vi "main4Ch_Biopsy.vi"() -> ()   [LabVIEW 2024]
doc: "Main VI for FLS imaging system."
uses:
  SubVI/DigitizerConfiguration/FLImDAQ.ctl
  <instrlib>/niScope/Controls/niScope trigger source.ctl
  SubVI/LabJack/LJ Pin Setting.ctl
  ConfigFiles/AimingBeamVideoConfig.ctl
  LaguerreDeconLib/DeconEngineClass/LaguerreDeconEngineClass.lvclass/LaguerreDeconEngineClass.ctl
  <vilib>/Utility/error.llb/DialogType.ctl
  LaguerreDeconLib/DeconEngineClass/LaguerreDeconEngineClass.lvclass
  <vilib>/event_ctls.llb/usereventprio.ctl
  <vilib>/Utility/miscctls.llb/LVMinMaxIncTypeDef.ctl
  SubVI/APD/APDClass.lvclass
  <vilib>/userDefined/High Color/IMAQdx.ctl
  <vilib>/vision/driver/IMAQdx.llb/IMAQdx Camera Control Mode.ctl
  <vilib>/vision/driver/IMAQdx.llb/IMAQdx Acquisition Mode.ctl
  <vilib>/vision/driver/IMAQdx.llb/IMAQdx Buffer Number Mode.ctl
  <vilib>/Analysis/baseanly.llb/Mean (DBL).vi
  SubVI/GlobalVariables.vi
  <vilib>/addons/control/pid/pid.llb/PID (DBL).vi
  <vilib>/Utility/file.llb/Write Delimited Spreadsheet (DBL).vi
  <instrlib>/niScope/Acquire/Fetch/niScope Multi Fetch Binary 16.vi
  <vilib>/Instr/_visa.llb/VISA Configure Serial Port (Instr).vi
  C:/Users/MarcuLab/Desktop/V6 APD LV/V6 APD LV/Kinesis/ThorLabs.MotionControl.KCube.DCServoCLI.dll
  Kinesis/ThorLabs.MotionControl.KCube.DCServoCLI.dll
  C:/Users/MarcuLab/Desktop/V6 APD LV/V6 APD LV/Kinesis/Thorlabs.MotionControl.DeviceManagerCLI.dll
  Kinesis/Thorlabs.MotionControl.DeviceManagerCLI.dll
  C:/Users/MarcuLab/Desktop/V6 APD LV/V6 APD LV/Kinesis/Thorlabs.MotionControl.GenericMotorCLI.dll
  Kinesis/Thorlabs.MotionControl.GenericMotorCLI.dll
  <userlib>/_OpenG.lib/file/file.llb/openg_file.lvlib
  <userlib>/_OpenG.lib/time/time.llb/openg_time.lvlib
  <vilib>/Analysis/NI_AALBase.lvlib
  <vilib>/Utility/miscctls.llb/LVPointTypeDef.ctl
  <vilib>/addons/control/pid/NI_PID_pid.lvlib
  <vilib>/vision/driver/NI_Vision_Acquisition_Software.lvlib
  <resource>/objmgr/imaqdx.rc
panel:
  out "Image 2":T1(plugin-control)
  in  "Live?":bool
  out "Record Backlog 2":i32
  in  "Auto gain ch4":bool=TRUE caption="Auto gain ch3"
  in  "V 4":dbl caption="Gain 3" min=0.0 max=4.67 step=0.1
  out "Gain4":dbl
  out "Lifetime 4":dbl caption="Lifetime 3"
  out "IntR4":dbl format="%#_2g"
  out "SNR4":dbl format="%#_3g"
  out "Channel 4":dbl[][](graph) caption="Channel 3"
  out "RunStartTime":u32
  out "Dig1 Temp":dbl
  out "Dig2 Temp":dbl
  out "Visualization PC video source":T2
  in  "V target(1.0)":dbl=1.0 caption="V target(1.5)" min=0.3 max=1.5 step=0.1 format="%#_4g"
  out "SNR3":dbl format="%#_3g"
  out "SNR2":dbl format="%#_3g"
  out "SNR1":dbl format="%#_3g"
  in  "Show BG removed?":bool=TRUE
  out "IntR3":dbl format="%#_2g"
  out "IntR2":dbl format="%#_2g"
  out "IntR1":dbl format="%#_2g"
  in  "Video Display":bool
  out "Gain3":dbl
  out "Gain2":dbl
  out "Gain1":dbl
  in  "Skip Data Save?":bool
  out "Aq Loop?":bool
  out "ML?":bool
  out "aquisition loop Error Out":errorcluster
  out "Laser f (Hz)":dbl
  out "Record Backlog":i32
  out "Fetch Record #":i32
  out "Sync Success?":bool
  out "Disclamer":picture
  out "Calibration #":i8
  out "BG #":i8
  in  "TCP Connect":bool
  out "Help":string
  in  "355nm Laser toggle":bool caption="355nm 460Hz"
  in  "Cali&iRF alignment":bool
  in  "Background":bool
  in  "Aiming beam toggle":bool caption="445nm 0Hz 20mA"
  out "Lifetime 3":dbl
  out "Lifetime 2":dbl
  in  "Auto gain ch3":bool=TRUE
  in  "Auto gain ch2":bool=TRUE
  in  "Auto gain ch1":bool=TRUE
  out "Run #":i8
  in  "StopButton":bool caption="Stop"
  out "Aquisition Status:":bool
  in  "StartButton":bool caption="Start"
  in  "V 3":dbl caption="Gain 3" min=0.0 max=4.68 step=0.1
  in  "V 2":dbl caption="Gain 2" min=0.0 max=4.62 step=0.1
  out "Lifetime 1":dbl
  in  "V 1":dbl caption="Gain 1" min=0.0 max=4.66 step=0.1 format="%#_4g"
  in  "Video Source":enum32{"Camera", "FrameGrabber"}(radio)
  out "Case #":string
  out "System Hardware Connection Status":T3
  out "Channel 3":dbl[][](graph)
  out "Channel 2":dbl[][](graph)
  out "Channel 1":dbl[][](graph)
  in  "Tab Control":T4(tab)
  in  "ScanRange(mm)":dbl=25.0
  in  "SerialNumber(Slow)":string="27000986"
  out "SlowAxisInfo":T5
  out "SlowAxisStatus":T6
  out "PNG write time (ms)":dbl(graph)
  in  "VideoMode":u32=12
  out "Acquired Frames/s":dbl
  out "FLIm 1st point time":dbl format="%_19f"
  out "Cam error out":errorcluster
  out "display loop timing(ms)":u32
  out "Aquisition loop timing(ms)":u32 format="%.2f"
  out "DisplayLoop":i32
  out "PID loop":i32 caption="processing loop"
  out "PID loop timing(ms)":u32 caption="processing loop timing(ms)"
  out "laser EM lamp V":dbl format="%0.6f"
  out "Decon Loop timing (ms)":dbl
  out "Auisition Loop idx":i32
  out "LJ process (ms)":u32
  out "LJ time(ms)":u32[](array[numeric])
  out "output variable":i32
  out "Lifetime (ns)":dbl(graph)
  out "Waveform Chart":dbl(graph)
  in  "Truncation":u32=600
  out "iRF Graph":dbl[][](graph)
  in  "Show BG":bool
  out "iRF length":i32
  out "BG length":i32
  out "data length":i32
  out "SysConfigCluster":T7
  out "LJ Pinout":T8={"Ch1 Bias"="DAC0", "Ch2 Bias"="DAC1", "Ch3 Bias"="DAC2", "Ch4 Bias"="DAC0", "355 PWM"="FIO0", "AimingBeam PWM"="FIO2", "Laser Ready"="FIO3", "Interlock"="FIO1", "Laser Start/Stop"="FIO1", "Red LED"="FIO1", "Green LED"="DIO3", "Foot Pedal"="DIO15"}
  out "FLImDAQ":T9={"Digitizer 1"="", "Digitizer 2"="", "Channel"=enum."Channel 0", "trigger source"="VAL_EXTERNAL", "trigger level"=0.5, "trigger delay"=1.35e-07, "min sample rate"=12500000000.0, "min record length"=2500, "vertical range"=1.0, "vertical offset"=-0.25, "Waveform to Avg"=2000} caption="FLIm DAQ Configuration" {"trigger delay" format="%^#.4e"; "trigger level" min=0.0 max=3.5 step=0.5 format="%.2f"; "vertical offset" format="%.4f"; "vertical range" format="%.2f"; "min sample rate" format="%#.2p"}
  in  "Sys Reconfig":bool
  out "PID loop error out":errorcluster caption="processing Error Out"
  out "decon error out":errorcluster
  out "Laser Rep Rate":dbl
  out "V4 Size":i32 caption="V3 Size"
  in  "Data Class":enum16{"Data", "BG", "Cali"}(ring)
  out "V1 Size":i32
  out "V2 Size":i32
  out "V3 Size":i32
  out "data Size":i32[](array[numeric])
  out "State log":string
  in  "Ch4 PID gains":T11={"proportional gain (Kc)"=30.0, "integral time (Ti, min)"=0.0003, "derivative time (Td, min)"=1e-05}
  in  "Ch3 PID gains":T11={"proportional gain (Kc)"=30.0, "integral time (Ti, min)"=0.0003, "derivative time (Td, min)"=1e-05}
  in  "Ch2 PID gains":T11={"proportional gain (Kc)"=30.0, "integral time (Ti, min)"=0.0003, "derivative time (Td, min)"=1e-05}
  in  "Ch1 PID gains":T11={"proportional gain (Kc)"=30.0, "integral time (Ti, min)"=0.0003, "derivative time (Td, min)"=1e-05}
  in  "Quit":bool
  in  "Radio Buttons":T12(radio)=enum."Ch2" caption="DeCon Chan"
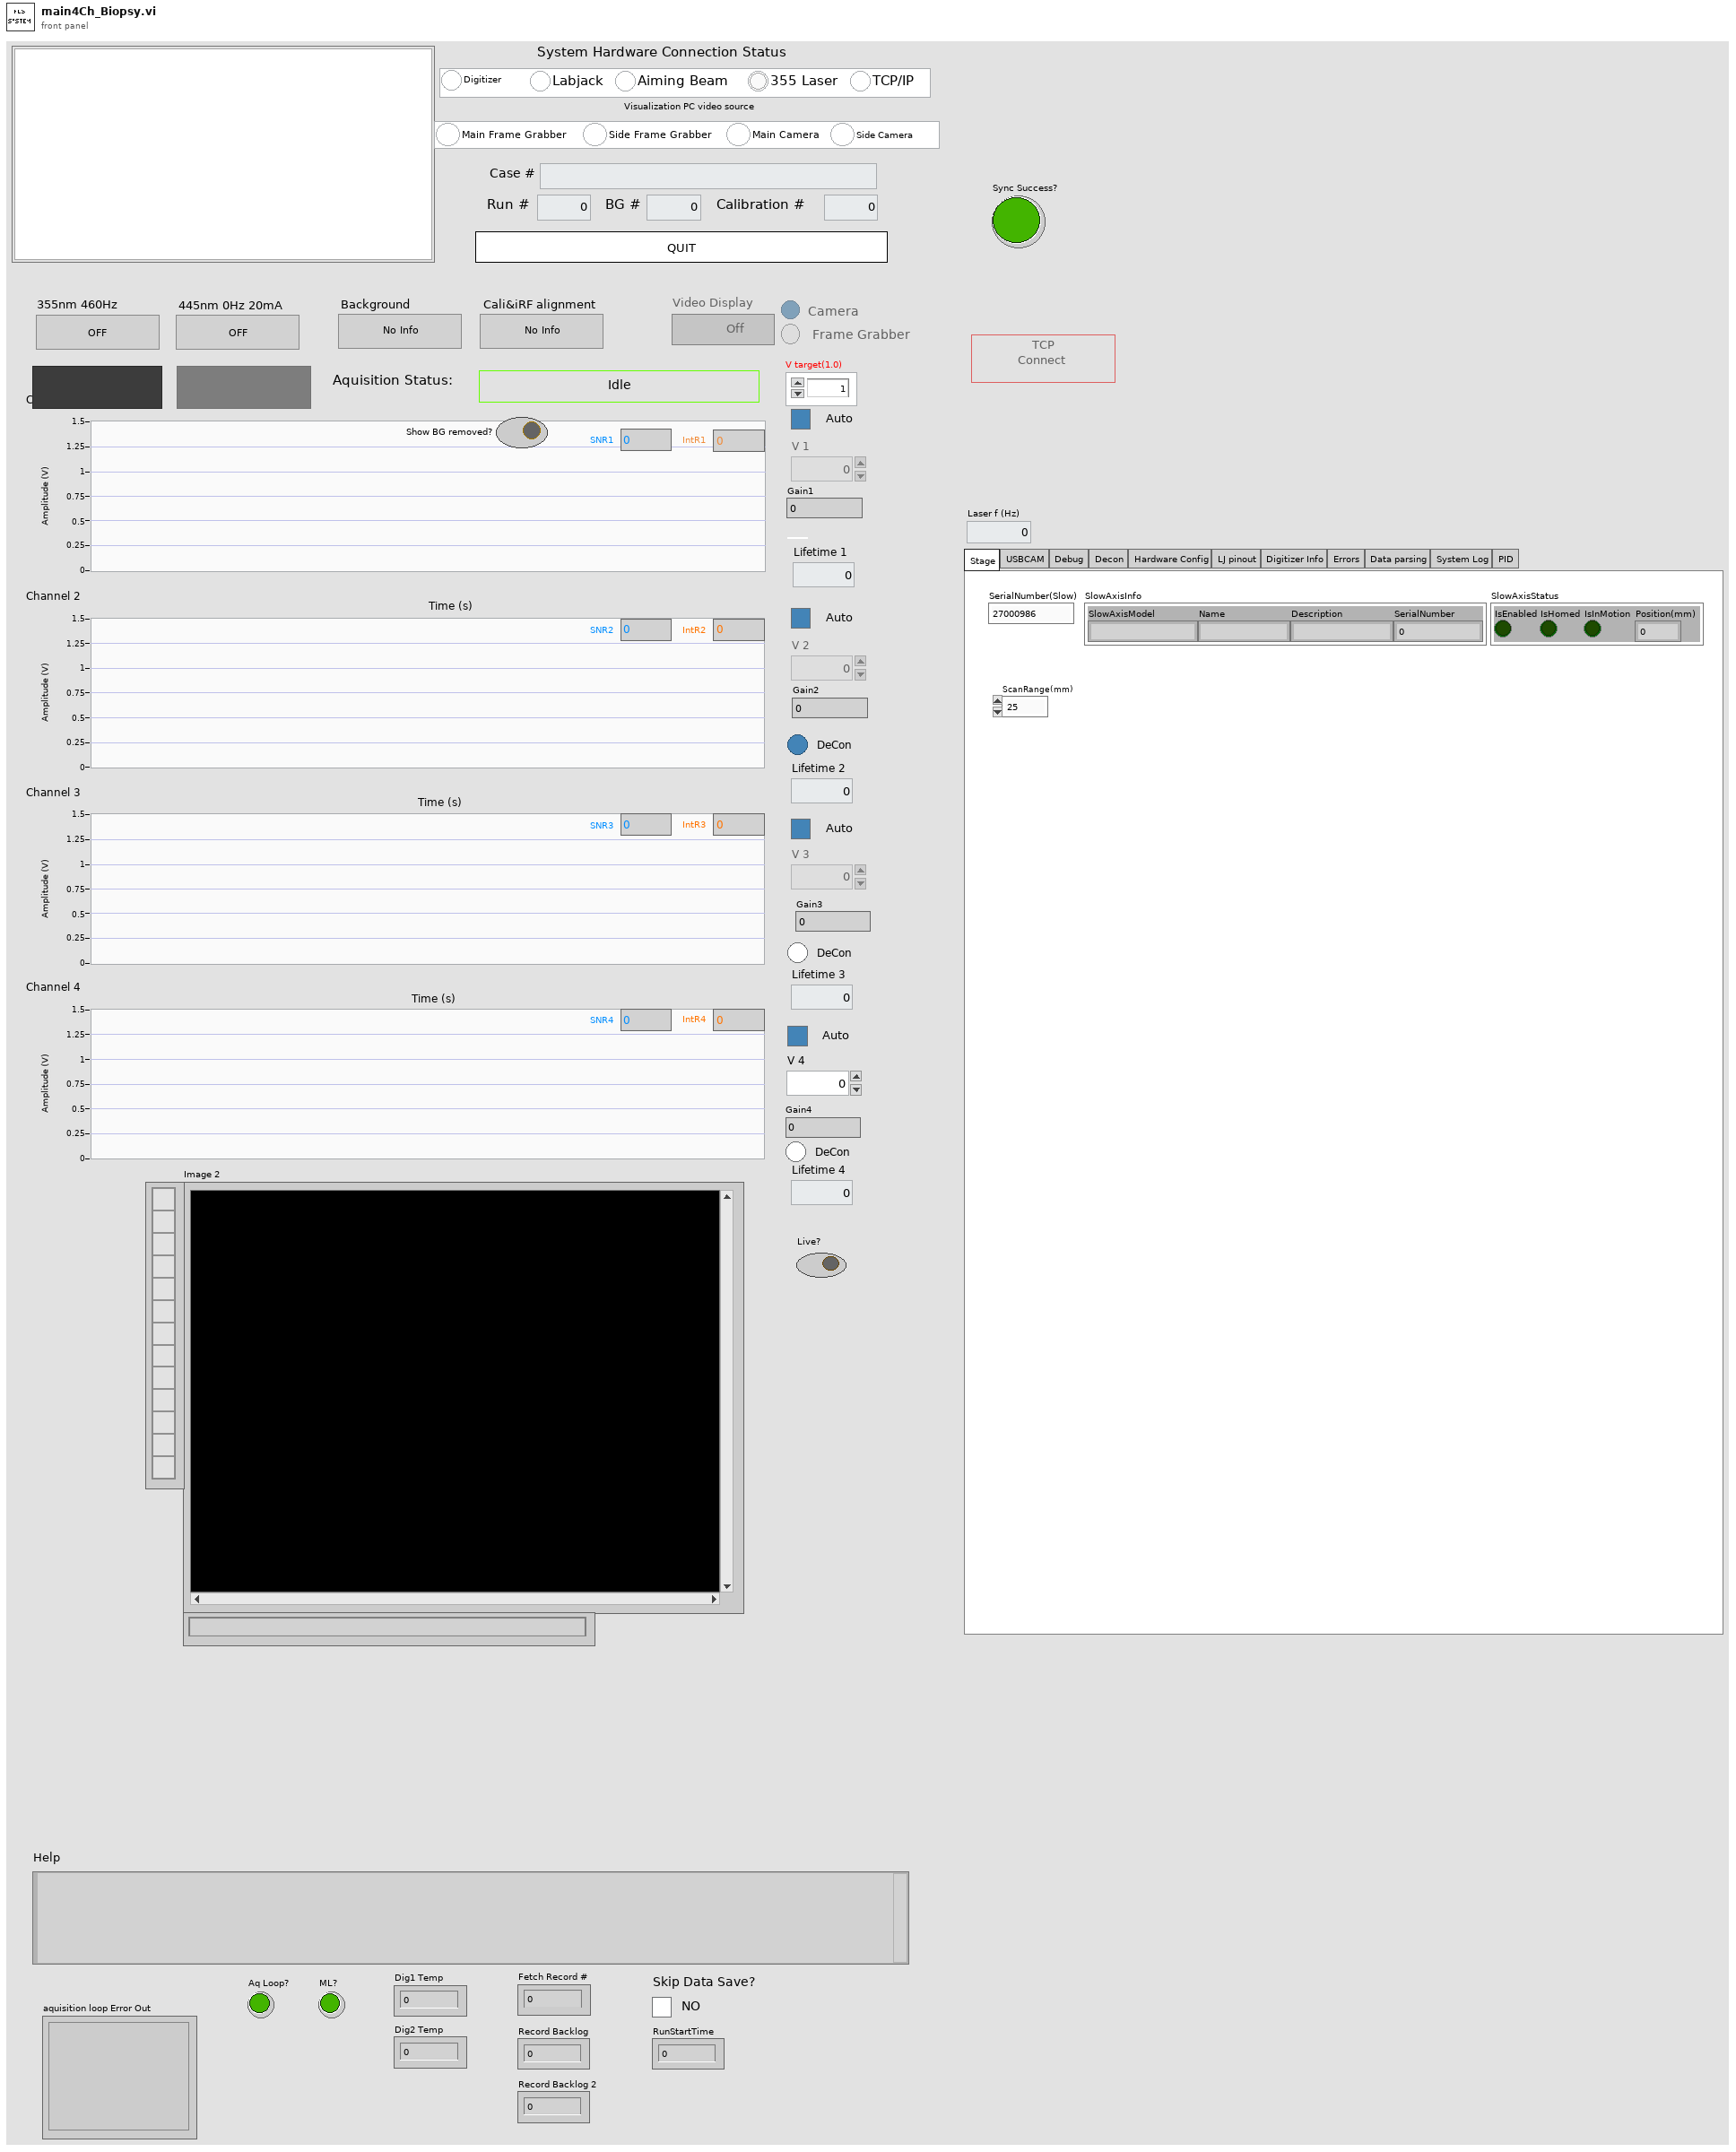
[diagram p1: front panel]
types:
  T1 = typedef "IMAQ Image.ctl" = refnum<image>
  T2 = cluster{"Main Frame Grabber":bool, "Side Frame Grabber":bool, "Main Camera":bool, "Side Camera":bool}
  T3 = cluster{"Digitizer":bool, "Labjack":bool, "Aiming Beam":bool, "355 Laser":bool, "TCP/IP":bool}
  T4 = enum32{"Stage", "USBCAM", "Debug", "Decon", "Hardware Config", "LJ pinout", "Digitizer Info", "Errors", "Data parsing", "System Log", "PID"}
  T5 = cluster{"SlowAxisModel":string, "Name":string, "Description":string, "SerialNumber":u32}
  T6 = cluster{"IsEnabled":bool, "IsHomed":bool, "IsInMotion":bool, "Position(mm)":dbl}
  T7 = cluster{"Ch1Enable?":bool, "Ch2Enable?":bool, "Ch3Enable?":bool, "Ch1AutoGain?":bool, "Ch2AutoGain?":bool, "Ch3AutoGain?":bool, "AimingBeamEnable?":bool}
  T8 = typedef "LJ Pin Setting.ctl" = cluster{"Ch1 Bias":string, "Ch2 Bias":string, "Ch3 Bias":string, "Ch4 Bias":string, "355 PWM":string, "AimingBeam PWM":string, "Laser Ready":string, "Interlock":string, "Laser Start/Stop":string, "Red LED":string, "Green LED":string, "Foot Pedal":string}
  T9 = typedef "FLImDAQ.ctl" = cluster{"Digitizer 1":refnum<k15>, "Digitizer 2":refnum<k15>, "Channel":enum16{"Channel 0", "Channel 1", "Channel 0&1"}, "trigger source":T10, "trigger level":dbl, "trigger delay":dbl, "min sample rate":dbl, "min record length":i32, "vertical range":dbl, "vertical offset":dbl, "Waveform to Avg":i16}
  T10 = typedef "niScope trigger source.ctl" = string
  T11 = cluster{"proportional gain (Kc)":dbl, "integral time (Ti, min)":dbl, "derivative time (Td, min)":dbl}
  T12 = enum32{"No Selection", "Ch1", "Ch2", "Ch3", "Ch4"}
  T13 = cluster{"remote start event":refnum<user-event>, "remote stop  event":refnum<user-event>}
  T14 = enum8{"Enabled", "Disabled", "Disabled and Grayed Out"}
  T15 = enum16{"open", "replace", "create", "open or create", "replace or create", "replace or create with confirmation"}
  T16 = cluster{"CH1":dbl[][], "CH2":dbl[][], "CH3":dbl[][], "CH4":dbl[][], "Gain cluster":cluster{"V1":dbl, "V2":dbl, "V3":dbl, "V4":dbl}}
  T17 = cluster{"idx":i32, "CH1&2":dbl[][], "CH3":dbl[][], "V cluster":cluster{"V1":dbl, "V2":dbl, "V3":dbl, "V4":dbl}}
  T18 = cluster{"Ch1 iRF":dbl[], "Ch2 iRF":dbl[], "Ch3 iRF":dbl[], "Ch4 iRF":dbl[]}
  T19 = enum16{"open", "open or create", "create or replace", "create", "open (read-only)"}
  T20 = enum32{"Invalid", "Standard", "Closed", "Hidden", "Minimized", "Maximized"}
  T21 = enum32{"invalid app kind", "Development System", "Run Time System", "Student Edition", "Embedded LabVIEW", "Evaluation", "Custom"}
  T22 = typedef "usereventprio.ctl" = enum32{"high priority", "normal priority"}
  T23 = enum32{"Bad", "Idle", "Run top level", "Running"}
  T24 = enum16{"Standard", "Buffered", "CRLF", "Immediate"}
  T25 = typedef "NI_Vision_Acquisition_Software.lvlib/IMAQdx Camera Control Mode.ctl" = enum32{"Controller", "Listener"}
  T26 = typedef "IMAQdx.ctl" = refnum<k21>
  T27 = typedef "NI_Vision_Acquisition_Software.lvlib/IMAQdx Acquisition Mode.ctl" = enum32{"One Shot", "Continuous"}
  T28 = typedef "AimingBeamVideoConfig.ctl" = cluster{"DeCon Channel":enum16{"1", "2", "3"}, "Scale Bar":bool, "Scale Low":dbl, "Scale High":dbl, "ANSI":dbl, "Radius":dbl, "3D?":bool, "Firefly?":bool, "Pentero?":bool}
  T29 = cluster{"Core":cluster{"Current VI Reference":refnum<vi>, "Close Panel on Exit?":bool}, "SysConfigCluster":cluster{"Ch1Enable?":bool, "Ch2Enable?":bool, "Ch3Enable?":bool, "Ch1AutoGain?":bool, "Ch2AutoGain?":bool, "Ch3AutoGain?":bool, "AimingBeamEnable?":bool}, "System Status":cluster{"Digitizer":bool, "Labjack":bool, "Aiming Beam":bool, "355 Laser":bool, "TCP/IP":bool}, "IDs":cluster{"RunID":i8, "BG ID":i8, "Cali ID":i8}, "CaseID":string, "DefaultPath":path, "Pathes":cluster{"DataPath":path, "BG Path":path, "iRFPath":path, "CaliPath":path}, "FLImDAQ":cluster{"resource name":refnum<k15>, "resource name 2":refnum<k15>, "Channel":enum16{"Channel 0", "Channel 1", "Channel 0&1"}, "trigger source":T10, "trigger level":dbl, "trigger delay":dbl, "min sample rate":dbl, "min record length":i32, "vertical range":dbl, "vertical offset":dbl, "Waveform to Avg":i32}, "SysRunning?":bool, "AB Cluster":cluster{"Aiming Beam COM Port":refnum<visa-resource-name>, "Min Current":dbl, "Max Current":dbl, "Default Current":dbl, "Freq":i32}, "LJ Pinout":T8, "355 PWM setting":cluster{"DIO_EF_CLOCK1_DIVISOR":i16, "DIO_EF_CLOCK1_ROLL_VALUE":i32, "DIO#_EF_INDEX":i16, "DIO#_EF_OPTIONS":i16, "DIO#_EF_CONFIG_A":i32}, "AB PWM setting":cluster{"DIO_EF_CLOCK1_DIVISOR":i16, "DIO_EF_CLOCK1_ROLL_VALUE":i32, "DIO#_EF_INDEX":i16, "DIO#_EF_OPTIONS":i16, "DIO#_EF_CONFIG_A":i32}, "Last Trigger":u32, "niTClk sessions":refnum<k20>[], "Laser start tic":u32, "TCP attempt count":i32, "Ch1Data":dbl[][], "Ch2Data":dbl[][], "Ch3Data":dbl[][], "Ch4Data":dbl[][], "V1":dbl[], "V2":dbl[], "V3":dbl[], "V4":dbl[], "SlowTimer":u32, "FastTimer":u32, "listener ID":refnum<k5>, "TempPath":path, "CaliPath":path, "LED vi reference":refnum<vi>, "Aquisition Timer":u32, "APDSerialNum":cluster{"Ch1APDSerial#":string, "Ch2APDSerial#":string, "Ch3APDSerial#":string, "Ch4APDSerial#":string}, "VideoConfig":T28, "LED vi ref open?":bool, "video source":cluster{"Main Frame Grabber":bool, "Side Frame Grabber":bool, "Main Camera":bool, "Side Camera":bool}, "bothVidSourceAvail":bool, "StageSerial":string, "DeviceHandle":refnum<k24>, "StageHomed?":bool}
  T30 = typedef "LVCursorListTypeDef.ctl" = cluster{"Name":string, "Color":u32, "Style":u8, "Point Style":u8, "Name Visible":bool, "Allow Drag":bool, "Cursor Mode":u32, "Plot":i32, "Index":i32, "Position":cluster{"X":dbl, "Y":dbl}, "X Scale":u32, "Y Scale":u32, "Watch Plots":i32[], "Watch All Plots":bool, "Plot Area":i32, "Label Offset":cluster{"X":dbl, "Y":dbl}}[]
  T31 = cluster{"Name":string, "Color":u32, "Style":u8, "Point Style":u8, "Name Visible":bool, "Allow Drag":bool, "Cursor Mode":u32, "Plot":i32, "Index":i32, "Position":cluster{"X":dbl, "Y":dbl}, "X Scale":u32, "Y Scale":u32, "Watch Plots":i32[], "Watch All Plots":bool, "Plot Area":i32, "Label Offset":cluster{"X":dbl, "Y":dbl}}
  T32 = cluster{"Ch1APDSerial#":string, "Ch2APDSerial#":string, "Ch3APDSerial#":string, "Ch4APDSerial#":string}
  T33 = cluster{"DataPath":path, "BG Path":path, "iRFPath":path, "CaliPath":path}
  T34 = cluster{"DIO_EF_CLOCK1_DIVISOR":i16, "DIO_EF_CLOCK1_ROLL_VALUE":i32, "DIO#_EF_INDEX":i16, "DIO#_EF_OPTIONS":i16, "DIO#_EF_CONFIG_A":i32}
  T35 = cluster{"Aiming Beam COM Port":refnum<visa-resource-name>, "Min Current":dbl, "Max Current":dbl, "Default Current":dbl, "Freq":i32}
  T36 = cluster{"resource name":refnum<k15>, "resource name 2":refnum<k15>, "Channel":enum16{"Channel 0", "Channel 1", "Channel 0&1"}, "trigger source":T10, "trigger level":dbl, "trigger delay":dbl, "min sample rate":dbl, "min record length":i32, "vertical range":dbl, "vertical offset":dbl, "Waveform to Avg":i32}
  T37 = cluster{"Current VI Reference":refnum<vi>, "Close Panel on Exit?":bool}
  T38 = cluster{"Channel 1":dbl[], "Channel 2":dbl[], "Channel 3":dbl[], "Channel 4":dbl[]}
  T39 = cluster{"V 1":dbl[], "V 2":dbl[], "V 3":dbl[], "V 4":dbl[]}
  T40 = cluster{"Ch1 WF":dbl[], "Ch2 WF":dbl[], "Ch3 WF":dbl[], "Ch4 WF":dbl[], "V1":dbl, "V2":dbl, "V3":dbl, "V4":dbl}
  T41 = typedef "iRFData.ctl" = cluster{"dt":dbl, "NumOfWFs":i32, "WFLength":i32, "iRFCtrlV":dbl[], "iRFWFsAvg":dbl[][], "iRFRaw":dbl[][]}
  T42 = cluster{"mean":dbl, "mean":dbl, "mean":dbl, "mean":dbl}
  T43 = cluster{"V1":dbl, "V2":dbl, "V3":dbl, "V4":dbl}[]
  T44 = cluster{"DataPath":path, "CaseID":string, "RunID":i16, "Ch1Data":dbl[][], "Ch2Data":dbl[][], "Ch3Data":dbl[][], "Ch4Data":dbl[][], "V1":dbl[], "V2":dbl[], "V3":dbl[], "V4":dbl[], "LaserRepRate":u16, "WFAverage":i16, "RunStartTime":u64}
  T45 = typedef "DialogType.ctl" = u16
  T46 = typedef "LJ PWM Setting.ctl" = cluster{"DIO_EF_CLOCK1_DIVISOR":i16, "DIO_EF_CLOCK1_ROLL_VALUE":i32, "DIO#_EF_INDEX":i16, "DIO#_EF_OPTIONS":i16, "DIO#_EF_CONFIG_A":i32}
  T47 = typedef "AimingBeam.ctl" = cluster{"Aiming Beam COM Port":refnum<visa-resource-name>, "Min Current":dbl, "Max Current":dbl, "Default Current":dbl, "Frequency(Hz)":u32}
  T48 = cluster{"DC1":i32, "DC2":i32, "BG1":i32, "BG2":i32}
  T49 = typedef "LVMinMaxIncTypeDef.ctl" = cluster{"Minimum":dbl, "Maximum":dbl, "Increment":dbl}
  T50 = typedef "LVBoundsTypeDef.ctl" = cluster{"Width":u32, "Height":u32}
  T51 = typedef "imagedata.ctl" = cluster{"image type":i32, "image depth":i32, "image":u8[], "mask":u8[], "colors":u32[], "Rectangle":cluster{"left":i16, "top":i16, "right":i16, "bottom":i16}}
  T52 = cluster{"DC Idx1":i32, "DC Idx2":i32, "BG Idx1":i32, "BG Idx2":i32}
  T53 = cluster{"IsEnabled":bool, "IsHomed":bool, "IsInMotion":bool, "Position":dbl}
  T54 = typedef "LVPointTypeDef.ctl" = cluster{"Horizontal":i16, "Vertical":i16}
  T55 = cluster{"actualSamples":i32, "absoluteInitialX":dbl, "relativeInitialX":dbl, "xIncrement":dbl, "offset":dbl, "gain":dbl, "reserved1":dbl, "reserved2":dbl}[]
  T56 = cluster{"V1 out":dbl, "V2 out":dbl, "V3 out":dbl, "V3 out":dbl}
  T57 = cluster{i32, dbl[][], dbl[][], cluster{"V1 out":dbl, "V2 out":dbl, "V3 out":dbl, "V3 out":dbl}}
  T58 = cluster{dbl[][], dbl[][], dbl[][], dbl[][], "V cluster":cluster{"V1":dbl, "V2":dbl, "V3":dbl, "V4":dbl}}
  T59 = typedef "NI_Vision_Acquisition_Software.lvlib/IMAQdx Buffer Number Mode.ctl" = enum32{"Next", "Last", "Buffer Number", "Every", "Last New"}
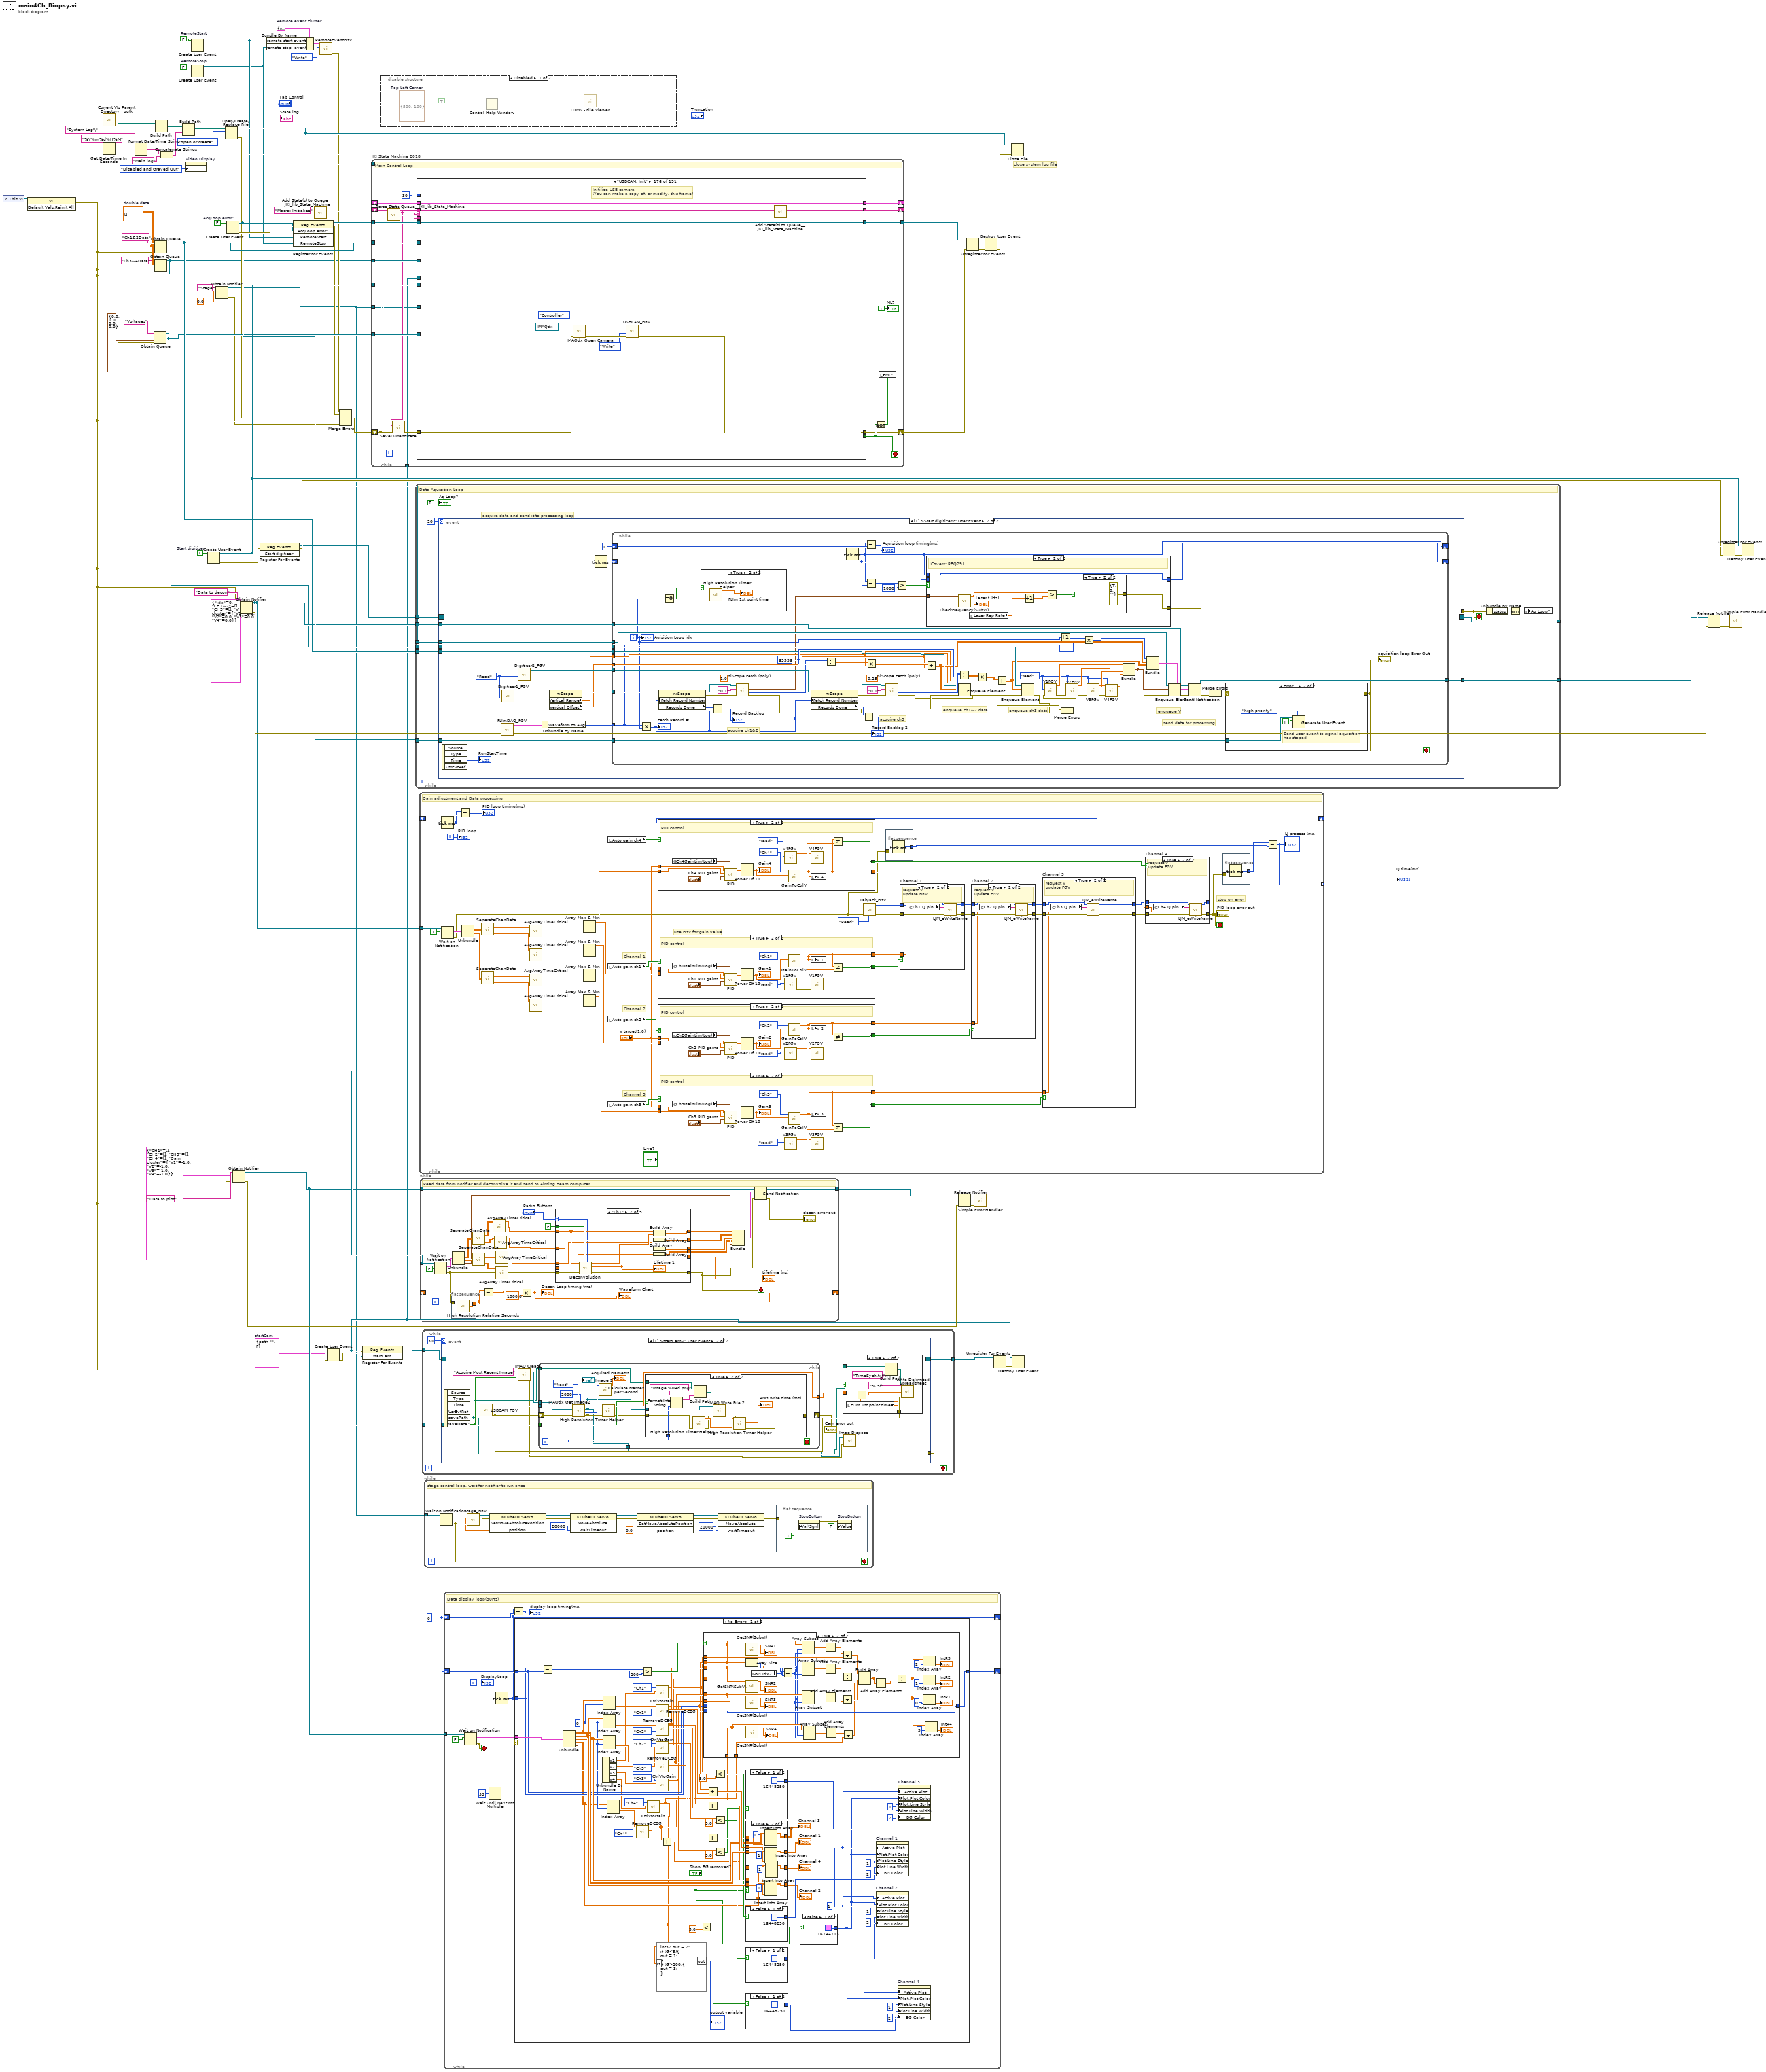
[diagram p0: block diagram]
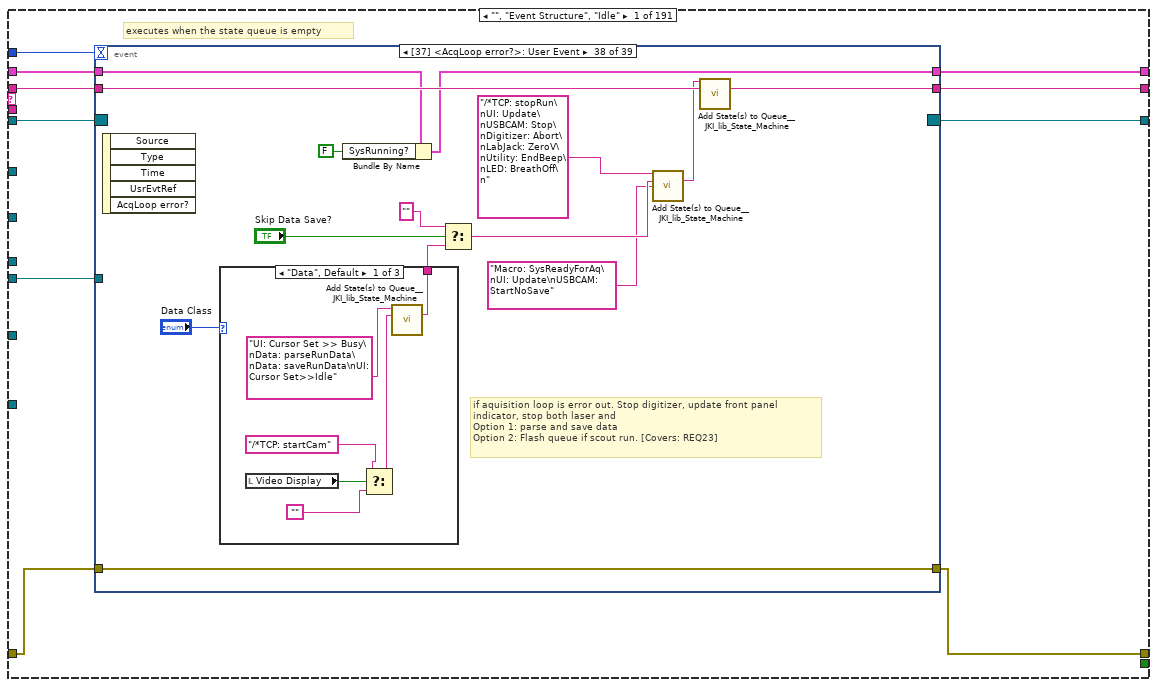
[diagram p2: hidden frame]
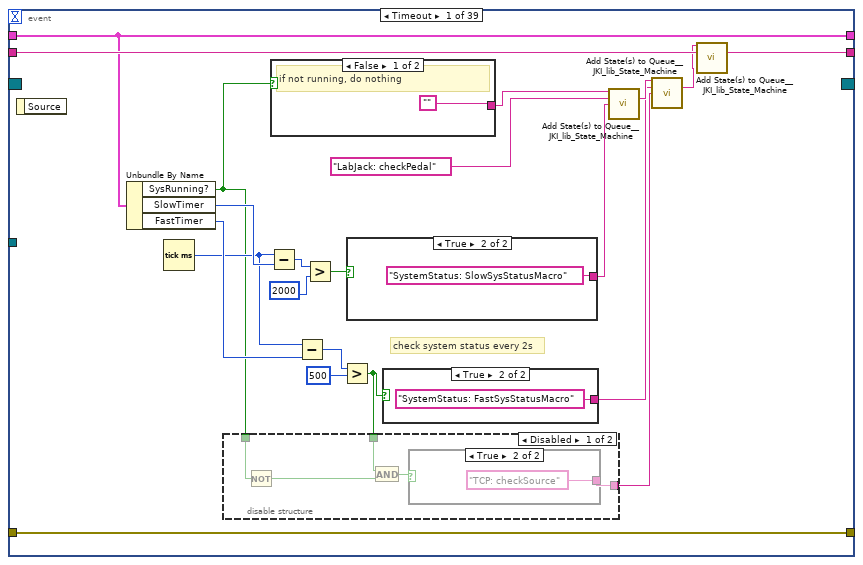
[diagram p3: hidden frame]
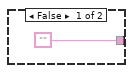
[diagram p4: hidden frame]
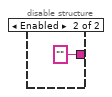
[diagram p5: hidden frame]
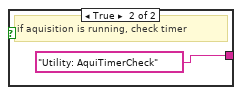
[diagram p6: hidden frame]
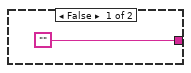
[diagram p7: hidden frame]
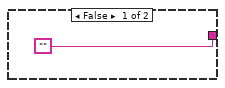
[diagram p8: hidden frame]
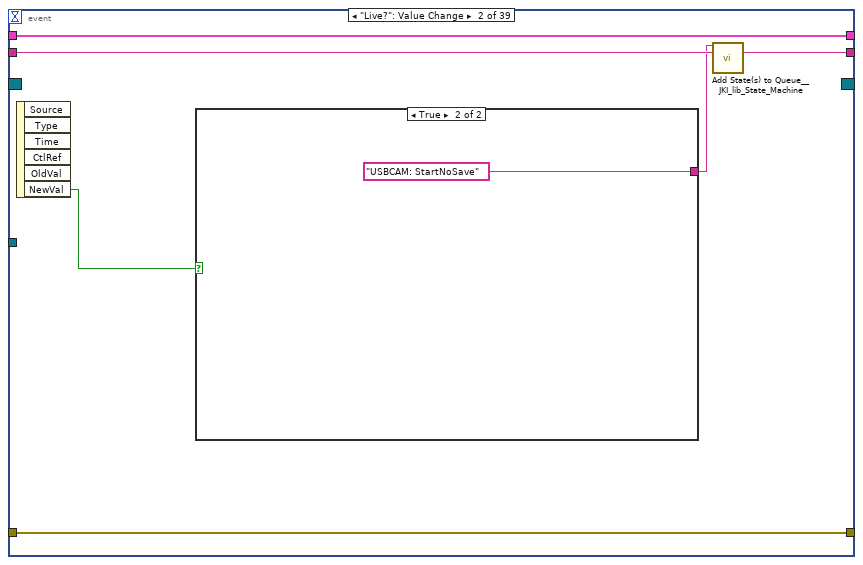
[diagram p9: hidden frame]
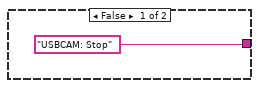
[diagram p10: hidden frame]
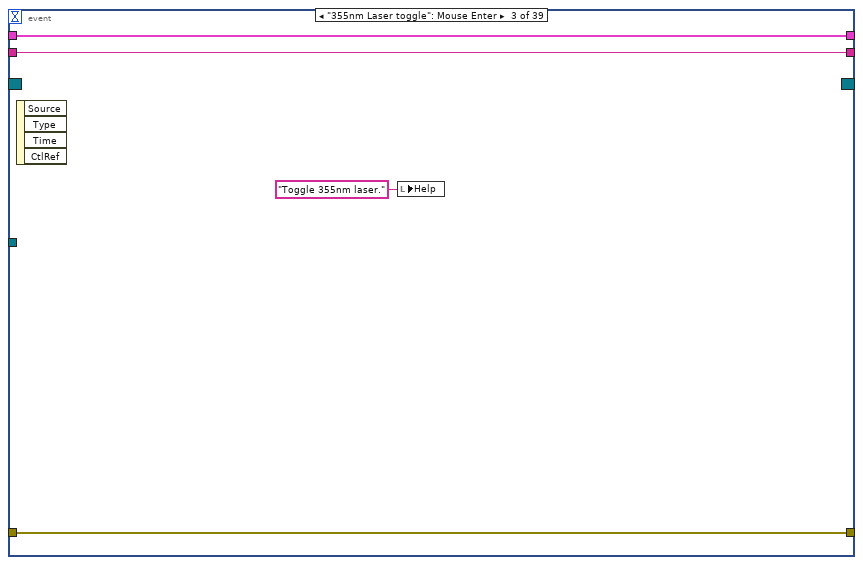
[diagram p11: hidden frame]
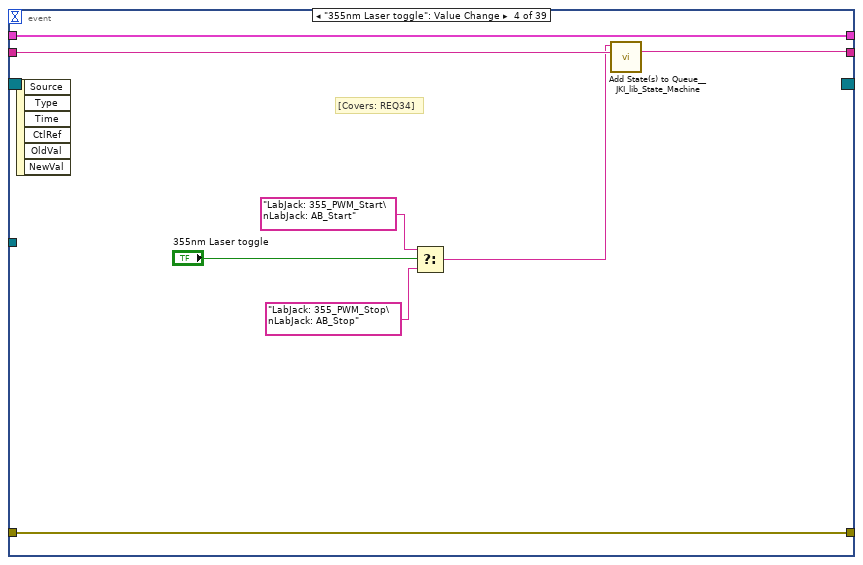
[diagram p12: hidden frame]
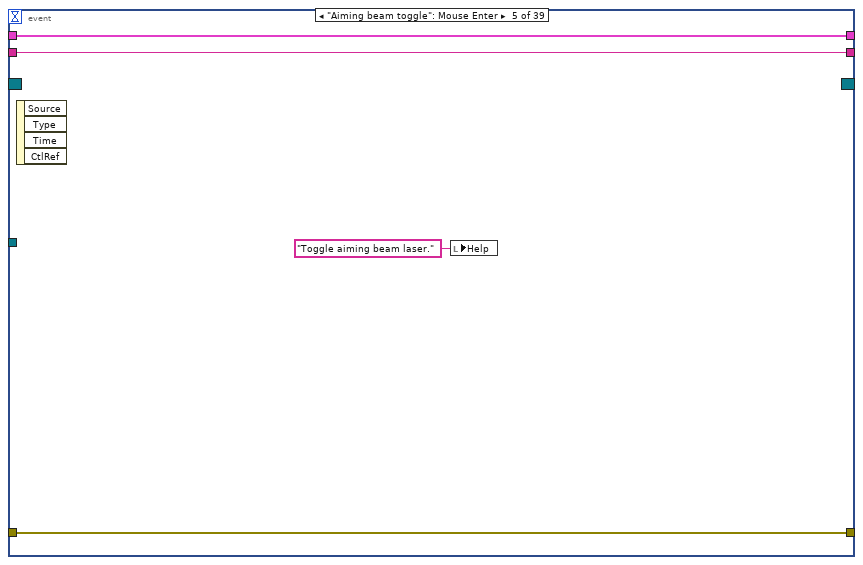
[diagram p13: hidden frame]
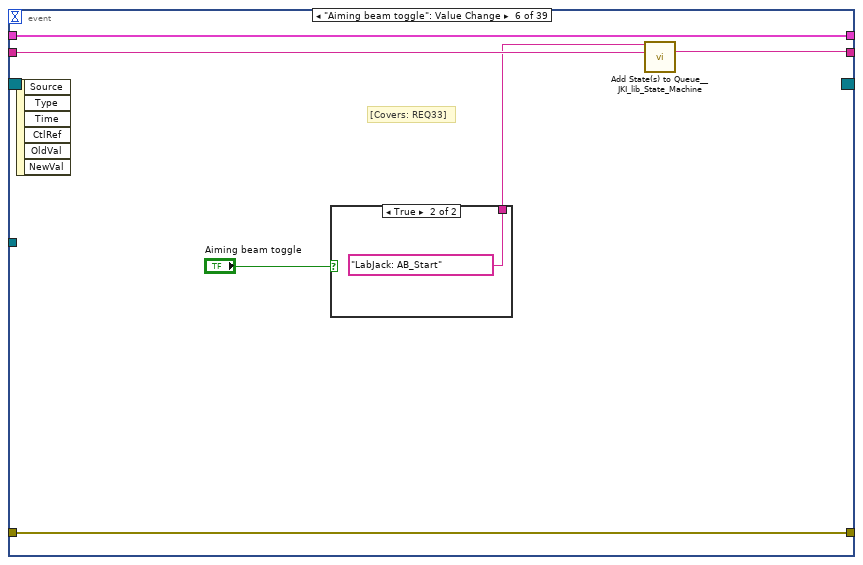
[diagram p14: hidden frame]
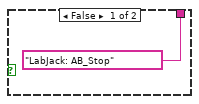
[diagram p15: hidden frame]
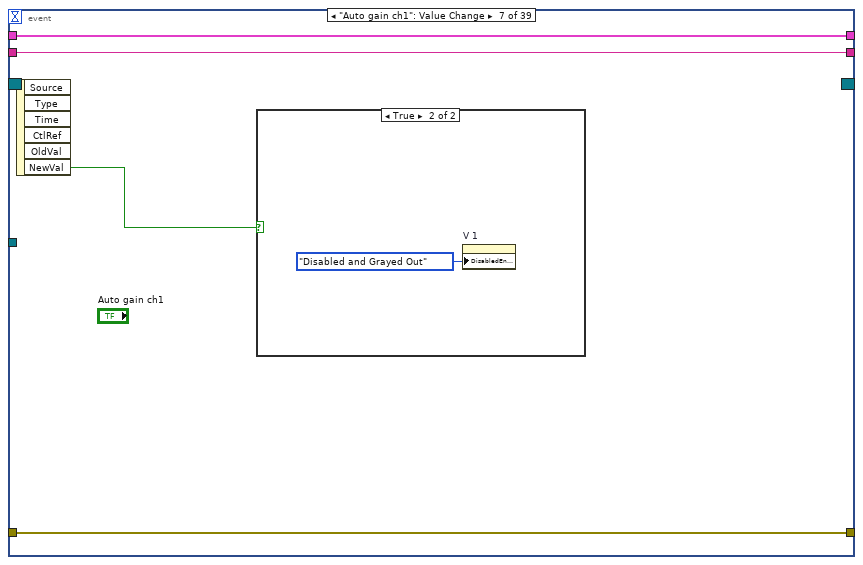
[diagram p16: hidden frame]
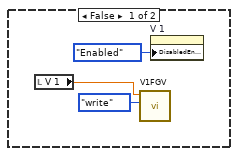
[diagram p17: hidden frame]
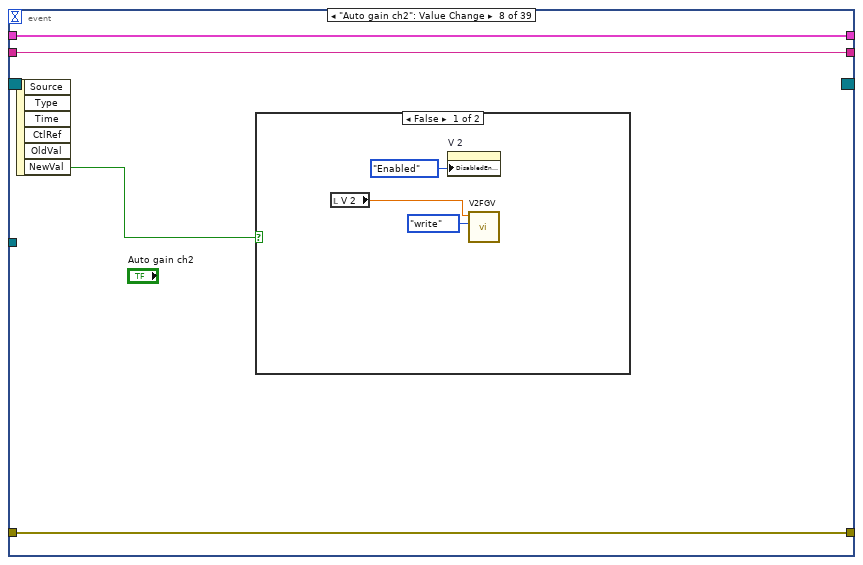
[diagram p18: hidden frame]
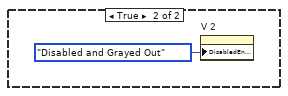
[diagram p19: hidden frame]
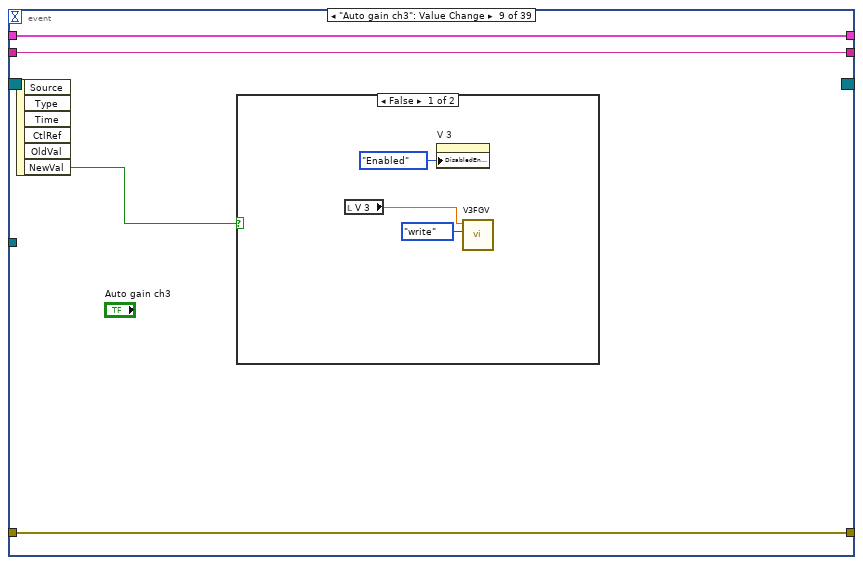
[diagram p20: hidden frame]
diagram:
  w12 = cluster{"savePath":path, "saveData?":bool} {"savePath"=path "", "saveData?"=FALSE}  # startCam
  w20 = T13 {"remote start event"=refnum, "remote stop  event"=refnum}  # Remote event cluster
  w23 = FALSE  # RemoteStop
  w24 = FALSE  # RemoteStart
  w27 = u32 0 ("millisecond timer value")
  w57 = FALSE  # AcqLoop error?
  w67 = TRUE  # Start digitizer
  w70 = dbl[][] []  # double data
  # "close system log file"
  n1 = control-ref of="This VI"() -> (w72:refnum<vi>)
  n2 = invoke on="Invoke Node" class="VI" method="Default Vals.Reinit All"(reference=w72) -> (error out=w11:errorcluster)  [unwired: 2 in, 2 out]
  n3 = call <userlib>:"Current VIs Parent Directory__ogtk.vi"() -> ("Parent Directory (+ Relative)"=w43:path)  [unwired: 5 in]
  n4 = Get Date/Time In Seconds() -> (seconds since 1Jan1904=w41:timestamp)
  n5 = Format Date/Time String(time format string (%c)="%Y%m%d%H%M", seconds (now)=w41) -> (date/time string=w38:string)  [unwired: 1 in]
  n6 = Obtain Queue(name (unnamed)="Voltages", element data type=cluster{"V1":dbl, "V2":dbl, "V3":dbl, "V4":dbl} {"V1"=0.0, "V2"=0.0, "V3"=0.0, "V4"=0.0}, error in (no error)=w11) -> (queue out=w44:refnum<queue>)  [unwired: 2 in, 2 out]
  n7 = Obtain Queue(name (unnamed)="Ch3&4Data", element data type=w70, error in (no error)=w11) -> (queue out=w8:refnum<queue>)  [unwired: 2 in, 2 out]
  n8 = Obtain Queue(name (unnamed)="Ch1&2Data", element data type=w70, error in (no error)=w11) -> (queue out=w68:refnum<queue>)  [unwired: 2 in, 2 out]
  n9 = Build Path(base path=w43, name or relative path="System Log\\") -> (appended path=w34:path)
  n10 = Concatenate Strings(w38, "Main.log" ("string")) -> (w36:string)
  n11 = Build Path(base path=w34, name or relative path=w36) -> (appended path=w39:path)
  n12 = property on="Video Display" class="Bool (strict)"("DisabledEnum"=T14."Disabled and Grayed Out" ("Disabled")) -> ()  [unwired: 2 in, 2 out]
  n13 = Create User Event(user event datatype=w24) -> (user event=w22:refnum<user-event>)  [unwired: 1 in, 1 out]
  n14 = Create User Event(user event datatype=w23) -> (user event=w21:refnum<user-event>)  [unwired: 1 in, 1 out]
  n15 = Create User Event(user event datatype=w67, error in=w11) -> (user event=w56:refnum<user-event>, error out=w48:errorcluster)
  n16 = Obtain Notifier(name (unnamed)="Stage", notification data type=0.0) -> (notifier out=w1:refnum<notifier>, error out=w2:errorcluster)  [unwired: 2 in, 1 out]
  n17 = Open/Create/Replace File(file path (use dialog)=w39, operation (0:open)=T15."open or create") -> (refnum out=w31:refnum<file>, error out=w32:errorcluster)  [unwired: 4 in, 1 out]
  n18 = Create User Event(user event datatype=w57) -> (user event=w47:refnum<user-event>, error out=w49:errorcluster)  [unwired: 1 in]
  n19 = Obtain Notifier(name (unnamed)="Data to plot", notification data type=T16 {"CH1"=[], "CH2"=[], "CH3"=[], "CH4"=[], "Gain cluster"={"V1"=-1.0, "V2"=-1.0, "V3"=-1.0, "V4"=-1.0}}, error in (no error)=w11) -> (notifier out=w25:refnum<notifier>, error out=w52:errorcluster)  [unwired: 1 in, 1 out]
  n20 = Obtain Notifier(name (unnamed)="Data to decon", notification data type=T17 {"idx"=0, "CH1&2"=[], "CH3"=[], "V cluster"={"V1"=0.0, "V2"=0.0, "V3"=0.0, "V4"=0.0}}, error in (no error)=w11) -> (notifier out=w29:refnum<notifier>, error out=w61:errorcluster)  [unwired: 1 in, 1 out]
  n21 = register-events(error in=w48, w56) -> (reference out=w58:refnum<event-registration>, error out=w64:errorcluster)  [unwired: 1 in]
  n22 = Bundle By Name(cluster=w20, "remote start event"=w22, "remote stop  event"=w21) -> (w18:T13)
  n23 = register-events(error in=w49, w47, w22, w21) -> (reference out=w51:refnum<event-registration>, error out=w17:errorcluster)  [unwired: 1 in]
  n24 = call <vilib>:"Add State(s) to Queue__JKI_lib_State_Machine.vi"("State(s) in (\"\")"="Macro: Initialize") -> ("States Out"=w74:string)  [unwired: 14 in]
  n25 = call "RemoteEventFGV.vi"("Operation (Read)"=enum16{"Read", "Write"}."Write", "Remote Event in"=w18) -> ("Error Out"=w14:errorcluster)  [unwired: 8 in, 1 out]
  n26 = Create User Event(user event datatype=w12, error in=w11) -> (user event=w5:refnum<user-event>, error out=w10:errorcluster)
  n27 = Merge Errors(w14, w17, w32, w11, w2) -> (w33:errorcluster)
  n28 = register-events(error in=w10, w5) -> (reference out=w9:refnum<event-registration>)  [unwired: 1 in, 1 out]
  n29 = while "JKI State Machine 2018" {
    shift-right: [w93] -> _
    shift-left: _ -> [w92]
    shift-right: [w77] -> w16
    shift-left: w33 -> [w79]
    shift-right: [w94] -> _
    shift-left: w74 -> [w95]
    tunnel: w68 -> [w90]
    tunnel: w8 -> [w89]
    tunnel: w56 -> [w88]
    tunnel: w51 -> [w87]
    tunnel: [w86] -> w50
    tunnel: w44 -> [w82]
    tunnel: w31 -> [w81]
    tunnel: w5 -> [w76]
    tunnel: w1 -> [w75]
    stop <- w85 stop-if-true
    # "Main Control Loop"
    n30 = call <vilib>:"Parse State Queue__JKI_lib_State_Machine.vi"("State Queue"=w95, "Error In (no error)"=w79) -> ("Remaining States"=w97:string, "Current State"=w80:string, "Arguments"=w96:string)  [unwired: 11 in]
    n31 = call "SaveCurrentState.vi"("error in (no error)"=w79, "Current State"=w80, "Byte Stream File in"=w81) -> ("error out"=w78:errorcluster)  [unwired: 8 in]
    n32 = case shown="\"USBCAM: Init\"" w80 {
      selector: w80 -> [_ _ _ _ _ _ _ _ _ _ _ _ _ _ _ _ _ _ _ _ _ _ _ _ w1090 _ _ _ _ _ _ _ _ _ _ _ _ _ _ _ _ _ _ _ _ _ _ _ _ _ _ _ _ _ _ _ _ _ _ _ _ _ _ _ _ _ _ _ _ _ _ _ _ _ _ _ _ _ _ _ _ _ _ _ _ _ _ _ _ _ _ _ _ _ _ _ _ _ _ _ _ _ _ _ _ _ _ _ _ _ _ _ _ _ _ _ _ _ _ _ _ _ _ _ _ _ _ _ _ _ _ _ _ _ _ _ _ _ _ _ _ _ _ _ _ _ _ _ _ _ _ _ _ _ _ _ _ _ _ _ _ _ _ _ _ _ _ _ _ _ _ _ _ _ _ _ _ _ _ _ _ _ _ _ _ _ _ _ _ _ _]
      tunnel: w97 -> [w107 w523 w532 w538 w544 w566 w579 w624 w630 w657 w676 w747 w762 w793 w820 w852 w866 w895 w909 w994 w1031 w1070 w1083 w1088 w1094 w1122 w1130 w1153 w1158 w1171 w1190 w1218 w1246 w1284 w1289 w1295 w1319 w1343 w1367 w1391 w1396 w1413 w1460 w1482 w1498 w1513 w1533 w1538 w1550 w1579 w1605 w1617 w1655 w1668 w1674 w1685 w1697 w1728 w1741 w1755 w1770 w1789 w1824 w1829 w1843 w1853 w1869 w1881 w1893 w1921 w1936 w1941 w1953 w1967 w1972 w1980 w1988 w1997 w2006 w2011 w2019 w2028 w2046 w2063 w2083 w2094 w2116 w2131 w2148 w2153 w2161 w2169 w2174 w2182 w2189 w2197 w2204 w2214 w2242 w2250 w2257 w2265 w2270 w2278 w2285 w2291 w2300 w2316 w2321 w2328 w2340 w2410 w2422 w2431 w2448 w2457 w2480 w2497 w2508 w2521 w2546 w2569 w2575 w2591 w2613 w2621 w2627 w2632 w2639 w2649 w2661 w2670 w2675 w2687 w2692 w2702 w2708 w2714 w2719 w2724 w2729 w2739 w2763 w2784 w2789 w2800 w2825 w2852 w2875 w2880 w2895 w2946 w2992 w3037 w3048 w3066 w3086 w3100 w3113 w3121 w3138 w3160 w3184 w3203 w3221 w3239 w3257 w3271 w3285 w3304 w3318 w3333 w3348 w3357 w3362 w3373 w3385 w3406 w3420 w3428 w3439 w3444 w3451 w3475 w3482 w3501 w3515 w3523 w3550 w3559 w3564]
      tunnel: w96 -> [_ _ _ _ _ _ _ _ _ _ _ _ _ _ _ _ _ _ _ _ _ _ _ _ _ _ _ _ _ _ _ _ _ _ _ _ _ _ _ _ _ _ _ _ _ _ _ _ _ _ _ _ _ _ _ _ w1695 _ _ _ _ _ _ _ _ _ _ _ _ _ _ _ _ _ _ _ _ _ _ _ _ _ _ _ _ _ _ _ _ _ _ _ _ _ _ _ _ w2205 _ _ _ _ _ _ _ _ _ _ _ w2323 w2334 _ _ _ _ w2454 _ _ _ _ _ w2565 _ _ _ _ _ _ w2634 _ _ _ _ _ _ w2698 _ _ _ _ _ _ _ _ _ _ _ _ _ _ _ _ _ _ _ _ _ _ _ _ _ _ _ _ _ _ _ _ _ _ _ _ _ _ _ _ _ _ _ _ _ _ _ _ _ _ _ _ _ _ _]
      tunnel: w92 -> [w105 w520 w528 w535 w541 w563 w576 _ w626 w653 w672 w744 w753 w790 w812 w843 w863 w892 w906 w955 w1023 w1058 w1078 w1085 w1092 w1115 w1127 w1151 w1155 w1159 w1180 w1210 w1238 w1280 w1286 w1292 w1300 w1324 w1349 w1373 w1393 w1406 w1450 w1479 w1483 w1510 w1530 w1535 w1539 w1568 w1595 w1610 w1638 w1666 w1671 w1678 w1693 w1711 w1736 w1747 w1765 w1782 w1807 w1826 w1839 w1847 w1866 w1878 w1890 w1909 w1925 w1938 w1951 w1965 w1969 w1974 w1981 w1993 w2002 w2008 w2015 w2025 w2033 w2050 w2078 w2084 w2113 w2124 w2146 w2150 w2154 w2162 w2171 w2180 w2186 w2194 w2201 w2211 w2239 w2247 w2254 w2262 w2267 w2272 w2283 w2288 w2294 w2313 w2318 w2326 w2336 w2407 w2412 w2425 w2446 w2455 w2470 w2494 w2505 w2515 w2539 w2566 w2572 w2584 w2609 w2618 w2624 w2629 w2636 w2643 w2657 w2667 w2672 w2684 w2689 w2695 w2705 w2711 w2716 w2721 w2726 w2736 w2761 w2782 w2786 w2798 w2823 w2850 w2873 w2877 w2888 w2940 w2988 w3034 w3044 w3061 w3081 w3095 w3109 w3115 w3133 w3155 w3179 w3198 w3216 w3234 w3252 w3266 w3280 w3299 w3313 w3328 w3345 w3355 w3359 w3367 w3383 w3398 w3412 w3426 w3436 w3442 w3449 w3461 w3479 w3490 w3502 w3519 w3548 w3551 w3561]
      tunnel: [w98 w521 w530 w536 w542 w564 w577 w622 w628 w649 w668 w721 w749 w791 w800 w832 w856 w883 w907 w931 w1020 w1057 w1079 w1086 w1096 w1119 errorcluster {"status"=FALSE, "code"=0, "source"=""} ("error out") w1150 w1156 w1169 w1188 w1202 w1225 w1282 w1287 w1293 w1301 w1325 w1350 w1374 w1394 w1397 w1442 w1473 w1487 w1511 w1521 w1536 w1542 w1566 w1594 w1609 w1625 w1660 w1672 w1683 w1687 w1702 w1731 w1743 w1761 w1781 w1798 w1827 w1831 w1849 w1864 w1876 w1888 w1911 w1926 w1939 w1943 w1962 w1970 w1978 w1986 w1990 w1999 w2009 w2012 w2021 w2036 w2058 w2077 w2088 w2106 w2128 w2144 w2151 w2159 w2167 w2172 w2179 w2187 w2195 w2202 w2212 w2240 w2248 w2255 w2263 w2268 w2276 w2282 w2289 w2297 w2314 w2319 w2324 w2337 w2408 w2416 w2428 w2438 w2451 w2471 w2495 w2504 w2517 w2541 w2567 w2573 w2581 w2603 w2619 w2625 w2630 w2637 w2647 w2659 w2668 w2673 w2685 w2690 w2700 w2706 w2712 w2717 w2722 w2727 w2737 w2751 w2775 w2787 w2791 w2810 w2842 w2867 w2878 w2882 w2941 w2989 w3035 w3043 w3063 w3083 w3097 w3111 w3117 w3135 w3157 w3181 w3200 w3218 w3236 w3254 w3268 w3282 w3301 w3315 w3329 w3346 w3353 w3360 w3364 w3374 w3400 w3414 w3422 w3435 w3440 w3446 w3455 w3477 w3498 w3512 w3518 w3545 w3556 w3562] -> w77
      tunnel: w78 -> [w104 w521 w530 w536 w542 w564 w577 w622 w628 w650 w666 w721 w748 w791 w801 w839 w856 w873 w907 w931 w1021 w1060 w1080 w1086 w1095 w1119 w1123 w1150 w1156 w1169 w1188 w1201 w1237 w1282 w1287 w1293 w1305 w1329 w1354 w1378 w1394 w1404 w1445 w1472 w1486 w1511 w1523 w1536 w1541 w1567 w1585 w1615 w1636 w1659 w1672 w1680 w1690 w1701 w1730 w1746 w1760 w1780 w1797 w1827 w1837 w1850 w1863 w1875 w1887 w1910 w1927 w1939 w1942 w1955 w1970 w1978 w1986 w1989 w1998 w2009 w2013 w2022 w2041 w2057 w2076 w2087 w2112 w2127 w2143 w2151 w2159 w2167 w2172 w2179 w2187 w2195 w2202 w2212 w2240 w2248 w2255 w2263 w2268 w2276 w2282 w2289 w2297 w2314 w2319 w2325 w2338 w2408 w2417 w2427 w2434 w2450 w2472 w2495 w2504 w2512 w2544 w2567 w2573 w2586 w2602 w2619 w2625 w2630 w2637 w2647 w2659 w2668 w2673 w2685 w2690 w2700 w2706 w2712 w2717 w2722 w2727 w2737 w2750 w2774 w2787 w2790 w2809 w2832 w2858 w2878 _ w2942 w2989 w3035 w3042 w3062 w3082 w3096 w3111 w3116 w3134 w3156 w3180 w3199 w3217 w3235 w3253 w3267 w3281 w3300 w3314 w3327 w3346 w3352 w3360 w3368 w3381 w3399 w3413 w3421 w3434 w3440 w3445 w3459 w3476 w3498 w3512 w3517 w3544 w3556 w3562]
      tunnel: [w106 w522 w531 w537 w543 w565 w578 w623 w629 w656 w675 w746 w761 w792 w819 w851 w865 w894 w908 w993 w1030 w1069 w1082 w1087 w1093 w1121 w1129 w1152 w1157 w1170 w1189 w1217 w1245 w1283 w1288 w1294 w1318 w1342 w1366 w1390 w1395 w1412 w1459 w1481 w1497 w1512 w1532 w1537 w1549 w1578 w1604 w1616 w1654 w1667 w1673 w1684 w1696 w1727 w1740 w1754 w1769 w1788 w1823 w1828 w1842 w1852 w1868 w1880 w1892 w1920 w1935 w1940 w1952 w1966 w1971 w1979 w1987 w1996 w2005 w2010 w2018 w2027 w2045 w2062 w2082 w2093 w2115 w2130 w2147 w2152 w2160 w2168 w2173 w2181 w2188 w2196 w2203 w2213 w2241 w2249 w2256 w2264 w2269 w2277 w2284 w2290 w2299 w2315 w2320 w2327 w2339 w2409 w2421 w2430 w2447 w2456 w2479 w2496 w2507 w2520 w2545 w2568 w2574 w2590 w2612 w2620 w2626 w2631 w2638 w2648 w2660 w2669 w2674 w2686 w2691 w2701 w2707 w2713 w2718 w2723 w2728 w2738 w2762 w2783 w2788 w2799 w2824 w2851 w2874 w2879 w2894 w2945 w2991 w3036 w3047 w3065 w3085 w3099 w3112 w3120 w3137 w3159 w3183 w3202 w3220 w3238 w3256 w3270 w3284 w3303 w3317 w3332 w3347 w3356 w3361 w3372 w3384 w3405 w3419 w3427 w3438 w3443 w3450 w3474 w3481 w3500 w3514 w3522 w3549 w3558 w3563] -> w94
      tunnel: [_ _ _ _ _ _ _ _ _ _ _ _ _ _ _ _ _ _ _ _ _ _ _ _ _ _ _ TRUE _ _ _ _ _ _ _ _ _ _ _ _ _ _ _ _ _ _ _ _ _ _ _ _ _ _ _ _ _ _ _ _ _ _ _ _ _ _ _ _ _ _ _ _ _ _ _ _ _ _ _ _ _ _ _ _ _ _ _ _ _ _ _ _ _ _ _ _ _ _ _ _ _ _ _ _ _ _ _ _ _ _ _ _ _ _ _ _ _ _ _ _ _ _ _ _ _ _ _ _ _ _ _ _ _ _ _ _ _ _ _ _ _ _ _ _ _ _ _ _ _ _ _ _ _ _ _ _ _ _ _ _ _ _ _ _ _ _ _ _ _ _ _ _ _ _ _ _ _ _ _ _ _ _ _ _ _ _ _ _ _ _ _] -> w85
      tunnel: [w103 w520 w528 w535 w541 w563 w576 w597 w626 w653 w672 w744 w753 w790 w812 w843 w863 w892 w906 w955 w1024 w1059 w1078 w1085 w1092 w1120 w1127 w1151 w1155 w1160 w1181 w1211 w1239 w1281 w1286 w1292 w1300 w1324 w1349 w1373 w1393 w1406 w1451 w1479 w1484 w1510 w1531 w1535 w1540 w1568 w1595 w1614 w1638 w1666 w1671 w1681 w1693 w1711 w1736 w1747 w1765 w1782 w1807 w1826 w1840 w1847 w1866 w1878 w1890 w1909 w1925 w1938 w1951 w1965 w1969 w1975 w1982 w1994 w2003 w2008 w2016 w2026 w2034 w2056 w2065 w2089 w2114 w2125 w2146 w2150 w2155 w2163 w2171 w2180 w2186 w2194 w2201 w2211 w2239 w2247 w2254 w2262 w2267 w2272 w2283 w2288 w2294 w2313 w2318 w2326 w2336 w2407 w2413 w2426 w2446 w2455 w2470 w2494 w2505 w2516 w2540 w2566 w2572 w2585 w2609 w2618 w2624 w2629 w2636 w2644 w2657 w2667 w2672 w2684 w2689 w2695 w2705 w2711 w2716 w2721 w2726 w2736 w2761 w2782 w2786 w2798 w2823 w2850 w2873 w2877 w2893 w2939 w2988 w3034 w3044 w3061 w3081 w3095 w3109 w3115 w3133 w3155 w3179 w3198 w3216 w3234 w3252 w3266 w3280 w3299 w3313 w3330 w3345 w3355 w3359 w3367 w3383 w3398 w3412 w3426 w3436 w3442 w3449 w3462 w3479 w3490 w3503 w3519 w3548 w3551 w3561] -> w93
      tunnel: 30 ("Timeout") -> [w102 _ _ _ _ _ _ _ _ _ _ _ _ _ _ _ _ _ _ _ _ _ _ _ _ _ _ _ _ _ _ _ _ _ _ _ _ _ _ _ _ _ _ _ _ _ _ _ _ _ _ _ _ _ _ _ _ _ _ _ _ _ _ _ _ _ _ _ _ _ _ _ _ _ _ _ _ _ _ _ _ _ _ _ _ _ _ _ _ _ _ _ _ _ _ _ _ _ _ _ _ _ _ _ _ _ _ _ _ _ _ _ _ _ _ _ _ _ _ _ _ _ _ _ _ _ _ _ _ _ _ _ _ _ _ _ _ _ _ _ _ _ _ _ _ _ _ _ _ _ _ _ _ _ _ _ _ _ _ _ _ _ _ _ _ _ _ _ _ _ _ _ _ _ _ _ _ _ _ _ _ _ _ _ _ _ _ _ _ _ _]
      tunnel: w90 -> [_ _ _ _ _ _ _ _ _ _ _ _ _ _ _ _ _ _ _ _ w1028 _ _ _ _ _ _ _ _ _ _ _ _ _ _ _ _ _ _ _ _ _ _ _ _ _ _ _ _ _ _ _ _ _ _ _ _ _ _ _ _ _ _ _ _ _ _ _ _ _ _ _ w1948 w1961 _ _ _ _ _ _ _ _ _ _ _ _ _ _ _ _ _ _ _ _ _ _ _ _ _ _ _ _ _ _ _ _ _ _ _ _ _ _ _ _ _ _ _ _ _ _ _ _ _ _ _ _ _ _ _ _ _ _ _ _ _ _ _ _ _ _ _ _ _ _ _ _ _ _ _ _ _ _ _ _ _ _ _ _ _ _ _ _ _ _ _ _ _ _ _ _ _ _ _ _ _ _ _ _ _ _ _ _ _ _ _ _ _ _ _ _ _]
      tunnel: w89 -> [_ _ _ _ _ _ _ _ _ _ _ _ _ _ _ _ _ _ _ _ w1027 _ _ _ _ _ _ _ _ _ _ _ _ _ _ _ _ _ _ _ _ _ _ _ _ _ _ _ _ _ _ _ _ _ _ _ _ _ _ _ _ _ _ _ _ _ _ _ _ _ _ _ w1949 w1960 _ _ _ _ _ _ _ _ _ _ _ _ _ _ _ _ _ _ _ _ _ _ _ _ _ _ _ _ _ _ _ _ _ _ _ _ _ _ _ _ _ _ _ _ _ _ _ _ _ _ _ _ _ _ _ _ _ _ _ _ _ _ _ _ _ _ _ _ _ _ _ _ _ _ _ _ _ _ _ _ _ _ _ _ _ _ _ _ _ _ _ _ _ _ _ _ _ _ _ _ _ _ _ _ _ _ _ _ _ _ _ _ _ _ _ _ _]
      tunnel: w88 -> [w101 _ _ _ _ _ _ _ _ _ _ _ _ _ _ _ _ _ _ _ _ _ _ _ _ _ _ _ _ _ _ _ _ _ _ _ _ _ _ _ _ _ _ w1475 _ _ _ _ _ _ _ _ _ _ _ _ _ _ _ _ _ _ _ _ _ _ _ _ _ _ _ _ _ _ _ _ _ _ _ _ _ _ _ _ _ _ _ _ _ _ _ _ _ _ _ _ _ _ _ _ _ _ _ _ _ _ _ _ _ _ _ _ _ _ _ _ _ _ _ _ _ _ _ _ _ _ _ _ _ _ _ _ _ _ _ _ _ _ _ _ _ _ _ _ _ _ _ _ _ _ _ _ _ _ _ _ _ _ _ _ _ _ _ _ _ _ _ _ _ _ _ _ _ _ _ _ _ _ _ _ _ _ _ _ _ _ _ _ _ _ _]
      tunnel: w87 -> [w100 w519 w529 w534 w540 w555 w575 w607 w627 w655 w674 w745 w760 w789 w818 w850 w864 w893 w905 w992 w1029 w1068 w1077 w1084 w1089 w1107 w1126 w1149 w1154 w1168 w1187 w1216 w1236 w1279 w1285 w1291 w1299 w1323 w1348 w1372 w1392 w1401 w1425 w1480 w1496 w1509 w1518 w1534 w1548 w1577 w1603 w1608 w1653 w1658 w1670 w1677 w1686 w1698 w1729 w1745 w1759 w1779 w1794 w1825 w1841 w1851 w1867 w1879 w1891 w1919 w1922 w1937 w1950 w1959 w1968 w1977 w1985 w1992 w2001 w2007 w2017 w2020 w2032 w2051 w2066 w2085 w2111 w2129 w2145 w2149 w2157 w2165 w2170 w2178 w2185 w2193 w2200 w2210 w2238 w2246 w2253 w2258 w2266 w2275 w2281 w2287 w2296 w2308 w2317 w2322 w2333 w2406 w2411 w2423 w2433 w2449 w2478 w2493 w2506 w2518 w2542 w2562 w2570 w2583 w2611 w2616 w2622 w2628 w2635 w2646 w2658 w2666 w2671 w2683 w2688 w2699 w2704 w2710 w2715 w2720 w2725 w2735 w2760 w2781 w2785 w2797 w2822 w2849 w2872 w2876 w2892 w2944 w2990 w3031 w3046 w3064 w3084 w3098 w3110 w3119 w3136 w3158 w3182 w3201 w3219 w3237 w3255 w3269 w3283 w3302 w3316 w3331 w3344 w3354 w3358 w3371 w3382 w3404 w3418 w3425 w3437 w3441 w3448 w3473 w3480 w3499 w3513 w3521 w3547 w3557 w3560]
      tunnel: [w99 w519 w529 w534 w540 w555 w575 w607 w627 w655 w674 w745 w760 w789 w818 w850 w864 w893 w905 w992 w1029 w1068 w1077 w1084 w1089 w1107 w1126 w1149 w1154 w1168 w1187 w1216 w1236 w1279 w1285 w1291 w1299 w1323 w1348 w1372 w1392 w1401 w1425 w1480 w1496 w1509 w1518 w1534 w1548 w1577 w1603 w1608 w1653 w1658 w1670 w1677 w1686 w1698 w1729 w1745 w1759 w1779 w1794 w1825 w1841 w1851 w1867 w1879 w1891 w1919 w1922 w1937 w1950 w1959 w1968 w1977 w1985 w1992 w2001 w2007 w2017 w2020 w2032 w2051 w2066 w2085 w2111 w2129 w2145 w2149 w2157 w2165 w2170 w2178 w2185 w2193 w2200 w2210 w2238 w2246 w2253 w2258 w2266 w2275 w2281 w2287 w2296 w2308 w2317 w2322 w2333 w2406 w2411 w2423 w2433 w2449 w2478 w2493 w2506 w2518 w2542 w2562 w2570 w2583 w2611 w2616 w2622 w2628 w2635 w2646 w2658 w2666 w2671 w2683 w2688 w2699 w2704 w2710 w2715 w2720 w2725 w2735 w2760 w2781 w2785 w2797 w2822 w2849 w2872 w2876 w2892 w2944 w2990 w3031 w3046 w3064 w3084 w3098 w3110 w3119 w3136 w3158 w3182 w3201 w3219 w3237 w3255 w3269 w3283 w3302 w3316 w3331 w3344 w3354 w3358 w3371 w3382 w3404 w3418 w3425 w3437 w3441 w3448 w3473 w3480 w3499 w3513 w3521 w3547 w3557 w3560] -> w86
      tunnel: w82 -> [_ _ _ _ _ _ _ _ _ _ _ _ _ _ _ _ _ _ _ _ w1022 _ _ _ _ _ _ _ _ _ _ _ _ _ _ _ _ _ _ _ _ _ _ _ _ _ _ _ _ _ _ _ _ _ _ _ _ _ _ _ _ _ _ _ _ _ _ _ _ _ _ _ w1947 w1958 _ _ _ _ _ _ _ _ _ _ _ _ _ _ _ _ _ _ _ _ _ _ _ _ _ _ _ _ _ _ _ _ _ _ _ _ _ _ _ _ _ _ _ _ _ _ _ _ _ _ _ _ _ _ _ _ _ _ _ _ _ _ _ _ _ _ _ _ _ _ _ _ _ _ _ _ _ _ _ _ _ _ _ _ _ _ _ _ _ _ _ _ _ _ _ _ _ _ _ _ _ _ _ _ _ _ _ _ _ _ _ _ _ _ _ _ _]
      tunnel: w76 -> [_ _ _ _ _ _ _ _ _ _ _ _ _ _ _ _ _ _ _ _ _ _ _ _ _ _ _ _ _ _ _ _ _ _ _ _ _ _ _ _ _ _ _ _ _ _ _ _ _ _ _ _ _ _ _ _ _ _ _ _ _ _ _ _ _ _ _ _ _ _ _ _ _ _ _ _ _ _ _ _ _ _ _ _ _ _ _ _ _ _ _ _ _ _ _ _ _ _ _ _ _ _ _ _ _ _ _ _ _ _ _ _ _ _ _ _ _ _ _ _ _ _ _ _ _ _ _ _ _ _ _ _ _ _ _ _ _ _ _ _ _ _ _ _ _ _ _ _ _ _ _ _ _ _ _ _ _ _ _ _ _ _ _ _ _ _ _ _ _ _ _ _ _ _ _ _ _ w3401 w3415 _ _ _ _ _ _ _ _ _ _ _ _]
      tunnel: w75 -> [_ _ _ _ _ _ _ _ _ _ _ _ _ _ _ _ _ _ _ _ _ _ _ _ _ _ _ _ _ _ _ _ _ _ _ _ _ _ _ _ _ _ _ _ _ _ _ _ _ _ _ _ _ _ _ _ _ _ _ _ _ _ _ _ _ _ _ _ _ _ _ _ _ w1956 _ _ _ _ _ _ _ _ _ _ _ _ _ _ _ _ _ _ _ _ _ _ _ _ _ _ _ _ _ _ _ _ _ _ _ _ _ _ _ _ _ _ _ _ _ _ _ _ _ _ _ _ _ _ _ _ _ _ _ _ _ _ _ _ _ _ _ _ _ _ _ _ _ _ _ _ _ _ _ _ _ _ _ _ _ _ _ _ _ _ _ _ _ _ _ _ _ _ _ _ _ _ _ _ _ _ _ _ _ _ _ _ _ _ w3546 _ _]
      frame "", "Event Structure", "Idle" {
        # "executes when the state queue is empty"
        n33 = event shown="[37] <AcqLoop error?>: User Event" {
          selector: w100 -> [_ _ _ _ _ _ _ _ _ _ _ _ _ _ _ _ _ _ _ _ _ _ _ _ _ _ _ _ _ _ _ _ _ _ _ _ _ _ _]
          dyn-events: [_ _ _ _ _ _ _ _ _ _ _ _ _ _ _ _ _ _ _ _ _ _ _ _ _ _ _ _ _ _ _ _ _ _ _ _ _ _ _] -> w99
          timeout: w102 -> [_ _ _ _ _ _ _ _ _ _ _ _ _ _ _ _ _ _ _ _ _ _ _ _ _ _ _ _ _ _ _ _ _ _ _ _ _ _ _]
          tunnel: w107 -> [w127 w145 w154 w162 w166 w170 w178 w184 w192 w200 w210 w217 w246 w266 w286 w306 w310 w317 w340 w354 w368 w382 w387 w390 w396 w403 w410 w416 w422 w428 w435 w448 w459 w471 w478 w482 w486 w502 w518]
          tunnel: [w128 w144 w154 w161 w166 w169 w178 w184 w192 w200 w210 w216 w246 w266 w286 w306 w310 w316 w340 w354 w368 w382 w386 w389 w396 w404 w411 w415 w421 w428 w436 w449 w459 w472 w478 w482 w485 w503 w517] -> w106
          tunnel: w105 -> [w111 w147 w152 w156 w164 w171 w177 w185 w193 w201 w208 w212 w244 w264 w284 w304 w308 w312 w339 w353 w367 w381 w383 w391 w394 w399 w406 w418 w423 w426 w430 w443 w457 w467 w476 w480 w487 w500 w515]
          tunnel: [w126 w148 w153 w157 w165 w172 w176 w183 w191 w199 w209 w218 w245 w265 w285 w305 w309 w318 w337 w341 w364 w379 w385 w392 w395 w400 w407 w419 w424 w427 w434 w447 w458 w468 w477 w481 w488 w504 w516] -> w98
          tunnel: w104 -> [w126 w148 w153 w157 w165 w172 w176 w183 w191 w199 w209 w218 w245 w265 w285 w305 w309 w318 w334 w343 w355 w371 w385 w392 w395 w400 w407 w419 w424 w427 w434 w447 w458 w470 w477 w481 w488 w504 w516]
          tunnel: [w111 w147 w152 w156 w164 w171 w177 w185 w193 w201 w208 w213 w244 w264 w284 w304 w308 w313 w339 w353 w367 w381 w383 w391 w394 w401 w408 w418 w423 w426 w431 w444 w457 w473 w476 w480 w487 w501 w515] -> w103
          tunnel: w101 -> [_ _ _ _ _ _ _ _ _ _ _ _ _ _ _ _ _ _ _ _ _ _ _ _ _ _ _ _ _ _ _ _ _ _ _ _ _ _ _]
          event Timeout {
            # "check system status every 2s"
            n34 = event-data() -> ()  [unwired: 1 in, 1 out]
            n35 = Unbundle By Name(w111) -> ("SysRunning?"=w109:bool, "SlowTimer"=w125:u32, "FastTimer"=w119:u32)
            n36 = Tick Count (ms)() -> (millisecond timer value=w112:u32)
            n37 = Subtract(x=w112, y=w125) -> (x-y=w122:u32)
            n38 = case shown="False" w109 {
              tunnel: ["" "Utility: AquiTimerCheck" ("State(s) in Front (\"\")")] -> w117
              frame False {
                # "if not running, do nothing"
              }
              frame True {
                # "if aquisition is running, check timer"
              }
            }
            n39 = Subtract(x=w112, y=w119) -> (x-y=w120:u32)
            n40 = Greater?(x=w122, y=u32 2000) -> (0:w123:bool)
            n41 = Greater?(x=w120, y=u32 500) -> (0:w110:bool)
            n42 = disable-structure shown="Disabled" {
              disable-tunnel: w110 -> [w133 _]
              disable-tunnel: w109 -> [w132 _]
              disable-tunnel: [w129 "" ("State(s) at Back (\"\")")] -> w108
              frame Disabled {
                n43 = Not(x=w132) -> (.not. x?=w131:bool)
                n44 = And(x=w133, y=w131) -> (x .and. y?=w130:bool)
                n45 = case shown="True" w130 {
                  tunnel: ["" ("Empty String Constant") "TCP: checkSource" ("State(s) in Front (\"\")")] -> w129
                  frame False {
                  }
                  frame True {
                  }
                }
              }
              frame Enabled {
              }
            }
            n46 = case shown="True" w123 {
              tunnel: ["" ("Empty String Constant") "SystemStatus: SlowSysStatusMacro" ("State(s) in Front (\"\")")] -> w115
              frame False {
              }
              frame True {
              }
            }
            n47 = case shown="True" w110 {
              tunnel: ["" ("Empty String Constant") "SystemStatus: FastSysStatusMacro" ("State(s) in Front (\"\")")] -> w113
              frame False {
              }
              frame True {
              }
            }
            n48 = call <vilib>:"Add State(s) to Queue__JKI_lib_State_Machine.vi"("State(s) in Front (\"\")"=w117, "State(s) in (\"\")"="LabJack: checkPedal" ("State(s) in Front (\"\")"), "State(s) at Back (\"\")"=w115) -> ("States Out"=w114:string)  [unwired: 12 in]
            n49 = call <vilib>:"Add State(s) to Queue__JKI_lib_State_Machine.vi"("State(s) in Front (\"\")"=w114, "State(s) in (\"\")"=w113, "State(s) at Back (\"\")"=w108) -> ("States Out"=w118:string)  [unwired: 12 in]
            n50 = call <vilib>:"Add State(s) to Queue__JKI_lib_State_Machine.vi"("State(s) in Front (\"\")"=w118, "State(s) in (\"\")"=w127) -> ("States Out"=w128:string)  [unwired: 13 in]
          }
          event "Live?": Value Change {
            n51 = event-data() -> ("NewVal"=w146:bool)  [unwired: 1 in, 5 out]
            n52 = case shown="True" w146 {
              tunnel: ["USBCAM: Stop" "USBCAM: StartNoSave"] -> w143
              frame False {
              }
              frame True {
              }
            }
            n53 = call <vilib>:"Add State(s) to Queue__JKI_lib_State_Machine.vi"("State(s) in Front (\"\")"=w143, "State(s) in (\"\")"=w145) -> ("States Out"=w144:string)  [unwired: 13 in]
          }
          event "355nm Laser toggle": Mouse Enter {
            n54 = event-data() -> ()  [unwired: 1 in, 4 out]
            n55 = local write "Help"("Toggle 355nm laser." ("Help")) -> ()
          }
          event "355nm Laser toggle": Value Change {
            # "[Covers: REQ34]"
            n56 = event-data() -> ()  [unwired: 1 in, 6 out]
            n57 = Select(t="LabJack: 355_PWM_Start\nLabJack: AB_Start", s="355nm Laser toggle", f="LabJack: 355_PWM_Stop\nLabJack: AB_Stop") -> (s? t:f=w159:string)
            n58 = call <vilib>:"Add State(s) to Queue__JKI_lib_State_Machine.vi"("State(s) in Front (\"\")"=w159, "State(s) in (\"\")"=w162) -> ("States Out"=w161:string)  [unwired: 13 in]
          }
          event "Aiming beam toggle": Mouse Enter {
            n59 = event-data() -> ()  [unwired: 1 in, 4 out]
            n60 = local write "Help"("Toggle aiming beam laser." ("Help")) -> ()
          }
          event "Aiming beam toggle": Value Change {
            # "[Covers: REQ33]"
            n61 = event-data() -> ()  [unwired: 1 in, 6 out]
            n62 = case shown="True" "Aiming beam toggle" {
              tunnel: ["LabJack: AB_Stop" ("State(s) in Front (\"\")") "LabJack: AB_Start" ("State(s) in Front (\"\")")] -> w168
              frame False {
              }
              frame True {
              }
            }
            n63 = call <vilib>:"Add State(s) to Queue__JKI_lib_State_Machine.vi"("State(s) in Front (\"\")"=w168, "State(s) in (\"\")"=w170) -> ("States Out"=w169:string)  [unwired: 13 in]
          }
          event "Auto gain ch1": Value Change {
            n64 = event-data() -> ("NewVal"=w175:bool)  [unwired: 1 in, 5 out]
            n65 = case shown="True" w175 {
              frame False {
                n66 = local read "V 1"() -> (w179:dbl)
                n67 = call "V1FGV.vi"("action (write)"=enum16{"write", "read"}."write" ("action"), "V1 in"=w179) -> ()  [unwired: 8 in, 2 out]
                n68 = property on="V 1" class="DigNum (strict)"("DisabledEnum"=T14."Enabled" ("Disabled")) -> ()  [unwired: 2 in, 2 out]
              }
              frame True {
                n69 = property on="V 1" class="DigNum (strict)"("DisabledEnum"=T14."Disabled and Grayed Out" ("Disabled")) -> ()  [unwired: 2 in, 2 out]
              }
            }
          }
          event "Auto gain ch2": Value Change {
            n70 = event-data() -> ("NewVal"=w186:bool)  [unwired: 1 in, 5 out]
            n71 = case shown="False" w186 {
              frame False {
                n72 = local read "V 2"() -> (w187:dbl)
                n73 = property on="V 2" class="DigNum (strict)"("DisabledEnum"=T14."Enabled" ("Disabled")) -> ()  [unwired: 2 in, 2 out]
                n74 = call "V2FGV.vi"("action(write)"=enum16{"write", "read"}."write" ("action"), "V2 in"=w187) -> ()  [unwired: 8 in, 2 out]
              }
              frame True {
                n75 = property on="V 2" class="DigNum (strict)"("DisabledEnum"=T14."Disabled and Grayed Out" ("Disabled")) -> ()  [unwired: 2 in, 2 out]
              }
            }
          }
          event "Auto gain ch3": Value Change {
            n76 = event-data() -> ("NewVal"=w194:bool)  [unwired: 1 in, 5 out]
            n77 = case shown="False" w194 {
              frame False {
                n78 = local read "V 3"() -> (w195:dbl)
                n79 = property on="V 3" class="DigNum (strict)"("DisabledEnum"=T14."Enabled" ("Disabled")) -> ()  [unwired: 2 in, 2 out]
                n80 = call "V3FGV.vi"("action(write)"=enum16{"write", "read"}."write" ("action"), "V3 in"=w195) -> ()  [unwired: 8 in, 2 out]
              }
              frame True {
                n81 = property on="V 3" class="DigNum (strict)"("DisabledEnum"=T14."Disabled and Grayed Out" ("Disabled")) -> ()  [unwired: 2 in, 2 out]
              }
            }
          }
          event "Auto gain ch4": Value Change {
            n82 = event-data() -> ("NewVal"=w202:bool)  [unwired: 1 in, 5 out]
            n83 = case shown="False" w202 {
              frame False {
                n84 = local read "V 4"() -> (w203:dbl)
                n85 = property on="V 4" class="DigNum (strict)"("DisabledEnum"=T14."Enabled" ("Disabled")) -> ()  [unwired: 2 in, 2 out]
                n86 = call "V4FGV.vi"("action(write)"=enum16{"write", "read"}."write" ("action"), "V3 in"=w203) -> ()  [unwired: 8 in, 2 out]
              }
              frame True {
                n87 = property on="V 4" class="DigNum (strict)"("DisabledEnum"=T14."Disabled and Grayed Out" ("Disabled")) -> ()  [unwired: 2 in, 2 out]
              }
            }
          }
          event "Background": Mouse Enter {
            n88 = event-data() -> ()  [unwired: 1 in, 4 out]
            n89 = local write "Help"("Click to record a background." ("Help")) -> ()
          }
          event "Background": Value Change {
            n90 = event-data() -> ("NewVal"=w214:bool)  [unwired: 1 in, 5 out]
            n91 = case shown="True" w214 {
              tunnel: ["Utility: SetAllChanManualGain\nQueue: Flash\nUtility: Dewelling >> 2500\nLabJack: 355_PWM_Stop\nLabJack: AB_Stop" "Utility: SetDataClass >> Bg\nUI: Update\nLabJack: 355_PWM_Start\nLabJack: AB_Start\nUtility: SaveDeconChan\nUtility: Dewelling >> 50\nLabJack: SetV\nDigitizer: Start\nUtility: AquiTimerReset\nLED: BreathGreen\nUI: duringBGAcquire"] -> w215
              tunnel: [FALSE TRUE] -> w211
              frame False {
                n92 = local read "Skip Data Save?"() -> (w219:bool)
                n93 = case shown="False" w219 {
                  frame False {
                    n94 = property on="Background" class="Bool (strict)"("BoolText.Text"="Done!" ("Boolean Text.Text")) -> ()  [unwired: 2 in, 2 out]
                  }
                  frame True {
                  }
                }
              }
              frame True {
                # "[Covers: REQ6]"
                n95 = property on="Background" class="Bool (strict)"("BoolText.Text"="Running" ("Boolean Text.Text"), "Colors [4]"=cluster{u32, u32}[] [{6618880, 6618880}, {16711680, 16711680}]) -> ()  [unwired: 2 in, 2 out]
              }
            }
            n96 = Bundle By Name(cluster=w212, "SysRunning?"=w211) -> (w213:T29)
            n97 = call <vilib>:"Add State(s) to Queue__JKI_lib_State_Machine.vi"("State(s) in Front (\"\")"=w215, "State(s) in (\"\")"=w217) -> ("States Out"=w216:string)  [unwired: 13 in]
          }
          event "Channel 1": Cursor Move {
            n98 = event-data() -> ("CursIdx"=w230:i32, "CursLoc"=w242:cluster{"X":dbl, "Y":dbl})  [unwired: 1 in, 7 out]
            n99 = property on="Channel 3" class="WFGraph (strict)"() -> ("CrsrList"=w237:T30)  [unwired: 2 in, 2 out]
            n100 = property on="Channel 4" class="WFGraph (strict)"() -> ("CrsrList"=w229:T30)  [unwired: 2 in, 2 out]
            n101 = property on="Channel 2" class="WFGraph (strict)"() -> ("CrsrList"=w240:T30)  [unwired: 2 in, 2 out]
            n102 = Index Array(array=w237, index=w230) -> (element=w241:T31)
            n103 = Index Array(array=w229, index=w230) -> (element=w232:T31)
            n104 = Unbundle By Name(w242) -> ("X"=w231:dbl)
            n105 = Index Array(array=w240, index=w230) -> (element=w243:T31)
            n106 = Bundle By Name(cluster=w241, "Position.X"=w231) -> (w236:T31)
            n107 = Bundle By Name(cluster=w232, "Position.X"=w231) -> (w228:T31)
            n108 = Bundle By Name(cluster=w243, "Position.X"=w231) -> (w239:T31)
            n109 = control-ref of="Channel 1"() -> (w233:refnum<vi>)
            n110 = Replace Array Subset(array=w237, new element=w236, index=w230) -> (w235:T30)
            n111 = Replace Array Subset(array=w229, new element=w228, index=w230) -> (w227:T30)
            n112 = Replace Array Subset(array=w240, new element=w239, index=w230) -> (w238:T30)
            n113 = property on="Channel 3" class="WFGraph (strict)"("CrsrList"=w235) -> (error out=w234:errorcluster)  [unwired: 2 in, 1 out]
            n114 = property on="Channel 4" class="WFGraph (strict)"("CrsrList"=w227) -> ()  [unwired: 2 in, 2 out]
            n115 = property on="Channel 2" class="WFGraph (strict)"("CrsrList"=w238) -> ()  [unwired: 2 in, 2 out]
            n116 = call "UpdateCurserIdx(SubVI).vi"("error in (no error)"=w234, "WaveformGraph in"=w233) -> ()  [unwired: 9 in, 1 out]
          }
          event "Channel 2": Cursor Move {
            n117 = event-data() -> ("CursIdx"=w249:i32, "CursLoc"=w263:cluster{"X":dbl, "Y":dbl})  [unwired: 1 in, 7 out]
            n118 = Unbundle By Name(w263) -> ("X"=w251:dbl)
            n119 = property on="Channel 1" class="WFGraph (strict)"() -> ("CrsrList"=w257:T30)  [unwired: 2 in, 2 out]
            n120 = property on="Channel 3" class="WFGraph (strict)"() -> ("CrsrList"=w259:T30)  [unwired: 2 in, 2 out]
            n121 = property on="Channel 4" class="WFGraph (strict)"() -> ("CrsrList"=w250:T30)  [unwired: 2 in, 2 out]
            n122 = Index Array(array=w257, index=w249) -> (element=w262:T31)
            n123 = Index Array(array=w259, index=w249) -> (element=w261:T31)
            n124 = Index Array(array=w250, index=w249) -> (element=w252:T31)
            n125 = Bundle By Name(cluster=w252, "Position.X"=w251) -> (w248:T31)
            n126 = Bundle By Name(cluster=w262, "Position.X"=w251) -> (w260:T31)
            n127 = Bundle By Name(cluster=w261, "Position.X"=w251) -> (w258:T31)
            n128 = Replace Array Subset(array=w257, new element=w260, index=w249) -> (w256:T30)
            n129 = Replace Array Subset(array=w259, new element=w258, index=w249) -> (w255:T30)
            n130 = Replace Array Subset(array=w250, new element=w248, index=w249) -> (w247:T30)
            n131 = control-ref of="Channel 1"() -> (w254:refnum<vi>)
            n132 = property on="Channel 1" class="WFGraph (strict)"("CrsrList"=w256) -> ()  [unwired: 2 in, 2 out]
            n133 = property on="Channel 3" class="WFGraph (strict)"("CrsrList"=w255) -> (error out=w253:errorcluster)  [unwired: 2 in, 1 out]
            n134 = property on="Channel 4" class="WFGraph (strict)"("CrsrList"=w247) -> ()  [unwired: 2 in, 2 out]
            n135 = call "UpdateCurserIdx(SubVI).vi"("error in (no error)"=w253, "WaveformGraph in"=w254) -> ()  [unwired: 9 in, 1 out]
          }
          event "Channel 3": Cursor Move {
            n136 = event-data() -> ("CursIdx"=w269:i32, "CursLoc"=w283:cluster{"X":dbl, "Y":dbl})  [unwired: 1 in, 7 out]
            n137 = Unbundle By Name(w283) -> ("X"=w271:dbl)
            n138 = property on="Channel 4" class="WFGraph (strict)"() -> ("CrsrList"=w270:T30)  [unwired: 2 in, 2 out]
            n139 = property on="Channel 1" class="WFGraph (strict)"() -> ("CrsrList"=w280:T30)  [unwired: 2 in, 2 out]
            n140 = property on="Channel 2" class="WFGraph (strict)"() -> ("CrsrList"=w278:T30)  [unwired: 2 in, 2 out]
            n141 = Index Array(array=w270, index=w269) -> (element=w272:T31)
            n142 = Index Array(array=w280, index=w269) -> (element=w282:T31)
            n143 = Index Array(array=w278, index=w269) -> (element=w281:T31)
            n144 = Bundle By Name(cluster=w272, "Position.X"=w271) -> (w268:T31)
            n145 = Bundle By Name(cluster=w282, "Position.X"=w271) -> (w279:T31)
            n146 = Bundle By Name(cluster=w281, "Position.X"=w271) -> (w277:T31)
            n147 = Replace Array Subset(array=w270, new element=w268, index=w269) -> (w267:T30)
            n148 = Replace Array Subset(array=w280, new element=w279, index=w269) -> (w276:T30)
            n149 = Replace Array Subset(array=w278, new element=w277, index=w269) -> (w275:T30)
            n150 = control-ref of="Channel 1"() -> (w273:refnum<vi>)
            n151 = property on="Channel 4" class="WFGraph (strict)"("CrsrList"=w267) -> ()  [unwired: 2 in, 2 out]
            n152 = property on="Channel 1" class="WFGraph (strict)"("CrsrList"=w276) -> ()  [unwired: 2 in, 2 out]
            n153 = property on="Channel 2" class="WFGraph (strict)"("CrsrList"=w275) -> (error out=w274:errorcluster)  [unwired: 2 in, 1 out]
            n154 = call "UpdateCurserIdx(SubVI).vi"("error in (no error)"=w274, "WaveformGraph in"=w273) -> ()  [unwired: 9 in, 1 out]
          }
          event "Channel 4": Cursor Move {
            n155 = event-data() -> ("CursIdx"=w291:i32, "CursLoc"=w303:cluster{"X":dbl, "Y":dbl})  [unwired: 1 in, 7 out]
            n156 = Unbundle By Name(w303) -> ("X"=w289:dbl)
            n157 = property on="Channel 1" class="WFGraph (strict)"() -> ("CrsrList"=w301:T30)  [unwired: 2 in, 2 out]
            n158 = property on="Channel 2" class="WFGraph (strict)"() -> ("CrsrList"=w297:T30)  [unwired: 2 in, 2 out]
            n159 = property on="Channel 3" class="WFGraph (strict)"() -> ("CrsrList"=w292:T30)  [unwired: 2 in, 2 out]
            n160 = Index Array(array=w301, index=w291) -> (element=w302:T31)
            n161 = Index Array(array=w297, index=w291) -> (element=w298:T31)
            n162 = Index Array(array=w292, index=w291) -> (element=w294:T31)
            n163 = Bundle By Name(cluster=w302, "Position.X"=w289) -> (w300:T31)
            n164 = Bundle By Name(cluster=w298, "Position.X"=w289) -> (w296:T31)
            n165 = Bundle By Name(cluster=w294, "Position.X"=w289) -> (w293:T31)
            n166 = Replace Array Subset(array=w301, new element=w300, index=w291) -> (w299:T30)
            n167 = Replace Array Subset(array=w297, new element=w296, index=w291) -> (w295:T30)
            n168 = Replace Array Subset(array=w292, new element=w293, index=w291) -> (w290:T30)
            n169 = control-ref of="Channel 1"() -> (w287:refnum<vi>)
            n170 = call "UpdateCurserIdx(SubVI).vi"() -> ()  [unwired: 11 in, 1 out]
            n171 = call "UpdateCurserIdx(SubVI).vi"() -> ()  [unwired: 11 in, 1 out]
            n172 = property on="Channel 1" class="WFGraph (strict)"("CrsrList"=w299) -> ()  [unwired: 2 in, 2 out]
            n173 = property on="Channel 2" class="WFGraph (strict)"("CrsrList"=w295) -> ()  [unwired: 2 in, 2 out]
            n174 = property on="Channel 3" class="WFGraph (strict)"("CrsrList"=w290) -> (error out=w288:errorcluster)  [unwired: 2 in, 1 out]
            n175 = call "UpdateCurserIdx(SubVI).vi"("error in (no error)"=w288, "WaveformGraph in"=w287) -> ()  [unwired: 9 in, 1 out]
          }
          event "Cali&iRF alignment": Mouse Enter {
            n176 = event-data() -> ()  [unwired: 1 in, 4 out]
            n177 = local write "Help"("Click to run system intensity calibration and irf alignment" ("Help")) -> ()
          }
          event "Cali&iRF alignment": Value Change {
            n178 = event-data() -> ("NewVal"=w314:bool)  [unwired: 1 in, 5 out]
            n179 = case shown="False" w314 {
              tunnel: ["Utility: SetAllChanManualGain\nQueue: Flash\nUtility: Dewelling >> 2500\nLabJack: 355_PWM_Stop\nLabJack: AB_Stop" "Utility: SetDataClass >> Cali\nUI: Update\nUtility: SaveDeconChan\nLabJack: 355_PWM_Start\nLabJack: AB_Start\nLabJack: SetV\nDigitizer: Start\nUtility: AquiTimerReset\nLED: BreathGreen\nUI: duringIRFAlign"] -> w315
              tunnel: [FALSE TRUE] -> w311
              frame False {
                n180 = local read "Skip Data Save?"() -> (w319:bool)
                n181 = case shown="False" w319 {
                  frame False {
                    n182 = property on="Cali&iRF alignment" class="Bool (strict)"("BoolText.Text"="Done!" ("Boolean Text.Text")) -> ()  [unwired: 2 in, 2 out]
                  }
                  frame True {
                  }
                }
              }
              frame True {
                n183 = property on="Cali&iRF alignment" class="Bool (strict)"("BoolText.Text"="Running" ("Boolean Text.Text"), "Colors [4]"=cluster{u32, u32}[] [{6618880, 6618880}, {16711680, 16711680}]) -> ()  [unwired: 2 in, 2 out]
              }
            }
            n184 = Bundle By Name(cluster=w312, "SysRunning?"=w311) -> (w313:T29)
            n185 = call <vilib>:"Add State(s) to Queue__JKI_lib_State_Machine.vi"("State(s) in Front (\"\")"=w315, "State(s) in (\"\")"=w317) -> ("States Out"=w316:string)  [unwired: 13 in]
          }
          event "V 1": Value Change {
            n186 = event-data() -> ()  [unwired: 1 in, 6 out]
            n187 = call "LabJack_FGV.vi"("Operation(Read)"=enum16{"Write", "Read"}."Read" ("Operation"), "error in (no error)"=w334) -> ("error out"=w331:errorcluster, "Read data"=w332:i32)  [unwired: 8 in]
            n188 = global read "GlobalVariables.vi" "Ch1 LJ pin"() -> (w330:string)
            n189 = call "LJM_eWriteName.vi"("Handle In"=w332, "Name"=w330, "Value"="V 1", "error in"=w331) -> ("error out"=w328:errorcluster)  [unwired: 10 in, 1 out]
            n190 = call "V1FGV.vi"("Error In"=w328, "action (write)"=enum16{"write", "read"}."write" ("action"), "V1 in"="V 1") -> ("Error Out"=w327:errorcluster)  [unwired: 7 in, 1 out]
            n191 = call "CtrlVtoGain.vi"("error in (no error)"=w327, "CtrlV(V)"="V 1", "Channel"=enum16{"Ch1", "Ch2", "Ch3"}."Ch1" ("Enum")) -> ("error out"=w337:errorcluster, "Gain"=w336:dbl)  [unwired: 7 in]
            n192 = local write "Gain1"(w336) -> ()
          }
          event "V 2": Value Change {
            n193 = event-data() -> ()  [unwired: 1 in, 6 out]
            n194 = call "LabJack_FGV.vi"("Operation(Read)"=enum16{"Write", "Read"}."Read" ("Operation"), "error in (no error)"=w343) -> ("error out"=w348:errorcluster, "Read data"=w349:i32)  [unwired: 8 in]
            n195 = global read "GlobalVariables.vi" "Ch2 LJ pin"() -> (w347:string)
            n196 = call "LJM_eWriteName.vi"("Handle In"=w349, "Name"=w347, "Value"="V 2", "error in"=w348) -> ("error out"=w346:errorcluster)  [unwired: 10 in, 1 out]
            n197 = call "V2FGV.vi"("Error In"=w346, "action(write)"=enum16{"write", "read"}."write" ("action"), "V2 in"="V 2") -> ("Error Out"=w345:errorcluster)  [unwired: 7 in, 1 out]
            n198 = call "CtrlVtoGain.vi"("error in (no error)"=w345, "CtrlV(V)"="V 2", "Channel"=enum16{"Ch1", "Ch2", "Ch3"}."Ch2" ("Enum")) -> ("error out"=w341:errorcluster, "Gain"=w342:dbl)  [unwired: 7 in]
            n199 = local write "Gain2"(w342) -> ()
          }
          event "V 3": Value Change {
            n200 = event-data() -> ()  [unwired: 1 in, 6 out]
            n201 = call "LabJack_FGV.vi"("Operation(Read)"=enum16{"Write", "Read"}."Read" ("Operation"), "error in (no error)"=w355) -> ("error out"=w360:errorcluster, "Read data"=w361:i32)  [unwired: 8 in]
            n202 = global read "GlobalVariables.vi" "Ch3 LJ pin"() -> (w359:string)
            n203 = call "LJM_eWriteName.vi"("Handle In"=w361, "Name"=w359, "Value"="V 3", "error in"=w360) -> ("error out"=w357:errorcluster)  [unwired: 10 in, 1 out]
            n204 = call "V3FGV.vi"("Error In"=w357, "action(write)"=enum16{"write", "read"}."write" ("action"), "V3 in"="V 3") -> ("Error Out"=w356:errorcluster)  [unwired: 7 in, 1 out]
            n205 = call "CtrlVtoGain.vi"("error in (no error)"=w356, "CtrlV(V)"="V 3", "Channel"=enum16{"Ch1", "Ch2", "Ch3"}."Ch3" ("Enum")) -> ("error out"=w364:errorcluster, "Gain"=w363:dbl)  [unwired: 7 in]
            n206 = local write "Gain3"(w363) -> ()
          }
          event "V 4": Value Change {
            n207 = event-data() -> ()  [unwired: 1 in, 6 out]
            n208 = call "LabJack_FGV.vi"("Operation(Read)"=enum16{"Write", "Read"}."Read" ("Operation"), "error in (no error)"=w371) -> ("error out"=w375:errorcluster, "Read data"=w376:i32)  [unwired: 8 in]
            n209 = global read "GlobalVariables.vi" "Ch4 LJ pin"() -> (w374:string)
            n210 = call "LJM_eWriteName.vi"("Handle In"=w376, "Name"=w374, "Value"="V 4", "error in"=w375) -> ("error out"=w373:errorcluster)  [unwired: 10 in, 1 out]
            n211 = call "V4FGV.vi"("Error In"=w373, "action(write)"=enum16{"write", "read"}."write" ("action"), "V3 in"="V 4") -> ("Error Out"=w372:errorcluster)  [unwired: 7 in, 1 out]
            n212 = call "CtrlVtoGain.vi"("error in (no error)"=w372, "CtrlV(V)"="V 4", "Channel"=enum16{"Ch1", "Ch2", "Ch3", "Ch4"}."Ch4") -> ("error out"=w379:errorcluster, "Gain"=w378:dbl)  [unwired: 7 in]
            n213 = local write "Gain4"(w378) -> ()
          }
          event "Quit": Value Change {
            # "Exit Button Value Change (pressed) Event\n(when pressed.  quite)"
            n214 = event-data() -> ()  [unwired: 1 in, 1 out]
            n215 = call <vilib>:"Add State(s) to Queue__JKI_lib_State_Machine.vi"("State(s) in Front (\"\")"="LED: Off\nMacro: Exit", "State(s) in (\"\")"=w387) -> ("States Out"=w386:string)  [unwired: 13 in]
          }
          event "Show BG": Value Change {
            n216 = event-data() -> ()  [unwired: 1 in, 6 out]
            n217 = call <vilib>:"Add State(s) to Queue__JKI_lib_State_Machine.vi"("State(s) in Front (\"\")"="Data: showBG" ("State(s) in Front (\"\")"), "State(s) in (\"\")"=w390) -> ("States Out"=w389:string)  [unwired: 13 in]
          }
          event "StartButton": Mouse Enter {
            n218 = event-data() -> ()  [unwired: 1 in, 4 out]
            n219 = local write "Help"("Press to start aquisition." ("Help")) -> ()
          }
          event "StartButton": Value Change {
            # "[Covers: REQ32]"
            # "start PWM before acquisition"
            # "Initialize both digitizer aquisition and\n send user event to trigger aquisition loop"
            n220 = event-data() -> ()  [unwired: 1 in, 6 out]
            n221 = local write "StartButton"(FALSE ("StartButton")) -> ()
            n222 = Bundle By Name(cluster=w399, "SysRunning?"=TRUE) -> (w401:T29)
            n223 = call <vilib>:"Add State(s) to Queue__JKI_lib_State_Machine.vi"("State(s) in Front (\"\")"="/*TCP: stopCam\nUSBCAM: Stop\nUtility: SetDataClass >> Data\nQueue: Flash\nUI: Update\nUSBCAM: StartAndSave\nUtility: StartBeep\nLabJack: 355_PWM_Start\nLabJack: AB_Start\nLabJack: SetV\nDigitizer: Start\nUtility: AquiTimerReset\nUI: DuringAquisition\nLED: BreathGreen\nStage: Scan\n/*TCP: sendRunNum\n/*TCP: sendVideoSource\n/*TCP: sendChannel\n/*TCP: startRun", "State(s) in (\"\")"=w403) -> ("States Out"=w404:string)  [unwired: 13 in]
          }
          event User Event {
            # "[Covers: REQ32]"
            # "start PWM before acquisition"
            # "Initialize both digitizer aquisition and\n send user event to trigger aquisition loop"
            n224 = event-data() -> ()  [unwired: 1 in, 5 out]
            n225 = Bundle By Name(cluster=w406, "SysRunning?"=TRUE) -> (w408:T29)
            n226 = call <vilib>:"Add State(s) to Queue__JKI_lib_State_Machine.vi"("State(s) in Front (\"\")"="/*TCP: stopCam\nUtility: SetDataClass >> Data\nQueue: Flash\nUI: Update\nUtility: StartBeep\nLabJack: 355_PWM_Start\nLabJack: AB_Start\nLabJack: SetV\nDigitizer: Start\nUtility: AquiTimerReset\nUI: DuringAquisition\nLED: BreathGreen\n/*TCP: sendRunNum\n/*TCP: sendVideoSource\n/*TCP: sendChannel\n/*TCP: startRun", "State(s) in (\"\")"=w410) -> ("States Out"=w411:string)  [unwired: 13 in]
          }
          event "Video Display": Value Change {
            n227 = event-data() -> ("NewVal"=w417:bool)  [unwired: 1 in, 5 out]
            n228 = Select(t="/*TCP: startCam", s=w417, f="/*TCP: stopCam") -> (s? t:f=w414:string)
            n229 = call <vilib>:"Add State(s) to Queue__JKI_lib_State_Machine.vi"("State(s) in (\"\")"=w416, "State(s) at Back (\"\")"=w414) -> ("States Out"=w415:string)  [unwired: 13 in]
          }
          event "Video Source": Value Change {
            n230 = event-data() -> ()  [unwired: 1 in, 6 out]
            n231 = call <vilib>:"Add State(s) to Queue__JKI_lib_State_Machine.vi"("State(s) in Front (\"\")"="TCP: sendVideoSource" ("State(s) in Front (\"\")"), "State(s) in (\"\")"=w422) -> ("States Out"=w421:string)  [unwired: 13 in]
          }
          event "StopButton": Mouse Enter {
            n232 = event-data() -> ()  [unwired: 1 in, 4 out]
            n233 = local write "Help"("Press to stop data aquisition." ("Help")) -> ()
          }
          event "StopButton": Value Change {
            # "if system is running, send stop command, if not do nothing."
            # "stop aquisition\nupdate UI"
            n234 = event-data() -> ()  [unwired: 1 in, 6 out]
            n235 = Unbundle By Name(w430) -> ("SysRunning?"=w432:bool)
            n236 = case shown="True" w432 {
              tunnel: ["" ("Empty String Constant") "LabJack: AB_Stop\nLabJack: 355_PWM_Stop\n/*Digitizer: Abort"] -> w433
              tunnel: w430 -> [w437 w441]
              tunnel: [w437 w440] -> w431
              frame False {
              }
              frame True {
                n237 = Bundle By Name(cluster=w441, "SysRunning?"=FALSE) -> (w440:T29)
              }
            }
            n238 = call <vilib>:"Add State(s) to Queue__JKI_lib_State_Machine.vi"("State(s) in Front (\"\")"=w433, "State(s) in (\"\")"=w435) -> ("States Out"=w436:string)  [unwired: 13 in]
            n239 = local write "StopButton"(FALSE ("StopButton")) -> ()
          }
          event User Event {
            # "if system is running, send stop command, if not do nothing."
            # "stop aquisition\nupdate UI"
            n240 = event-data() -> ()  [unwired: 1 in, 5 out]
            n241 = Unbundle By Name(w443) -> ("SysRunning?"=w445:bool)
            n242 = case shown="True" w445 {
              tunnel: ["" ("Empty String Constant") "LabJack: AB_Stop\nLabJack: 355_PWM_Stop\n/*Digitizer: Abort"] -> w446
              tunnel: w443 -> [w450 w454]
              tunnel: [w450 w453] -> w444
              frame False {
              }
              frame True {
                n243 = Bundle By Name(cluster=w454, "SysRunning?"=FALSE) -> (w453:T29)
              }
            }
            n244 = call <vilib>:"Add State(s) to Queue__JKI_lib_State_Machine.vi"("State(s) in Front (\"\")"=w446, "State(s) in (\"\")"=w448) -> ("States Out"=w449:string)  [unwired: 13 in]
          }
          event "Sys Reconfig": Mouse Enter {
            n245 = event-data() -> ()  [unwired: 1 in, 4 out]
            n246 = local write "Help"("Click to reconfig digitizer settings." ("Help")) -> ()
          }
          event "Sys Reconfig": Value Change {
            # "everytime the user change data aquisition setting, need to reinitilize decon engine and realign iRF.\ncheck whether data length has changed, if changed, reinitialize Decon engine\nreset BG ready, need a new BG"
            # "update DAQ FGV"
            n247 = event-data() -> ()  [unwired: 1 in, 6 out]
            n248 = call "SystemConfigEditorV6.vi"("error in"=w470) -> ("error out"=w469:errorcluster, "FLImDAQ out"=w464:T9)  [unwired: 1 in]
            n249 = Unbundle By Name(w467) -> ("FLImDAQ.min record length"=w466:i32)
            n250 = Unbundle By Name(w464) -> ("min record length"=w465:i32)
            n251 = call "FLImDAQ_FGV.vi"("error in (no error)"=w469, "Operation (Read)"=enum16{"Write", "Read"}."Write" ("Operation"), "Write data"=w464) -> ("error out"=w468:errorcluster, "Read data"=w463:T9)  [unwired: 7 in]
            n252 = Equal?(x=w466, y=w465) -> (x = y?=w462:bool)
            n253 = case shown="False" w462 {
              tunnel: ["UI: Cursor Set >> Busy\nDigitizer: Config\nDeconEngine: InitializeCh1\nDeconEngine: InitializeCh2\nDeconEngine: InitializeCh3\nUI: CaliAndiRFNotReady\n/*UI iRF not ready\nUI: Update\nUI: Cursor Set >> Idle" "UI: Cursor Set >> Busy\nDigitizer: Config\nUI: Update\nUI: Cursor Set >> Idle"] -> w461
              frame False {
              }
              frame True {
              }
            }
            n254 = Bundle By Name(cluster=w467, "FLImDAQ"=w463) -> (w473:T29)
            n255 = call <vilib>:"Add State(s) to Queue__JKI_lib_State_Machine.vi"("State(s) in Front (\"\")"=w461, "State(s) in (\"\")"=w471) -> ("States Out"=w472:string)  [unwired: 13 in]
          }
          event "System Hardware Connection Status", "StartButton", "StopButton", "355nm Laser toggle", "Aiming beam toggle", "Cali&iRF alignment", "Background", "Sys Reconfig": Mouse Leave {
            n256 = event-data() -> ()  [unwired: 1 in, 4 out]
            n257 = invoke on="Help" class="Str" method="Reinit To Default"() -> ()  [unwired: 3 in, 3 out]
          }
          event "System Hardware Connection Status.Digitizer": Mouse Enter {
            n258 = event-data() -> ()  [unwired: 1 in, 4 out]
            n259 = local write "Help"("Status of hardware connections. TCP/IP is optional." ("Help")) -> ()
          }
          event "TCP Connect": Value Change {
            n260 = event-data() -> ("NewVal"=w483:bool)  [unwired: 1 in, 5 out]
            n261 = case shown="False" w483 {
              tunnel: ["/*TCP: Close\nUI: Update" ("State(s) in Front (\"\")") "/*TCP: SendSettingMacro\nUI: Update" ("State(s) in Front (\"\")")] -> w484
              frame False {
              }
              frame True {
              }
            }
            n262 = call <vilib>:"Add State(s) to Queue__JKI_lib_State_Machine.vi"("State(s) in Front (\"\")"=w484, "State(s) in (\"\")"=w486) -> ("States Out"=w485:string)  [unwired: 13 in]
          }
          event User Event {
            # "if aquisition loop is error out. Stop digitizer, update front panel indicator, stop both laser and \nOption 1: parse and save data\nOption 2: Flash queue if scout run. [Covers: REQ23]"
            n263 = event-data() -> ()  [unwired: 1 in, 5 out]
            n264 = case shown="\"Data\", Default" "Data Class" {
              tunnel: [w508 "UI: Cursor Set >> Busy\nUtility: SetAllChanAutoGain\nUtility: RestoreDeConChan\nData: parseRunData\nData: irfAlignment\nUI: Cursor Set >> Idle" "UI: Cursor Set >> Busy\nUtility: SetAllChanAutoGain\nUtility: RestoreDeConChan\nData: parseRunData\nData: saveBGtoFGV\nData: saveBGtoFile\nUI: Cursor Set >> Idle\nData: showBG\nRun: BGIncrement"] -> w498
              frame "Data", Default {
                n265 = local read "Video Display"() -> (w510:bool)
                n266 = Select(t="/*TCP: startCam", s=w510, f="") -> (s? t:f=w506:string)
                n267 = call <vilib>:"Add State(s) to Queue__JKI_lib_State_Machine.vi"("State(s) in Front (\"\")"="UI: Cursor Set >> Busy\nData: parseRunData\nData: saveRunData\nUI: Cursor Set>>Idle" ("State(s) in Front (\"\")"), "State(s) in (\"\")"=w506) -> ("States Out"=w508:string)  [unwired: 13 in]
              }
              frame "Cali" {
              }
              frame "BG" {
              }
            }
            n268 = Bundle By Name(cluster=w500, "SysRunning?"=FALSE) -> (w501:T29)
            n269 = Select(t="" ("State(s) in Front (\"\")"), s="Skip Data Save?", f=w498) -> (s? t:f=w495:string)
            n270 = call <vilib>:"Add State(s) to Queue__JKI_lib_State_Machine.vi"("State(s) in Front (\"\")"="/*TCP: stopRun\nUI: Update\nUSBCAM: Stop\nDigitizer: Abort\nLabJack: ZeroV\nUtility: EndBeep\nLED: BreathOff\n" ("State(s) in Front (\"\")"), "State(s) in (\"\")"=w495, "State(s) at Back (\"\")"="Macro: SysReadyForAq\nUI: Update\nUSBCAM: StartNoSave" ("State(s) in Front (\"\")")) -> ("States Out"=w493:string)  [unwired: 12 in]
            n271 = call <vilib>:"Add State(s) to Queue__JKI_lib_State_Machine.vi"("State(s) in Front (\"\")"=w493, "State(s) in (\"\")"=w502) -> ("States Out"=w503:string)  [unwired: 13 in]
          }
          event Panel Close? {
            # "Discard the event because we'll close the front panel ourselves in Macro: Exit"
            # "Close Panel button (pressed) Event\n(this executes Macro: Exit to terminate the VI)"
            n272 = event-data() -> ()  [unwired: 1 in, 1 out]
            n273 = call <vilib>:"Add State(s) to Queue__JKI_lib_State_Machine.vi"("State(s) in Front (\"\")"="Macro: Exit", "State(s) in (\"\")"=w518) -> ("States Out"=w517:string)  [unwired: 13 in]
            n274 = event-data ("Event Filter Node")("Discard?"=TRUE) -> ()  [unwired: 1 in, 1 out]
          }
        }
      }
      frame "---------- Macro ----------" {
        # "Do not put any code in this frame.\n(It is a separator no-op. You can make a copy of this frame to create a new Macro frame)"
        n275 = call <vilib>:"Add State(s) to Queue__JKI_lib_State_Machine.vi"("State(s) in (\"\")"=w523) -> ("States Out"=w522:string)  [unwired: 14 in]
      }
      frame "Macro: Initialize" {
        # "load Labjack setting 1st as it contaisn laser pin infortmation"
        # "start laser 1st, need 7.5s for laser to get ready"
        # "Initialization Macro\n(This is called once, when the VI starts)"
        n276 = call <vilib>:"Add State(s) to Queue__JKI_lib_State_Machine.vi"("State(s) in Front (\"\")"="UI: showDisclaimer\nUI: Cursor Set >> Busy\nData: Initialize\nInitialize Core Data\nUI: Initialize\nUI: Front Panel State >> Open\nMacro: LoadSysConfig\nUSBCAM: Init\nUSBCAM: Config\n/*TCP: InitializeNew\n/*TCP: checkSource\nUI: Update\nLabJack: Open\nLabJack: SetDefaultSub\nLED: OpenVIRef\nLED: BreathOrange\nUI: Update\n355 Laser: CheckControllerStatus\n355 Laser: Laser enable\n355 Laser: Dewelling>>500\n355 Laser: CheckControllerStatus\nUI: Update\nLabJack: 355_PWM_Config\nLabJack: AB_PWM_Config\nUI: Update", "State(s) in (\"\")"="Digitizer: Initialize\nDigitizer: Config\nUI: Update\nAimingBeam: Initialize\nAimingBeam: Set Status>>Enable\nAimingBeam: Set Current\nUI: Update\n355 Laser: Check Dewelling\nUSBCAM: StartNoSave\nStage: BuildDeviceList\nStage: Connect\nStage: WaitSettingToLoad\nStage: GetDeviceInfo\nStage: CheckStatus\nStage: Home\nUI: Cursor Set >> Idle\nCase: GetID\nUI: Update\n/*TCP: SendSettingMacro\nCase: CreatFileStruct\nUI: Update\nData: loadLastUseMacro\nDeconEngine: InitilizeMacro\nGraph: SetXMultiplier\nGraph: AddCursors\nAPD: Initialize\nAPD: LoadFromSerial\nAPD: UpdateCtrlVLimit\nAPD: GetGainLimits\nPID: loadPID\nLED: BreathOff\nMacro: SysReadyForAq") -> ("States Out"=w524:string)  [unwired: 13 in]
        n277 = call <vilib>:"Add State(s) to Queue__JKI_lib_State_Machine.vi"("State(s) in Front (\"\")"=w524, "State(s) in (\"\")"=w532) -> ("States Out"=w531:string)  [unwired: 13 in]
        "Help" <- "Hover over controls to see help!" ("Help")
      }
      frame "Macro: LoadSysConfig" {
        # "System configuration Macro. [Covers: REQ15]\n(Load configurations for different component of the system)"
        n278 = call <vilib>:"Add State(s) to Queue__JKI_lib_State_Machine.vi"("State(s) in Front (\"\")"="SysConfig: Load Sys Config\nSysConfig: Load Digitizer Setting\nSysConfig: Load AB setting\nSysConfig: Load LJ Pinout\nSysConfig: Load 355 PWM\nSysConfig: LoadAPDSerialNumber\nSysConfig: LoadABVideoSetting\nSysConfig: LoadCursorLocation", "State(s) in (\"\")"=w538) -> ("States Out"=w537:string)  [unwired: 13 in]
      }
      frame "Macro: SysReadyForAq" {
        # "Macro for system ready\n(It is a separator no-op. You can make a copy of this frame to create a new Macro frame)"
        n279 = call <vilib>:"Add State(s) to Queue__JKI_lib_State_Machine.vi"("State(s) in Front (\"\")"="UI: ReadyForAquisition\nLED: Green" ("State(s) in Front (\"\")"), "State(s) in (\"\")"=w544) -> ("States Out"=w543:string)  [unwired: 13 in]
      }
      frame "Macro: Exit" {
        # "close LJ last"
        # "check whether hardware is initilized, if so close, if not do nothing"
        # "Exit Macro, close all hardware\n(This is called once, when the VI exits)"
        n280 = Unbundle By Name(w563) -> ("System Status.Digitizer"=w559:bool, "System Status.Aiming Beam"=w558:bool, "System Status.355 Laser"=w557:bool, "System Status.Labjack"=w548:bool, "Core.Close Panel on Exit?"=w552:bool)
        n281 = case shown="True" w559 {
          tunnel: ["" ("Empty String Constant") "Digitizer: Close"] -> w554
          frame False {
          }
          frame True {
          }
        }
        n282 = case shown="True" w548 {
          tunnel: ["" ("Empty String Constant") "LabJack: SetDefaultAndClose"] -> w545
          frame False {
          }
          frame True {
          }
        }
        n283 = case shown="True" w558 {
          tunnel: ["" ("Empty String Constant") w570] -> w547
          frame False {
          }
          frame True {
            w570 = "AimingBeam: Set Status >> Disable\nAimingBeam: Close"  # AimingBeam: Set Status >> Disable AimingBeam: Close
          }
        }
        n284 = case shown="True" w557 {
          tunnel: ["" ("Empty String Constant") "355 Laser: Close\n355 Laser: CheckControllerStatus"] -> w546
          frame False {
          }
          frame True {
          }
        }
        n285 = Select(t="UI: Front Panel State >> Close", s=w552, f="" ("Empty String Constant")) -> (s? t:f=w549:string)
        n286 = call <vilib>:"Add State(s) to Queue__JKI_lib_State_Machine.vi"("State(s) in Front (\"\")"="USBCAM: Close\nStage: Close", "State(s) in (\"\")"=w554, "State(s) at Back (\"\")"=w547) -> ("States Out"=w556:string)  [unwired: 12 in]
        n287 = call <vilib>:"Add State(s) to Queue__JKI_lib_State_Machine.vi"("State(s) in Front (\"\")"=w556, "State(s) in (\"\")"=w546, "State(s) at Back (\"\")"=w545) -> ("States Out"=w551:string)  [unwired: 12 in]
        n288 = call <vilib>:"Add State(s) to Queue__JKI_lib_State_Machine.vi"("State(s) in Front (\"\")"=w551, "State(s) in (\"\")"="UI: Update\nUI: Reset\nGraph: SaveCursorLoc\nLED: CloseVIRef\nQueue: Destory\nData: Cleanup\nExit", "State(s) at Back (\"\")"=w549) -> ("States Out"=w560:string)  [unwired: 12 in]
        n289 = call <vilib>:"Add State(s) to Queue__JKI_lib_State_Machine.vi"("State(s) in Front (\"\")"=w560, "State(s) in (\"\")"=w566) -> ("States Out"=w565:string)  [unwired: 13 in]
      }
      frame "---------- Data ----------" {
        # "Do not put any code in this frame.\n(It is a separator no-op. You can make a copy of this frame to create a new Data frame)"
        n290 = call <vilib>:"Add State(s) to Queue__JKI_lib_State_Machine.vi"("State(s) in (\"\")"=w579) -> ("States Out"=w578:string)  [unwired: 14 in]
      }
      frame "Data: Initialize" {
        w582 = ""  # StageSerial
        w583 = path ""  # CaliPath
        w584 = dbl[] []  # V4
        w585 = dbl[][] []  # Ch4Data
        w586 = FALSE  # bothVidSourceAvail
        w587 = T2 {"Main Frame Grabber"=FALSE, "Side Frame Grabber"=FALSE, "Main Camera"=FALSE, "Side Camera"=FALSE}  # video source
        w588 = FALSE  # LED vi ref open?
        w590 = T28 {"DeCon Channel"=enum."1", "Scale Bar"=FALSE, "Scale Low"=3.0, "Scale High"=8.0, "ANSI"=20.0, "Radius"=1.0, "3D?"=FALSE, "Firefly?"=FALSE, "Pentero?"=FALSE}  # VideoConfig
        w591 = T32 {"Ch1APDSerial#"="", "Ch2APDSerial#"="", "Ch3APDSerial#"="", "Ch4APDSerial#"=""}  # APDSerialNum
        w592 = u32 0  # Aquisition Timer
        w593 = cluster{"RunID":i8, "BG ID":i8, "Cali ID":i8} {"RunID"=1, "BG ID"=1, "Cali ID"=1}  # IDs
        w594 = refnum<vi> refnum  # LED vi reference
        w595 = path ""  # TempPath
        w596 = T33 {"DataPath"=path "", "BG Path"=path "", "iRFPath"=path "", "CaliPath"=path ""}  # Pathes
        w598 = dbl[] []  # V3
        w599 = dbl[] []  # V2
        w600 = dbl[] []  # V1
        w602 = u32 0  # FastTimer
        w603 = u32 0  # SlowTimer
        w604 = dbl[][] []  # Ch3Data
        w605 = dbl[][] []  # Ch2Data
        w589 = dbl[][] []  # Ch1Data
        w608 = T3 {"Digitizer"=FALSE, "Labjack"=FALSE, "Aiming Beam"=FALSE, "355 Laser"=FALSE, "TCP/IP"=FALSE}  # System Status
        w609 = T34 {"DIO_EF_CLOCK1_DIVISOR"=16, "DIO_EF_CLOCK1_ROLL_VALUE"=25000, "DIO#_EF_INDEX"=0, "DIO#_EF_OPTIONS"=1, "DIO#_EF_CONFIG_A"=6250}  # AB PWM setting
        w610 = T8 {"Ch1 Bias"="TDA11", "Ch2 Bias"="DAC10", "Ch3 Bias"="DAC0", "Ch4 Bias"="DAC0", "355 PWM"="FIO0", "AimingBeam PWM"="FIO2", "Laser Ready"="FIO3", "Interlock"="FIO1", "Laser Start/Stop"="FIO1", "Red LED"="FIO1", "Green LED"="FIO1", "Foot Pedal"="DIO15"}  # LJ Pinout
        w611 = 0  # TCP attempt count
        w612 = u32 0  # Laser start tic
        w613 = refnum<k20>[] []  # niTClk sessions
        w614 = u32 0  # Last Trigger
        w615 = T34 {"DIO_EF_CLOCK1_DIVISOR"=16, "DIO_EF_CLOCK1_ROLL_VALUE"=25000, "DIO#_EF_INDEX"=0, "DIO#_EF_OPTIONS"=1, "DIO#_EF_CONFIG_A"=6250}  # 355 PWM setting
        w616 = T35 {"Aiming Beam COM Port"="COM3", "Min Current"=0.0, "Max Current"=63.0, "Default Current"=20.0, "Freq"=0}  # AB Cluster
        w617 = T36 {"resource name"="", "resource name 2"="", "Channel"=enum."Channel 0", "trigger source"="VAL_EXTERNAL", "trigger level"=0.5, "trigger delay"=1.35e-07, "min sample rate"=12500000000.0, "min record length"=2500, "vertical range"=1.0, "vertical offset"=-0.25, "Waveform to Avg"=2000}  # FLImDAQ
        w618 = FALSE  # SysRunning?
        w606 = path ""  # DefaultPath
        w619 = ""  # CaseID
        w620 = T7 {"Ch1Enable?"=FALSE, "Ch2Enable?"=FALSE, "Ch3Enable?"=FALSE, "Ch1AutoGain?"=FALSE, "Ch2AutoGain?"=FALSE, "Ch3AutoGain?"=FALSE, "AimingBeamEnable?"=FALSE}  # SysConfigCluster
        w621 = T37 {"Current VI Reference"=refnum, "Close Panel on Exit?"=FALSE}  # Core
        # "Initialize the shift-register data, here.\n(data names are defined by what you wire into the bundle function)"
        n291 = Bundle("Core"=w621, "SysConfigCluster"=w620, "System Status"=w608, "IDs"=w593, "CaseID"=w619, "DefaultPath"=w606, "Pathes"=w596, "FLImDAQ"=w617, "SysRunning?"=w618, "AB Cluster"=w616, "LJ Pinout"=w610, "355 PWM setting"=w615, "AB PWM setting"=w609, "Last Trigger"=w614, "niTClk sessions"=w613, "Laser start tic"=w612, "TCP attempt count"=w611, "Ch1Data"=w589, "Ch2Data"=w605, "Ch3Data"=w604, "Ch4Data"=w585, "V1"=w600, "V2"=w599, "V3"=w598, "V4"=w584, "SlowTimer"=w603, "FastTimer"=w602, "listener ID"=refnum<k5> refnum, "TempPath"=w595, "CaliPath"=w583, "LED vi reference"=w594, "Aquisition Timer"=w592, "APDSerialNum"=w591, "VideoConfig"=w590, "LED vi ref open?"=w588, "video source"=w587, "bothVidSourceAvail"=w586, "StageSerial"=w582, "DeviceHandle"=refnum<k24> refnum, "StageHomed?"=FALSE) -> (w597:T29)  [unwired: 1 in]
        n292 = call <vilib>:"Add State(s) to Queue__JKI_lib_State_Machine.vi"("State(s) in (\"\")"=w624) -> ("States Out"=w623:string)  [unwired: 14 in]
      }
      frame "Data: loadLastUseMacro" {
        # "Load last use BG and Cali and iRF.\n(It is a separator no-op. You can make a copy of this frame to create a new Data frame)"
        n293 = call <vilib>:"Add State(s) to Queue__JKI_lib_State_Machine.vi"("State(s) in Front (\"\")"="Data: loadLastUseBG\nData: loadSystemCali\nData: loadLastUseiRF\n/*Data: LoadiRFFromAPDFile\nUI: CaliAndiRFLoaded\nData: ShowiRF" ("State(s) in Front (\"\")"), "State(s) in (\"\")"=w630) -> ("States Out"=w629:string)  [unwired: 13 in]
      }
      frame "Data: loadLastUseBG" {
        w634 = enum16{"write", "read"}."write" ("action")
        # "Load last use BG.\n()"
        n294 = Unbundle By Name(w653) -> ("TempPath"=w652:path)
        n295 = call "FLImDAQ_FGV.vi"() -> ("Read data"=w648:T9)  [unwired: 10 in, 1 out]
        n296 = Build Path(base path=w652, name or relative path="Background.tdms") -> (appended path=w651:path)
        n297 = call "ReadBGorCali (SubVI).vi"("DataType"=enum16{"BG", "Cali"}."BG", "error in (no error)"=w650, "file path in"=w651) -> ("error out"=w649:errorcluster, "AvgDataCluster"=w644:T38)  [unwired: 6 in, 1 out]
        n298 = Unbundle By Name(w644) -> ("Channel 1"=w631:dbl[], "Channel 2"=w643:dbl[], "Channel 3"=w636:dbl[], "Channel 4"=w633:dbl[])
        n299 = Unbundle By Name(w648) -> ("min record length"=w640:i32)
        n300 = Array Size(array=w631) -> (size(s)=w642:i32)
        "BG length" <- w642
        n301 = Equal?(x=w642, y=w640) -> (x = y?=w641:bool)
        n302 = Select(t="UI: BGLoaded" ("State(s) in Front (\"\")"), s=w641, f="UI: BGSizeError" ("State(s) in Front (\"\")")) -> (s? t:f=w645:string)
        n303 = case shown="True" w641 {
          tunnel: w631 -> [_ w664]
          tunnel: w643 -> [_ w663]
          tunnel: w636 -> [_ w662]
          tunnel: w640 -> [w659 _]
          tunnel: [w658 w664] -> w639
          tunnel: [w658 w663] -> w638
          tunnel: [w658 w662] -> w637
          tunnel: w633 -> [_ w661]
          tunnel: [w658 w661] -> w632
          frame False {
            # "If error set BG all 0, update UI"
            n304 = for {
              N: w659 -> [_]
              tunnel: [0.0] -> w658 mode=indexing
            }
          }
          frame True {
            # "If no error, check size match"
          }
        }
        n305 = call "BG4FGV.vi"("action"=w634, "BG4 in"=w632) -> ()  [unwired: 8 in, 2 out]
        n306 = call "BG3FGV.vi"("action"=w634, "BG3 in"=w637) -> ()  [unwired: 8 in, 2 out]
        n307 = call "BG1FGV.vi"("action"=w634, "BG1 in"=w639) -> ()  [unwired: 8 in, 2 out]
        n308 = call "BG2FGV.vi"("action"=w634, "BG2 in"=w638) -> ()  [unwired: 8 in, 2 out]
        n309 = call <vilib>:"Add State(s) to Queue__JKI_lib_State_Machine.vi"("State(s) in Front (\"\")"=w645, "State(s) in (\"\")"=w657) -> ("States Out"=w656:string)  [unwired: 13 in]
      }
      frame "Data: loadSystemCali" {
        # "Load last use calibration.\n()"
        n310 = Unbundle By Name(w672) -> ("CaliPath"=w671:path)
        n311 = Build Path(base path=w671, name or relative path="Calibration.tdms") -> (appended path=w667:path)
        n312 = call "ReadBGorCali (SubVI).vi"("DataType"=enum16{"BG", "Cali"}."Cali", "error in (no error)"=w666, "file path in"=w667) -> ("error out"=w668:errorcluster, "CtrlVCluster"=w670:T39, "AvgDataCluster"=w669:T38)  [unwired: 6 in]
        n313 = case shown="No Error" w668 {
          tunnel: w670 -> [w691 _]
          tunnel: w669 -> [w690 _]
          frame No Error {
            w681 = T40 {"Ch1 WF"=[], "Ch2 WF"=[], "Ch3 WF"=[], "Ch4 WF"=[], "V1"=0.0, "V2"=0.0, "V3"=0.0, "V4"=0.0}  # SysCaliData
            n314 = Unbundle By Name(w690) -> ("Channel 1"=w689:dbl[], "Channel 2"=w688:dbl[], "Channel 3"=w687:dbl[], "Channel 4"=w680:dbl[])
            n315 = Unbundle By Name(w691) -> ("V 1"=w686:dbl[], "V 2"=w685:dbl[], "V 3"=w679:dbl[], "V 4"=w677:dbl[])
            n316 = Index Array(array=w686) -> (element=w684:dbl)  [unwired: 1 in]
            n317 = Index Array(array=w685) -> (element=w683:dbl)  [unwired: 1 in]
            n318 = Index Array(array=w679) -> (element=w682:dbl)  [unwired: 1 in]
            n319 = Index Array(array=w677) -> (element=w678:dbl)  [unwired: 1 in]
            n320 = Bundle By Name(cluster=w681, "Ch1 WF"=w689, "Ch2 WF"=w688, "Ch3 WF"=w687, "Ch4 WF"=w680, "V1"=w684, "V2"=w683, "V3"=w682, "V4"=w678) -> (w692:T40)
            n321 = global write "GlobalVariables.vi" "SysCaliData"(w692) -> ()
          }
          frame Error {
          }
        }
        n322 = call <vilib>:"Add State(s) to Queue__JKI_lib_State_Machine.vi"("State(s) in (\"\")"=w676) -> ("States Out"=w675:string)  [unwired: 14 in]
      }
      frame "Data: LoadiRFFromAPDFile" {
        w722 = T18 {"Ch1 iRF"=[], "Ch2 iRF"=[], "Ch3 iRF"=[], "Ch4 iRF"=[]}  # LastUseiRF
        # "only load the last 5th  iRF for the moment"
        # "Load APD detector data\n(It is a separator no-op. You can make a copy of this frame to create a new Data frame)"
        n323 = Unbundle By Name(w744) -> ("APDSerialNum.Ch1APDSerial#"=w743:string, "APDSerialNum.Ch2APDSerial#"=w724:string, "APDSerialNum.Ch3APDSerial#"=w723:string, "APDSerialNum.Ch4APDSerial#"=w720:string)
        n324 = call "CreatFromSerialNumNoRaw.vi"("error in (no error)"=w721, "APD Serial #"=w743) -> ("error out"=w741:errorcluster, "APDClass out"=w742:refnum<class "APDClass.lvclass">)  [unwired: 8 in]
        n325 = call "CreatFromSerialNumNoRaw.vi"("error in (no error)"=w721, "APD Serial #"=w724) -> ("error out"=w732:errorcluster, "APDClass out"=w733:refnum<class "APDClass.lvclass">)  [unwired: 8 in]
        n326 = call "CreatFromSerialNumNoRaw.vi"("error in (no error)"=w721, "APD Serial #"=w723) -> ("error out"=w726:errorcluster, "APDClass out"=w727:refnum<class "APDClass.lvclass">)  [unwired: 8 in]
        n327 = call "CreatFromSerialNumNoRaw.vi"("error in (no error)"=w721, "APD Serial #"=w720) -> ("error out"=w718:errorcluster, "APDClass out"=w719:refnum<class "APDClass.lvclass">)  [unwired: 8 in]
        n328 = call-dynamic "Read iRFData.vi"("error in (no error)"=w741, "APDClass in"=w742) -> ("iRFData"=w740:T41)  [unwired: 7 in, 2 out]
        n329 = call-dynamic "Read iRFData.vi"("error in (no error)"=w732, "APDClass in"=w733) -> ("iRFData"=w736:T41)  [unwired: 7 in, 2 out]
        n330 = call-dynamic "Read iRFData.vi"("error in (no error)"=w726, "APDClass in"=w727) -> ("iRFData"=w730:T41)  [unwired: 7 in, 2 out]
        n331 = call-dynamic "Read iRFData.vi"("error in (no error)"=w718, "APDClass in"=w719) -> ("iRFData"=w717:T41)  [unwired: 7 in, 2 out]
        n332 = Unbundle By Name(w740) -> ("iRFWFsAvg"=w739:dbl[][])
        n333 = Unbundle By Name(w736) -> ("iRFWFsAvg"=w735:dbl[][])
        n334 = Unbundle By Name(w730) -> ("iRFWFsAvg"=w729:dbl[][])
        n335 = Unbundle By Name(w717) -> ("iRFWFsAvg"=w714:dbl[][])
        n336 = Array Size(array=w739) -> (size(s)=w738:i32[])
        n337 = Array Size(array=w735) -> (size(s)=w731:i32[])
        n338 = Array Size(array=w729) -> (size(s)=w725:i32[])
        n339 = Array Size(array=w714) -> (size(s)=w715:i32[])
        n340 = Index Array(array=w738, index=0) -> (element=w713:i32)
        n341 = Index Array(array=w731, index=0) -> (element=w709:i32)
        n342 = Index Array(array=w725, index=0) -> (element=w706:i32)
        n343 = Index Array(array=w715, index=0) -> (element=w703:i32)
        n344 = Subtract(x=w713, y=5) -> (x-y=w711:i32)
        n345 = Subtract(x=w709, y=5) -> (x-y=w708:i32)
        n346 = Subtract(x=w706, y=5) -> (x-y=w705:i32)
        n347 = Subtract(x=w703, y=5) -> (x-y=w702:i32)
        n348 = Index Array(array=w739, index (row)=w711) -> (element=w701:dbl[])  [unwired: 1 in]
        n349 = Index Array(array=w735, index (row)=w708) -> (element=w700:dbl[])  [unwired: 1 in]
        n350 = Index Array(array=w729, index (row)=w705) -> (element=w699:dbl[])  [unwired: 1 in]
        n351 = Index Array(array=w714, index (row)=w702) -> (element=w698:dbl[])  [unwired: 1 in]
        n352 = call "DownSampleAndShiftiRF (SubVI).vi"("ArrayIn"=w701) -> ("ArrayOut"=w697:dbl[])  [unwired: 10 in]
        n353 = call "DownSampleAndShiftiRF (SubVI).vi"("ArrayIn"=w700) -> ("ArrayOut"=w693:dbl[])  [unwired: 10 in]
        n354 = call "DownSampleAndShiftiRF (SubVI).vi"("ArrayIn"=w699) -> ("ArrayOut"=w694:dbl[])  [unwired: 10 in]
        n355 = call "DownSampleAndShiftiRF (SubVI).vi"("ArrayIn"=w698) -> ("ArrayOut"=w696:dbl[])  [unwired: 10 in]
        n356 = call <vilib>:"Add State(s) to Queue__JKI_lib_State_Machine.vi"("State(s) in (\"\")"=w747) -> ("States Out"=w746:string)  [unwired: 14 in]
        n357 = Bundle(cluster=w722, "Ch1 iRF"=w697, "Ch2 iRF"=w693, "Ch3 iRF"=w694, "Ch4 iRF"=w696) -> (w695:T18)
        n358 = global write "GlobalVariables.vi" "LastUseiRF"(w695) -> ()
      }
      frame "Data: loadLastUseiRF" {
        # "Load last use iRF.\n()"
        n359 = Unbundle By Name(w753) -> ("TempPath"=w752:path)
        n360 = Build Path(base path=w752, name or relative path="iRF.tdms") -> (appended path=w758:path)
        n361 = TDMS Open(8:w748, 11:w758) -> (0:w756:errorcluster, 3:w757:refnum<k34>)  [unwired: 5 in]
        n362 = TDMS Read(0:w757, 11:w756, 12:dbl[][] []) -> (4:w751:refnum<k34>, 10:w754:dbl[][], 15:w750:errorcluster)  [unwired: 5 in, 3 out]
        n363 = TDMS Close(8:w750, 11:w751) -> (0:w749:errorcluster)  [unwired: 1 out]
        n364 = case shown="No Error" w750 {
          tunnel: w754 -> [w764 _]
          frame No Error {
            w768 = T18 {"Ch1 iRF"=[], "Ch2 iRF"=[], "Ch3 iRF"=[], "Ch4 iRF"=[]}  # LastUseiRF
            n365 = Index Array(array=w764, index (row)=0) -> (element=w777:dbl[])  [unwired: 1 in]
            n366 = Index Array(array=w764, index (row)=1) -> (element=w774:dbl[])  [unwired: 1 in]
            n367 = Index Array(array=w764, index (row)=2) -> (element=w771:dbl[])  [unwired: 1 in]
            n368 = Index Array(array=w764, index (row)=3) -> (element=w766:dbl[])  [unwired: 1 in]
            n369 = Add Array Elements(numeric array=w777) -> (sum=w776:dbl)
            n370 = Add Array Elements(numeric array=w774) -> (sum=w773:dbl)
            n371 = Add Array Elements(numeric array=w771) -> (sum=w770:dbl)
            n372 = Add Array Elements(numeric array=w766) -> (sum=w765:dbl)
            n373 = Divide(x=w777, y=w776) -> (x/y=w775:dbl[])
            n374 = Divide(x=w774, y=w773) -> (x/y=w772:dbl[])
            n375 = Divide(x=w771, y=w770) -> (x/y=w769:dbl[])
            n376 = Divide(x=w766, y=w765) -> (x/y=w763:dbl[])
            n377 = Bundle(cluster=w768, "Ch1 iRF"=w775, "Ch2 iRF"=w772, "Ch3 iRF"=w769, "Ch4 iRF"=w763) -> (w779:T18)
            n378 = Array Size(array=w777) -> (size(s)=→"iRF length":i32)
            n379 = global write "GlobalVariables.vi" "LastUseiRF"(w779) -> ()
          }
          frame Error {
          }
        }
        n380 = call <vilib>:"Add State(s) to Queue__JKI_lib_State_Machine.vi"("State(s) in (\"\")"=w762) -> ("States Out"=w761:string)  [unwired: 14 in]
      }
      frame "Data: ShowiRF" {
        # "Show loaded iRF.\n(It is a separator no-op. You can make a copy of this frame to create a new Data frame)"
        n381 = global read "GlobalVariables.vi" "LastUseiRF"() -> (w788:T18)
        n382 = Unbundle By Name(w788) -> ("Ch1 iRF"=w787:dbl[], "Ch2 iRF"=w786:dbl[], "Ch3 iRF"=w785:dbl[], "Ch4 iRF"=w784:dbl[])
        n383 = Build Array(w787, w786, w785, w784) -> (→"iRF Graph":dbl[][])
        n384 = call <vilib>:"Add State(s) to Queue__JKI_lib_State_Machine.vi"("State(s) in (\"\")"=w793) -> ("States Out"=w792:string)  [unwired: 14 in]
      }
      frame "Data: saveCalibration" {
        # "Average data and save calibration file. [Covers: REQ11]\n(It is a separator no-op. You can make a copy of this frame to create a new Data frame)"
        n385 = Unbundle By Name(w812) -> ("Ch1Data"=w811:dbl[][], "V1"=w810:dbl[], "Ch2Data"=w809:dbl[][], "V2"=w808:dbl[], "Ch3Data"=w807:dbl[][], "V3"=w806:dbl[], "Ch4Data"=w797:dbl[][], "V4"=w796:dbl[], "Pathes.CaliPath"=w815:path, "IDs.Cali ID"=w814:i8)
        n386 = Increment(x=w814) -> (x+1=w798:i8)
        n387 = Bundle("Ch1Data"=w811, "V1"=w810) -> (w805:cluster{"Ch1Data":dbl[][], "V1":dbl[]})  [unwired: 1 in]
        n388 = Bundle("Ch4Data"=w797, "V4"=w796) -> (w795:cluster{"Ch4Data":dbl[][], "V4":dbl[]})  [unwired: 1 in]
        n389 = Bundle("Ch2Data"=w809, "V2"=w808) -> (w804:cluster{"Ch2Data":dbl[][], "V2":dbl[]})  [unwired: 1 in]
        n390 = Bundle("Ch3Data"=w807, "V3"=w806) -> (w803:cluster{"Ch3Data":dbl[][], "V3":dbl[]})  [unwired: 1 in]
        n391 = Format Value(string ("")="Calibration" ("default name"), format string="%02d", value (0)=w798) -> (output string=w817:string)
        n392 = Build Path(base path=w815, name or relative path=w817) -> (appended path=w802:path)
        n393 = call "SaveBGorCali(SubVI).vi"("Channel1"=w805, "BG path"=w802, "DataType"=enum16{"BG", "Cali"}."Cali", "Channel 2"=w804, "Channel 3"=w803, "Channel 4"=w795, "error in (no error)"=w801, "SytemID"="UCDVetMed") -> ("error out"=w800:errorcluster)  [unwired: 7 in]
        n394 = call <vilib>:"Add State(s) to Queue__JKI_lib_State_Machine.vi"("State(s) in (\"\")"=w820) -> ("States Out"=w819:string)  [unwired: 14 in]
      }
      frame "Data: saveiRF" {
        w826 = enum16{"write", "read"}."read" ("action")
        # "Get iRF from decon stracture and save it on disk.\n(It is a separator no-op. You can make a copy of this frame to create a new Data frame)"
        n395 = Unbundle By Name(w843) -> ("TempPath"=w842:path)
        n396 = call "Ch1DeconEngineFGV.vi"("action(read)"=w826) -> ("Error Out"=w848:errorcluster, "Ch1DeconEngine out"=w849:refnum<class "LaguerreDeconEngineClass.lvclass">)  [unwired: 9 in]
        n397 = call "Ch2DeconEngineFGV.vi"("action(read)"=w826) -> ("Error Out"=w846:errorcluster, "Ch2DeconEngine out"=w847:refnum<class "LaguerreDeconEngineClass.lvclass">)  [unwired: 9 in]
        n398 = call "Ch3DeconEngineFGV.vi"("action(read)"=w826) -> ("Error Out"=w844:errorcluster, "Ch3DeconEngine out"=w845:refnum<class "LaguerreDeconEngineClass.lvclass">)  [unwired: 9 in]
        n399 = call "Ch4DeconEngineFGV.vi"("action(read)"=w826) -> ("Error Out"=w825:errorcluster, "Ch3DeconEngine out"=w824:refnum<class "LaguerreDeconEngineClass.lvclass">)  [unwired: 9 in]
        n400 = Build Path(base path=w842, name or relative path="iRF" ("default name")) -> (appended path=w840:path)
        n401 = call "getIRF.vi"("error in (no error)"=w825, "LaguerreDeconEngineClass in"=w824) -> ("iRF"=w823:dbl[])  [unwired: 7 in, 2 out]
        n402 = call "getIRF.vi"("error in (no error)"=w848, "LaguerreDeconEngineClass in"=w849) -> ("iRF"=w831:dbl[])  [unwired: 7 in, 2 out]
        n403 = call "getIRF.vi"("error in (no error)"=w846, "LaguerreDeconEngineClass in"=w847) -> ("iRF"=w830:dbl[])  [unwired: 7 in, 2 out]
        n404 = call "getIRF.vi"("error in (no error)"=w844, "LaguerreDeconEngineClass in"=w845) -> ("iRF"=w829:dbl[])  [unwired: 7 in, 2 out]
        n405 = TDMS Open(8:w839, 10:T19."create or replace" ("operation (0:open)"), 11:w840) -> (0:w836:errorcluster, 3:w837:refnum<k34>)  [unwired: 4 in]
        n406 = Bundle(cluster=T18 {"Ch1 iRF"=[], "Ch2 iRF"=[], "Ch3 iRF"=[], "Ch4 iRF"=[]} ("LastUseiRF"), "Ch1 iRF"=w831, "Ch2 iRF"=w830, "Ch3 iRF"=w829, "Ch4 iRF"=w823) -> (w827:T18)
        n407 = Build Array(w831, w830, w829, w823) -> (w835:dbl[][])
        n408 = global write "GlobalVariables.vi" "LastUseiRF"(w827) -> ()
        n409 = TDMS Write(0:w837, 5:"iRF" ("group name in (Untitled)"), 7:string[] ["Ch1", "Ch2", "Ch3", "Ch4"] ("channel name(s) in (Untitled)"), 9:w835, 11:w836) -> (4:w834:refnum<k34>, 15:w833:errorcluster)  [unwired: 1 in, 2 out]
        n410 = TDMS Close(8:w833, 11:w834) -> (0:w832:errorcluster)  [unwired: 1 out]
        n411 = call <vilib>:"Add State(s) to Queue__JKI_lib_State_Machine.vi"("State(s) in (\"\")"=w852) -> ("States Out"=w851:string)  [unwired: 14 in]
      }
      frame "Data: saveBGtoFGV" {
        w853 = enum16{"write", "read"}."write" ("action")
        # "Save BG and pass it to FGV.\n(save BG to disk and set it to FGV)"
        n412 = Unbundle By Name(w863) -> ("Ch1Data"=w862:dbl[][], "Ch2Data"=w861:dbl[][], "Ch3Data"=w860:dbl[][], "Ch4Data"=w855:dbl[][])
        n413 = call "AvgArrayTimeCritical.vi"("2D array"=w862) -> ("1D Avg"=w859:dbl[])  [unwired: 10 in]
        n414 = call "AvgArrayTimeCritical.vi"("2D array"=w861) -> ("1D Avg"=w858:dbl[])  [unwired: 10 in]
        n415 = call "AvgArrayTimeCritical.vi"("2D array"=w860) -> ("1D Avg"=w857:dbl[])  [unwired: 10 in]
        n416 = call "AvgArrayTimeCritical.vi"("2D array"=w855) -> ("1D Avg"=w854:dbl[])  [unwired: 10 in]
        n417 = call "BG1FGV.vi"("action"=w853, "BG1 in"=w859) -> ()  [unwired: 8 in, 2 out]
        n418 = call "BG2FGV.vi"("action"=w853, "BG2 in"=w858) -> ()  [unwired: 8 in, 2 out]
        n419 = call "BG3FGV.vi"("action"=w853, "BG3 in"=w857) -> ()  [unwired: 8 in, 2 out]
        n420 = call "BG4FGV.vi"("action"=w853, "BG4 in"=w854) -> ()  [unwired: 8 in, 2 out]
        n421 = call <vilib>:"Add State(s) to Queue__JKI_lib_State_Machine.vi"("State(s) in (\"\")"=w866) -> ("States Out"=w865:string)  [unwired: 14 in]
      }
      frame "Data: saveBGtoFile" {
        w888 = "Background" ("name or relative path")
        # "Save BG to file.\n(save BG to disk both data folder and temp folder)"
        n422 = Unbundle By Name(w892) -> ("Pathes.BG Path"=w885:path, "IDs.BG ID"=w884:i8, "Ch1Data"=w882:dbl[][], "V1"=w881:dbl[], "Ch2Data"=w880:dbl[][], "V2"=w879:dbl[], "Ch3Data"=w878:dbl[][], "V3"=w877:dbl[], "Ch4Data"=w869:dbl[][], "V4"=w868:dbl[], "TempPath"=w890:path)
        n423 = Increment(x=w884) -> (x+1=w889:i8)
        n424 = Format Value(string ("")=w888, format string="%02d", value (0)=w889) -> (output string=w887:string)
        n425 = Build Path(base path=w890, name or relative path=w888) -> (appended path=w871:path)
        n426 = call "File Dialog2"("start path"=w885, "prompt"="Please select BG name, DO NOT CANCEL!", "default name"=w887) -> ("selected path"=w872:path)  [unwired: 9 in, 3 out]
        n427 = Bundle("Ch1Data"=w882, "V1"=w881) -> (w876:cluster{"Ch1Data":dbl[][], "V1":dbl[]})  [unwired: 1 in]
        n428 = Bundle("Ch4Data"=w869, "V4"=w868) -> (w867:cluster{"Ch4Data":dbl[][], "V4":dbl[]})  [unwired: 1 in]
        n429 = Bundle("Ch2Data"=w880, "V2"=w879) -> (w875:cluster{"Ch2Data":dbl[][], "V2":dbl[]})  [unwired: 1 in]
        n430 = Bundle("Ch3Data"=w878, "V3"=w877) -> (w874:cluster{"Ch3Data":dbl[][], "V3":dbl[]})  [unwired: 1 in]
        n431 = Build Array(w872, w871) -> (w870:path[])
        n432 = for {
          tunnel: w876 -> [w903]
          tunnel: w875 -> [w902]
          tunnel: w874 -> [w901]
          shift-right: [w904] -> w883
          shift-left: w873 -> [w900]
          tunnel: w870 -> [w899] mode=indexing
          tunnel: w867 -> [w897]
          n433 = call "SaveBGorCali(SubVI).vi"("Channel1"=w903, "BG path"=w899, "DataType"=enum16{"BG", "Cali"}."BG", "Channel 2"=w902, "Channel 3"=w901, "Channel 4"=w897, "error in (no error)"=w900, "SytemID"="UCDVetMed") -> ("error out"=w904:errorcluster)  [unwired: 7 in]
        }
        n434 = call <vilib>:"Add State(s) to Queue__JKI_lib_State_Machine.vi"("State(s) in (\"\")"=w895) -> ("States Out"=w894:string)  [unwired: 14 in]
      }
      frame "Data: showBG" {
        # "Show BG in seperate window.\n()"
        n435 = call "showBG.vi"() -> ()  [unwired: 12 in]
        n436 = call <vilib>:"Add State(s) to Queue__JKI_lib_State_Machine.vi"("State(s) in (\"\")"=w909) -> ("States Out"=w908:string)  [unwired: 14 in]
      }
      frame "Data: irfAlignment" {
        w910 = enum16{"write", "read"}."write" ("action")
        # "do iRF alignment in this state\n(It is a separator no-op. You can make a copy of this frame to create a new Data frame)"
        n437 = Unbundle By Name(w955) -> ("Ch1Data"=w991:dbl[][], "Ch2Data"=w990:dbl[][], "Ch3Data"=w989:dbl[][], "Ch4Data"=w932:dbl[][])
        n438 = call "Ch1DeconEngineFGV.vi"("Error In"=w931) -> ("Error Out"=w987:errorcluster, "Ch1DeconEngine out"=w988:refnum<class "LaguerreDeconEngineClass.lvclass">)  [unwired: 9 in]
        n439 = call "Ch2DeconEngineFGV.vi"("Error In"=w931) -> ("Error Out"=w985:errorcluster, "Ch2DeconEngine out"=w986:refnum<class "LaguerreDeconEngineClass.lvclass">)  [unwired: 9 in]
        n440 = call "Ch3DeconEngineFGV.vi"("Error In"=w931) -> ("Error Out"=w983:errorcluster, "Ch3DeconEngine out"=w984:refnum<class "LaguerreDeconEngineClass.lvclass">)  [unwired: 9 in]
        n441 = call "Ch4DeconEngineFGV.vi"("Error In"=w931) -> ("Error Out"=w922:errorcluster, "Ch3DeconEngine out"=w921:refnum<class "LaguerreDeconEngineClass.lvclass">)  [unwired: 9 in]
        n442 = call "AvgArray.vi"("2D array in"=w990) -> ("1D Avg out"=w937:dbl[])  [unwired: 10 in]
        n443 = call "AvgArray.vi"("2D array in"=w989) -> ("1D Avg out"=w936:dbl[])  [unwired: 10 in]
        n444 = call "AvgArray.vi"("2D array in"=w932) -> ("1D Avg out"=w911:dbl[])  [unwired: 10 in]
        n445 = call "AvgArray.vi"("2D array in"=w991) -> ("1D Avg out"=w938:dbl[])  [unwired: 10 in]
        n446 = call "RemoveDCBG.vi"("WF in"=w938) -> ("DC"=w945:dbl, "WF out"=w935:dbl[])  [unwired: 8 in, 1 out]
        n447 = call "RemoveDCBG.vi"("WF in"=w937) -> ("DC"=w942:dbl, "WF out"=w948:dbl[])  [unwired: 8 in, 1 out]
        n448 = call "RemoveDCBG.vi"("WF in"=w936) -> ("DC"=w940:dbl, "WF out"=w947:dbl[])  [unwired: 8 in, 1 out]
        n449 = call "RemoveDCBG.vi"("WF in"=w911) -> ("DC"=w915:dbl, "WF out"=w913:dbl[])  [unwired: 8 in, 1 out]
        n450 = call "computeIRFAlignment.vi"("error in (no error)"=w987, "fIRF temp"=w935, "LaguerreDeconEngineClass in"=w988) -> ("error out"=w979:errorcluster, "LaguerreDeconEngineClass out"=w980:refnum<class "LaguerreDeconEngineClass.lvclass">)  [unwired: 6 in, 1 out]
        n451 = call "computeIRFAlignment.vi"("error in (no error)"=w985, "fIRF temp"=w948, "LaguerreDeconEngineClass in"=w986) -> ("error out"=w977:errorcluster, "LaguerreDeconEngineClass out"=w978:refnum<class "LaguerreDeconEngineClass.lvclass">)  [unwired: 6 in, 1 out]
        n452 = call "computeIRFAlignment.vi"("error in (no error)"=w983, "fIRF temp"=w947, "LaguerreDeconEngineClass in"=w984) -> ("error out"=w981:errorcluster, "LaguerreDeconEngineClass out"=w982:refnum<class "LaguerreDeconEngineClass.lvclass">)  [unwired: 6 in, 1 out]
        n453 = call "computeIRFAlignment.vi"("error in (no error)"=w922, "fIRF temp"=w913, "LaguerreDeconEngineClass in"=w921) -> ("error out"=w929:errorcluster, "LaguerreDeconEngineClass out"=w930:refnum<class "LaguerreDeconEngineClass.lvclass">)  [unwired: 6 in, 1 out]
        n454 = call "Ch1DeconEngineFGV.vi"("Error In"=w979, "action(read)"=w910, "Ch1DeconEngine in"=w980) -> ("Error Out"=w975:errorcluster, "Ch1DeconEngine out"=w976:refnum<class "LaguerreDeconEngineClass.lvclass">)  [unwired: 7 in]
        n455 = call "Ch2DeconEngineFGV.vi"("Error In"=w977, "action(read)"=w910, "Ch2DeconEngine in"=w978) -> ("Error Out"=w965:errorcluster, "Ch2DeconEngine out"=w966:refnum<class "LaguerreDeconEngineClass.lvclass">)  [unwired: 7 in]
        n456 = call "Ch3DeconEngineFGV.vi"("Error In"=w981, "action(read)"=w910, "Ch3DeconEngine in"=w982) -> ("Error Out"=w959:errorcluster, "Ch3DeconEngine out"=w960:refnum<class "LaguerreDeconEngineClass.lvclass">)  [unwired: 7 in]
        n457 = call "Ch4DeconEngineFGV.vi"("Error In"=w929, "action(read)"=w910, "Ch3DeconEngine in"=w930) -> ("Error Out"=w923:errorcluster, "Ch3DeconEngine out"=w924:refnum<class "LaguerreDeconEngineClass.lvclass">)  [unwired: 7 in]
        n458 = call "setfIRF.vi"("error in (no error)"=w959, "fIRF"=w947, "LaguerreDeconEngineClass in"=w960) -> ("error out"=w963:errorcluster, "LaguerreDeconEngineClass out"=w964:refnum<class "LaguerreDeconEngineClass.lvclass">)  [unwired: 7 in]
        n459 = call "setfIRF.vi"("error in (no error)"=w923, "fIRF"=w913, "LaguerreDeconEngineClass in"=w924) -> ("error out"=w927:errorcluster, "LaguerreDeconEngineClass out"=w928:refnum<class "LaguerreDeconEngineClass.lvclass">)  [unwired: 7 in]
        n460 = call "setfIRF.vi"("error in (no error)"=w965, "fIRF"=w948, "LaguerreDeconEngineClass in"=w966) -> ("error out"=w969:errorcluster, "LaguerreDeconEngineClass out"=w970:refnum<class "LaguerreDeconEngineClass.lvclass">)  [unwired: 7 in]
        n461 = call "setfIRF.vi"("error in (no error)"=w975, "fIRF"=w935, "LaguerreDeconEngineClass in"=w976) -> ("error out"=w973:errorcluster, "LaguerreDeconEngineClass out"=w974:refnum<class "LaguerreDeconEngineClass.lvclass">)  [unwired: 7 in]
        n462 = Unbundle By Name(w955) -> ("V1"=w934:dbl[], "V2"=w954:dbl[], "V3"=w953:dbl[], "V4"=w920:dbl[])
        n463 = call "computeLCs.vi"("error in (no error)"=w973, "LaguerreDeconClass in"=w974) -> ("error out"=w971:errorcluster, "LaguerreDeconClass out"=w972:refnum<class "LaguerreDeconEngineClass.lvclass">)  [unwired: 8 in]
        n464 = call "computeLCs.vi"("error in (no error)"=w969, "LaguerreDeconClass in"=w970) -> ("error out"=w967:errorcluster, "LaguerreDeconClass out"=w968:refnum<class "LaguerreDeconEngineClass.lvclass">)  [unwired: 8 in]
        n465 = call "computeLCs.vi"("error in (no error)"=w963, "LaguerreDeconClass in"=w964) -> ("error out"=w961:errorcluster, "LaguerreDeconClass out"=w962:refnum<class "LaguerreDeconEngineClass.lvclass">)  [unwired: 8 in]
        n466 = call "computeLCs.vi"("error in (no error)"=w927, "LaguerreDeconClass in"=w928) -> ("error out"=w925:errorcluster, "LaguerreDeconClass out"=w926:refnum<class "LaguerreDeconEngineClass.lvclass">)  [unwired: 8 in]
        n467 = call-poly <vilib>:"Mean.vi"("X"=w934) -> ("mean"=w933:dbl)  [unwired: 1 out]
        n468 = call-poly <vilib>:"Mean.vi"("X"=w920) -> ("mean"=w919:dbl)  [unwired: 1 out]
        n469 = call-poly <vilib>:"Mean.vi"("X"=w954) -> ("mean"=w952:dbl)  [unwired: 1 out]
        n470 = call "getFitting.vi"("error in (no error)"=w971, "LaguerreDeconEngineClass in"=w972) -> ("Fitting"=w944:dbl[])  [unwired: 7 in, 2 out]
        n471 = call "getFitting.vi"("error in (no error)"=w967, "LaguerreDeconEngineClass in"=w968) -> ("Fitting"=w941:dbl[])  [unwired: 7 in, 2 out]
        n472 = call "getFitting.vi"("error in (no error)"=w961, "LaguerreDeconEngineClass in"=w962) -> ("Fitting"=w917:dbl[])  [unwired: 7 in, 2 out]
        n473 = call "getFitting.vi"("error in (no error)"=w925, "LaguerreDeconEngineClass in"=w926) -> ("Fitting"=w916:dbl[])  [unwired: 7 in, 2 out]
        n474 = Add(x=w945, y=w944) -> (x+y=w946:dbl[])
        n475 = Add(x=w942, y=w941) -> (x+y=w943:dbl[])
        n476 = call-poly <vilib>:"Mean.vi"("X"=w953) -> ("mean"=w951:dbl)  [unwired: 1 out]
        n477 = Add(x=w940, y=w917) -> (x+y=w939:dbl[])
        n478 = Build Array(w938, w946) -> (w958:dbl[][])
        n479 = Build Array(w937, w943) -> (w957:dbl[][])
        n480 = Build Array(w936, w939) -> (w956:dbl[][])
        n481 = Add(x=w915, y=w916) -> (x+y=w914:dbl[])
        n482 = Bundle("mean"=w933, "mean"=w952, "mean"=w951, "mean"=w919) -> (w918:T42)  [unwired: 1 in]
        n483 = Build Array(w911, w914) -> (w912:dbl[][])
        n484 = call "Calib_and_iRFAlign_confirm.vi"("Current V"=w918, "Ch4 Data"=w912, "Ch3 Data"=w956, "Ch2 Data"=w957, "Ch1 Data"=w958) -> ("Save?"=w950:bool)  [unwired: 6 in]
        n485 = case shown="True" w950 {
          tunnel: ["" ("Empty String Constant") "Data: saveCalibration\nData: saveiRF\nRun: CaliIncrement"] -> w949
          frame False {
          }
          frame True {
            # "[Covers: REQ2]"
          }
        }
        n486 = call <vilib>:"Add State(s) to Queue__JKI_lib_State_Machine.vi"("State(s) in Front (\"\")"=w949, "State(s) in (\"\")"=w994) -> ("States Out"=w993:string)  [unwired: 13 in]
      }
      frame "Data: parseRunData" {
        # "All APD bias"
        # "flash queue"
        # "Ch3&4"
        # "Ch1&2"
        # "Flash data from queue and save it in structure\n()"
        n487 = Flush Queue(queue=w1022, error in (no error)=w1021) -> (remaining elements=w1016:T43, error out=w1017:errorcluster)  [unwired: 1 out]
        n488 = Flush Queue(queue=w1027, error in (no error)=w1021) -> (remaining elements=w1025:cluster{"double data":dbl[][]}[], error out=w1018:errorcluster)  [unwired: 1 out]
        n489 = Flush Queue(queue=w1028, error in (no error)=w1021) -> (remaining elements=w1026:cluster{"double data":dbl[][]}[], error out=w1019:errorcluster)  [unwired: 1 out]
        n490 = for {
          tunnel: w1026 -> [w1044] mode=indexing
          tunnel: [w1042] -> w1011 mode=concatenating
          tunnel: [w1041] -> w1012 mode=concatenating
          n491 = Unbundle By Name(w1044) -> ("double data"=w1043:dbl[][])
          n492 = call "SeperateChanData.vi"("Input (Ch1&2)"=w1043) -> ("Ch1"=w1042:dbl[][], "Ch2"=w1041:dbl[][])
        }
        n493 = for {
          tunnel: w1025 -> [w1040] mode=indexing
          tunnel: [w1039] -> w1001 mode=concatenating
          tunnel: [w1037] -> w1002 mode=concatenating
          n494 = Unbundle By Name(w1040) -> ("double data"=w1038:dbl[][])
          n495 = call "SeperateChanData.vi"("Input (Ch1&2)"=w1038) -> ("Ch1"=w1039:dbl[][], "Ch2"=w1037:dbl[][])
        }
        n496 = call "FLImDAQ_FGV.vi"() -> ("Read data"=w1009:T9)  [unwired: 10 in, 1 out]
        n497 = Unbundle By Name(w1009) -> ("Waveform to Avg"=w999:i16)
        n498 = for {
          tunnel: w1016 -> [w1036] mode=indexing
          tunnel: [w1035] -> w1008 mode=indexing
          tunnel: [w1034] -> w1006 mode=indexing
          tunnel: [w1033] -> w1004 mode=indexing
          tunnel: [w1032] -> w1000 mode=indexing
          n499 = Unbundle By Name(w1036) -> ("V1"=w1035:dbl, "V2"=w1034:dbl, "V3"=w1033:dbl, "V4"=w1032:dbl)
        }
        n500 = call "DuplicateV(SubVI).vi"("Averaging"=w999, "V in"=w1008) -> ("V out"=w1007:dbl[])  [unwired: 9 in]
        n501 = Array Size(array=w1001) -> (size(s)=→"data Size":i32[])
        n502 = call "DuplicateV(SubVI).vi"("Averaging"=w999, "V in"=w1006) -> ("V out"=w1005:dbl[])  [unwired: 9 in]
        n503 = call "DuplicateV(SubVI).vi"("Averaging"=w999, "V in"=w1004) -> ("V out"=w1003:dbl[])  [unwired: 9 in]
        n504 = call "DuplicateV(SubVI).vi"("Averaging"=w999, "V in"=w1000) -> ("V out"=w997:dbl[])  [unwired: 9 in]
        n505 = Bundle By Name(cluster=w1023, "Ch1Data"=w1011, "Ch2Data"=w1012, "Ch3Data"=w1001, "Ch4Data"=w1002, "V1"=w1007, "V2"=w1005, "V3"=w1003, "V4"=w997) -> (w1024:T29)
        n506 = Merge Errors(w1019, w1018, w1017) -> (w1020:errorcluster)
        n507 = Array Size(array=w1007) -> (size(s)=→"V1 Size":i32)
        n508 = Array Size(array=w1005) -> (size(s)=→"V2 Size":i32)
        n509 = Array Size(array=w1003) -> (size(s)=→"V3 Size":i32)
        n510 = Array Size(array=w997) -> (size(s)=→"V4 Size":i32)
        n511 = call <vilib>:"Add State(s) to Queue__JKI_lib_State_Machine.vi"("State(s) in (\"\")"=w1031) -> ("States Out"=w1030:string)  [unwired: 14 in]
      }
      frame "Data: saveRunData" {
        w1047 = T44 {"DataPath"=path "", "CaseID"="", "RunID"=0, "Ch1Data"=[], "Ch2Data"=[], "Ch3Data"=[], "Ch4Data"=[], "V1"=[], "V2"=[], "V3"=[], "V4"=[], "LaserRepRate"=0, "WFAverage"=0, "RunStartTime"=0}  # Data cluster
        # "Save FLIm data to disk.\n(Save to LV tdms file format)"
        n512 = Unbundle By Name(w1058) -> ("Pathes.DataPath"=w1054:path, "CaseID"=w1066:string, "IDs.RunID"=w1056:i8, "Ch1Data"=w1065:dbl[][], "Ch2Data"=w1064:dbl[][], "Ch3Data"=w1053:dbl[][], "Ch4Data"=w1046:dbl[][], "V1"=w1048:dbl[], "V2"=w1063:dbl[], "V3"=w1062:dbl[], "V4"=w1045:dbl[])
        n513 = call "FLImDAQ_FGV.vi"() -> ("Read data"=w1051:T9)  [unwired: 10 in, 1 out]
        n514 = Unbundle By Name(w1051) -> ("Waveform to Avg"=w1050:i16)
        n515 = local read "RunStartTime"() -> (w1049:u32)
        n516 = local read "Laser Rep Rate"() -> (w1052:dbl)
        n517 = Increment(x=w1056) -> (x+1=w1055:i8)
        n518 = Bundle By Name(cluster=w1047, "DataPath"=w1054, "CaseID"=w1066, "RunID"=w1055, "Ch1Data"=w1065, "Ch2Data"=w1064, "Ch3Data"=w1053, "Ch4Data"=w1046, "V1"=w1048, "V2"=w1063, "V3"=w1062, "V4"=w1045, "LaserRepRate"=w1052, "WFAverage"=w1050, "RunStartTime"=w1049) -> (w1061:T44)
        n519 = call "SaveRunData(SubVI).vi"("Data cluster"=w1061, "error in (no error)"=w1060) -> ("error out"=w1057:errorcluster)  [unwired: 13 in]
        n520 = flat-sequence {
          tunnel: w1058 -> [w1074]
          tunnel: [w1073] -> w1059
          tunnel: w1057 -> [_]
          frame #0 {
            w1071 = dbl[][] [] ("Ch1Data")
            w1072 = dbl[] [] ("V1")
            # "reset local data"
            n521 = Bundle By Name(cluster=w1074, "Ch1Data"=w1071, "Ch2Data"=w1071, "Ch3Data"=w1071, "Ch4Data"=w1071, "V1"=w1072, "V2"=w1072, "V3"=w1072, "V4"=w1072) -> (w1073:T29)
          }
        }
        n522 = case shown="No Error" w1057 {
          tunnel: ["Run: Increment" "" ("Empty String Constant")] -> w1067
          frame No Error {
          }
          frame Error {
          }
        }
        n523 = call <vilib>:"Add State(s) to Queue__JKI_lib_State_Machine.vi"("State(s) in Front (\"\")"=w1067, "State(s) in (\"\")"=w1070) -> ("States Out"=w1069:string)  [unwired: 13 in]
      }
      frame "Data: Cleanup" {
        # "Cleanup any data and references, here.\n(this is called automatically, by the Macro: Exit)"
        n524 = Unbundle By Name(w1078) -> ("Core.Current VI Reference"=w1081:refnum<vi>)
        n525 = Close Reference(reference=w1081, error in (no error)=w1080) -> (error out=w1079:errorcluster)
        n526 = call <vilib>:"Add State(s) to Queue__JKI_lib_State_Machine.vi"("State(s) in (\"\")"=w1083) -> ("States Out"=w1082:string)  [unwired: 14 in]
      }
      frame "---------- Core ----------" {
        # "Do not put any code in this frame.\n(it is a separator no-op)"
        n527 = call <vilib>:"Add State(s) to Queue__JKI_lib_State_Machine.vi"("State(s) in (\"\")"=w1088) -> ("States Out"=w1087:string)  [unwired: 14 in]
      }
      frame Default {
        w1099 = 42 items=["No error", "Argument error", "Memory is full", "Out of zone", "End of file", "File already open", "Generic file I/O error", "File not found", "File permission error", "Disk is full", "Duplicate path", "Too many files open", "System feature not enabled", "Resource file not found", "Cannot add resource", "Resource not found", "Image not found", "Image memory error", "Pen does not exist", "Config type invalid", "Config token not found", "Config parse error", "Config memory error", "Bad external code format", "Bad external code offset", "External code not present", "Null window", "Destroy window error", "Null menu", "Print aborted", "Bad print record", "Print driver error", "Windows error during printing", "Memory error during printing", "Print dialog error", "Generic print error", "Invalid device refnum", "Device not found", "Device parameter error", "Device unit error", "Cannot open device", "Device call aborted", "Generic error", "Cancelled by user", "Object ID too low", "Object ID too high", "Object not in heap", "Unknown heap", "Unknown object (invalid DefProc)", "Unknown object (DefProc not in table)", "Message out of range", "Invalid (null) method", "Unknown message", "Manager call not supported", "Bad address", "Network operation in progress", "Network operation timed out", "Connection is busy", "Network attribute not supported", "Network error", "Address in use", "System out of memory", "Connection aborted", "Connection refused", "Not connected", "Already connected", "Connection closed", "Initialization error (interapplication manager)", "Bad occurrence", "Wait on unbound occurrence handler", "Occurrence queue overflow", "Datalog type conflict", "Unused", "Unrecognized type (interapplication manager)", "Memory corrupt", "Failed to make temporary DLL", "Old CIN version", "Drag socket not found", "Failed to load drop-object", "Failed to register OLE object", "Failed to release OLE object", "Format specifier type mismatch", "Unknown format specifier", "Too few format specifiers", "Too many format specifiers", "Scan failed", "Newer CIN version", "Error converting to variant", "Runtime menu error", "Password tampered", "Variant attribute not found", "Incompatible variant data type", "Event data is not available", "Event Store is not present", "Occurrence is not found", "Event Queue is not created", "Event info is not available", "Refnum passed is NULL", "Error retrieving Class GUID", "Error retrieving CoClass GUID", "Error retrieving TypeLib GUID.", "Bad built application magic bytes.", "Specific driver is different from the specific driver associated with the Logical Name.", "There is no session opened to the class driver.", "Max Error", "MAX - Error with config objects", "MAX - Error loading configuration", "MAX - Group not supported"]
        # "Current State"
        # "Do not delete, rename, or modify this frame.\n(this is used to capture unhandled states and typos)"
        # "Handle mistyped state name (developer tool)"
        n528 = Format Into String(format string="Software Exception: Unhandled State \"%s\"." ("message"), error in=w1095, w1090) -> (resulting string=w1098:string, error out=w1097:errorcluster)  [unwired: 1 in]
        n529 = call <vilib>:"Error Cluster From Error Code.vi"("show call chain? (False)"=TRUE, "error in (no error)"=w1097, "error message (\"\")"=w1098, "error code (0)"=w1099) -> ("error out"=w1096:errorcluster)  [unwired: 5 in]
        n530 = call <vilib>:"Add State(s) to Queue__JKI_lib_State_Machine.vi"("State(s) in (\"\")"=w1094) -> ("States Out"=w1093:string)  [unwired: 14 in]
      }
      frame "Initialize Core Data" {
        # "Build default path based on the location of project"
        # "Do not delete, rename, or modify this frame.\n(this is used to determine panel behavior on exit)"
        # "originally closed?"
        # "exe?"
        # "If panel starts closed or is an EXE, then close it when we exit"
        n531 = call <vilib>:"Application Directory.vi"() -> ("Application Directory"=w1102:path)
        n532 = property on="Property Node" class="App"() -> ("App.Kind"=w1118:T21)  [unwired: 2 in, 2 out]
        n533 = property on="Property Node" class="VI"() -> ("FP.State"=w1112:T20)  [unwired: 2 in, 2 out]
        n534 = control-ref of="Current VI Reference"() -> (w1113:refnum<vi>)
        n535 = Equal?(x=w1112, y=T20."Closed" ("Front Panel Window:State")) -> (x = y?=w1110:bool)
        n536 = Strip Path(path=w1102) -> (stripped path=w1101:path)  [unwired: 1 out]
        n537 = Equal?(x=w1118, y=T21."Run Time System" ("Application:Kind")) -> (x = y?=w1116:bool)
        n538 = Build Path(base path=w1101, name or relative path="Data") -> (appended path=w1108:path)
        n539 = Build Path(base path=w1102, name or relative path="SystemTemp") -> (appended path=w1105:path)
        n540 = Build Path(base path=w1102, name or relative path="SystemCalibrationFile") -> (appended path=w1103:path)
        n541 = Or(x=w1110, y=w1116) -> (x .or. y?=w1114:bool)
        n542 = Bundle By Name(cluster=w1115, "Core.Current VI Reference"=w1113, "Core.Close Panel on Exit?"=w1114, "DefaultPath"=w1108, "TempPath"=w1105, "CaliPath"=w1103) -> (w1120:T29)
        n543 = call <vilib>:"Add State(s) to Queue__JKI_lib_State_Machine.vi"("State(s) in (\"\")"=w1122) -> ("States Out"=w1121:string)  [unwired: 14 in]
      }
      frame "Error Handler" {
        # "Unhandled Error -- Display it"
        # "Handle any errors here.\nYou can also output any states to clean-up after errors occur"
        # "Clear error"
        n544 = Unbundle By Name(w1123) -> ("code"=w1125:i32)
        n545 = case shown="Default" w1125 {
          tunnel: ["Macro: Exit" w1135 w1141] -> w1124
          tunnel: w1123 -> [w1131 _ _]
          frame Default {
            w1133 = T45 1 items=["no dialog", "OK message", "continue or stop message", "OK message + warnings", "continue/stop + warnings"] ("type of dialog (OK msg:1)")
            n546 = call <vilib>:"General Error Handler.vi"("type of dialog (OK msg:1)"=w1133, "error in (no error)"=w1131) -> ()  [unwired: 9 in, 5 out]
          }
          frame 5002 {
            n547 = Two Button Dialog(message="Laser interlock open! Please close interlock and try again! ", 1:"Safely Shutdown" ("F button name (\"Cancel\")"), 2:"OK" ("T button name (\"OK\")")) -> (T button?=w1136:bool)
            n548 = case shown="True" w1136 {
              tunnel: ["Macro: Exit" "355 Laser: CheckControllerStatus"] -> w1135
              frame False {
              }
              frame True {
              }
            }
          }
          frame 5001 {
            n549 = Two Button Dialog(message="Unable to connect to imaging computer, do you want to run data aquisiton alone? ", 1:"No" ("F button name (\"Cancel\")"), 2:"Yes" ("T button name (\"OK\")")) -> (T button?=w1142:bool)
            n550 = case shown="False" w1142 {
              tunnel: ["Macro: Exit" "" ("Empty String Constant")] -> w1141
              frame False {
              }
              frame True {
              }
            }
          }
        }
        n551 = call <vilib>:"Add State(s) to Queue__JKI_lib_State_Machine.vi"("State(s) in Front (\"\")"=w1124, "State(s) in (\"\")"=w1130) -> ("States Out"=w1129:string)  [unwired: 13 in]
      }
      frame "Exit" {
        # "Do not put any code in this frame.\n(No errors that occur here will be handled.)"
        n552 = call <vilib>:"Add State(s) to Queue__JKI_lib_State_Machine.vi"("State(s) in (\"\")"=w1153) -> ("States Out"=w1152:string)  [unwired: 14 in]
      }
      frame "---------- Case ----------" {
        # "Template Separator\n(You can make a copy of, or modify, this frame)"
        n553 = call <vilib>:"Add State(s) to Queue__JKI_lib_State_Machine.vi"("State(s) in (\"\")"=w1158) -> ("States Out"=w1157:string)  [unwired: 14 in]
      }
      frame "Case: getCaliID" {
        # "Get Calibration file #\n(You can make a copy of, or modify, this frame)"
        n554 = Unbundle By Name(w1159) -> ("Pathes.CaliPath"=w1162:path)
        n555 = call <vilib>:"Recursive File List.vi"("pattern"="*.tdms", "Treat LLBs as Folders?"=FALSE, "Folder Path"=w1162) -> ("All Files in Dir"=w1167:path[])  [unwired: 4 in, 4 out]
        n556 = for {
          tunnel: w1167 -> [w1177] mode=indexing
          tunnel: [w1176] -> w1166 mode=indexing
          tunnel: "Calibration" -> [w1173]
          n557 = Strip Path(path=w1177) -> (name=w1174:string)  [unwired: 1 out]
          n558 = Search and Replace String(input string=w1174, search string=w1173) -> (result string=w1172:string)  [unwired: 6 in, 3 out]
          n559 = Scan From String(format string="%d" ("string"), input string=w1172) -> (output 1=w1176:i32)  [unwired: 3 in, 3 out]
        }
        n560 = Array Max & Min(array=w1166) -> (max value=w1165:i32)  [unwired: 3 out]
        n561 = Bundle By Name(cluster=w1159, "IDs.Cali ID"=w1165) -> (w1160:T29)
        n562 = call <vilib>:"Add State(s) to Queue__JKI_lib_State_Machine.vi"("State(s) in (\"\")"=w1171) -> ("States Out"=w1170:string)  [unwired: 14 in]
      }
      frame "Case: getBGID" {
        # "Get background #\n(You can make a copy of, or modify, this frame)"
        n563 = Unbundle By Name(w1180) -> ("Pathes.BG Path"=w1185:path)
        n564 = call <vilib>:"Recursive File List.vi"("pattern"="*.tdms", "Treat LLBs as Folders?"=FALSE, "Folder Path"=w1185) -> ("All Files in Dir"=w1183:path[])  [unwired: 4 in, 4 out]
        n565 = for {
          tunnel: w1183 -> [w1200] mode=indexing
          tunnel: "Background" ("name or relative path") -> [w1198]
          shift-right: [w1191] -> w1178
          shift-left: 0 -> [w1195]
          n566 = Strip Path(path=w1200) -> (name=w1199:string)  [unwired: 1 out]
          n567 = Search and Replace String(input string=w1199, search string=w1198) -> (number of replacements=w1197:i32)  [unwired: 6 in, 3 out]
          n568 = Greater Than 0?(x=w1197) -> (x > 0?=w1196:bool)
          n569 = Select(t=1, s=w1196, f=0) -> (s? t:f=w1194:i32)
          n570 = Add(x=w1194, y=w1195) -> (x+y=w1191:i32)
        }
        n571 = Bundle By Name(cluster=w1180, "IDs.BG ID"=w1178) -> (w1181:T29)
        n572 = call <vilib>:"Add State(s) to Queue__JKI_lib_State_Machine.vi"("State(s) in (\"\")"=w1190) -> ("States Out"=w1189:string)  [unwired: 14 in]
      }
      frame "Case: getRunID" {
        # "Check folder for run ID\n(You can make a copy of, or modify, this frame)"
        n573 = Unbundle By Name(w1210) -> ("Pathes.DataPath"=w1209:path, "CaseID"=w1205:string)
        n574 = Build Array("Background" ("name or relative path"), "Calibration", "3DScanData" ("element")) -> (w1215:string[])
        n575 = call <vilib>:"Recursive File List.vi"("Folders to Exclude"=w1215, "pattern"="*.tdms", "Treat LLBs as Folders?"=FALSE, "Folder Path"=w1209) -> ("All Files in Dir"=w1206:path[])  [unwired: 3 in, 4 out]
        n576 = for {
          tunnel: w1206 -> [w1224] mode=indexing
          tunnel: [w1223] -> w1212 mode=indexing
          tunnel: w1205 -> [w1220]
          n577 = Strip Path(path=w1224) -> (name=w1221:string)  [unwired: 1 out]
          n578 = Search and Replace String(input string=w1221, search string=w1220) -> (result string=w1219:string)  [unwired: 6 in, 3 out]
          n579 = Scan From String(format string="_%d" ("string"), input string=w1219) -> (output 1=w1223:i32)  [unwired: 3 in, 3 out]
        }
        n580 = Array Max & Min(array=w1212) -> (max value=w1203:i32)  [unwired: 3 out]
        n581 = Bundle By Name(cluster=w1210, "IDs.RunID"=w1203) -> (w1211:T29)
        n582 = call "RunIDFGV.vi"("Error In"=w1201, "RunID in"=w1203) -> ("Error Out"=w1202:errorcluster)  [unwired: 8 in, 1 out]
        n583 = call <vilib>:"Add State(s) to Queue__JKI_lib_State_Machine.vi"("State(s) in (\"\")"=w1218) -> ("States Out"=w1217:string)  [unwired: 14 in]
      }
      frame "Case: CreatFileStruct" {
        # "Creat case file structure"
        n584 = Unbundle By Name(w1238) -> ("DefaultPath"=w1244:path, "CaseID"=w1231:string)
        n585 = Build Path(base path=w1244, name or relative path=w1231) -> (appended path=w1243:path)
        n586 = call <vilib>:"Check if File or Folder Exists.vi"("error in (no error)"=w1237, "path"=w1243) -> ("error out"=w1240:errorcluster, "file or folder exists?"=w1242:bool, "dup path"=w1241:path)  [unwired: 7 in]
        n587 = case shown="False" w1242 {
          tunnel: w1241 -> [w1261 w1269]
          tunnel: w1240 -> [w1259 w1264]
          tunnel: [w1253 w1269] -> w1229
          tunnel: [w1257 w1271] -> w1228
          tunnel: [u32 0 u32 0] -> w1227
          tunnel: [w1255 w1274] -> w1235
          tunnel: "Background" ("name or relative path") -> [w1254 w1266]
          tunnel: "Calibration" -> [w1252 w1265]
          tunnel: [w1248 w1267] -> w1232
          tunnel: w1231 -> [_ _]
          tunnel: ["" ("Empty String Constant") "Case: getRunID\nCase: getBGID\nCase: getCaliID\nUI: Update"] -> w1230
          frame False {
            # "Folder not exist. Creat folders."
            n588 = Create Folder(path (use dialog)=w1261, error in=w1259) -> (created path=w1253:path, error out=w1250:errorcluster)  [unwired: 1 in, 1 out]
            n589 = Build Path(base path=w1253, name or relative path=w1252) -> (appended path=w1251:path)
            n590 = Build Path(base path=w1253, name or relative path=w1254) -> (appended path=w1260:path)
            n591 = Create Folder(path (use dialog)=w1260, error in=w1250) -> (created path=w1255:path, error out=w1256:errorcluster)  [unwired: 1 in, 1 out]
            n592 = Create Folder(path (use dialog)=w1251, error in=w1250) -> (created path=w1248:path, error out=w1249:errorcluster)  [unwired: 1 in, 1 out]
            n593 = Merge Errors(w1256, w1249) -> (w1257:errorcluster)
          }
          frame True {
            # "Folder exsit, check file #"
            n594 = Build Path(base path=w1269, name or relative path=w1265) -> (appended path=w1270:path)
            n595 = Build Path(base path=w1269, name or relative path=w1266) -> (appended path=w1275:path)
            n596 = call <vilib>:"Check if File or Folder Exists.vi"("path"=w1270) -> ("file or folder exists?"=w1268:bool, "dup path"=w1267:path)  [unwired: 8 in, 1 out]
            n597 = call <vilib>:"Check if File or Folder Exists.vi"("path"=w1275) -> ("file or folder exists?"=w1273:bool, "dup path"=w1274:path)  [unwired: 8 in, 1 out]
            n598 = And(x=w1273, y=w1268) -> (x .and. y?=w1272:bool)
            n599 = case shown="False" w1272 {
              tunnel: w1264 -> [_ w1277]
              tunnel: [errorcluster {"status"=TRUE, "code"=5003, "source"="File structure error."} ("error out") w1277] -> w1271
              frame False {
              }
              frame True {
              }
            }
          }
        }
        n600 = Bundle By Name(cluster=w1238, "Pathes.DataPath"=w1229, "Pathes.BG Path"=w1235, "Pathes.CaliPath"=w1232, "IDs.RunID"=w1227, "IDs.BG ID"=w1227, "IDs.Cali ID"=w1227) -> (w1239:T29)
        n601 = call "DataRootPathFGV.vi"("Error In"=w1228, "PathIn"=w1229) -> ("Error Out"=w1226:errorcluster)  [unwired: 8 in, 1 out]
        n602 = call "RunIDFGV.vi"("Error In"=w1226, "RunID in"=w1227) -> ("Error Out"=w1225:errorcluster)  [unwired: 8 in, 1 out]
        n603 = call <vilib>:"Add State(s) to Queue__JKI_lib_State_Machine.vi"("State(s) in Front (\"\")"=w1230, "State(s) in (\"\")"=w1246) -> ("States Out"=w1245:string)  [unwired: 13 in]
      }
      frame "Case: GetID" {
        # "Template Separator\n(You can make a copy of, or modify, this frame)"
        n604 = call "set_subjectID.vi"() -> ("subject_id"=w1278:string)  [unwired: 10 in]
        n605 = Bundle By Name(cluster=w1280, "CaseID"=w1278) -> (w1281:T29)
        n606 = call <vilib>:"Add State(s) to Queue__JKI_lib_State_Machine.vi"("State(s) in (\"\")"=w1284) -> ("States Out"=w1283:string)  [unwired: 14 in]
      }
      frame "---------- DeconEngine ----------" {
        # "start data aquisition and then set irfAligh to ture and decon channel to 1,2 and 3."
        # "Template Separator\n(You can make a copy of, or modify, this frame)"
        n607 = call <vilib>:"Add State(s) to Queue__JKI_lib_State_Machine.vi"("State(s) in (\"\")"=w1289) -> ("States Out"=w1288:string)  [unwired: 14 in]
      }
      frame "DeconEngine: InitilizeMacro" {
        # "start data aquisition and then set irfAligh to ture and decon channel to 1,2 and 3."
        # "Initilize Decon Engine for all channel\n(You can make a copy of, or modify, this frame)"
        n608 = call <vilib>:"Add State(s) to Queue__JKI_lib_State_Machine.vi"("State(s) in Front (\"\")"="DeconEngine: InitializeCh1\nDeconEngine: InitializeCh2\nDeconEngine: InitializeCh3\nDeconEngine: InitializeCh4" ("State(s) in Front (\"\")"), "State(s) in (\"\")"=w1295) -> ("States Out"=w1294:string)  [unwired: 13 in]
      }
      frame "DeconEngine: InitializeCh1" {
        w1317 = refnum<class "LaguerreDeconEngineClass.lvclass"> refnum  # Ch1DeconObj
        # "Initilize Laguerre Deconvolution engine Object\n(You can make a copy of, or modify, this frame)"
        n609 = global read "GlobalVariables.vi" "LastUseiRF"() -> (w1298:T18)
        n610 = local read "Truncation"() -> (w1296:u32)
        n611 = call "setLaguerreOrder.vi"("error in (no error)"=w1305, "LaguerreOrder"=u32 12, "LaguerreDeconClass in"=w1317) -> ("error out"=w1314:errorcluster, "LaguerreDeconClass out"=w1315:refnum<class "LaguerreDeconEngineClass.lvclass">)  [unwired: 7 in]
        n612 = Unbundle By Name(w1298) -> ("Ch1 iRF"=w1297:dbl[])
        n613 = call "setDataLength.vi"("error in (no error)"=w1314, "dataLength"=w1296, "LaguerreDeconClass in"=w1315) -> ("error out"=w1313:errorcluster, "LaguerreDeconClass out"=w1312:refnum<class "LaguerreDeconEngineClass.lvclass">)  [unwired: 7 in]
        n614 = call "setIRF.vi"("error in (no error)"=w1313, "iRF"=w1297, "LaguerreDeconClass in"=w1312) -> ("error out"=w1310:errorcluster, "LaguerreDeconClass out"=w1311:refnum<class "LaguerreDeconEngineClass.lvclass">)  [unwired: 7 in]
        n615 = call "computeAlpha.vi"("error in (no error)"=w1310, "LaguerreDeconClass in"=w1311) -> ("error out"=w1308:errorcluster, "LaguerreDeconClass out"=w1309:refnum<class "LaguerreDeconEngineClass.lvclass">)  [unwired: 8 in]
        n616 = call "dataInitilize.vi"("error in (no error)"=w1308, "LaguerreDeconClass in"=w1309) -> ("error out"=w1306:errorcluster, "LaguerreDeconClass out"=w1307:refnum<class "LaguerreDeconEngineClass.lvclass">)  [unwired: 8 in]
        n617 = call "computeDeconMatrix.vi"("error in (no error)"=w1306, "LaguerreDeconClass in"=w1307) -> ("error out"=w1302:errorcluster, "LaguerreDeconClass out"=w1304:refnum<class "LaguerreDeconEngineClass.lvclass">)  [unwired: 8 in]
        n618 = call "Ch1DeconEngineFGV.vi"("Error In"=w1302, "action(read)"=enum16{"write", "read"}."write" ("action"), "Ch1DeconEngine in"=w1304) -> ("Error Out"=w1301:errorcluster)  [unwired: 7 in, 1 out]
        n619 = call <vilib>:"Add State(s) to Queue__JKI_lib_State_Machine.vi"("State(s) in (\"\")"=w1319) -> ("States Out"=w1318:string)  [unwired: 14 in]
      }
      frame "DeconEngine: InitializeCh2" {
        w1341 = refnum<class "LaguerreDeconEngineClass.lvclass"> refnum  # Ch2DeconObj
        # "Initilize Laguerre Deconvolution engine Object\n(You can make a copy of, or modify, this frame)"
        n620 = global read "GlobalVariables.vi" "LastUseiRF"() -> (w1322:T18)
        n621 = call "setLaguerreOrder.vi"("error in (no error)"=w1329, "LaguerreOrder"=u32 12, "LaguerreDeconClass in"=w1341) -> ("error out"=w1338:errorcluster, "LaguerreDeconClass out"=w1339:refnum<class "LaguerreDeconEngineClass.lvclass">)  [unwired: 7 in]
        n622 = local read "Truncation"() -> (w1320:u32)
        n623 = Unbundle By Name(w1322) -> ("Ch2 iRF"=w1321:dbl[])
        n624 = call "setDataLength.vi"("error in (no error)"=w1338, "dataLength"=w1320, "LaguerreDeconClass in"=w1339) -> ("error out"=w1337:errorcluster, "LaguerreDeconClass out"=w1336:refnum<class "LaguerreDeconEngineClass.lvclass">)  [unwired: 7 in]
        n625 = call "setIRF.vi"("error in (no error)"=w1337, "iRF"=w1321, "LaguerreDeconClass in"=w1336) -> ("error out"=w1334:errorcluster, "LaguerreDeconClass out"=w1335:refnum<class "LaguerreDeconEngineClass.lvclass">)  [unwired: 7 in]
        n626 = call "computeAlpha.vi"("error in (no error)"=w1334, "LaguerreDeconClass in"=w1335) -> ("error out"=w1332:errorcluster, "LaguerreDeconClass out"=w1333:refnum<class "LaguerreDeconEngineClass.lvclass">)  [unwired: 8 in]
        n627 = call "dataInitilize.vi"("error in (no error)"=w1332, "LaguerreDeconClass in"=w1333) -> ("error out"=w1330:errorcluster, "LaguerreDeconClass out"=w1331:refnum<class "LaguerreDeconEngineClass.lvclass">)  [unwired: 8 in]
        n628 = call "computeDeconMatrix.vi"("error in (no error)"=w1330, "LaguerreDeconClass in"=w1331) -> ("error out"=w1326:errorcluster, "LaguerreDeconClass out"=w1328:refnum<class "LaguerreDeconEngineClass.lvclass">)  [unwired: 8 in]
        n629 = call "Ch2DeconEngineFGV.vi"("Error In"=w1326, "action(read)"=enum16{"write", "read"}."write" ("action"), "Ch2DeconEngine in"=w1328) -> ("Error Out"=w1325:errorcluster)  [unwired: 7 in, 1 out]
        n630 = call <vilib>:"Add State(s) to Queue__JKI_lib_State_Machine.vi"("State(s) in (\"\")"=w1343) -> ("States Out"=w1342:string)  [unwired: 14 in]
      }
      frame "DeconEngine: InitializeCh3" {
        w1345 = refnum<class "LaguerreDeconEngineClass.lvclass"> refnum  # Ch3DeconObj
        # "Initilize Laguerre Deconvolution engine Object\n(You can make a copy of, or modify, this frame)"
        n631 = global read "GlobalVariables.vi" "LastUseiRF"() -> (w1347:T18)
        n632 = local read "Truncation"() -> (w1344:u32)
        n633 = call "setLaguerreOrder.vi"("error in (no error)"=w1354, "LaguerreOrder"=u32 12, "LaguerreDeconClass in"=w1345) -> ("error out"=w1363:errorcluster, "LaguerreDeconClass out"=w1364:refnum<class "LaguerreDeconEngineClass.lvclass">)  [unwired: 7 in]
        n634 = Unbundle By Name(w1347) -> ("Ch3 iRF"=w1346:dbl[])
        n635 = call "setDataLength.vi"("error in (no error)"=w1363, "dataLength"=w1344, "LaguerreDeconClass in"=w1364) -> ("error out"=w1362:errorcluster, "LaguerreDeconClass out"=w1361:refnum<class "LaguerreDeconEngineClass.lvclass">)  [unwired: 7 in]
        n636 = call "setIRF.vi"("error in (no error)"=w1362, "iRF"=w1346, "LaguerreDeconClass in"=w1361) -> ("error out"=w1359:errorcluster, "LaguerreDeconClass out"=w1360:refnum<class "LaguerreDeconEngineClass.lvclass">)  [unwired: 7 in]
        n637 = call "computeAlpha.vi"("error in (no error)"=w1359, "LaguerreDeconClass in"=w1360) -> ("error out"=w1357:errorcluster, "LaguerreDeconClass out"=w1358:refnum<class "LaguerreDeconEngineClass.lvclass">)  [unwired: 8 in]
        n638 = call "dataInitilize.vi"("error in (no error)"=w1357, "LaguerreDeconClass in"=w1358) -> ("error out"=w1355:errorcluster, "LaguerreDeconClass out"=w1356:refnum<class "LaguerreDeconEngineClass.lvclass">)  [unwired: 8 in]
        n639 = call "computeDeconMatrix.vi"("error in (no error)"=w1355, "LaguerreDeconClass in"=w1356) -> ("error out"=w1351:errorcluster, "LaguerreDeconClass out"=w1353:refnum<class "LaguerreDeconEngineClass.lvclass">)  [unwired: 8 in]
        n640 = call "Ch3DeconEngineFGV.vi"("Error In"=w1351, "action(read)"=enum16{"write", "read"}."write" ("action"), "Ch3DeconEngine in"=w1353) -> ("Error Out"=w1350:errorcluster)  [unwired: 7 in, 1 out]
        n641 = call <vilib>:"Add State(s) to Queue__JKI_lib_State_Machine.vi"("State(s) in (\"\")"=w1367) -> ("States Out"=w1366:string)  [unwired: 14 in]
      }
      frame "DeconEngine: InitializeCh4" {
        w1369 = refnum<class "LaguerreDeconEngineClass.lvclass"> refnum  # Ch3DeconObj
        # "Initilize Laguerre Deconvolution engine Object\n(You can make a copy of, or modify, this frame)"
        n642 = global read "GlobalVariables.vi" "LastUseiRF"() -> (w1371:T18)
        n643 = local read "Truncation"() -> (w1368:u32)
        n644 = call "setLaguerreOrder.vi"("error in (no error)"=w1378, "LaguerreOrder"=u32 12, "LaguerreDeconClass in"=w1369) -> ("error out"=w1387:errorcluster, "LaguerreDeconClass out"=w1388:refnum<class "LaguerreDeconEngineClass.lvclass">)  [unwired: 7 in]
        n645 = Unbundle By Name(w1371) -> ("Ch4 iRF"=w1370:dbl[])
        n646 = call "setDataLength.vi"("error in (no error)"=w1387, "dataLength"=w1368, "LaguerreDeconClass in"=w1388) -> ("error out"=w1386:errorcluster, "LaguerreDeconClass out"=w1385:refnum<class "LaguerreDeconEngineClass.lvclass">)  [unwired: 7 in]
        n647 = call "setIRF.vi"("error in (no error)"=w1386, "iRF"=w1370, "LaguerreDeconClass in"=w1385) -> ("error out"=w1383:errorcluster, "LaguerreDeconClass out"=w1384:refnum<class "LaguerreDeconEngineClass.lvclass">)  [unwired: 7 in]
        n648 = call "computeAlpha.vi"("error in (no error)"=w1383, "LaguerreDeconClass in"=w1384) -> ("error out"=w1381:errorcluster, "LaguerreDeconClass out"=w1382:refnum<class "LaguerreDeconEngineClass.lvclass">)  [unwired: 8 in]
        n649 = call "dataInitilize.vi"("error in (no error)"=w1381, "LaguerreDeconClass in"=w1382) -> ("error out"=w1379:errorcluster, "LaguerreDeconClass out"=w1380:refnum<class "LaguerreDeconEngineClass.lvclass">)  [unwired: 8 in]
        n650 = call "computeDeconMatrix.vi"("error in (no error)"=w1379, "LaguerreDeconClass in"=w1380) -> ("error out"=w1375:errorcluster, "LaguerreDeconClass out"=w1377:refnum<class "LaguerreDeconEngineClass.lvclass">)  [unwired: 8 in]
        n651 = call "Ch4DeconEngineFGV.vi"("Error In"=w1375, "action(read)"=enum16{"write", "read"}."write" ("action"), "Ch3DeconEngine in"=w1377) -> ("Error Out"=w1374:errorcluster)  [unwired: 7 in, 1 out]
        n652 = call <vilib>:"Add State(s) to Queue__JKI_lib_State_Machine.vi"("State(s) in (\"\")"=w1391) -> ("States Out"=w1390:string)  [unwired: 14 in]
      }
      frame "---------- Digitizer ----------" {
        # "Template Separator\n(You can make a copy of, or modify, this frame)"
        n653 = call <vilib>:"Add State(s) to Queue__JKI_lib_State_Machine.vi"("State(s) in (\"\")"=w1396) -> ("States Out"=w1395:string)  [unwired: 14 in]
      }
      frame "Digitizer: Initialize" {
        # "reset digitizer to everytime the system runs"
        # "reset digitizer to everytime the system runs"
        # "Initialize digitizer.\nInitialize both digitizer and update status."
        n654 = call "FLImDAQ_FGV.vi"("error in (no error)"=w1404) -> ("error out"=w1398:errorcluster, "Read data"=w1403:T9)  [unwired: 9 in]
        n655 = Unbundle By Name(w1406) -> ("SysConfigCluster.Ch1Enable?"=w1411:bool, "SysConfigCluster.Ch2Enable?"=w1410:bool, "SysConfigCluster.Ch3Enable?"=w1408:bool)
        n656 = Unbundle By Name(w1403) -> ("Digitizer 1"=w1399:refnum<k15>, "Digitizer 2"=w1402:refnum<k15>)
        n657 = property on="Digitizer" class="Bool (strict)"("Blinking"=TRUE) -> ()  [unwired: 2 in, 2 out]
        n658 = Or(x=w1411, y=w1410) -> (x .or. y?=w1409:bool)
        n659 = case shown="True" w1409 {
          tunnel: w1398 -> [w1419 w1422]
          tunnel: [w1419 w1421] -> w1400
          tunnel: w1399 -> [_ w1423]
          frame False {
          }
          frame True {
            n660 = call <instrlib>:"niScope Initialize.vi"("resource name"=w1423, "reset device"=TRUE, "error in"=w1422) -> ("error out"=w1421:errorcluster)  [unwired: 11 in, 1 out]
          }
        }
        n661 = case shown="True" w1408 {
          tunnel: w1398 -> [w1414 w1416]
          tunnel: [w1414 w1418] -> w1405
          tunnel: w1402 -> [_ w1417]
          frame False {
          }
          frame True {
            n662 = call <instrlib>:"niScope Initialize.vi"("resource name"=w1417, "reset device"=TRUE, "error in"=w1416) -> ("error out"=w1418:errorcluster)  [unwired: 11 in, 1 out]
          }
        }
        n663 = Merge Errors(w1400, w1405) -> (w1397:errorcluster)
        n664 = call <vilib>:"Add State(s) to Queue__JKI_lib_State_Machine.vi"("State(s) in (\"\")"=w1413) -> ("States Out"=w1412:string)  [unwired: 14 in]
      }
      frame "Digitizer: Config" {
        # "Synchronize is taking time ~3s."
        # "Config  digitizer\nCall subVi to config digitizer"
        n665 = call "FLImDAQ_FGV.vi"() -> ("Read data"=w1441:T9)  [unwired: 10 in, 1 out]
        n666 = Unbundle By Name(w1450) -> ("SysConfigCluster.Ch1Enable?"=w1458:bool, "SysConfigCluster.Ch2Enable?"=w1457:bool, "SysConfigCluster.Ch3Enable?"=w1455:bool, "FLImDAQ"=w1452:T36)
        n667 = Unbundle By Name(w1441) -> ("Digitizer 1"=w1444:refnum<k15>, "Digitizer 2"=w1443:refnum<k15>)
        n668 = property on="Digitizer" class="Bool (strict)"(error in=w1445, "Blinking"=TRUE) -> (error out=w1446:errorcluster)  [unwired: 1 in, 1 out]
        n669 = Or(x=w1458, y=w1457) -> (x .or. y?=w1456:bool)
        n670 = case shown="True" w1456 {
          tunnel: w1452 -> [_ w1471]
          tunnel: w1446 -> [w1467 w1470]
          tunnel: [w1467 w1469] -> w1453
          tunnel: w1444 -> [_ w1468]
          frame False {
          }
          frame True {
            n671 = call "DigitizerConfig.vi"("error in (no error)"=w1470, "FLImDAQ"=w1471, "IVI Refnum in"=w1468) -> ("error out"=w1469:errorcluster)  [unwired: 7 in, 1 out]
          }
        }
        n672 = case shown="True" w1455 {
          tunnel: w1452 -> [_ w1466]
          tunnel: w1453 -> [w1461 w1465]
          tunnel: [w1461 w1464] -> w1429
          tunnel: w1443 -> [_ w1462]
          frame False {
          }
          frame True {
            n673 = call "DigitizerConfig.vi"("Config Trigger? (T)"=FALSE ("Config Trigge(T)r:"), "error in (no error)"=w1465, "FLImDAQ"=w1466, "IVI Refnum in"=w1462) -> ("error out"=w1464:errorcluster)  [unwired: 6 in, 1 out]
          }
        }
        n674 = call "Digitizer1_FGV.vi"("error in (no error)"=w1429) -> ("error out"=w1439:errorcluster, "Read data"=w1440:refnum<k15>)  [unwired: 9 in]
        n675 = call <instrlib>:"niScope Get Session Reference.vi"("instrument handle"=w1440, "error in"=w1439) -> ("session reference"=w1433:refnum<k20>, "error out"=w1431:errorcluster)  [unwired: 11 in, 1 out]
        n676 = call "Digitizer2_FGV.vi"("error in (no error)"=w1431) -> ("error out"=w1437:errorcluster, "Read data"=w1438:refnum<k15>)  [unwired: 9 in]
        n677 = call <instrlib>:"niScope Get Session Reference.vi"("instrument handle"=w1438, "error in"=w1437) -> ("session reference"=w1432:refnum<k20>, "error out"=w1430:errorcluster)  [unwired: 11 in, 1 out]
        n678 = Build Array(w1433, w1432) -> (w1436:refnum<k20>[])
        n679 = call <instrlib>:"niTClk Configure For Homogeneous Triggers.vi"("error in (no error)"=w1430, "sessions"=w1436) -> ("error out"=w1435:errorcluster, "sessions out"=w1434:refnum<k20>[])  [unwired: 8 in]
        n680 = call <instrlib>:"niTClk Synchronize.vi"("error in (no error)"=w1435, "sessions"=w1434) -> ("error out"=w1428:errorcluster, "sessions out"=w1426:refnum<k20>[])  [unwired: 8 in]
        n681 = call <userlib>:"Wait (ms)__ogtk.vi"("error in (no error)"=w1428, "milliseconds to wait"=u32 1500) -> ("error out"=w1424:errorcluster)  [unwired: 8 in, 1 out]
        n682 = Unbundle By Name(w1424) -> ("status"=w1449:bool)
        n683 = Not(x=w1449) -> (.not. x?=w1448:bool)
        n684 = Bundle By Name(cluster=w1450, "System Status.Digitizer"=w1448, "niTClk sessions"=w1426) -> (w1451:T29)
        n685 = property on="Digitizer" class="Bool (strict)"(error in=w1424, "Blinking"=FALSE) -> (error out=w1442:errorcluster)  [unwired: 1 in, 1 out]
        n686 = call <vilib>:"Add State(s) to Queue__JKI_lib_State_Machine.vi"("State(s) in (\"\")"=w1460) -> ("States Out"=w1459:string)  [unwired: 14 in]
      }
      frame "Digitizer: Start" {
        # "send trigger to start acquisition loop"
        # "initilize aquisition"
        # "Start Digitizer\n(TClk start)"
        n687 = Unbundle By Name(w1479) -> ("niTClk sessions"=w1478:refnum<k20>[])
        n688 = call <instrlib>:"niTClk Initiate.vi"("error in (no error)"=w1472, "sessions"=w1478) -> ("error out"=w1474:errorcluster)  [unwired: 8 in, 1 out]
        n689 = Generate User Event(priority (normal)=usereventprio."high priority", user event=w1475, event data cluster=TRUE ("event data"), error in=w1474) -> (error out=w1473:errorcluster)  [unwired: 1 out]
        n690 = call <vilib>:"Add State(s) to Queue__JKI_lib_State_Machine.vi"("State(s) in (\"\")"=w1482) -> ("States Out"=w1481:string)  [unwired: 14 in]
      }
      frame "Digitizer: Abort" {
        # "Template Separator\n(You can make a copy of, or modify, this frame)"
        n691 = call "Digitizer1_FGV.vi"("error in (no error)"=w1486, "Operation (Read)"=enum16{"Write", "Read"}."Read" ("Operation")) -> ("error out"=w1493:errorcluster, "Read data"=w1490:refnum<k15>)  [unwired: 8 in]
        n692 = call "Digitizer2_FGV.vi"("error in (no error)"=w1486, "Operation (Read)"=enum16{"Write", "Read"}."Read" ("Operation")) -> ("error out"=w1489:errorcluster, "Read data"=w1491:refnum<k15>)  [unwired: 8 in]
        n693 = Bundle By Name(cluster=w1483, "SysRunning?"=FALSE ("System Status")) -> (w1484:T29)
        n694 = call <instrlib>:"niScope Abort.vi"("instrument handle"=w1490, "error in"=w1493) -> ("error out"=w1495:errorcluster)  [unwired: 12 in, 1 out]
        n695 = call <instrlib>:"niScope Abort.vi"("instrument handle"=w1491, "error in"=w1489) -> ("error out"=w1494:errorcluster)  [unwired: 12 in, 1 out]
        n696 = Merge Errors(w1495, w1494) -> (w1487:errorcluster)
        n697 = call <vilib>:"Add State(s) to Queue__JKI_lib_State_Machine.vi"("State(s) in (\"\")"=w1498) -> ("States Out"=w1497:string)  [unwired: 14 in]
      }
      frame "Digitizer: checkTemp" {
        w1501 = 65.0 ("y")
        w1506 = enum16{"Write", "Read"}."Read" ("Operation")
        # "Template Separator\n(You can make a copy of, or modify, this frame)"
        n698 = call "Digitizer1_FGV.vi"("Operation (Read)"=w1506) -> ("error out"=w1507:errorcluster, "Read data"=w1508:refnum<k15>)  [unwired: 9 in]
        n699 = call "Digitizer2_FGV.vi"("Operation (Read)"=w1506) -> ("error out"=w1504:errorcluster, "Read data"=w1505:refnum<k15>)  [unwired: 9 in]
        n700 = property on="Property Node" class="niScope"(reference=w1505, error in=w1504) -> ("Device Temperature"=w1502:dbl)  [unwired: 2 out]
        "Dig2 Temp" <- w1502
        n701 = property on="Property Node" class="niScope"(reference=w1508, error in=w1507) -> ("Device Temperature"=w1503:dbl)  [unwired: 2 out]
        "Dig1 Temp" <- w1503
        n702 = Greater?(x=w1503, y=w1501) -> (0:w1500:bool)
        n703 = Greater?(x=w1502, y=w1501) -> (0:w1499:bool)
        n704 = case shown="True" w1500 {
          frame False {
          }
          frame True {
            n705 = One Button Dialog(message="Digitizer 1 over heating!", button name ("OK")="OK") -> ()  [unwired: 1 out]
          }
        }
        n706 = case shown="True" w1499 {
          frame False {
          }
          frame True {
            n707 = One Button Dialog(message="Digitizer 2 over heating!", button name ("OK")="OK") -> ()  [unwired: 1 out]
          }
        }
        n708 = call <vilib>:"Add State(s) to Queue__JKI_lib_State_Machine.vi"("State(s) in (\"\")"=w1513) -> ("States Out"=w1512:string)  [unwired: 14 in]
      }
      frame "Digitizer: Close" {
        # "Close Digitizer"
        n709 = call "Digitizer1_FGV.vi"("error in (no error)"=w1523, "Operation (Read)"=enum16{"Write", "Read"}."Read" ("Operation")) -> ("error out"=w1525:errorcluster, "Read data"=w1529:refnum<k15>)  [unwired: 8 in]
        n710 = call "Digitizer2_FGV.vi"("error in (no error)"=w1523, "Operation (Read)"=enum16{"Write", "Read"}."Read" ("Operation")) -> ("error out"=w1524:errorcluster, "Read data"=w1527:refnum<k15>)  [unwired: 8 in]
        n711 = call <instrlib>:"niScope Close.vi"("instrument handle"=w1529, "error in"=w1525) -> ("error out"=w1522:errorcluster)  [unwired: 13 in]
        n712 = call <instrlib>:"niScope Close.vi"("instrument handle"=w1527, "error in"=w1524) -> ("error out"=w1521:errorcluster)  [unwired: 13 in]
        n713 = Merge Errors(w1522, w1521) -> (w1520:errorcluster)
        n714 = Unbundle By Name(w1520) -> ("status"=w1519:bool)
        n715 = Bundle By Name(cluster=w1530, "System Status.Digitizer"=w1519) -> (w1531:T29)
        n716 = call <vilib>:"Add State(s) to Queue__JKI_lib_State_Machine.vi"("State(s) in (\"\")"=w1533) -> ("States Out"=w1532:string)  [unwired: 14 in]
      }
      frame "---------- LabJack ----------" {
        # "Template Separator\n(You can make a copy of, or modify, this frame)"
        n717 = call <vilib>:"Add State(s) to Queue__JKI_lib_State_Machine.vi"("State(s) in (\"\")"=w1538) -> ("States Out"=w1537:string)  [unwired: 14 in]
      }
      frame "LabJack: checkPedal" {
        # "Template Separator\n(You can make a copy of, or modify, this frame)"
        n718 = Unbundle By Name(w1539) -> ("LJ Pinout.Foot Pedal"=w1543:string)
        n719 = call "LabJack_FGV.vi"("Operation(Read)"=enum16{"Write", "Read"}."Read" ("Operation"), "error in (no error)"=w1541) -> ("error out"=w1545:errorcluster, "Read data"=w1546:i32)  [unwired: 8 in]
        n720 = call "LJM_eReadName.vi"("Handle In"=w1546, "Name"=w1543, "error in"=w1545) -> ("Value"=w1544:dbl, "error out"=w1542:errorcluster)  [unwired: 10 in, 1 out]
        n721 = case shown="1" w1544 {
          tunnel: w1539 -> [w1551 w1554]
          tunnel: [w1551 w1552] -> w1540
          frame 0, Default {
          }
          frame 1 {
            # "If Pedal pressed"
            n722 = Tick Count (ms)() -> (millisecond timer value=w1558:u32)
            n723 = Unbundle By Name(w1554) -> ("Last Trigger"=w1553:u32)
            n724 = Subtract(x=w1558, y=w1553) -> (x-y=w1557:u32)
            n725 = Greater Or Equal?(x=w1557, y=u32 2000) -> (x >= y?=w1555:bool)
            n726 = case shown="True" w1555 {
              tunnel: w1554 -> [w1559 w1560]
              tunnel: w1553 -> [_ _]
              tunnel: [w1559 w1561] -> w1552
              frame False {
              }
              frame True {
                n727 = Tick Count (ms)() -> (millisecond timer value=w1562:u32)
                n728 = Unbundle By Name(w1560) -> ("SysRunning?"=w1563:bool)
                n729 = case shown="False" w1563 {
                  frame False {
                    n730 = property on="StartButton" class="Bool (strict)"("Val(Sgnl)"=TRUE ("Value (Signaling)")) -> ()  [unwired: 2 in, 2 out]
                  }
                  frame True {
                    n731 = property on="StopButton" class="Bool (strict)"("Val(Sgnl)"=TRUE ("Value (Signaling)")) -> ()  [unwired: 2 in, 2 out]
                  }
                }
                n732 = Bundle By Name(cluster=w1560, "Last Trigger"=w1562) -> (w1561:T29)
              }
            }
          }
        }
        n733 = call <vilib>:"Add State(s) to Queue__JKI_lib_State_Machine.vi"("State(s) in (\"\")"=w1550) -> ("States Out"=w1549:string)  [unwired: 14 in]
      }
      frame "LabJack: ZeroV" {
        # "Just Zero V\nDO not update FGV and front panel\nWIll resume from last V"
        # "set bias to 0"
        # "Zero APD bias\n(You can make a copy of, or modify, this frame)"
        n734 = Unbundle By Name(w1568) -> ("LJ Pinout.Ch1 Bias"=w1573:string, "LJ Pinout.Ch2 Bias"=w1572:string, "LJ Pinout.Ch3 Bias"=w1571:string)
        n735 = Build Array(w1573, w1572, w1571) -> (w1570:string[])
        n736 = call "LabJack_FGV.vi"("Operation(Read)"=enum16{"Write", "Read"}."Read" ("Operation"), "error in (no error)"=w1567) -> ("error out"=w1574:errorcluster, "Read data"=w1575:i32)  [unwired: 8 in]
        n737 = call "LJM_eWriteNames.vi"("Handle In"=w1575, "aNames"=w1570, "aValuesIn"=dbl[] [0.0, 0.0, 0.0], "error in"=w1574) -> ("error out"=w1566:errorcluster)  [unwired: 9 in, 2 out]
        n738 = call <vilib>:"Add State(s) to Queue__JKI_lib_State_Machine.vi"("State(s) in (\"\")"=w1579) -> ("States Out"=w1578:string)  [unwired: 14 in]
      }
      frame "LabJack: SetV" {
        w1586 = enum16{"write", "read"}."read" ("action (write)")
        # "set bias to user specifid"
        # "Set APD bias\n(You can make a copy of, or modify, this frame)"
        n739 = Unbundle By Name(w1595) -> ("LJ Pinout.Ch1 Bias"=w1599:string, "LJ Pinout.Ch2 Bias"=w1598:string, "LJ Pinout.Ch3 Bias"=w1597:string, "LJ Pinout.Ch4 Bias"=w1589:string)
        n740 = call "V2FGV.vi"("Error In"=w1585, "action(write)"=w1586) -> ("Error Out"=w1583:errorcluster, "V2 out"=w1591:dbl)  [unwired: 8 in]
        n741 = call "V4FGV.vi"("Error In"=w1585, "action(write)"=w1586) -> ("Error Out"=w1581:errorcluster, "V3 out"=w1587:dbl)  [unwired: 8 in]
        n742 = call "V1FGV.vi"("Error In"=w1585, "action (write)"=w1586) -> ("Error Out"=w1584:errorcluster, "V1 out"=w1588:dbl)  [unwired: 8 in]
        n743 = call "V3FGV.vi"("Error In"=w1585, "action(write)"=w1586) -> ("Error Out"=w1582:errorcluster, "V3 out"=w1590:dbl)  [unwired: 8 in]
        n744 = local write "V 3"(w1590) -> ()
        n745 = local write "V 2"(w1591) -> ()
        n746 = local write "V 4"(w1587) -> ()
        n747 = local write "V 1"(w1588) -> ()
        n748 = Build Array(w1599, w1598, w1597, w1589) -> (w1596:string[])
        n749 = call "LabJack_FGV.vi"("Operation(Read)"=enum16{"Write", "Read"}."Read" ("Operation"), "error in (no error)"=w1585) -> ("error out"=w1600:errorcluster, "Read data"=w1601:i32)  [unwired: 8 in]
        n750 = Build Array(w1588, w1591, w1590, w1587) -> (w1592:dbl[])
        n751 = call "LJM_eWriteNames.vi"("Handle In"=w1601, "aNames"=w1596, "aValuesIn"=w1592, "error in"=w1600) -> ("error out"=w1593:errorcluster)  [unwired: 9 in, 2 out]
        n752 = Merge Errors(w1584, w1583, w1582, w1581) -> (w1580:errorcluster)
        n753 = call <vilib>:"Add State(s) to Queue__JKI_lib_State_Machine.vi"("State(s) in (\"\")"=w1605) -> ("States Out"=w1604:string)  [unwired: 14 in]
        n754 = Merge Errors(w1580, w1593) -> (w1594:errorcluster)
      }
      frame "LabJack: Open" {
        # "Initialize LabJack T7\nEstablish connection and initialize pins"
        n755 = call "LJ_Open.vi"("error in"=w1615, "DeviceType"="LJM_dtT7") -> ("error out"=w1612:errorcluster, "Success?"=w1613:bool, "Handle Out"=w1607:i32)  [unwired: 7 in]
        n756 = call "LabJack_FGV.vi"("Operation(Read)"=enum16{"Write", "Read"}."Write" ("Operation"), "error in (no error)"=w1612, "Write data"=w1607) -> ("error out"=w1609:errorcluster)  [unwired: 7 in, 1 out]
        n757 = Bundle By Name(cluster=w1610, "System Status.Labjack"=w1613) -> (w1614:T29)
        n758 = call <vilib>:"Add State(s) to Queue__JKI_lib_State_Machine.vi"("State(s) in (\"\")"=w1617) -> ("States Out"=w1616:string)  [unwired: 14 in]
      }
      frame "LabJack: SetDefaultSub" {
        w1627 = enum16{"write", "read"}."write" ("action")
        w1628 = 0.0 ("V1 in")
        w1641 = "_EF_ENABLE" ("string")
        # "1. Disable PWM\n2. Set all V to 0\n3. Set 355 relay to open\n4. Set LED to off"
        # "read once to set DIO to input"
        # "set all initila V to 0. Set footpedal to input. Set PWM to low. Set laser relay to open. Set LEDs to yellow."
        # "Set Labjack to correct input and output state and initial values"
        n759 = disable-structure shown="Disabled" {
          frame Disabled {
            (unwired) dbl[] [0.0, 0.0, 0.0, 0.0, 0.0, 0.0, 0.0, 0.0, 0.0] ("aValuesIn")
          }
          frame Enabled {
          }
        }
        n760 = Unbundle By Name(w1638) -> ("LJ Pinout.355 PWM"=w1643:string, "LJ Pinout.AimingBeam PWM"=w1642:string, "LJ Pinout.Ch1 Bias"=w1648:string, "LJ Pinout.Ch2 Bias"=w1618:string, "LJ Pinout.Ch3 Bias"=w1652:string, "LJ Pinout.Ch4 Bias"=w1632:string, "LJ Pinout.Laser Start/Stop"=w1651:string, "LJ Pinout.Red LED"=w1650:string, "LJ Pinout.Green LED"=w1649:string)
        n761 = call "V1FGV.vi"("Error In"=w1636, "action (write)"=w1627, "V1 in"=w1628) -> ("Error Out"=w1631:errorcluster, "V1 out"=w1635:dbl)  [unwired: 7 in]
        n762 = local write "V 1"(w1635) -> ()
        n763 = call "V2FGV.vi"("Error In"=w1631, "action(write)"=w1627, "V2 in"=w1628) -> ("Error Out"=w1630:errorcluster, "V2 out"=w1634:dbl)  [unwired: 7 in]
        n764 = call "LabJack_FGV.vi"("Operation(Read)"=enum16{"Write", "Read"}."Read" ("Operation"), "error in (no error)"=w1636) -> ("error out"=w1624:errorcluster, "Read data"=w1646:i32)  [unwired: 8 in]
        n765 = Concatenate Strings(w1643, w1641) -> (w1640:string)
        n766 = Concatenate Strings(w1642, w1641) -> (w1639:string)
        n767 = local write "V 2"(w1634) -> ()
        n768 = call "V3FGV.vi"("Error In"=w1630, "action(write)"=w1627, "V3 in"=w1628) -> ("Error Out"=w1629:errorcluster, "V3 out"=w1633:dbl)  [unwired: 7 in]
        n769 = Build Array(w1640, w1639, w1648, w1618, w1652, w1632, w1651, w1650, w1649) -> (w1622:string[])
        n770 = local write "V 3"(w1633) -> ()
        n771 = call "V4FGV.vi"("Error In"=w1629, "action(write)"=w1627, "V3 in"=w1628) -> ("Error Out"=w1625:errorcluster, "V3 out"=w1626:dbl)  [unwired: 7 in]
        n772 = Array Size(array=w1622) -> (size(s)=w1621:i32)
        n773 = local write "V 4"(w1626) -> ()
        n774 = Initialize Array(0.0 ("element"), w1621) -> (w1619:dbl[])
        n775 = Unbundle By Name(w1638) -> ("LJ Pinout.Foot Pedal"=w1637:string)
        n776 = call "LJM_eWriteNames.vi"("Handle In"=w1646, "aNames"=w1622, "aValuesIn"=w1619, "error in"=w1624) -> ("Handle Out"=w1645:i32, "error out"=w1644:errorcluster)  [unwired: 9 in, 1 out]
        n777 = call "LJM_eReadName.vi"("Handle In"=w1645, "Name"=w1637, "error in"=w1644) -> ("error out"=w1623:errorcluster)  [unwired: 10 in, 2 out]
        n778 = case shown="Error .." w1623 {
          frame No Error {
            # "no error"
          }
          frame Error {
            # "handle error"
            n779 = One Button Dialog(message="Labjack error! The pin assignment is likely wrong. Please check pin setting of Labjack. Program will terminate.", button name ("OK")="OK") -> ()  [unwired: 1 out]
          }
        }
        n780 = call <vilib>:"Add State(s) to Queue__JKI_lib_State_Machine.vi"("State(s) in (\"\")"=w1655) -> ("States Out"=w1654:string)  [unwired: 14 in]
      }
      frame "LabJack: FootPedalConfig" {
        # "Setup footPedal\n(You can make a copy of, or modify, this frame)"
        n781 = call "LabJack_FGV.vi"("Operation(Read)"=enum16{"Write", "Read"}."Read" ("Operation"), "error in (no error)"=w1659) -> ("error out"=w1663:errorcluster, "Read data"=w1664:i32)  [unwired: 8 in]
        n782 = call "LJM_eWriteName.vi"("Handle In"=w1664, "Name"="DIO15", "Value"=1.0, "error in"=w1663) -> ("error out"=w1660:errorcluster)  [unwired: 10 in, 1 out]
        n783 = call <vilib>:"Add State(s) to Queue__JKI_lib_State_Machine.vi"("State(s) in (\"\")"=w1668) -> ("States Out"=w1667:string)  [unwired: 14 in]
      }
      frame "LabJack: SetDefaultAndClose" {
        # "Template Separator\n(You can make a copy of, or modify, this frame)"
        n784 = call <vilib>:"Add State(s) to Queue__JKI_lib_State_Machine.vi"("State(s) in Front (\"\")"="LabJack: SetDefaultSub\nLabJack: Close" ("State(s) in Front (\"\")"), "State(s) in (\"\")"=w1674) -> ("States Out"=w1673:string)  [unwired: 13 in]
      }
      frame "LabJack: Close" {
        # "Close LabJack Refnum"
        n785 = call "LabJack_FGV.vi"("Operation(Read)"=enum16{"Write", "Read"}."Read" ("Operation"), "error in (no error)"=w1680) -> ("error out"=w1675:errorcluster, "Read data"=w1676:i32)  [unwired: 8 in]
        n786 = Bundle By Name(cluster=w1678, "System Status.Labjack"=FALSE ("System Status.Gain Control")) -> (w1681:T29)
        n787 = call "LJM_Close.vi"("error in"=w1675, "Handle"=w1676) -> ("error out"=w1683:errorcluster)  [unwired: 9 in]
        n788 = call <vilib>:"Add State(s) to Queue__JKI_lib_State_Machine.vi"("State(s) in (\"\")"=w1685) -> ("States Out"=w1684:string)  [unwired: 14 in]
      }
      frame "LabJack: Interlock enable/disable" {
        w1694 = i8 0  # int8
        # "[Covers: REQ8]"
        # "Interlock enable/disable\n(Usage: \"LabJack: Interlock enable/disable >> 1|0\")"
        n789 = Fract/Exp String To Number(string=w1695, default (0 dbl)=w1694) -> (number=w1691:i8)  [unwired: 2 in, 1 out]
        n790 = Unbundle By Name(w1693) -> ("LJ Pinout.Interlock"=w1692:string)
        n791 = call "LabJack_FGV.vi"("Operation(Read)"=enum16{"Write", "Read"}."Read" ("Operation")) -> ("Read data"=w1689:i32)  [unwired: 9 in, 1 out]
        n792 = call "LJM_eWriteName.vi"("Handle In"=w1689, "Name"=w1692, "Value"=w1691, "error in"=w1690) -> ("error out"=w1687:errorcluster)  [unwired: 10 in, 1 out]
        n793 = call <vilib>:"Add State(s) to Queue__JKI_lib_State_Machine.vi"("State(s) in (\"\")"=w1697) -> ("States Out"=w1696:string)  [unwired: 14 in]
      }
      frame "LabJack: 355_PWM_Config" {
        w1699 = 0.0 ("element")
        w1719 = "DIO_EF_CLOCK1_ENABLE"
        # "Config PWM frequency"
        n794 = Unbundle By Name(w1711) -> ("LJ Pinout.355 PWM"=w1718:string)
        n795 = Unbundle By Name(w1711) -> ("355 PWM setting.DIO_EF_CLOCK1_DIVISOR"=w1710:i16, "355 PWM setting.DIO_EF_CLOCK1_ROLL_VALUE"=w1709:i32, "355 PWM setting.DIO#_EF_INDEX"=w1706:i16, "355 PWM setting.DIO#_EF_OPTIONS"=w1705:i16, "355 PWM setting.DIO#_EF_CONFIG_A"=w1704:i32)
        n796 = Concatenate Strings(w1718, "_EF_ENABLE" ("string")) -> (w1714:string)
        n797 = Concatenate Strings(w1718, "_EF_INDEX") -> (w1717:string)
        n798 = Concatenate Strings(w1718, "_EF_OPTIONS") -> (w1716:string)
        n799 = Concatenate Strings(w1718, "_EF_CONFIG_A") -> (w1715:string)
        n800 = call "LabJack_FGV.vi"("Operation(Read)"=enum16{"Write", "Read"}."Read" ("Operation")) -> ("Read data"=w1712:i32)  [unwired: 9 in, 1 out]
        n801 = Build Array(w1699, w1699, w1710, w1709, 1.0 ("element"), 0.0 ("element"), w1706, w1705, w1704) -> (w1703:dbl[])
        n802 = Build Array("DIO_EF_CLOCK0_ENABLE", w1719, "DIO_EF_CLOCK1_DIVISOR", "DIO_EF_CLOCK1_ROLL_VALUE", w1719, w1714, w1717, w1716, w1715) -> (w1713:string[])
        n803 = call "LJM_eWriteNames.vi"("Handle In"=w1712, "aNames"=w1713, "aValuesIn"=w1703, "error in"=w1701) -> ("error out"=w1702:errorcluster)  [unwired: 9 in, 2 out]
        n804 = call <vilib>:"Add State(s) to Queue__JKI_lib_State_Machine.vi"("State(s) in (\"\")"=w1728) -> ("States Out"=w1727:string)  [unwired: 14 in]
      }
      frame "LabJack: 355_PWM_Start" {
        # "Template Separator\n(You can make a copy of, or modify, this frame)"
        n805 = Unbundle By Name(w1736) -> ("LJ Pinout.355 PWM"=w1735:string)
        n806 = call "LabJack_FGV.vi"("Operation(Read)"=enum16{"Write", "Read"}."Read" ("Operation"), "error in (no error)"=w1730) -> ("error out"=w1737:errorcluster, "Read data"=w1738:i32)  [unwired: 8 in]
        n807 = Concatenate Strings(w1735, "_EF_ENABLE" ("string")) -> (w1733:string)
        n808 = call "LJM_eWriteName.vi"("Handle In"=w1738, "Name"=w1733, "Value"=1.0, "error in"=w1737) -> ("error out"=w1731:errorcluster)  [unwired: 10 in, 1 out]
        n809 = call <vilib>:"Add State(s) to Queue__JKI_lib_State_Machine.vi"("State(s) in (\"\")"=w1741) -> ("States Out"=w1740:string)  [unwired: 14 in]
      }
      frame "LabJack: 355_PWM_Stop" {
        # "Template Separator\n(You can make a copy of, or modify, this frame)"
        n810 = Unbundle By Name(w1747) -> ("LJ Pinout.355 PWM"=w1751:string)
        n811 = call "LabJack_FGV.vi"("Operation(Read)"=enum16{"Write", "Read"}."Read" ("Operation"), "error in (no error)"=w1746) -> ("error out"=w1752:errorcluster, "Read data"=w1744:i32)  [unwired: 8 in]
        n812 = Concatenate Strings(w1751, "_EF_ENABLE" ("string")) -> (w1749:string)
        n813 = call "LJM_eWriteName.vi"("Handle In"=w1744, "Name"=w1749, "Value"=0.0, "error in"=w1752) -> ("error out"=w1743:errorcluster)  [unwired: 10 in, 1 out]
        n814 = local write "355nm Laser toggle"(FALSE ("355nm Laser toggle")) -> ()
        n815 = call <vilib>:"Add State(s) to Queue__JKI_lib_State_Machine.vi"("State(s) in (\"\")"=w1755) -> ("States Out"=w1754:string)  [unwired: 14 in]
      }
      frame "LabJack: AB_Start" {
        # "Aiming Beam Start\n(Based on aimging beam frequency, set LabJack pin)"
        n816 = Unbundle By Name(w1765) -> ("AB Cluster.Freq"=w1757:i32, "LJ Pinout.AimingBeam PWM"=w1764:string)
        n817 = Greater Than 0?(x=w1757) -> (x > 0?=w1756:bool)
        n818 = case shown="False" w1756 {
          tunnel: w1764 -> [w1771 w1774]
          tunnel: [w1771 w1772] -> w1763
          frame False {
            # "if 0 freq, set PWM pin"
          }
          frame True {
            # "if non zero freq, set PWM enable"
            n819 = Concatenate Strings(w1774, "_EF_ENABLE" ("string")) -> (w1772:string)
          }
        }
        n820 = call "LabJack_FGV.vi"("Operation(Read)"=enum16{"Write", "Read"}."Read" ("Operation"), "error in (no error)"=w1760) -> ("error out"=w1766:errorcluster, "Read data"=w1767:i32)  [unwired: 8 in]
        n821 = call "LJM_eWriteName.vi"("Handle In"=w1767, "Name"=w1763, "Value"=1.0, "error in"=w1766) -> ("error out"=w1761:errorcluster)  [unwired: 10 in, 1 out]
        n822 = local write "Aiming beam toggle"(TRUE ("Aiming beam toggle")) -> ()
        n823 = call <vilib>:"Add State(s) to Queue__JKI_lib_State_Machine.vi"("State(s) in (\"\")"=w1770) -> ("States Out"=w1769:string)  [unwired: 14 in]
      }
      frame "LabJack: AB_Stop" {
        # "Aiming Beam Stop\n(Based on aiming beam frequency, set LabJack pin low)"
        n824 = Unbundle By Name(w1782) -> ("AB Cluster.Freq"=w1777:i32, "LJ Pinout.AimingBeam PWM"=w1784:string)
        n825 = Greater Than 0?(x=w1777) -> (x > 0?=w1776:bool)
        n826 = case shown="False" w1776 {
          tunnel: w1784 -> [w1790 w1793]
          tunnel: [w1790 w1791] -> w1775
          frame False {
          }
          frame True {
            n827 = Concatenate Strings(w1793, "_EF_ENABLE" ("string")) -> (w1791:string)
          }
        }
        n828 = call "LabJack_FGV.vi"("Operation(Read)"=enum16{"Write", "Read"}."Read" ("Operation"), "error in (no error)"=w1780) -> ("error out"=w1785:errorcluster, "Read data"=w1786:i32)  [unwired: 8 in]
        n829 = call "LJM_eWriteName.vi"("Handle In"=w1786, "Name"=w1775, "Value"=0.0, "error in"=w1785) -> ("error out"=w1781:errorcluster)  [unwired: 10 in, 1 out]
        n830 = local write "Aiming beam toggle"(FALSE ("Aiming beam toggle")) -> ()
        n831 = call <vilib>:"Add State(s) to Queue__JKI_lib_State_Machine.vi"("State(s) in (\"\")"=w1789) -> ("States Out"=w1788:string)  [unwired: 14 in]
      }
      frame "LabJack: AB_PWM_Config" {
        w1795 = 0.0 ("element")
        w1815 = "DIO_EF_CLOCK2_ENABLE"
        # "Config PWM frequency"
        n832 = Unbundle By Name(w1807) -> ("LJ Pinout.AimingBeam PWM"=w1814:string)
        n833 = Unbundle By Name(w1807) -> ("AB PWM setting.DIO_EF_CLOCK1_DIVISOR"=w1806:i16, "AB PWM setting.DIO_EF_CLOCK1_ROLL_VALUE"=w1805:i32, "AB PWM setting.DIO#_EF_INDEX"=w1802:i16, "AB PWM setting.DIO#_EF_OPTIONS"=w1801:i16, "AB PWM setting.DIO#_EF_CONFIG_A"=w1800:i32)
        n834 = Concatenate Strings(w1814, "_EF_ENABLE" ("string")) -> (w1810:string)
        n835 = Concatenate Strings(w1814, "_EF_INDEX") -> (w1813:string)
        n836 = Concatenate Strings(w1814, "_EF_OPTIONS") -> (w1812:string)
        n837 = Concatenate Strings(w1814, "_EF_CONFIG_A") -> (w1811:string)
        n838 = call "LabJack_FGV.vi"("Operation(Read)"=enum16{"Write", "Read"}."Read" ("Operation")) -> ("Read data"=w1808:i32)  [unwired: 9 in, 1 out]
        n839 = Build Array(w1795, w1795, w1806, w1805, 1.0 ("element"), 0.0 ("element"), w1802, w1801, w1800) -> (w1799:dbl[])
        n840 = Build Array("DIO_EF_CLOCK0_ENABLE", w1815, "DIO_EF_CLOCK2_DIVISOR", "DIO_EF_CLOCK2_ROLL_VALUE", w1815, w1810, w1813, w1812, w1811) -> (w1809:string[])
        n841 = call "LJM_eWriteNames.vi"("Handle In"=w1808, "aNames"=w1809, "aValuesIn"=w1799, "error in"=w1797) -> ("error out"=w1798:errorcluster)  [unwired: 9 in, 2 out]
        n842 = call <vilib>:"Add State(s) to Queue__JKI_lib_State_Machine.vi"("State(s) in (\"\")"=w1824) -> ("States Out"=w1823:string)  [unwired: 14 in]
      }
      frame "---------- LED ----------" {
        # "Template Separator\n(You can make a copy of, or modify, this frame)"
        n843 = call <vilib>:"Add State(s) to Queue__JKI_lib_State_Machine.vi"("State(s) in (\"\")"=w1829) -> ("States Out"=w1828:string)  [unwired: 14 in]
      }
      frame "LED: OpenVIRef" {
        # "Template Separator\n(You can make a copy of, or modify, this frame)"
        n844 = call <vilib>:"Application Directory.vi"() -> ("Application Directory"=w1836:path)
        n845 = Build Path(base path=w1836, name or relative path="SubVI") -> (appended path=w1834:path)
        n846 = Build Path(base path=w1834, name or relative path="LEDBreath.vi") -> (appended path=w1832:path)
        n847 = Open VI Reference(vi path=w1832, error in (no error)=w1837) -> (vi reference=w1838:refnum<vi>, error out=w1831:errorcluster)  [unwired: 4 in]
        n848 = case shown="Error .." w1831 {
          tunnel: [TRUE FALSE] -> w1830
          frame No Error {
          }
          frame Error {
          }
        }
        n849 = Bundle By Name(cluster=w1839, "LED vi reference"=w1838, "LED vi ref open?"=w1830) -> (w1840:T29)
        n850 = call <vilib>:"Add State(s) to Queue__JKI_lib_State_Machine.vi"("State(s) in (\"\")"=w1843) -> ("States Out"=w1842:string)  [unwired: 14 in]
      }
      frame "LED: CloseVIRef" {
        # "Template Separator\n(You can make a copy of, or modify, this frame)"
        n851 = Unbundle By Name(w1847) -> ("LED vi reference"=w1848:refnum<vi>, "LED vi ref open?"=w1846:bool)
        n852 = case shown="True" w1846 {
          tunnel: w1850 -> [w1854 w1857]
          tunnel: [w1854 w1856] -> w1849
          tunnel: w1848 -> [_ w1855]
          frame False {
          }
          frame True {
            n853 = Close Reference(reference=w1855, error in (no error)=w1857) -> (error out=w1856:errorcluster)
          }
        }
        n854 = call <vilib>:"Add State(s) to Queue__JKI_lib_State_Machine.vi"("State(s) in (\"\")"=w1853) -> ("States Out"=w1852:string)  [unwired: 14 in]
      }
      frame "LED: BreathGreen" {
        w1858 = FALSE ("Wait Until Done")
        # "Breath system LED\n(LED: Breath >> True/False)"
        n855 = Unbundle By Name(w1866) -> ("LED vi reference"=w1865:refnum<vi>)
        n856 = invoke class="VI" method="Ctrl Val.Set"(reference=w1865, error in=w1863, "Control Name"="Color", "Value"=0) -> (reference out=w1862:refnum<vi>, error out=w1861:errorcluster)  [unwired: 1 in, 3 out]
        n857 = invoke on="Invoke Node" class="VI" method="Run VI"(reference=w1862, error in=w1861, "Wait until done"=w1858, "Auto Dispose Ref"=w1858) -> (error out=w1864:errorcluster)  [unwired: 1 in, 4 out]
        n858 = call <vilib>:"Add State(s) to Queue__JKI_lib_State_Machine.vi"("State(s) in (\"\")"=w1869) -> ("States Out"=w1868:string)  [unwired: 14 in]
      }
      frame "LED: BreathOrange" {
        w1870 = FALSE ("Wait Until Done")
        # "Breath system LED\n(LED: Breath >> True/False)"
        n859 = Unbundle By Name(w1878) -> ("LED vi reference"=w1877:refnum<vi>)
        n860 = invoke class="VI" method="Ctrl Val.Set"(reference=w1877, error in=w1875, "Control Name"="Color", "Value"=1) -> (reference out=w1874:refnum<vi>, error out=w1873:errorcluster)  [unwired: 1 in, 3 out]
        n861 = invoke on="Invoke Node" class="VI" method="Run VI"(reference=w1874, error in=w1873, "Wait until done"=w1870, "Auto Dispose Ref"=w1870) -> (error out=w1876:errorcluster)  [unwired: 1 in, 4 out]
        n862 = call <vilib>:"Add State(s) to Queue__JKI_lib_State_Machine.vi"("State(s) in (\"\")"=w1881) -> ("States Out"=w1880:string)  [unwired: 14 in]
      }
      frame "LED: BreathOff" {
        # "System LED Breath Off\n(Breath off, check VI status to make sure it is off)"
        n863 = Unbundle By Name(w1890) -> ("LED vi reference"=w1889:refnum<vi>)
        n864 = invoke on="Invoke Node" class="VI" method="Ctrl Val.Set"(reference=w1889, error in=w1887, "Control Name"="Stop", "Value"=TRUE) -> (reference out=w1882:refnum<vi>, error out=w1883:errorcluster)  [unwired: 1 in, 3 out]
        n865 = case shown="No Error" w1883 {
          selector: w1883 -> [w1895 _]
          tunnel: [w1894 errorcluster {"status"=FALSE, "code"=0, "source"=""} ("error IO")] -> w1888
          tunnel: ["" ("State(s) in Front (\"\")") "LED: BreathOff" ("State(s) in Front (\"\")")] -> w1886
          tunnel: w1882 -> [w1896 _]
          frame No Error {
            # "No error, wait for VI to stop"
            n866 = while {
              tunnel: w1896 -> [w1904]
              shift-right: [w1898] -> w1894
              shift-left: w1895 -> [w1903]
              stop <- w1900 stop-if-true
              # "continue check whether vi is running"
              n867 = property class="VI"(reference=w1904, error in=w1903) -> (error out=w1898:errorcluster, "Exec.State"=w1902:T23)  [unwired: 1 out]
              n868 = Wait (ms)(milliseconds to wait=u32 50) -> ()  [unwired: 1 out]
              n869 = Equal?(x=w1902, y=T23."Idle") -> (x = y?=w1900:bool)
            }
          }
          frame Error {
            # "try again when error"
          }
        }
        n870 = call <vilib>:"Add State(s) to Queue__JKI_lib_State_Machine.vi"("State(s) in Front (\"\")"=w1886, "State(s) in (\"\")"=w1893) -> ("States Out"=w1892:string)  [unwired: 13 in]
      }
      frame "LED: Off" {
        # "set LED to red"
        # "Template Separator\n(You can make a copy of, or modify, this frame)"
        n871 = Unbundle By Name(w1909) -> ("LJ Pinout.Red LED"=w1908:string, "LJ Pinout.Green LED"=w1907:string)
        n872 = call "LabJack_FGV.vi"("Operation(Read)"=enum16{"Write", "Read"}."Read" ("Operation"), "error in (no error)"=w1910) -> ("error out"=w1917:errorcluster, "Read data"=w1916:i32)  [unwired: 8 in]
        n873 = call "LJM_eWriteName.vi"("Handle In"=w1916, "Name"=w1908, "Value"=0.0, "error in"=w1917) -> ("Handle Out"=w1914:i32, "error out"=w1913:errorcluster)  [unwired: 10 in]
        n874 = call "LJM_eWriteName.vi"("Handle In"=w1914, "Name"=w1907, "Value"=0.0, "error in"=w1913) -> ("error out"=w1911:errorcluster)  [unwired: 10 in, 1 out]
        n875 = call <vilib>:"Add State(s) to Queue__JKI_lib_State_Machine.vi"("State(s) in (\"\")"=w1921) -> ("States Out"=w1920:string)  [unwired: 14 in]
      }
      frame "LED: Green" {
        # "set LED to green"
        # "Template Separator\n(You can make a copy of, or modify, this frame)"
        n876 = Unbundle By Name(w1925) -> ("LJ Pinout.Red LED"=w1923:string, "LJ Pinout.Green LED"=w1924:string)
        n877 = call "LabJack_FGV.vi"("Operation(Read)"=enum16{"Write", "Read"}."Read" ("Operation"), "error in (no error)"=w1927) -> ("error out"=w1933:errorcluster, "Read data"=w1932:i32)  [unwired: 8 in]
        n878 = call "LJM_eWriteName.vi"("Handle In"=w1932, "Name"=w1923, "Value"=0.0, "error in"=w1933) -> ("Handle Out"=w1930:i32, "error out"=w1929:errorcluster)  [unwired: 10 in]
        n879 = call "LJM_eWriteName.vi"("Handle In"=w1930, "Name"=w1924, "Value"=9.0, "error in"=w1929) -> ("error out"=w1926:errorcluster)  [unwired: 10 in, 1 out]
        n880 = call <vilib>:"Add State(s) to Queue__JKI_lib_State_Machine.vi"("State(s) in (\"\")"=w1936) -> ("States Out"=w1935:string)  [unwired: 14 in]
      }
      frame "---------- Queue ----------" {
        # "Template Separator\n(You can make a copy of, or modify, this frame)"
        n881 = call <vilib>:"Add State(s) to Queue__JKI_lib_State_Machine.vi"("State(s) in (\"\")"=w1941) -> ("States Out"=w1940:string)  [unwired: 14 in]
      }
      frame "Queue: Flash" {
        # "Clear queue contnet\n(clear queue content by flash it)"
        n882 = Flush Queue(queue=w1948, error in (no error)=w1942) -> (error out=w1946:errorcluster)  [unwired: 2 out]
        n883 = Flush Queue(queue=w1949, error in (no error)=w1942) -> (error out=w1945:errorcluster)  [unwired: 2 out]
        n884 = Flush Queue(queue=w1947, error in (no error)=w1942) -> (error out=w1944:errorcluster)  [unwired: 2 out]
        n885 = Merge Errors(w1946, w1945, w1944) -> (w1943:errorcluster)
        n886 = call <vilib>:"Add State(s) to Queue__JKI_lib_State_Machine.vi"("State(s) in (\"\")"=w1953) -> ("States Out"=w1952:string)  [unwired: 14 in]
      }
      frame "Queue: Destory" {
        # "Destory Data Queue\nDistory data queue ref so the aquisition loop stop"
        n887 = Release Queue(queue=w1961, error in (no error)=w1955) -> (error out=w1964:errorcluster)  [unwired: 1 in, 2 out]
        n888 = Release Queue(queue=w1960, error in (no error)=w1955) -> (error out=w1963:errorcluster)  [unwired: 1 in, 2 out]
        n889 = Release Queue(queue=w1958, error in (no error)=w1955) -> (error out=w1957:errorcluster)  [unwired: 1 in, 2 out]
        n890 = Release Notifier(notifier=w1956, error in (no error)=w1955) -> (error out=w1954:errorcluster)  [unwired: 1 in, 2 out]
        n891 = Merge Errors(w1964, w1963, w1957, w1954) -> (w1962:errorcluster)
        n892 = call <vilib>:"Simple Error Handler.vi"("error in (no error)"=w1962) -> ()  [unwired: 4 in, 5 out]
        n893 = call <vilib>:"Add State(s) to Queue__JKI_lib_State_Machine.vi"("State(s) in (\"\")"=w1967) -> ("States Out"=w1966:string)  [unwired: 14 in]
      }
      frame "---------- Run ----------" {
        # "Template Separator\n(You can make a copy of, or modify, this frame)"
        n894 = call <vilib>:"Add State(s) to Queue__JKI_lib_State_Machine.vi"("State(s) in (\"\")"=w1972) -> ("States Out"=w1971:string)  [unwired: 14 in]
      }
      frame "Run: CaliIncrement" {
        # "Increment Calibration #\n(You can make a copy of, or modify, this frame)"
        n895 = Unbundle By Name(w1974) -> ("IDs.Cali ID"=w1976:i8)
        n896 = Increment(x=w1976) -> (x+1=w1973:i8)
        n897 = Bundle By Name(cluster=w1974, "IDs.Cali ID"=w1973) -> (w1975:T29)
        n898 = call <vilib>:"Add State(s) to Queue__JKI_lib_State_Machine.vi"("State(s) in (\"\")"=w1980) -> ("States Out"=w1979:string)  [unwired: 14 in]
      }
      frame "Run: BGIncrement" {
        # "Increment BG #\n(You can make a copy of, or modify, this frame)"
        n899 = Unbundle By Name(w1981) -> ("IDs.BG ID"=w1984:i8)
        n900 = Increment(x=w1984) -> (x+1=w1983:i8)
        n901 = Bundle By Name(cluster=w1981, "IDs.BG ID"=w1983) -> (w1982:T29)
        n902 = call <vilib>:"Add State(s) to Queue__JKI_lib_State_Machine.vi"("State(s) in (\"\")"=w1988) -> ("States Out"=w1987:string)  [unwired: 14 in]
      }
      frame "Run: Increment" {
        # "Increase Run# by 1"
        n903 = Unbundle By Name(w1993) -> ("IDs.RunID"=w1995:i8)
        n904 = Increment(x=w1995) -> (x+1=w1991:i8)
        n905 = Bundle By Name(cluster=w1993, "IDs.RunID"=w1991) -> (w1994:T29)
        n906 = call "RunIDFGV.vi"("Error In"=w1989, "RunID in"=w1991) -> ("Error Out"=w1990:errorcluster)  [unwired: 8 in, 1 out]
        n907 = call <vilib>:"Add State(s) to Queue__JKI_lib_State_Machine.vi"("State(s) in (\"\")"=w1997) -> ("States Out"=w1996:string)  [unwired: 14 in]
      }
      frame "Run: Decrement" {
        # "Increase Run# by 1"
        n908 = Unbundle By Name(w2002) -> ("IDs.RunID"=w2004:i8)
        n909 = Decrement(x=w2004) -> (x-1=w2000:i8)
        n910 = Bundle By Name(cluster=w2002, "IDs.RunID"=w2000) -> (w2003:T29)
        n911 = call "RunIDFGV.vi"("Error In"=w1998, "RunID in"=w2000) -> ("Error Out"=w1999:errorcluster)  [unwired: 8 in, 1 out]
        n912 = call <vilib>:"Add State(s) to Queue__JKI_lib_State_Machine.vi"("State(s) in (\"\")"=w2006) -> ("States Out"=w2005:string)  [unwired: 14 in]
      }
      frame "---------- SysConfig ----------" {
        # "Template Separator\n(You can make a copy of, or modify, this frame)"
        n913 = call <vilib>:"Add State(s) to Queue__JKI_lib_State_Machine.vi"("State(s) in (\"\")"=w2011) -> ("States Out"=w2010:string)  [unwired: 14 in]
      }
      frame "SysConfig: LoadAPDSerialNumber" {
        # "Template Separator\n(You can make a copy of, or modify, this frame)"
        n914 = call "readAPDSerial.vi"("Error In"=w2013) -> ("Error Out"=w2012:errorcluster, "output cluster"=w2014:T32)  [unwired: 9 in]
        n915 = Bundle By Name(cluster=w2015, "APDSerialNum"=w2014) -> (w2016:T29)
        n916 = call <vilib>:"Add State(s) to Queue__JKI_lib_State_Machine.vi"("State(s) in (\"\")"=w2019) -> ("States Out"=w2018:string)  [unwired: 14 in]
      }
      frame "SysConfig: Load Sys Config" {
        # "[Covers: REQ5]"
        # "Load System config"
        # "Load system configuration\n(Load both hardware and DAQ config)"
        n917 = call "LoadSysConfig.vi"("Error In"=w2022, "Enum"=enum16{"LastUse", "Default"}."LastUse") -> ("Error Out"=w2021:errorcluster, "SysConfigCluster"=w2024:T7)  [unwired: 8 in]
        "SysConfigCluster" <- w2024
        n918 = Bundle By Name(cluster=w2025, "SysConfigCluster"=w2024) -> (w2026:T29)
        n919 = call <vilib>:"Add State(s) to Queue__JKI_lib_State_Machine.vi"("State(s) in (\"\")"=w2028) -> ("States Out"=w2027:string)  [unwired: 14 in]
      }
      frame "SysConfig: Load Digitizer Setting" {
        w2029 = enum16{"Write", "Read"}."Write" ("Operation")
        # "Load DAQ config\nSave to FGV"
        # "Template Separator\n(You can make a copy of, or modify, this frame)"
        n920 = call <userlib>:"Current VIs Parent Directory__ogtk.vi"() -> ("Parent Directory (+ Relative)"=w2043:path)  [unwired: 5 in]
        n921 = Build Path(base path=w2043, name or relative path="SubVI\\DigitizerConfiguration\\V6_Scope_last_use.config") -> (appended path=w2044:path)
        n922 = call "ReadDigitizerConfig(SubVI).vi"("error in (no error)"=w2041, "appended path"=w2044) -> ("error out"=w2037:errorcluster, "FLImDAQ"=w2035:T9)  [unwired: 8 in]
        n923 = call "FLImDAQ_FGV.vi"("error in (no error)"=w2037, "Operation (Read)"=w2029, "Write data"=w2035) -> ("error out"=w2039:errorcluster)  [unwired: 7 in, 1 out]
        n924 = Unbundle By Name(w2035) -> ("min record length"=→"data length":i32, "Digitizer 1"=w2031:refnum<k15>, "Digitizer 2"=w2038:refnum<k15>)
        n925 = Bundle By Name(cluster=w2033, "FLImDAQ"=w2035) -> (w2034:T29)
        n926 = call "Digitizer1_FGV.vi"("error in (no error)"=w2039, "Operation (Read)"=w2029, "Write data"=w2031) -> ("error out"=w2040:errorcluster)  [unwired: 7 in, 1 out]
        n927 = call "Digitizer2_FGV.vi"("error in (no error)"=w2040, "Operation (Read)"=w2029, "Write data"=w2038) -> ("error out"=w2036:errorcluster)  [unwired: 7 in, 1 out]
        n928 = call <vilib>:"Add State(s) to Queue__JKI_lib_State_Machine.vi"("State(s) in (\"\")"=w2046) -> ("States Out"=w2045:string)  [unwired: 14 in]
      }
      frame "SysConfig: Load LJ Pinout" {
        # "Template Separator\n(You can make a copy of, or modify, this frame)"
        n929 = call <userlib>:"Current VIs Parent Directory__ogtk.vi"() -> ("Parent Directory (+ Relative)"=w2061:path)  [unwired: 5 in]
        n930 = Build Path(base path=w2061, name or relative path="SubVI\\LabJack\\LJ_pin_setting.config") -> (appended path=w2059:path)
        n931 = call "ReadLabjackConfig(SubVI).vi"("error in (no error)"=w2057, "appended path"=w2059) -> ("error out"=w2058:errorcluster, "Utility"=w2055:T8)  [unwired: 8 in]
        n932 = Unbundle By Name(w2055) -> ("Ch1 Bias"=w2054:string, "Ch2 Bias"=w2053:string, "Ch3 Bias"=w2052:string, "Ch4 Bias"=w2047:string, "Red LED"=w2049:string, "Green LED"=w2048:string)
        n933 = global write "GlobalVariables.vi" "LED Green pin"(w2048) -> ()
        n934 = global write "GlobalVariables.vi" "Ch1 LJ pin"(w2054) -> ()
        n935 = global write "GlobalVariables.vi" "Ch2 LJ pin"(w2053) -> ()
        n936 = global write "GlobalVariables.vi" "Ch3 LJ pin"(w2052) -> ()
        n937 = global write "GlobalVariables.vi" "Ch4 LJ pin"(w2047) -> ()
        n938 = global write "GlobalVariables.vi" "LED Red pin"(w2049) -> ()
        n939 = Bundle By Name(cluster=w2050, "LJ Pinout"=w2055) -> (w2056:T29)
        n940 = call <vilib>:"Add State(s) to Queue__JKI_lib_State_Machine.vi"("State(s) in (\"\")"=w2063) -> ("States Out"=w2062:string)  [unwired: 14 in]
      }
      frame "SysConfig: Load 355 PWM" {
        # "Template Separator\n(You can make a copy of, or modify, this frame)"
        n941 = call <userlib>:"Current VIs Parent Directory__ogtk.vi"() -> ("Parent Directory (+ Relative)"=w2081:path)  [unwired: 5 in]
        n942 = Build Path(base path=w2081, name or relative path="SubVI\\LabJack\\PWM_setting_355.config") -> (appended path=w2079:path)
        n943 = call "ReadPWMConfig(SubVI).vi"("error in (no error)"=w2076, "appended path"=w2079) -> ("error out"=w2077:errorcluster, "PWM Setting"=w2075:T46)  [unwired: 8 in]
        n944 = Unbundle By Name(w2075) -> ("DIO_EF_CLOCK1_DIVISOR"=w2072:i16, "DIO_EF_CLOCK1_ROLL_VALUE"=w2071:i32)
        n945 = Multiply(x=w2072, y=w2071) -> (x*y=w2073:i32)
        n946 = Bundle By Name(cluster=w2078, "355 PWM setting"=w2075) -> (w2065:T29)
        n947 = Divide(x=80000000.0, y=w2073) -> (x/y=w2070:dbl)
        "Laser Rep Rate" <- w2070
        n948 = Number To Decimal String(number=w2070) -> (decimal integer string=w2069:string)  [unwired: 1 in]
        n949 = Concatenate Strings("355nm " ("string"), w2069, "Hz" ("string")) -> (w2067:string)
        n950 = property on="355nm Laser toggle" class="Bool (strict)"("Caption.Text"=w2067) -> ()  [unwired: 2 in, 2 out]
        n951 = call <vilib>:"Add State(s) to Queue__JKI_lib_State_Machine.vi"("State(s) in (\"\")"=w2083) -> ("States Out"=w2082:string)  [unwired: 14 in]
      }
      frame "SysConfig: Load AB PWM" {
        # "Template Separator\n(You can make a copy of, or modify, this frame)"
        n952 = call <userlib>:"Current VIs Parent Directory__ogtk.vi"() -> ("Parent Directory (+ Relative)"=w2092:path)  [unwired: 5 in]
        n953 = Build Path(base path=w2092, name or relative path="SubVI\\LabJack\\PWM_setting_AB.config") -> (appended path=w2090:path)
        n954 = call "ReadPWMConfig(SubVI).vi"("error in (no error)"=w2087, "appended path"=w2090) -> ("error out"=w2088:errorcluster, "PWM Setting"=w2086:T46)  [unwired: 8 in]
        n955 = Bundle By Name(cluster=w2084, "AB PWM setting"=w2086) -> (w2089:T29)
        n956 = call <vilib>:"Add State(s) to Queue__JKI_lib_State_Machine.vi"("State(s) in (\"\")"=w2094) -> ("States Out"=w2093:string)  [unwired: 14 in]
      }
      frame "SysConfig: Load AB setting" {
        # "load aming beam setting\n(check frequency, if 0 do nothing, if not zero, config PWM)"
        n957 = call "readAimingBeamSetting.vi"("error in (no error)"=w2112) -> ("error out"=w2107:errorcluster, "Aiming Beam Setting"=w2099:T47)  [unwired: 9 in]
        n958 = Unbundle By Name(w2099) -> ("Default Current"=w2098:dbl)
        n959 = Unbundle By Name(w2099) -> ("Frequency(Hz)"=w2095:u32)
        n960 = Equal To 0?(x=w2095) -> (x = 0?=w2105:bool)
        n961 = Select(t="", s=w2105, f="SysConfig: Load AB PWM" ("State(s) in Front (\"\")")) -> (s? t:f=w2108:string)
        n962 = Number To Decimal String(number=w2095) -> (decimal integer string=w2104:string)  [unwired: 1 in]
        n963 = Number To Decimal String(number=w2098, width (-)=i16 2) -> (decimal integer string=w2097:string)
        n964 = Concatenate Strings("445nm " ("string"), w2104, "Hz " ("string"), w2097, "mA" ("string")) -> (w2103:string)
        n965 = property on="Aiming beam toggle" class="Bool (strict)"("Caption.Text"=w2103) -> ()  [unwired: 2 in, 2 out]
        n966 = case shown="False" w2105 {
          tunnel: w2107 -> [w2120 w2123]
          tunnel: [w2119 w2123] -> w2106
          tunnel: w2095 -> [w2118 _]
          frame False {
            n967 = call "LJ_calculate_PWM_parameters.vi"("Duty Cycle (%)"=u32 10, "Error In"=w2120, "Show Confirmation"=FALSE, "Laser Rep Rate (Hz)"=w2118, "Laser"=enum16{"355nm", "AimingBeam"}."AimingBeam") -> ("Error Out"=w2119:errorcluster)  [unwired: 5 in, 1 out]
          }
          frame True {
          }
        }
        n968 = Bundle By Name(cluster=w2113, "AB Cluster"=w2099) -> (w2114:T29)
        n969 = call <vilib>:"Add State(s) to Queue__JKI_lib_State_Machine.vi"("State(s) in Front (\"\")"=w2108, "State(s) in (\"\")"=w2116) -> ("States Out"=w2115:string)  [unwired: 13 in]
      }
      frame "SysConfig: LoadABVideoSetting" {
        # "Load AB video setting form ini file\n()"
        n970 = call "readVideoConfig.vi"("error in (no error)"=w2127) -> ("error out"=w2128:errorcluster, "Aiming Beam Config"=w2126:T28)  [unwired: 8 in, 1 out]
        n971 = Bundle By Name(cluster=w2124, "VideoConfig"=w2126) -> (w2125:T29)
        n972 = call <vilib>:"Add State(s) to Queue__JKI_lib_State_Machine.vi"("State(s) in (\"\")"=w2131) -> ("States Out"=w2130:string)  [unwired: 14 in]
      }
      frame "SysConfig: LoadCursorLocation" {
        # "Load cursor location from ini file\n(load cursor from system setting ini file)"
        n973 = call "readCursorConfigMain.vi"("error in (no error)"=w2143) -> ("error out"=w2144:errorcluster, "Cursor Locations"=w2142:T48)  [unwired: 9 in]
        n974 = Unbundle By Name(w2142) -> ("DC1"=w2141:i32, "DC2"=w2140:i32, "BG1"=w2135:i32, "BG2"=w2134:i32)
        n975 = Build Array(w2141, w2140) -> (w2139:i32[])
        n976 = Build Array(w2135, w2134) -> (w2136:i32[])
        n977 = Array Max & Min(array=w2139) -> (max value=w2138:i32, min value=w2137:i32)  [unwired: 2 out]
        n978 = Array Max & Min(array=w2136) -> (max value=w2133:i32, min value=w2132:i32)  [unwired: 2 out]
        n979 = global write "GlobalVariables.vi" "DC Idx2"(w2138) -> ()
        n980 = global write "GlobalVariables.vi" "DC Idx1"(w2137) -> ()
        n981 = global write "GlobalVariables.vi" "BG Idx2"(w2133) -> ()
        n982 = global write "GlobalVariables.vi" "BG Idx1"(w2132) -> ()
        n983 = call <vilib>:"Add State(s) to Queue__JKI_lib_State_Machine.vi"("State(s) in (\"\")"=w2148) -> ("States Out"=w2147:string)  [unwired: 14 in]
      }
      frame "---------- SystemStatus ----------" {
        # "Template Separator\n(You can make a copy of, or modify, this frame)"
        n984 = call <vilib>:"Add State(s) to Queue__JKI_lib_State_Machine.vi"("State(s) in (\"\")"=w2153) -> ("States Out"=w2152:string)  [unwired: 14 in]
      }
      frame "SystemStatus: SlowSysStatusMacro" {
        # "store system check time"
        # "Template Separator\n(You can make a copy of, or modify, this frame)"
        n985 = Tick Count (ms)() -> (millisecond timer value=w2156:u32)
        n986 = Bundle By Name(cluster=w2154, "SlowTimer"=w2156) -> (w2155:T29)
        n987 = call <vilib>:"Add State(s) to Queue__JKI_lib_State_Machine.vi"("State(s) in Front (\"\")"="Digitizer: checkTemp\n/*TCP: CheckConnection" ("State(s) in Front (\"\")"), "State(s) in (\"\")"=w2161) -> ("States Out"=w2160:string)  [unwired: 13 in]
      }
      frame "SystemStatus: FastSysStatusMacro" {
        # "store system check time"
        # "Template Separator\n(You can make a copy of, or modify, this frame)"
        n988 = Tick Count (ms)() -> (millisecond timer value=w2164:u32)
        n989 = Bundle By Name(cluster=w2162, "FastTimer"=w2164) -> (w2163:T29)
        n990 = call <vilib>:"Add State(s) to Queue__JKI_lib_State_Machine.vi"("State(s) in Front (\"\")"="355 Laser: CheckPWMStatus\nAimingBeam: GetPWMStatus\n/*355 Laser: CheckControllerStatus" ("State(s) in Front (\"\")"), "State(s) in (\"\")"=w2169) -> ("States Out"=w2168:string)  [unwired: 13 in]
      }
      frame "---------- UI ----------" {
        # "Do not put any code in this frame.\n(It is a separator no-op. You can make a copy of this frame to create a new UI frame)"
        n991 = call <vilib>:"Add State(s) to Queue__JKI_lib_State_Machine.vi"("State(s) in (\"\")"=w2174) -> ("States Out"=w2173:string)  [unwired: 14 in]
      }
      frame "UI: Initialize" {
        w2176 = T49 {"Minimum"=0.0, "Maximum"=4.6, "Increment"=0.1} ("Data Entry Limits")
        w2175 = T14."Disabled and Grayed Out" ("Disabled")
        # "Disable all button on startup"
        # "Initialize the User Interface, here.\n(this is called automatically, by the Macro: Init)"
        n992 = property on="V 1" class="DigNum (strict)"("DisabledEnum"=w2175) -> ()  [unwired: 2 in, 2 out]
        n993 = property on="V 2" class="DigNum (strict)"("DisabledEnum"=w2175) -> ()  [unwired: 2 in, 2 out]
        n994 = property on="StopButton" class="Bool (strict)"("DisabledEnum"=w2175) -> ()  [unwired: 2 in, 2 out]
        n995 = property on="Sys Reconfig" class="Bool"("DisabledEnum"=w2175) -> ()  [unwired: 2 in, 2 out]
        n996 = property on="StartButton" class="Bool (strict)"("DisabledEnum"=w2175) -> ()  [unwired: 2 in, 2 out]
        n997 = property on="355nm Laser toggle" class="Bool (strict)"("DisabledEnum"=w2175) -> ()  [unwired: 2 in, 2 out]
        n998 = property on="Aiming beam toggle" class="Bool (strict)"("DisabledEnum"=w2175) -> ()  [unwired: 2 in, 2 out]
        n999 = property on="Background" class="Bool (strict)"("DisabledEnum"=w2175) -> ()  [unwired: 2 in, 2 out]
        n1000 = property on="Cali&iRF alignment" class="Bool (strict)"("DisabledEnum"=w2175) -> ()  [unwired: 2 in, 2 out]
        n1001 = property on="V 3" class="DigNum (strict)"("DisabledEnum"=w2175) -> ()  [unwired: 2 in, 2 out]
        n1002 = property on="Video Source" class="RadioBtnsControl (strict)"("DisabledEnum"=w2175) -> ()  [unwired: 2 in, 2 out]
        n1003 = property on="V 1" class="DigNum (strict)"("Data Range"=w2176) -> ()  [unwired: 2 in, 2 out]
        n1004 = property on="V 2" class="DigNum (strict)"("Data Range"=w2176) -> ()  [unwired: 2 in, 2 out]
        n1005 = property on="V 3" class="DigNum (strict)"("Data Range"=w2176) -> ()  [unwired: 2 in, 2 out]
        n1006 = call <vilib>:"Add State(s) to Queue__JKI_lib_State_Machine.vi"("State(s) in Front (\"\")"="UI: CaliAndiRFNotReady" ("State(s) in Front (\"\")"), "State(s) in (\"\")"=w2182) -> ("States Out"=w2181:string)  [unwired: 13 in]
      }
      frame "UI: BGLoaded" {
        # "[Covers: REQ24]"
        # "Do not put any code in this frame.\n(It is a separator no-op. You can make a copy of this frame to create a new UI frame)"
        n1007 = property on="Background" class="Bool (strict)"("BoolText.Text"="Loaded!" ("Boolean Text.Text"), "Colors [4]"=cluster{u32, u32}[] [{15764023, 15764023}, {16711680, 16711680}]) -> ()  [unwired: 2 in, 2 out]
        n1008 = call <vilib>:"Add State(s) to Queue__JKI_lib_State_Machine.vi"("State(s) in (\"\")"=w2189) -> ("States Out"=w2188:string)  [unwired: 14 in]
      }
      frame "UI: BGSizeError" {
        # "[Covers: REQ24]"
        # "Do not put any code in this frame.\n(It is a separator no-op. You can make a copy of this frame to create a new UI frame)"
        n1009 = property on="Background" class="Bool (strict)"("BoolText.Text"="Loaded!" ("Boolean Text.Text"), "Colors [4]"=cluster{u32, u32}[] [{7171459, 7171459}, {16711680, 16711680}]) -> ()  [unwired: 2 in, 2 out]
        n1010 = One Button Dialog(message="Background waveform length and current digitizer setting mismatch! Please take a new background before any aquisition!") -> ()  [unwired: 1 in, 1 out]
        n1011 = call <vilib>:"Add State(s) to Queue__JKI_lib_State_Machine.vi"("State(s) in (\"\")"=w2197) -> ("States Out"=w2196:string)  [unwired: 14 in]
      }
      frame "UI: CaliAndiRFLoaded" {
        # "[Covers: REQ24]"
        # "Do not put any code in this frame.\n(It is a separator no-op. You can make a copy of this frame to create a new UI frame)"
        n1012 = property on="Cali&iRF alignment" class="Bool (strict)"("BoolText.Text"="Loaded!" ("Boolean Text.Text"), "Colors [4]"=cluster{u32, u32}[] [{15764023, 15764023}, {16711680, 16711680}]) -> ()  [unwired: 2 in, 2 out]
        n1013 = call <vilib>:"Add State(s) to Queue__JKI_lib_State_Machine.vi"("State(s) in (\"\")"=w2204) -> ("States Out"=w2203:string)  [unwired: 14 in]
      }
      frame "UI: WFAutoScale" {
        # "Set graph auto scale.\n(UI: WFAutoScale >> T/F)"
        n1014 = Equal?(x=w2205, y="F") -> (x = y?=w2206:bool)
        n1015 = Equal?(x=w2205, y="T") -> (x = y?=w2208:bool)
        n1016 = case shown="True" w2208 {
          frame False {
          }
          frame True {
            w2224 = u8 2 ("Y Scale.Scale Fit")
            n1017 = property on="Channel 1" class="WFGraph (strict)"("YScale.ScaleFit"=w2224) -> ()  [unwired: 2 in, 2 out]
            n1018 = property on="Channel 2" class="WFGraph (strict)"("YScale.ScaleFit"=w2224) -> ()  [unwired: 2 in, 2 out]
            n1019 = property on="Channel 3" class="WFGraph (strict)"("YScale.ScaleFit"=w2224) -> ()  [unwired: 2 in, 2 out]
          }
        }
        n1020 = case shown="True" w2206 {
          frame False {
          }
          frame True {
            w2221 = 0.0 ("Y Scale.Range:Maximum")
            w2222 = 2.0 ("Y Scale.Range:Maximum")
            w2223 = u8 0 ("Y Scale.Scale Fit")
            n1021 = property on="Channel 1" class="WFGraph (strict)"("YScale.ScaleFit"=w2223) -> (error out=w2220:errorcluster)  [unwired: 2 in, 1 out]
            n1022 = property on="Channel 2" class="WFGraph (strict)"("YScale.ScaleFit"=w2223) -> (error out=w2219:errorcluster)  [unwired: 2 in, 1 out]
            n1023 = property on="Channel 3" class="WFGraph (strict)"("YScale.ScaleFit"=w2223) -> (error out=w2218:errorcluster)  [unwired: 2 in, 1 out]
            n1024 = property on="Channel 1" class="WFGraph (strict)"(error in=w2220, "YScale.Maximum"=w2222) -> (error out=w2217:errorcluster)  [unwired: 1 in, 1 out]
            n1025 = property on="Channel 2" class="WFGraph (strict)"(error in=w2219, "YScale.Maximum"=w2222) -> (error out=w2216:errorcluster)  [unwired: 1 in, 1 out]
            n1026 = property on="Channel 3" class="WFGraph (strict)"(error in=w2218, "YScale.Maximum"=w2222) -> (error out=w2215:errorcluster)  [unwired: 1 in, 1 out]
            n1027 = property on="Channel 1" class="WFGraph (strict)"(error in=w2217, "YScale.Minimum"=w2221) -> ()  [unwired: 1 in, 2 out]
            n1028 = property on="Channel 2" class="WFGraph (strict)"(error in=w2216, "YScale.Minimum"=w2221) -> ()  [unwired: 1 in, 2 out]
            n1029 = property on="Channel 3" class="WFGraph (strict)"(error in=w2215, "YScale.Minimum"=w2221) -> ()  [unwired: 1 in, 2 out]
          }
        }
        n1030 = call <vilib>:"Add State(s) to Queue__JKI_lib_State_Machine.vi"("State(s) in (\"\")"=w2214) -> ("States Out"=w2213:string)  [unwired: 14 in]
      }
      frame "UI: showDisclaimer" {
        # "Show disclamer window.\n(It is a separator no-op. You can make a copy of this frame to create a new UI frame)"
        n1031 = call <vilib>:"Application Directory.vi"() -> ("Application Directory"=w2237:path)
        n1032 = Build Path(base path=w2237, name or relative path="Disclamer.png") -> (appended path=w2235:path)
        n1033 = property on="Disclamer" class="Pict"() -> ("Draw Area Size"=w2233:T50)  [unwired: 2 in, 2 out]
        n1034 = disable-structure "Diagram Disable Structure" shown="Disabled" {
          frame Disabled {
            n1035 = flat-sequence {
              frame #0 {
                n1036 = call "disclaimer.vi"() -> ()  [unwired: 12 in]
              }
              frame #1 {
                n1037 = Wait (ms)(milliseconds to wait=u32 250) -> ()  [unwired: 1 out]
              }
              frame #2 {
                n1038 = call "SoftwareNote.vi"() -> ()  [unwired: 12 in]
              }
            }
          }
          frame Enabled {
          }
        }
        n1039 = call <vilib>:"Read PNG File.vi"("path to PNG file"=w2235) -> ("image data"=w2232:T51)  [unwired: 8 in, 2 out]
        n1040 = Unbundle By Name(w2232) -> ("Rectangle.right"=w2230:i16, "Rectangle.bottom"=w2228:i16)
        n1041 = Unbundle By Name(w2233) -> ("Width"=w2231:u32, "Height"=w2229:u32)
        n1042 = call <vilib>:"Draw Flattened Pixmap.vi"("image data"=w2232) -> ("new picture"=→"Disclamer":picture)  [unwired: 8 in]
        n1043 = Divide(x=w2231, y=w2230) -> (x/y=w2227:dbl)
        n1044 = Divide(x=w2229, y=w2228) -> (x/y=w2226:dbl)
        n1045 = Max & Min(x=w2227, y=w2226) -> (min(x,y)=w2225:dbl)  [unwired: 1 out]
        n1046 = property on="Disclamer" class="Pict"("ZoomFactor"=w2225) -> ()  [unwired: 2 in, 2 out]
        n1047 = call <vilib>:"Add State(s) to Queue__JKI_lib_State_Machine.vi"("State(s) in (\"\")"=w2242) -> ("States Out"=w2241:string)  [unwired: 14 in]
      }
      frame "UI: CaliAndiRFNotReady" {
        # "Do not put any code in this frame.\n(It is a separator no-op. You can make a copy of this frame to create a new UI frame)"
        n1048 = property on="Cali&iRF alignment" class="Bool (strict)"("BoolText.Text"="No Info" ("Boolean Text.Text"), "Colors [4]"=cluster{u32, u32}[] [{13816530, 13816530}, {16711680, 16711680}]) -> ()  [unwired: 2 in, 2 out]
        n1049 = call <vilib>:"Add State(s) to Queue__JKI_lib_State_Machine.vi"("State(s) in (\"\")"=w2250) -> ("States Out"=w2249:string)  [unwired: 14 in]
      }
      frame "UI: BGnotReady" {
        # "Do not put any code in this frame.\n(It is a separator no-op. You can make a copy of this frame to create a new UI frame)"
        n1050 = property on="Background" class="Bool (strict)"("BoolText.Text"="No Info" ("Boolean Text.Text"), "Colors [4]"=cluster{u32, u32}[] [{13816530, 13816530}, {16711680, 16711680}]) -> ()  [unwired: 2 in, 2 out]
        n1051 = call <vilib>:"Add State(s) to Queue__JKI_lib_State_Machine.vi"("State(s) in (\"\")"=w2257) -> ("States Out"=w2256:string)  [unwired: 14 in]
      }
      frame "UI: Reset" {
        w2259 = cluster{u32, u32}[] [{13816530, 13816530}, {13816530, 13816530}] ("Colors [4]")
        # "Do not put any code in this frame.\n(It is a separator no-op. You can make a copy of this frame to create a new UI frame)"
        n1052 = property on="Cali&iRF alignment" class="Bool (strict)"("BoolText.Text"="No Info" ("Boolean Text.Text"), "Colors [4]"=w2259) -> ()  [unwired: 2 in, 2 out]
        n1053 = property on="Background" class="Bool (strict)"("BoolText.Text"="No Info" ("Boolean Text.Text"), "Colors [4]"=w2259) -> ()  [unwired: 2 in, 2 out]
        n1054 = call <vilib>:"Add State(s) to Queue__JKI_lib_State_Machine.vi"("State(s) in (\"\")"=w2265) -> ("States Out"=w2264:string)  [unwired: 14 in]
      }
      frame "UI: SetButtonText" {
        # "Set button text of 355nm laser and aiming beam."
        n1055 = call <vilib>:"Add State(s) to Queue__JKI_lib_State_Machine.vi"("State(s) in (\"\")"=w2270) -> ("States Out"=w2269:string)  [unwired: 14 in]
      }
      frame "UI: DuringAquisition" {
        w2273 = T14."Disabled and Grayed Out" ("Disabled")
        # "Do not put any code in this frame.\n(It is a separator no-op. You can make a copy of this frame to create a new UI frame)"
        n1056 = Unbundle By Name(w2272) -> ("bothVidSourceAvail"=w2271:bool)
        n1057 = case shown="True" w2271 {
          tunnel: w2273 -> [_ w2279]
          frame False {
          }
          frame True {
            n1058 = property on="Video Source" class="RadioBtnsControl (strict)"("DisabledEnum"=w2279) -> ()  [unwired: 2 in, 2 out]
          }
        }
        n1059 = property on="StartButton" class="Bool (strict)"("DisabledEnum"=w2273) -> ()  [unwired: 2 in, 2 out]
        n1060 = property on="Sys Reconfig" class="Bool"("DisabledEnum"=w2273) -> ()  [unwired: 2 in, 2 out]
        n1061 = property on="355nm Laser toggle" class="Bool (strict)"("DisabledEnum"=w2273) -> ()  [unwired: 2 in, 2 out]
        n1062 = property on="Aiming beam toggle" class="Bool (strict)"("DisabledEnum"=w2273) -> ()  [unwired: 2 in, 2 out]
        n1063 = property on="Background" class="Bool (strict)"("DisabledEnum"=w2273) -> ()  [unwired: 2 in, 2 out]
        n1064 = property on="Radio Buttons" class="RadioBtnsControl (strict)"("DisabledEnum"=w2273) -> ()  [unwired: 2 in, 2 out]
        n1065 = property on="Cali&iRF alignment" class="Bool (strict)"("DisabledEnum"=w2273) -> ()  [unwired: 2 in, 2 out]
        n1066 = property on="Quit" class="Bool"("DisabledEnum"=w2273) -> ()  [unwired: 2 in, 2 out]
        n1067 = property on="Skip Data Save?" class="Bool (strict)"("DisabledEnum"=w2273) -> ()  [unwired: 2 in, 2 out]
        n1068 = property on="Video Display" class="Bool (strict)"("DisabledEnum"=w2273) -> ()  [unwired: 2 in, 2 out]
        n1069 = property on="StopButton" class="Bool (strict)"("DisabledEnum"=T14."Enabled" ("Disabled")) -> ()  [unwired: 2 in, 2 out]
        n1070 = call <vilib>:"Add State(s) to Queue__JKI_lib_State_Machine.vi"("State(s) in (\"\")"=w2278) -> ("States Out"=w2277:string)  [unwired: 14 in]
      }
      frame "UI: duringIRFAlign" {
        w2280 = T14."Disabled and Grayed Out" ("Disabled")
        # "Set UI to during iRF alignment\n(It is a separator no-op. You can make a copy of this frame to create a new UI frame)"
        n1071 = property on="StartButton" class="Bool (strict)"("DisabledEnum"=w2280) -> ()  [unwired: 2 in, 2 out]
        n1072 = property on="Sys Reconfig" class="Bool"("DisabledEnum"=w2280) -> ()  [unwired: 2 in, 2 out]
        n1073 = property on="355nm Laser toggle" class="Bool (strict)"("DisabledEnum"=w2280) -> ()  [unwired: 2 in, 2 out]
        n1074 = property on="Aiming beam toggle" class="Bool (strict)"("DisabledEnum"=w2280) -> ()  [unwired: 2 in, 2 out]
        n1075 = property on="Background" class="Bool (strict)"("DisabledEnum"=w2280) -> ()  [unwired: 2 in, 2 out]
        n1076 = property on="StopButton" class="Bool (strict)"("DisabledEnum"=w2280) -> ()  [unwired: 2 in, 2 out]
        n1077 = call <vilib>:"Add State(s) to Queue__JKI_lib_State_Machine.vi"("State(s) in (\"\")"=w2285) -> ("States Out"=w2284:string)  [unwired: 14 in]
      }
      frame "UI: duringBGAcquire" {
        w2286 = T14."Disabled and Grayed Out" ("Disabled")
        # "Do not put any code in this frame.\n(It is a separator no-op. You can make a copy of this frame to create a new UI frame)"
        n1078 = property on="StartButton" class="Bool (strict)"("DisabledEnum"=w2286) -> ()  [unwired: 2 in, 2 out]
        n1079 = property on="StopButton" class="Bool (strict)"("DisabledEnum"=w2286) -> ()  [unwired: 2 in, 2 out]
        n1080 = property on="Sys Reconfig" class="Bool"("DisabledEnum"=w2286) -> ()  [unwired: 2 in, 2 out]
        n1081 = property on="355nm Laser toggle" class="Bool (strict)"("DisabledEnum"=w2286) -> ()  [unwired: 2 in, 2 out]
        n1082 = property on="Aiming beam toggle" class="Bool (strict)"("DisabledEnum"=w2286) -> ()  [unwired: 2 in, 2 out]
        n1083 = property on="Cali&iRF alignment" class="Bool (strict)"("DisabledEnum"=w2286) -> ()  [unwired: 2 in, 2 out]
        n1084 = call <vilib>:"Add State(s) to Queue__JKI_lib_State_Machine.vi"("State(s) in (\"\")"=w2291) -> ("States Out"=w2290:string)  [unwired: 14 in]
      }
      frame "UI: ReadyForAquisition" {
        w2295 = T14."Enabled" ("Disabled")
        # "Do not put any code in this frame.\n(It is a separator no-op. You can make a copy of this frame to create a new UI frame)"
        n1085 = Unbundle By Name(w2294) -> ("System Status.TCP/IP"=w2293:bool, "bothVidSourceAvail"=w2292:bool)
        n1086 = property on="StartButton" class="Bool (strict)"("DisabledEnum"=w2295) -> ()  [unwired: 2 in, 2 out]
        n1087 = property on="Sys Reconfig" class="Bool"("DisabledEnum"=w2295) -> ()  [unwired: 2 in, 2 out]
        n1088 = property on="355nm Laser toggle" class="Bool (strict)"("DisabledEnum"=w2295) -> ()  [unwired: 2 in, 2 out]
        n1089 = property on="Aiming beam toggle" class="Bool (strict)"("DisabledEnum"=w2295) -> ()  [unwired: 2 in, 2 out]
        n1090 = property on="Cali&iRF alignment" class="Bool (strict)"("DisabledEnum"=w2295) -> ()  [unwired: 2 in, 2 out]
        n1091 = property on="Background" class="Bool (strict)"("DisabledEnum"=w2295) -> ()  [unwired: 2 in, 2 out]
        n1092 = property on="Quit" class="Bool"("DisabledEnum"=w2295) -> ()  [unwired: 2 in, 2 out]
        n1093 = property on="Radio Buttons" class="RadioBtnsControl (strict)"("DisabledEnum"=w2295) -> ()  [unwired: 2 in, 2 out]
        n1094 = case shown="True" w2292 {
          tunnel: w2295 -> [_ w2301]
          frame False {
          }
          frame True {
            n1095 = property on="Video Source" class="RadioBtnsControl (strict)"("DisabledEnum"=w2301) -> ()  [unwired: 2 in, 2 out]
          }
        }
        n1096 = property on="Skip Data Save?" class="Bool (strict)"("DisabledEnum"=w2295) -> ()  [unwired: 2 in, 2 out]
        n1097 = case shown="True" w2293 {
          tunnel: w2295 -> [_ w2302]
          frame False {
          }
          frame True {
            n1098 = property on="Video Display" class="Bool (strict)"("DisabledEnum"=w2302) -> ()  [unwired: 2 in, 2 out]
          }
        }
        n1099 = property on="StopButton" class="Bool (strict)"("DisabledEnum"=T14."Disabled and Grayed Out" ("Disabled")) -> ()  [unwired: 2 in, 2 out]
        n1100 = call <vilib>:"Add State(s) to Queue__JKI_lib_State_Machine.vi"("State(s) in (\"\")"=w2300) -> ("States Out"=w2299:string)  [unwired: 14 in]
      }
      frame "UI: Update" {
        # "Do not put any code in this frame.\n(It is a separator no-op. You can make a copy of this frame to create a new UI frame)"
        n1101 = Unbundle By Name(w2313) -> ("System Status"=→"System Hardware Connection Status":T3, "IDs.RunID"=→"Run #":i8, "CaseID"=→"Case #":string, "FLImDAQ"=→"FLImDAQ":T36, "SysRunning?"=→"Aquisition Status:":bool, "LJ Pinout"=→"LJ Pinout":T8, "IDs.BG ID"=→"BG #":i8, "IDs.Cali ID"=→"Calibration #":i8, "video source"=→"Visualization PC video source":T2)
        n1102 = call <vilib>:"Add State(s) to Queue__JKI_lib_State_Machine.vi"("State(s) in (\"\")"=w2316) -> ("States Out"=w2315:string)  [unwired: 14 in]
      }
      frame "UI: updateVideoToggle" {
        # "Set video toggle based on visualization PC video source.\n(take )"
        n1103 = call <vilib>:"Add State(s) to Queue__JKI_lib_State_Machine.vi"("State(s) in (\"\")"=w2321) -> ("States Out"=w2320:string)  [unwired: 14 in]
      }
      frame "UI: Cursor Set" {
        # "Argument"
        # "Set and Unset Cursor Busy.\n(Usage: \"UI: Cursor Set >> Busy|Idle\")"
        n1104 = case shown="\"Idle\", Default" w2323 {
          tunnel: w2325 -> [w2330 w2332]
          tunnel: [w2329 w2331] -> w2324
          frame "Idle", Default {
            n1105 = call <vilib>:"Unset Busy.vi"("error in (no error)"=w2330) -> ("error out"=w2329:errorcluster)  [unwired: 10 in]
          }
          frame "Busy" {
            n1106 = call <vilib>:"Set Busy.vi"("error in (no error)"=w2332) -> ("error out"=w2331:errorcluster)  [unwired: 9 in, 1 out]
          }
        }
        n1107 = call <vilib>:"Add State(s) to Queue__JKI_lib_State_Machine.vi"("State(s) in (\"\")"=w2328) -> ("States Out"=w2327:string)  [unwired: 14 in]
      }
      frame "UI: Front Panel State" {
        # "Argument"
        # "Set Front Panel Open or Closed\n(Usage: \"UI: Front Panel State >> Open|Close\")"
        n1108 = Unbundle By Name(w2336) -> ("Core.Current VI Reference"=w2335:refnum<vi>)
        n1109 = case shown="\"Open\", \"Standard\", Default" w2334 {
          tunnel: w2338 -> [w2346 w2361 w2372 w2385 w2398]
          tunnel: [w2348 w2362 w2374 w2387 w2400] -> w2337
          tunnel: w2335 -> [w2347 w2359 w2373 w2386 w2399]
          frame "Open", "Standard", Default {
            w2341 = T20."Standard" ("State")
            n1110 = property on="Property Node" class="VI"(reference=w2347, error in=w2346) -> (reference out=w2344:refnum<vi>, error out=w2345:errorcluster, "FP.State"=w2343:T20)
            n1111 = Not Equal?(x=w2343, y=w2341) -> (x != y?=w2342:bool)
            n1112 = case shown="True" w2342 {
              tunnel: [w2352 w2354] -> w2348
              tunnel: w2345 -> [w2351 w2354]
              tunnel: w2344 -> [w2350 _]
              tunnel: w2341 -> [w2349 _]
              frame True {
                n1113 = invoke on="Invoke Node" class="VI" method="FP.Open"(reference=w2350, error in=w2351, "Activate"=TRUE, "State"=w2349) -> (error out=w2352:errorcluster)  [unwired: 1 in, 4 out]
              }
              frame False {
              }
            }
          }
          frame "Close", "Closed" {
            n1114 = property on="Property Node" class="VI"(reference=w2359, error in=w2361) -> (reference out=w2358:refnum<vi>, error out=w2360:errorcluster, "FP.State"=w2356:T20)
            n1115 = Not Equal?(x=w2356, y=T20."Closed" ("Front Panel Window:State")) -> (x != y?=w2355:bool)
            n1116 = case shown="True" w2355 {
              tunnel: [w2363 w2366] -> w2362
              tunnel: w2360 -> [w2363 w2365]
              tunnel: w2358 -> [_ w2364]
              frame False {
              }
              frame True {
                n1117 = invoke on="Invoke Node" class="VI" method="FP.Close"(reference=w2364, error in=w2365) -> (error out=w2366:errorcluster)  [unwired: 1 in, 2 out]
              }
            }
          }
          frame "Hidden", "Hide" {
            w2367 = T20."Hidden" ("State")
            n1118 = property on="Property Node" class="VI"(reference=w2373, error in=w2372) -> (reference out=w2370:refnum<vi>, error out=w2371:errorcluster, "FP.State"=w2369:T20)
            n1119 = Not Equal?(x=w2369, y=w2367) -> (x != y?=w2368:bool)
            n1120 = case shown="True" w2368 {
              tunnel: [w2378 w2379] -> w2374
              tunnel: w2371 -> [w2377 w2379]
              tunnel: w2370 -> [w2376 _]
              tunnel: w2367 -> [w2375 _]
              frame True {
                n1121 = invoke on="Invoke Node" class="VI" method="FP.Open"(reference=w2376, error in=w2377, "State"=w2375) -> (error out=w2378:errorcluster)  [unwired: 2 in, 4 out]
              }
              frame False {
              }
            }
          }
          frame "Minimize", "Minimized" {
            w2380 = T20."Minimized" ("State")
            n1122 = property on="Property Node" class="VI"(reference=w2386, error in=w2385) -> (reference out=w2383:refnum<vi>, error out=w2384:errorcluster, "FP.State"=w2382:T20)
            n1123 = Not Equal?(x=w2382, y=w2380) -> (x != y?=w2381:bool)
            n1124 = case shown="True" w2381 {
              tunnel: [w2391 w2392] -> w2387
              tunnel: w2384 -> [w2390 w2392]
              tunnel: w2383 -> [w2389 _]
              tunnel: w2380 -> [w2388 _]
              frame True {
                n1125 = invoke on="Invoke Node" class="VI" method="FP.Open"(reference=w2389, error in=w2390, "State"=w2388) -> (error out=w2391:errorcluster)  [unwired: 2 in, 4 out]
              }
              frame False {
              }
            }
          }
          frame "Maximize", "Maximized" {
            w2393 = T20."Maximized" ("State")
            n1126 = property on="Property Node" class="VI"(reference=w2399, error in=w2398) -> (reference out=w2396:refnum<vi>, error out=w2397:errorcluster, "FP.State"=w2395:T20)
            n1127 = Not Equal?(x=w2395, y=w2393) -> (x != y?=w2394:bool)
            n1128 = case shown="True" w2394 {
              tunnel: [w2404 w2405] -> w2400
              tunnel: w2397 -> [w2403 w2405]
              tunnel: w2396 -> [w2402 _]
              tunnel: w2393 -> [w2401 _]
              frame True {
                n1129 = invoke on="Invoke Node" class="VI" method="FP.Open"(reference=w2402, error in=w2403, "State"=w2401) -> (error out=w2404:errorcluster)  [unwired: 2 in, 4 out]
              }
              frame False {
              }
            }
          }
        }
        n1130 = call <vilib>:"Add State(s) to Queue__JKI_lib_State_Machine.vi"("State(s) in (\"\")"=w2340) -> ("States Out"=w2339:string)  [unwired: 14 in]
      }
      frame "---------- AimingBeam ----------" {
        # "Template Separator\n(You can make a copy of, or modify, this frame)"
        n1131 = call <vilib>:"Add State(s) to Queue__JKI_lib_State_Machine.vi"("State(s) in (\"\")"=w2410) -> ("States Out"=w2409:string)  [unwired: 14 in]
      }
      frame "AimingBeam: Initialize" {
        # "set aiming beam button color"
        # "Open COM port for Aiming Beam\n(Require USB connection)"
        n1132 = Unbundle By Name(w2412) -> ("AB Cluster.Aiming Beam COM Port"=w2420:refnum<visa-resource-name>)
        n1133 = call-poly "VISA Configure Serial Port"("VISA resource name"=w2420, "Enable Termination\nChar (T)"=TRUE ("Enable Termination\nChar (T)"), "baud rate (9600)"=u32 9600, "error in (no error)"=w2417) -> ("error out"=w2416:errorcluster)  [unwired: 10 in, 1 out]
        n1134 = Unbundle By Name(w2416) -> ("status"=w2415:bool)
        n1135 = Not(x=w2415) -> (.not. x?=w2414:bool)
        n1136 = Bundle By Name(cluster=w2412, "System Status.Aiming Beam"=w2414) -> (w2413:T29)
        n1137 = call <vilib>:"Add State(s) to Queue__JKI_lib_State_Machine.vi"("State(s) in (\"\")"=w2422) -> ("States Out"=w2421:string)  [unwired: 14 in]
      }
      frame "AimingBeam: Close" {
        # "Close Aiming Beam COM port\n(Require USB connection to Aiming Beam Laser)"
        n1138 = Unbundle By Name(w2425) -> ("AB Cluster.Aiming Beam COM Port"=w2429:refnum<visa-resource-name>)
        n1139 = VISA Close(VISA resource name=w2429, error in (no error)=w2427) -> (error out=w2428:errorcluster)
        n1140 = Bundle By Name(cluster=w2425, "System Status.Aiming Beam"=FALSE) -> (w2426:T29)
        n1141 = call <vilib>:"Add State(s) to Queue__JKI_lib_State_Machine.vi"("State(s) in (\"\")"=w2431) -> ("States Out"=w2430:string)  [unwired: 14 in]
      }
      frame "AimingBeam: Set Current" {
        # "Set Aiming Beam Current\n(You can make a copy of, or modify, this frame)"
        n1142 = Unbundle By Name(w2446) -> ("AB Cluster.Aiming Beam COM Port"=w2439:refnum<visa-resource-name>, "AB Cluster.Max Current"=w2435:dbl, "AB Cluster.Default Current"=w2437:dbl, "AB Cluster.Min Current"=w2436:dbl)
        n1143 = In Range and Coerce(upper limit=w2435, x=w2437, lower limit=w2436) -> (coerced(x)=w2432:dbl)  [unwired: 1 out]
        n1144 = Number To Fractional String(number=w2432, precision (6)=i16 2) -> (F-format string=w2440:string)  [unwired: 2 in]
        n1145 = Concatenate Strings("slc:", w2440, "\r" ("Carriage Return Constant"), "\n" ("Line Feed Constant")) -> (w2443:string)
        n1146 = VISA Write(VISA resource name=w2439, write buffer=w2443, error in (no error)=w2434) -> (error out=w2438:errorcluster)  [unwired: 2 out]
        n1147 = call <vilib>:"Add State(s) to Queue__JKI_lib_State_Machine.vi"("State(s) in (\"\")"=w2448) -> ("States Out"=w2447:string)  [unwired: 14 in]
      }
      frame "AimingBeam: Set Status" {
        # "Enable Aiming Beam\n(Usage: \"AimingBeam: Set >> Enable|Disable\")"
        n1148 = Unbundle By Name(w2455) -> ("AB Cluster.Aiming Beam COM Port"=w2452:refnum<visa-resource-name>)
        n1149 = case shown="\"Enable\"" w2454 {
          tunnel: [w2458 w2462] -> w2453
          frame "Disable", Default {
            n1150 = Concatenate Strings("cof", "\r" ("Carriage Return Constant"), "\n" ("Line Feed Constant")) -> (w2458:string)
          }
          frame "Enable" {
            n1151 = Concatenate Strings("con", "\r" ("Carriage Return Constant"), "\n" ("Line Feed Constant")) -> (w2462:string)
          }
        }
        n1152 = VISA Write(VISA resource name=w2452, write buffer=w2453, error in (no error)=w2450) -> (error out=w2451:errorcluster)  [unwired: 2 out]
        n1153 = call <vilib>:"Add State(s) to Queue__JKI_lib_State_Machine.vi"("State(s) in (\"\")"=w2457) -> ("States Out"=w2456:string)  [unwired: 14 in]
      }
      frame "AimingBeam: GetPWMStatus" {
        # "Get aiming beam PWM status\n()"
        n1154 = Unbundle By Name(w2470) -> ("AB Cluster.Freq"=w2469:i32, "LJ Pinout.AimingBeam PWM"=w2476:string)
        n1155 = Equal To 0?(x=w2469) -> (x = 0?=w2468:bool)
        n1156 = call "LabJack_FGV.vi"("Operation(Read)"=enum16{"Write", "Read"}."Read" ("Operation"), "error in (no error)"=w2472) -> ("error out"=w2474:errorcluster, "Read data"=w2475:i32)  [unwired: 8 in]
        n1157 = case shown="True" w2468 {
          tunnel: w2476 -> [w2489 _]
          tunnel: [w2487 "DIO_STATE"] -> w2473
          frame False {
            n1158 = Concatenate Strings(w2489, "_EF_ENABLE" ("string")) -> (w2487:string)
          }
          frame True {
          }
        }
        n1159 = call "LJM_eReadName.vi"("Handle In"=w2475, "Name"=w2473, "error in"=w2474) -> ("Value"=w2467:dbl, "error out"=w2471:errorcluster)  [unwired: 10 in, 1 out]
        n1160 = case shown="True" w2468 {
          tunnel: w2467 -> [w2482 w2486]
          tunnel: [w2481 w2483] -> w2466
          frame False {
            n1161 = Greater Than 0?(x=w2482) -> (x > 0?=w2481:bool)
          }
          frame True {
            n1162 = Number To Boolean Array(number=w2486) -> (Boolean array=w2485:bool[])
            n1163 = Index Array(array=w2485, index=3) -> (element=w2483:bool)
          }
        }
        n1164 = case shown="False" w2466 {
          frame False {
            # "PWM is off\nset color to dark green"
            n1165 = local write "Aiming beam toggle"(FALSE ("Aimging beam")) -> ()
          }
          frame True {
            # "PWM is on\nset color to light green"
            n1166 = local write "Aiming beam toggle"(TRUE ("Aimging beam")) -> ()
          }
        }
        n1167 = call <vilib>:"Add State(s) to Queue__JKI_lib_State_Machine.vi"("State(s) in (\"\")"=w2480) -> ("States Out"=w2479:string)  [unwired: 14 in]
      }
      frame "---------- 355 Laser ----------" {
        # "Template Separator\n(You can make a copy of, or modify, this frame)"
        n1168 = call <vilib>:"Add State(s) to Queue__JKI_lib_State_Machine.vi"("State(s) in (\"\")"=w2497) -> ("States Out"=w2496:string)  [unwired: 14 in]
      }
      frame "355 Laser: Check Dewelling" {
        # "if time laser start time is less than 7.5s before, wait 250ms then check again."
        # "Template Separator\n(You can make a copy of, or modify, this frame)"
        n1169 = Unbundle By Name(w2505) -> ("Laser start tic"=w2502:u32)
        n1170 = Tick Count (ms)() -> (millisecond timer value=w2503:u32)
        n1171 = Subtract(x=w2503, y=w2502) -> (x-y=w2501:u32)
        n1172 = Greater?(x=w2501, y=u32 5000) -> (0:w2499:bool)
        n1173 = case shown="False" w2499 {
          tunnel: ["355 Laser: Check Dewelling" ""] -> w2498
          frame False {
            n1174 = Wait (ms)(milliseconds to wait=u32 250) -> ()  [unwired: 1 out]
          }
          frame True {
          }
        }
        n1175 = call <vilib>:"Add State(s) to Queue__JKI_lib_State_Machine.vi"("State(s) in Front (\"\")"=w2498, "State(s) in (\"\")"=w2508) -> ("States Out"=w2507:string)  [unwired: 13 in]
      }
      frame "355 Laser: Laser enable" {
        # "Laser enable/disable\n(Usage: \"LabJack: Laser enable/disable >> 1|0\")"
        n1176 = Unbundle By Name(w2515) -> ("LJ Pinout.Laser Start/Stop"=w2519:string, "System Status.355 Laser"=w2513:bool)
        n1177 = case shown="False" w2513 {
          tunnel: w2512 -> [w2534 w2535]
          tunnel: w2519 -> [w2528 _]
          tunnel: [w2523 w2535] -> w2517
          tunnel: [w2522 u32 0 ("millisecond timer value")] -> w2514
          frame False {
            n1178 = call "LabJack_FGV.vi"("Operation(Read)"=enum16{"Write", "Read"}."Read" ("Operation")) -> ("Read data"=w2530:i32)  [unwired: 9 in, 1 out]
            n1179 = call "LJM_eWriteName.vi"("Handle In"=w2530, "Name"=w2528, "Value"=1.0, "error in"=w2534) -> ("Handle Out"=w2529:i32, "error out"=w2527:errorcluster)  [unwired: 10 in]
            n1180 = call <userlib>:"Wait (ms)__ogtk.vi"("error in (no error)"=w2527, "milliseconds to wait"=u32 250) -> ("error out"=w2526:errorcluster)  [unwired: 8 in, 1 out]
            n1181 = call "LJM_eWriteName.vi"("Handle In"=w2529, "Name"=w2528, "Value"=0.0, "error in"=w2526) -> ("error out"=w2524:errorcluster)  [unwired: 10 in, 1 out]
            n1182 = call <userlib>:"Tick Count (ms)__ogtk.vi"("error in (no error)"=w2524) -> ("error out"=w2523:errorcluster, "millisecond timer value"=w2522:u32)  [unwired: 9 in]
          }
          frame True {
          }
        }
        n1183 = Bundle By Name(cluster=w2515, "Laser start tic"=w2514) -> (w2516:T29)
        n1184 = call <vilib>:"Add State(s) to Queue__JKI_lib_State_Machine.vi"("State(s) in (\"\")"=w2521) -> ("States Out"=w2520:string)  [unwired: 14 in]
      }
      frame "355 Laser: Laser disable" {
        # "Laser enable/disable\n(Usage: \"LabJack: Laser enable/disable >> 1|0\")"
        n1185 = Unbundle By Name(w2539) -> ("LJ Pinout.Laser Start/Stop"=w2543:string, "System Status.355 Laser"=w2537:bool)
        n1186 = case shown="True" w2537 {
          tunnel: w2544 -> [w2547 w2561]
          tunnel: w2543 -> [_ w2555]
          tunnel: [w2547 w2550] -> w2541
          tunnel: [u32 0 ("millisecond timer value") w2549] -> w2538
          frame False {
          }
          frame True {
            n1187 = call "LabJack_FGV.vi"("Operation(Read)"=enum16{"Write", "Read"}."Read" ("Operation")) -> ("Read data"=w2557:i32)  [unwired: 9 in, 1 out]
            n1188 = call "LJM_eWriteName.vi"("Handle In"=w2557, "Name"=w2555, "Value"=1.0, "error in"=w2561) -> ("Handle Out"=w2556:i32, "error out"=w2554:errorcluster)  [unwired: 10 in]
            n1189 = call <userlib>:"Wait (ms)__ogtk.vi"("error in (no error)"=w2554, "milliseconds to wait"=u32 250) -> ("error out"=w2553:errorcluster)  [unwired: 8 in, 1 out]
            n1190 = call "LJM_eWriteName.vi"("Handle In"=w2556, "Name"=w2555, "Value"=0.0, "error in"=w2553) -> ("error out"=w2551:errorcluster)  [unwired: 10 in, 1 out]
            n1191 = call <userlib>:"Tick Count (ms)__ogtk.vi"("error in (no error)"=w2551) -> ("error out"=w2550:errorcluster, "millisecond timer value"=w2549:u32)  [unwired: 9 in]
          }
        }
        n1192 = Bundle By Name(cluster=w2539, "Laser start tic"=w2538) -> (w2540:T29)
        n1193 = call <vilib>:"Add State(s) to Queue__JKI_lib_State_Machine.vi"("State(s) in (\"\")"=w2546) -> ("States Out"=w2545:string)  [unwired: 14 in]
      }
      frame "355 Laser: Dewelling" {
        # "Wait some time (ms)\n(355 Laser: Dewelling >> #)"
        n1194 = Fract/Exp String To Number(string=w2565, default (0 dbl)=0) -> (number=w2563:i32)  [unwired: 2 in, 1 out]
        n1195 = Wait (ms)(milliseconds to wait=w2563) -> ()  [unwired: 1 out]
        n1196 = call <vilib>:"Add State(s) to Queue__JKI_lib_State_Machine.vi"("State(s) in (\"\")"=w2569) -> ("States Out"=w2568:string)  [unwired: 14 in]
      }
      frame "355 Laser: Close" {
        # "Template Separator\n(You can make a copy of, or modify, this frame)"
        n1197 = call <vilib>:"Add State(s) to Queue__JKI_lib_State_Machine.vi"("State(s) in Front (\"\")"="355 Laser: CheckControllerStatus\n355 Laser: Laser disable\n355 Laser: Dewelling >>1000", "State(s) in (\"\")"=w2575) -> ("States Out"=w2574:string)  [unwired: 13 in]
      }
      frame "355 Laser: CheckControllerStatus" {
        # "if average < 2, laser no power\nif average 2 < average < 9.3, laser on\nif 9.3<average<10, interlock open, blink indicator\nif average > 10, laser off\n[Covers: REQ30]"
        # "take 10 measuremt and look at average"
        # "Check 355 laser controller status\nBy probing Emisison Lamp negative terminal voltage"
        n1198 = Unbundle By Name(w2584) -> ("LJ Pinout.Laser Ready"=w2587:string)
        n1199 = call "LabJack_FGV.vi"("Operation(Read)"=enum16{"Write", "Read"}."Read" ("Operation")) -> ("Read data"=w2588:i32)  [unwired: 9 in, 1 out]
        n1200 = for {
          N: 20 -> [_]
          tunnel: w2588 -> [w2599]
          tunnel: w2587 -> [w2598]
          shift-right: [w2597] -> w2580
          shift-left: w2586 -> [w2596]
          tunnel: [w2594] -> w2579 mode=indexing
          n1201 = call "LJM_eReadName.vi"("Handle In"=w2599, "Name"=w2598, "error in"=w2596) -> ("Value"=w2594:dbl, "error out"=w2597:errorcluster)  [unwired: 10 in, 1 out]
          n1202 = Wait (ms)(milliseconds to wait=u32 25) -> ()  [unwired: 1 out]
        }
        n1203 = call "checkLaserStatus.vi"("error in (no error)"=w2580, "Laser LED voltage"=w2579) -> ("error out"=w2581:errorcluster, "Interlock open?"=w2576:bool, "Laser on?"=w2578:bool, "Mean voltage"=→"laser EM lamp V":dbl)  [unwired: 6 in]
        n1204 = Bundle By Name(cluster=w2584, "System Status.355 Laser"=w2578) -> (w2585:T29)
        n1205 = case shown="True" w2576 {
          frame False {
            n1206 = property on="355 Laser" class="Bool (strict)"("Blinking"=FALSE) -> ()  [unwired: 2 in, 2 out]
          }
          frame True {
            n1207 = property on="355 Laser" class="Bool (strict)"("Blinking"=TRUE) -> ()  [unwired: 2 in, 2 out]
          }
        }
        n1208 = call <vilib>:"Add State(s) to Queue__JKI_lib_State_Machine.vi"("State(s) in (\"\")"=w2591) -> ("States Out"=w2590:string)  [unwired: 14 in]
      }
      frame "355 Laser: CheckPWMStatus" {
        # "Check 355 laser PWM status\n(Read LJ DIO#EF_ENABLE register to determine PWM status)"
        n1209 = Unbundle By Name(w2609) -> ("LJ Pinout.355 PWM"=w2608:string)
        n1210 = call "LabJack_FGV.vi"("Operation(Read)"=enum16{"Write", "Read"}."Read" ("Operation"), "error in (no error)"=w2602) -> ("error out"=w2605:errorcluster, "Read data"=w2606:i32)  [unwired: 8 in]
        n1211 = Concatenate Strings(w2608, "_EF_ENABLE" ("string")) -> (w2604:string)
        n1212 = call "LJM_eReadName.vi"("Handle In"=w2606, "Name"=w2604, "error in"=w2605) -> ("Value"=w2601:dbl, "error out"=w2603:errorcluster)  [unwired: 10 in, 1 out]
        n1213 = Greater Than 0?(x=w2601) -> (x > 0?=w2600:bool)
        n1214 = case shown="False" w2600 {
          frame False {
            # "PWM is off\nset color to gray"
            n1215 = local write "355nm Laser toggle"(FALSE ("355nm Laser")) -> ()
          }
          frame True {
            # "PWM is on\nset color to light green"
            n1216 = local write "355nm Laser toggle"(TRUE ("355nm Laser")) -> ()
          }
        }
        n1217 = call <vilib>:"Add State(s) to Queue__JKI_lib_State_Machine.vi"("State(s) in (\"\")"=w2613) -> ("States Out"=w2612:string)  [unwired: 14 in]
      }
      frame "355 Laser: Start" {
        # "Template Separator\n(You can make a copy of, or modify, this frame)"
        n1218 = call <vilib>:"Add State(s) to Queue__JKI_lib_State_Machine.vi"("State(s) in Front (\"\")"="LabJack: 355_PWM_Start", "State(s) in (\"\")"=w2621) -> ("States Out"=w2620:string)  [unwired: 13 in]
      }
      frame "355 Laser: Stop" {
        # "Template Separator\n(You can make a copy of, or modify, this frame)"
        n1219 = call <vilib>:"Add State(s) to Queue__JKI_lib_State_Machine.vi"("State(s) in Front (\"\")"="LabJack: 355_PWM_Stop", "State(s) in (\"\")"=w2627) -> ("States Out"=w2626:string)  [unwired: 13 in]
      }
      frame "---------- Utility ----------" {
        # "Template Separator\n(You can make a copy of, or modify, this frame)"
        n1220 = call <vilib>:"Add State(s) to Queue__JKI_lib_State_Machine.vi"("State(s) in (\"\")"=w2632) -> ("States Out"=w2631:string)  [unwired: 14 in]
      }
      frame "Utility: SetDataClass" {
        # "Set Data Class in Queues\n(Set data class to either Data, Bg or Cali)"
        n1221 = case shown="\"Cali\"" w2634 {
          tunnel: [enum16{"Data", "BG", "Cali"}."Data" ("Data Class") enum16{"Data", "BG", "Cali"}."BG" ("Data Class") enum16{"Data", "BG", "Cali"}."Cali" ("Data Class")] -> w2633
          frame "Data", Default {
          }
          frame "Bg" {
          }
          frame "Cali" {
          }
        }
        n1222 = local write "Data Class"(w2633) -> ()
        n1223 = call <vilib>:"Add State(s) to Queue__JKI_lib_State_Machine.vi"("State(s) in (\"\")"=w2639) -> ("States Out"=w2638:string)  [unwired: 14 in]
      }
      frame "Utility: AquiTimerReset" {
        # "Set Aquisition Timer\n(You can make a copy of, or modify, this frame)"
        n1224 = Tick Count (ms)() -> (millisecond timer value=w2645:u32)
        n1225 = Bundle By Name(cluster=w2643, "Aquisition Timer"=w2645) -> (w2644:T29)
        n1226 = call <vilib>:"Add State(s) to Queue__JKI_lib_State_Machine.vi"("State(s) in (\"\")"=w2649) -> ("States Out"=w2648:string)  [unwired: 14 in]
      }
      frame "Utility: AquiTimerCheck" {
        # "5min to ms"
        # "Set Aquisition Timer\n([Covers: REQ35])"
        n1227 = Unbundle By Name(w2657) -> ("Aquisition Timer"=w2655:u32)
        n1228 = Tick Count (ms)() -> (millisecond timer value=w2656:u32)
        n1229 = Subtract(x=w2656, y=w2655) -> (x-y=w2654:u32)
        n1230 = Multiply(x=1000, y=300) -> (x*y=w2651:i32)
        n1231 = Greater Or Equal?(x=w2654, y=w2651) -> (x >= y?=w2650:bool)
        n1232 = case shown="True" w2650 {
          frame False {
            # "do nothing"
          }
          frame True {
            # "if timed out, stop aquisition"
            n1233 = property on="StopButton" class="Bool (strict)"("Val(Sgnl)"=TRUE ("Value (Signaling)")) -> ()  [unwired: 2 in, 2 out]
          }
        }
        n1234 = call <vilib>:"Add State(s) to Queue__JKI_lib_State_Machine.vi"("State(s) in (\"\")"=w2661) -> ("States Out"=w2660:string)  [unwired: 14 in]
      }
      frame "Utility: StartBeep" {
        # "Beep\n([Covers: REQ18])"
        n1235 = call <vilib>:"Beep.vi"("use system alert? (T)"=FALSE, "duration (msec)"=u32 1000, "frequency (Hz)"=u32 2000) -> ()  [unwired: 9 in]
        n1236 = call <vilib>:"Add State(s) to Queue__JKI_lib_State_Machine.vi"("State(s) in (\"\")"=w2670) -> ("States Out"=w2669:string)  [unwired: 14 in]
      }
      frame "Utility: EndBeep" {
        # "Beep\n([Covers: REQ18])"
        n1237 = flat-sequence {
          frame #0 {
            n1238 = call <vilib>:"Beep.vi"("use system alert? (T)"=FALSE, "duration (msec)"=u32 500, "frequency (Hz)"=u32 2000) -> ()  [unwired: 9 in]
          }
          frame #1 {
            n1239 = call <vilib>:"Beep.vi"("use system alert? (T)"=FALSE, "duration (msec)"=u32 500, "frequency (Hz)"=u32 2000) -> ()  [unwired: 9 in]
          }
        }
        n1240 = call <vilib>:"Add State(s) to Queue__JKI_lib_State_Machine.vi"("State(s) in (\"\")"=w2675) -> ("States Out"=w2674:string)  [unwired: 14 in]
      }
      frame "Utility: RestoreDeConChan" {
        # "Template Separator\n(You can make a copy of, or modify, this frame)"
        n1241 = global read "GlobalVariables.vi" "DeconChan Temp"() -> (w2682:T12)
        n1242 = local write "Radio Buttons"(w2682) -> ()
        n1243 = call <vilib>:"Add State(s) to Queue__JKI_lib_State_Machine.vi"("State(s) in (\"\")"=w2687) -> ("States Out"=w2686:string)  [unwired: 14 in]
      }
      frame "Utility: SaveDeconChan" {
        # "Save Decon Channel to global temp\n(You can make a copy of, or modify, this frame)"
        n1244 = flat-sequence {
          frame #0 {
            n1245 = local read "Radio Buttons"() -> (w2693:T12)
            n1246 = global write "GlobalVariables.vi" "DeconChan Temp"(w2693) -> ()
          }
          frame #1 {
            n1247 = local write "Radio Buttons"(T12."No Selection" ("Radio Buttons")) -> ()
          }
        }
        n1248 = flat-sequence {
          frame #0 {
          }
          frame #1 {
            (unwired) enum32{"No Selection", "Ch1", "Ch2", "Ch3"}."No Selection" ("Radio Buttons")
          }
        }
        n1249 = call <vilib>:"Add State(s) to Queue__JKI_lib_State_Machine.vi"("State(s) in (\"\")"=w2692) -> ("States Out"=w2691:string)  [unwired: 14 in]
      }
      frame "Utility: Dewelling" {
        # "Main loop dewell\n(Dewelling >> #)"
        n1250 = Fract/Exp String To Number(string=w2698, default (0 dbl)=0) -> (number=w2696:i32)  [unwired: 2 in, 1 out]
        n1251 = Wait (ms)(milliseconds to wait=w2696) -> ()  [unwired: 1 out]
        n1252 = call <vilib>:"Add State(s) to Queue__JKI_lib_State_Machine.vi"("State(s) in (\"\")"=w2702) -> ("States Out"=w2701:string)  [unwired: 14 in]
      }
      frame "Utility: SetAllChanManualGain" {
        w2703 = FALSE ("Value (Signaling)")
        # "Set all channel to manual gain\n(You can make a copy of, or modify, this frame)"
        n1253 = property on="Auto gain ch1" class="Bool (strict)"("Val(Sgnl)"=w2703) -> ()  [unwired: 2 in, 2 out]
        n1254 = property on="Auto gain ch2" class="Bool (strict)"("Val(Sgnl)"=w2703) -> ()  [unwired: 2 in, 2 out]
        n1255 = property on="Auto gain ch3" class="Bool (strict)"("Val(Sgnl)"=w2703) -> ()  [unwired: 2 in, 2 out]
        n1256 = property on="Auto gain ch4" class="Bool (strict)"("Val(Sgnl)"=w2703) -> ()  [unwired: 2 in, 2 out]
        n1257 = call <vilib>:"Add State(s) to Queue__JKI_lib_State_Machine.vi"("State(s) in (\"\")"=w2708) -> ("States Out"=w2707:string)  [unwired: 14 in]
      }
      frame "Utility: SetAllChanAutoGain" {
        w2709 = TRUE ("Value (Signaling)")
        # "Set all channels to auto gain\n(You can make a copy of, or modify, this frame)"
        n1258 = property on="Auto gain ch1" class="Bool (strict)"("Val(Sgnl)"=w2709) -> ()  [unwired: 2 in, 2 out]
        n1259 = property on="Auto gain ch2" class="Bool (strict)"("Val(Sgnl)"=w2709) -> ()  [unwired: 2 in, 2 out]
        n1260 = property on="Auto gain ch3" class="Bool (strict)"("Val(Sgnl)"=w2709) -> ()  [unwired: 2 in, 2 out]
        n1261 = property on="Auto gain ch4" class="Bool (strict)"("Val(Sgnl)"=w2709) -> ()  [unwired: 2 in, 2 out]
        n1262 = call <vilib>:"Add State(s) to Queue__JKI_lib_State_Machine.vi"("State(s) in (\"\")"=w2714) -> ("States Out"=w2713:string)  [unwired: 14 in]
      }
      frame "---------- SysLog ----------" {
        # "Template Separator\n(You can make a copy of, or modify, this frame)"
        n1263 = call <vilib>:"Add State(s) to Queue__JKI_lib_State_Machine.vi"("State(s) in (\"\")"=w2719) -> ("States Out"=w2718:string)  [unwired: 14 in]
      }
      frame "SysLog: OpenLogFile" {
        # "Template Separator\n(You can make a copy of, or modify, this frame)"
        n1264 = call <vilib>:"Add State(s) to Queue__JKI_lib_State_Machine.vi"("State(s) in (\"\")"=w2724) -> ("States Out"=w2723:string)  [unwired: 14 in]
      }
      frame "---------- Graph ----------" {
        # "Template Separator\n(You can make a copy of, or modify, this frame)"
        n1265 = call <vilib>:"Add State(s) to Queue__JKI_lib_State_Machine.vi"("State(s) in (\"\")"=w2729) -> ("States Out"=w2728:string)  [unwired: 14 in]
      }
      frame "Graph: SetXMultiplier" {
        # "Set X multiplier of WF graphs\n(You can make a copy of, or modify, this frame)"
        n1266 = call "Digitizer1_FGV.vi"() -> ("error out"=w2733:errorcluster, "Read data"=w2734:refnum<k15>)  [unwired: 10 in]
        n1267 = property class="niScope"(reference=w2734, error in=w2733) -> ("Min Sample Rate"=w2732:dbl)  [unwired: 2 out]
        n1268 = Divide(x=1.0, y=w2732) -> (x/y=w2730:dbl)
        n1269 = property on="Channel 1" class="WFGraph (strict)"("XScale.Multiplier"=w2730) -> ()  [unwired: 2 in, 2 out]
        n1270 = property on="Channel 2" class="WFGraph (strict)"("XScale.Multiplier"=w2730) -> ()  [unwired: 2 in, 2 out]
        n1271 = property on="Channel 3" class="WFGraph (strict)"("XScale.Multiplier"=w2730) -> ()  [unwired: 2 in, 2 out]
        n1272 = property on="Channel 4" class="WFGraph (strict)"("XScale.Multiplier"=w2730) -> ()  [unwired: 2 in, 2 out]
        n1273 = call <vilib>:"Add State(s) to Queue__JKI_lib_State_Machine.vi"("State(s) in (\"\")"=w2739) -> ("States Out"=w2738:string)  [unwired: 14 in]
      }
      frame "Graph: AddCursors" {
        # "Add BG and DC cursor to all graphs\n(You can make a copy of, or modify, this frame)"
        n1274 = property on="Channel 1" class="WFGraph (strict)"() -> ("XScale.Multiplier"=w2748:dbl)  [unwired: 2 in, 2 out]
        n1275 = global read "GlobalVariables.vi" "DC Idx1"() -> (w2747:i32)
        n1276 = global read "GlobalVariables.vi" "DC Idx2"() -> (w2746:i32)
        n1277 = global read "GlobalVariables.vi" "BG Idx1"() -> (w2745:i32)
        n1278 = global read "GlobalVariables.vi" "BG Idx2"() -> (w2744:i32)
        n1279 = property on="Channel 1" class="WFGraph (strict)"(error in=w2750) -> ("CrsrList"=w2759:T30)  [unwired: 1 in, 2 out]
        n1280 = property on="Channel 2" class="WFGraph (strict)"() -> ("CrsrList"=w2756:T30)  [unwired: 2 in, 2 out]
        n1281 = property on="Channel 3" class="WFGraph (strict)"() -> ("CrsrList"=w2755:T30)  [unwired: 2 in, 2 out]
        n1282 = property on="Channel 4" class="WFGraph (strict)"() -> ("CrsrList"=w2741:T30)  [unwired: 2 in, 2 out]
        n1283 = Build Array(w2747, w2746, w2745, w2744) -> (w2743:i32[])
        n1284 = Multiply(x=w2743, y=w2748) -> (x*y=w2742:dbl[])
        n1285 = for {
          tunnel: w2759 -> [w2773] mode=indexing
          tunnel: w2742 -> [w2766] mode=indexing
          tunnel: [w2772] -> w2758 mode=indexing
          tunnel: u32[] [6618880, 6618880, 16711680, 16711680] -> [w2765] mode=indexing
          tunnel: w2756 -> [w2771] mode=indexing
          tunnel: w2755 -> [w2770] mode=indexing
          tunnel: [w2769] -> w2754 mode=indexing
          tunnel: [w2768] -> w2753 mode=indexing
          tunnel: w2741 -> [w2767] mode=indexing
          tunnel: [w2764] -> w2740 mode=indexing
          n1286 = Bundle By Name(cluster=w2773, "Position.X"=w2766, "Color"=w2765) -> (w2772:T31)
          n1287 = Bundle By Name(cluster=w2771, "Position.X"=w2766, "Color"=w2765) -> (w2769:T31)
          n1288 = Bundle By Name(cluster=w2770, "Position.X"=w2766, "Color"=w2765) -> (w2768:T31)
          n1289 = Bundle By Name(cluster=w2767, "Position.X"=w2766, "Color"=w2765) -> (w2764:T31)
        }
        n1290 = property on="Channel 1" class="WFGraph (strict)"("CrsrList"=w2758) -> (error out=w2749:errorcluster)  [unwired: 2 in, 1 out]
        n1291 = property on="Channel 2" class="WFGraph (strict)"("CrsrList"=w2754) -> ()  [unwired: 2 in, 2 out]
        n1292 = property on="Channel 3" class="WFGraph (strict)"("CrsrList"=w2753) -> ()  [unwired: 2 in, 2 out]
        n1293 = property on="Channel 4" class="WFGraph (strict)"("CrsrList"=w2740) -> ()  [unwired: 2 in, 2 out]
        n1294 = control-ref of="Channel 1"() -> (w2752:refnum<vi>)
        n1295 = call <vilib>:"Add State(s) to Queue__JKI_lib_State_Machine.vi"("State(s) in (\"\")"=w2763) -> ("States Out"=w2762:string)  [unwired: 14 in]
        n1296 = call "UpdateCurserIdx(SubVI).vi"("error in (no error)"=w2749, "WaveformGraph in"=w2752) -> ("error out"=w2751:errorcluster)  [unwired: 9 in]
      }
      frame "Graph: SaveCursorLoc" {
        # "Save cursor location to ini file\n(Save cursor location to system setting ini file)"
        n1297 = global read "GlobalVariables.vi" "DC Idx1"() -> (w2780:i32)
        n1298 = global read "GlobalVariables.vi" "DC Idx2"() -> (w2779:i32)
        n1299 = global read "GlobalVariables.vi" "BG Idx1"() -> (w2778:i32)
        n1300 = global read "GlobalVariables.vi" "BG Idx2"() -> (w2777:i32)
        n1301 = Bundle("DC Idx1"=w2780, "DC Idx2"=w2779, "BG Idx1"=w2778, "BG Idx2"=w2777) -> (w2776:T52)  [unwired: 1 in]
        n1302 = call "writeCursorConfigMain.vi"("error in (no error)"=w2774, "Cursor Locations"=w2776) -> ("error out"=w2775:errorcluster)  [unwired: 9 in]
        n1303 = call <vilib>:"Add State(s) to Queue__JKI_lib_State_Machine.vi"("State(s) in (\"\")"=w2784) -> ("States Out"=w2783:string)  [unwired: 14 in]
      }
      frame "---------- APD ----------" {
        # "Template Separator\n(You can make a copy of, or modify, this frame)"
        n1304 = call <vilib>:"Add State(s) to Queue__JKI_lib_State_Machine.vi"("State(s) in (\"\")"=w2789) -> ("States Out"=w2788:string)  [unwired: 14 in]
      }
      frame "APD: Initialize" {
        w2796 = enum16{"Read", "Write"}."Write" ("Operation (Read)")
        w2795 = refnum<class "APDClass.lvclass"> refnum  # APDClass.lvclass
        # "Initialize APD FGV\n(Initialized APD FGV for holding data)"
        n1305 = call "APD1FGV.vi"("Error In"=w2790, "Operation (Read)"=w2796, "APDClass in"=w2795) -> ("Error Out"=w2794:errorcluster)  [unwired: 7 in, 1 out]
        n1306 = call "APD2FGV.vi"("Error In"=w2790, "Operation (Read)"=w2796, "APDClass in"=w2795) -> ("Error Out"=w2793:errorcluster)  [unwired: 7 in, 1 out]
        n1307 = call "APD3FGV.vi"("Error In"=w2790, "Operation (Read)"=w2796, "APDClass in"=w2795) -> ("Error Out"=w2792:errorcluster)  [unwired: 7 in, 1 out]
        n1308 = Merge Errors(w2794, w2793, w2792) -> (w2791:errorcluster)
        n1309 = call <vilib>:"Add State(s) to Queue__JKI_lib_State_Machine.vi"("State(s) in (\"\")"=w2800) -> ("States Out"=w2799:string)  [unwired: 14 in]
      }
      frame "APD: LoadFromSerial" {
        w2802 = enum16{"Read", "Write"}."Write" ("Operation (Read)")
        # "Load APD data from tdms file\n(load and update FGV)"
        n1310 = call "readAPDSerial.vi"("Error In"=w2809) -> ("Error Out"=w2805:errorcluster, "output cluster"=w2808:T32)  [unwired: 9 in]
        n1311 = Unbundle By Name(w2808) -> ("Ch1APDSerial#"=w2821:string, "Ch2APDSerial#"=w2807:string, "Ch3APDSerial#"=w2820:string, "Ch4APDSerial#"=w2806:string)
        n1312 = call "CreatFromSerialNumNoRaw.vi"("error in (no error)"=w2805, "APD Serial #"=w2821) -> ("error out"=w2818:errorcluster, "APDClass out"=w2819:refnum<class "APDClass.lvclass">)  [unwired: 8 in]
        n1313 = call "CreatFromSerialNumNoRaw.vi"("error in (no error)"=w2805, "APD Serial #"=w2807) -> ("error out"=w2816:errorcluster, "APDClass out"=w2817:refnum<class "APDClass.lvclass">)  [unwired: 8 in]
        n1314 = call "CreatFromSerialNumNoRaw.vi"("error in (no error)"=w2805, "APD Serial #"=w2820) -> ("error out"=w2814:errorcluster, "APDClass out"=w2815:refnum<class "APDClass.lvclass">)  [unwired: 8 in]
        n1315 = call "CreatFromSerialNumNoRaw.vi"("error in (no error)"=w2805, "APD Serial #"=w2806) -> ("error out"=w2803:errorcluster, "APDClass out"=w2804:refnum<class "APDClass.lvclass">)  [unwired: 8 in]
        n1316 = call "APD1FGV.vi"("Error In"=w2818, "Operation (Read)"=w2802, "APDClass in"=w2819) -> ("Error Out"=w2813:errorcluster)  [unwired: 7 in, 1 out]
        n1317 = call "APD2FGV.vi"("Error In"=w2816, "Operation (Read)"=w2802, "APDClass in"=w2817) -> ("Error Out"=w2811:errorcluster)  [unwired: 7 in, 1 out]
        n1318 = call "APD3FGV.vi"("Error In"=w2814, "Operation (Read)"=w2802, "APDClass in"=w2815) -> ("Error Out"=w2812:errorcluster)  [unwired: 7 in, 1 out]
        n1319 = call "APD4FGV.vi"("Error In"=w2803, "Operation (Read)"=w2802, "APDClass in"=w2804) -> ("Error Out"=w2801:errorcluster)  [unwired: 7 in, 1 out]
        n1320 = Merge Errors(w2813, w2811, w2812, w2801) -> (w2810:errorcluster)
        n1321 = call <vilib>:"Add State(s) to Queue__JKI_lib_State_Machine.vi"("State(s) in (\"\")"=w2825) -> ("States Out"=w2824:string)  [unwired: 14 in]
      }
      frame "APD: UpdateCtrlVLimit" {
        w2831 = enum16{"Read", "Write"}."Read" ("Operation (Read)")
        # "Set V limit\n(You can make a copy of, or modify, this frame)"
        n1322 = call "APD1FGV.vi"("Error In"=w2832, "Operation (Read)"=w2831) -> ("Error Out"=w2847:errorcluster, "APDClass out"=w2848:refnum<class "APDClass.lvclass">)  [unwired: 8 in]
        n1323 = call "APD2FGV.vi"("Error In"=w2832, "Operation (Read)"=w2831) -> ("Error Out"=w2845:errorcluster, "APDClass out"=w2846:refnum<class "APDClass.lvclass">)  [unwired: 8 in]
        n1324 = call "APD3FGV.vi"("Error In"=w2832, "Operation (Read)"=w2831) -> ("Error Out"=w2843:errorcluster, "APDClass out"=w2844:refnum<class "APDClass.lvclass">)  [unwired: 8 in]
        n1325 = call "APD4FGV.vi"("Error In"=w2832, "Operation (Read)"=w2831) -> ("Error Out"=w2829:errorcluster, "APDClass out"=w2830:refnum<class "APDClass.lvclass">)  [unwired: 8 in]
        n1326 = call-dynamic "ReadMaxCtrlV.vi"("error in (no error)"=w2847, "APDClass in"=w2848) -> ("error out"=w2838:errorcluster, "Numeric"=w2841:dbl)  [unwired: 7 in, 1 out]
        n1327 = call-dynamic "ReadMaxCtrlV.vi"("error in (no error)"=w2845, "APDClass in"=w2846) -> ("error out"=w2836:errorcluster, "Numeric"=w2840:dbl)  [unwired: 7 in, 1 out]
        n1328 = call-dynamic "ReadMaxCtrlV.vi"("error in (no error)"=w2843, "APDClass in"=w2844) -> ("error out"=w2834:errorcluster, "Numeric"=w2839:dbl)  [unwired: 7 in, 1 out]
        n1329 = call-dynamic "ReadMaxCtrlV.vi"("error in (no error)"=w2829, "APDClass in"=w2830) -> ("error out"=w2827:errorcluster, "Numeric"=w2828:dbl)  [unwired: 7 in, 1 out]
        n1330 = property on="V 1" class="DigNum (strict)"(error in=w2838, "Maximum"=w2841) -> (error out=w2837:errorcluster)  [unwired: 1 in, 1 out]
        n1331 = property on="V 2" class="DigNum (strict)"(error in=w2836, "Maximum"=w2840) -> (error out=w2835:errorcluster)  [unwired: 1 in, 1 out]
        n1332 = property on="V 4" class="DigNum (strict)"(error in=w2827, "Maximum"=w2828) -> (error out=w2826:errorcluster)  [unwired: 1 in, 1 out]
        n1333 = property on="V 3" class="DigNum (strict)"(error in=w2834, "Maximum"=w2839) -> (error out=w2833:errorcluster)  [unwired: 1 in, 1 out]
        n1334 = Merge Errors(w2837, w2835, w2833, w2826) -> (w2842:errorcluster)
        n1335 = call <vilib>:"Add State(s) to Queue__JKI_lib_State_Machine.vi"("State(s) in (\"\")"=w2852) -> ("States Out"=w2851:string)  [unwired: 14 in]
      }
      frame "APD: GetGainLimits" {
        w2857 = enum16{"Read", "Write"}."Read" ("Operation (Read)")
        # "Template Separator\n(You can make a copy of, or modify, this frame)"
        n1336 = call "APD1FGV.vi"("Error In"=w2858, "Operation (Read)"=w2857) -> ("Error Out"=w2863:errorcluster, "APDClass out"=w2864:refnum<class "APDClass.lvclass">)  [unwired: 8 in]
        n1337 = call "APD2FGV.vi"("Error In"=w2858, "Operation (Read)"=w2857) -> ("Error Out"=w2870:errorcluster, "APDClass out"=w2871:refnum<class "APDClass.lvclass">)  [unwired: 8 in]
        n1338 = call "APD3FGV.vi"("Error In"=w2858, "Operation (Read)"=w2857) -> ("Error Out"=w2868:errorcluster, "APDClass out"=w2869:refnum<class "APDClass.lvclass">)  [unwired: 8 in]
        n1339 = call "APD4FGV.vi"("Error In"=w2858, "Operation (Read)"=w2857) -> ("Error Out"=w2855:errorcluster, "APDClass out"=w2856:refnum<class "APDClass.lvclass">)  [unwired: 8 in]
        n1340 = call-dynamic "Read Gain Limits(Log).vi"("error in (no error)"=w2863, "APDClass in"=w2864) -> ("error out"=w2862:errorcluster, "GainLimits(Log)"=w2859:cluster{"GainMax":dbl, "GainMin":dbl})  [unwired: 7 in, 1 out]
        n1341 = call-dynamic "Read Gain Limits(Log).vi"("error in (no error)"=w2870, "APDClass in"=w2871) -> ("error out"=w2866:errorcluster, "GainLimits(Log)"=w2861:cluster{"GainMax":dbl, "GainMin":dbl})  [unwired: 7 in, 1 out]
        n1342 = call-dynamic "Read Gain Limits(Log).vi"("error in (no error)"=w2868, "APDClass in"=w2869) -> ("error out"=w2865:errorcluster, "GainLimits(Log)"=w2860:cluster{"GainMax":dbl, "GainMin":dbl})  [unwired: 7 in, 1 out]
        n1343 = call-dynamic "Read Gain Limits(Log).vi"("error in (no error)"=w2855, "APDClass in"=w2856) -> ("error out"=w2853:errorcluster, "GainLimits(Log)"=w2854:cluster{"GainMax":dbl, "GainMin":dbl})  [unwired: 7 in, 1 out]
        n1344 = Merge Errors(w2862, w2866, w2865, w2853) -> (w2867:errorcluster)
        n1345 = global write "GlobalVariables.vi" "Ch1GainLim(Log)"(w2859) -> ()
        n1346 = global write "GlobalVariables.vi" "Ch2GainLim(Log)"(w2861) -> ()
        n1347 = global write "GlobalVariables.vi" "Ch3GainLim(Log)"(w2860) -> ()
        n1348 = global write "GlobalVariables.vi" "Ch4GainLim(Log)"(w2854) -> ()
        n1349 = call <vilib>:"Add State(s) to Queue__JKI_lib_State_Machine.vi"("State(s) in (\"\")"=w2875) -> ("States Out"=w2874:string)  [unwired: 14 in]
      }
      frame "---------- TCP ----------" {
        # "Template Separator\n(You can make a copy of, or modify, this frame)"
        n1350 = call <vilib>:"Add State(s) to Queue__JKI_lib_State_Machine.vi"("State(s) in (\"\")"=w2880) -> ("States Out"=w2879:string)  [unwired: 14 in]
      }
      frame "TCP: InitializeNew" {
        # "if unsuccessful and count <10, increament count \nand try again"
        # "Initialize TCP connection to aimging beam computer\n(You can make a copy of, or modify, this frame)"
        n1351 = TCP Create Listener(10:u16 2100 ("port"), 11:"RTLT" ("service name")) -> (0:w2889:errorcluster, 3:w2881:refnum<k5>)  [unwired: 3 in, 1 out]
        n1352 = while {
          tunnel: w2881 -> [w2909]
          tunnel: w2889 -> [w2908]
          tunnel: [w2899] -> w2887
          tunnel: [w2896] -> w2883
          i -> [w2905]
          stop <- w2896 stop-if-true
          n1353 = TCP Wait On Listener(8:w2908, 9:200 ("timeout ms (wait forever: -1)"), 11:w2909) -> (0:w2906:errorcluster, 4:w2903:refnum<k5>)  [unwired: 1 in, 3 out]
          n1354 = Less Or Equal?(x=50, y=w2905) -> (x <= y?=w2902:bool)
          n1355 = case shown="No Error" w2906 {
            selector: w2906 -> [w2919 w2929]
            tunnel: w2903 -> [w2920 _]
            tunnel: [errorcluster {"status"=TRUE, "code"=0, "source"=""} ("No error") w2930] -> w2898
            tunnel: [w2911 FALSE ("TCP connected?")] -> w2899
            frame No Error {
              # "connection is ready, read data"
              n1356 = TCP Read(connection ID=w2920, bytes to read=512, error in (no error)=w2919, 7:T24."CRLF" ("mode (standard)"), 9:5000 ("timeout ms (25000)")) -> (connection ID out=w2913:refnum<k5>, data out=w2915:string, error out=w2912:errorcluster)
              n1357 = Concatenate Strings("alive" ("string"), "\r\n" ("End of Line Constant")) -> (w2916:string)
              n1358 = Equal?(x=w2916, y=w2915) -> (x = y?=w2914:bool)
              n1359 = case shown="False" w2914 {
                tunnel: w2913 -> [_ w2925]
                tunnel: w2912 -> [_ _]
                tunnel: [FALSE ("TCP connected?") TRUE ("TCP connected?")] -> w2911
                frame False {
                }
                frame True {
                  n1360 = call "TcpIDFGV.vi"("action"=enum16{"write", "read"}."write", "connection ID in"=w2925) -> ()  [unwired: 8 in, 2 out]
                }
              }
            }
            frame Error {
              # "connection not ready, keep waiting"
              n1361 = Unbundle By Name(w2929) -> ("code"=w2931:i32)
              n1362 = case shown="56" w2931 {
                tunnel: w2929 -> [w2932 _]
                tunnel: [w2932 w2933] -> w2930
                frame Default {
                }
                frame 56 {
                  w2933 = errorcluster {"status"=FALSE, "code"=0, "source"=""}  # No error
                }
              }
            }
          }
          n1363 = Select(t=errorcluster {"status"=TRUE, "code"=5001, "source"=""} ("error in (no error)"), s=w2902, f=errorcluster {"status"=FALSE, "code"=0, "source"=""} ("error in (no error)")) -> (s? t:f=w2897:errorcluster)
          n1364 = Merge Errors(w2898, w2897) -> (w2896:errorcluster)
        }
        n1365 = Unbundle By Name(w2883) -> ("code"=w2886:i32)
        n1366 = Bundle By Name(cluster=w2888, "System Status.TCP/IP"=w2887, "listener ID"=w2881) -> (w2893:T29)
        n1367 = global write "GlobalVariables.vi" "TCP connected?"(w2887) -> ()
        n1368 = Equal To 0?(x=w2886) -> (x = 0?=w2885:bool)
        n1369 = Select(t=errorcluster {"status"=FALSE, "code"=0, "source"=""} ("error in (no error)"), s=w2885, f=w2883) -> (s? t:f=w2882:errorcluster)
        n1370 = call <vilib>:"Add State(s) to Queue__JKI_lib_State_Machine.vi"("State(s) in (\"\")"=w2895) -> ("States Out"=w2894:string)  [unwired: 14 in]
      }
      frame "TCP: checkSource" {
        # "Check visualization PC video source\n(send !video_source message, listen for response, then parse it to binary mask)"
        n1371 = Unbundle By Name(w2940) -> ("System Status.TCP/IP"=w2943:bool)
        n1372 = case shown="True" w2943 {
          tunnel: w2942 -> [w2948 w2971]
          tunnel: [w2948 w2955] -> w2941
          tunnel: [w2947 w2960] -> w2938
          tunnel: [w2947 w2958] -> w2937
          tunnel: [w2947 w2959] -> w2936
          tunnel: [w2947 w2957] -> w2935
          tunnel: [w2947 w2949] -> w2934
          frame False {
            w2947 = FALSE
          }
          frame True {
            n1373 = call "TcpIDFGV.vi"("Error In"=w2971, "action"=enum16{"write", "read"}."read") -> ("Error Out"=w2968:errorcluster, "connection ID out"=w2970:refnum<k5>)  [unwired: 8 in]
            n1374 = call "TCP_WriteRead.vi"("error in (no error)"=w2968, "data in"="!video_source", "connectin ID in"=w2970) -> ("error out"=w2965:errorcluster, "data out"=w2967:string)  [unwired: 4 in, 1 out]
            n1375 = Scan From String(format string="!video_source:%d", input string=w2967, error in=w2965) -> (error out=w2956:errorcluster, output 1=w2954:i32)  [unwired: 2 in, 2 out]
            n1376 = case shown="5..7, 9..11, 13..15" w2954 {
              tunnel: w2956 -> [_ _ _ _]
              tunnel: [errorcluster {"status"=TRUE, "code"=5007, "source"="Visualization PC"} ("error out") errorcluster {"status"=FALSE, "code"=0, "source"=""} ("error out") errorcluster {"status"=FALSE, "code"=0, "source"=""} ("error out") errorcluster {"status"=FALSE, "code"=0, "source"=""} ("error out")] -> w2955
              tunnel: [FALSE FALSE FALSE TRUE] -> w2949
              frame 0, Default {
                # "No video source available or default"
                n1377 = property on="Video Source" class="RadioBtnsControl (strict)"("DisabledEnum"=T14."Disabled and Grayed Out" ("Disabled")) -> ()  [unwired: 2 in, 2 out]
              }
              frame 1..3 {
                # "one or both camera available"
                n1378 = local write "Video Source"(enum32{"Camera", "FrameGrabber"}."Camera" ("Video Source")) -> ()
                n1379 = property on="Video Source" class="RadioBtnsControl (strict)"("DisabledEnum"=T14."Disabled and Grayed Out" ("Disabled")) -> ()  [unwired: 2 in, 2 out]
              }
              frame 4, 8, 12 {
                # "one or both frame grabber available"
                n1380 = local write "Video Source"(enum32{"Camera", "FrameGrabber"}."FrameGrabber" ("Video Source")) -> ()
                n1381 = property on="Video Source" class="RadioBtnsControl (strict)"("DisabledEnum"=T14."Disabled and Grayed Out" ("Disabled")) -> ()  [unwired: 2 in, 2 out]
              }
              frame 5..7, 9..11, 13..15 {
                n1382 = property on="Video Source" class="RadioBtnsControl (strict)"("DisabledEnum"=T14."Enabled" ("Disabled")) -> ()  [unwired: 2 in, 2 out]
              }
            }
            n1383 = Integer to Fixed-Point Cast(fixed-point type=fxp<+,4,4> 0.0, integer=w2954) -> (fixed-point=w2953:fxp<+,4,4>)
            n1384 = Number To Boolean Array(number=w2953) -> (Boolean array=w2951:bool[])
            n1385 = Reverse 1D Array(array=w2951) -> (reversed array=w2950:bool[])
            n1386 = Index Array(array=w2950, index=0) -> (element=w2960:bool)
            n1387 = Index Array(array=w2950, index=1) -> (element=w2958:bool)
            n1388 = Index Array(array=w2950, index=2) -> (element=w2959:bool)
            n1389 = Index Array(array=w2950, index=3) -> (element=w2957:bool)
          }
        }
        n1390 = Bundle By Name(cluster=w2940, "video source.Main Frame Grabber"=w2938, "video source.Side Frame Grabber"=w2937, "video source.Main Camera"=w2936, "video source.Side Camera"=w2935, "bothVidSourceAvail"=w2934) -> (w2939:T29)
        n1391 = call <vilib>:"Add State(s) to Queue__JKI_lib_State_Machine.vi"("State(s) in (\"\")"=w2946) -> ("States Out"=w2945:string)  [unwired: 14 in]
      }
      frame "TCP: SyncTime" {
        # "Template Separator\n(You can make a copy of, or modify, this frame)"
        n1392 = Unbundle By Name(w2988) -> ("System Status.TCP/IP"=w2987:bool)
        n1393 = case shown="True" w2987 {
          tunnel: w2989 -> [_ w2997]
          frame False {
          }
          frame True {
            n1394 = call "TcpIDFGV.vi"("Error In"=w2997, "action"=enum16{"write", "read"}."read") -> ("Error Out"=w2996:errorcluster, "connection ID out"=w2993:refnum<k5>)  [unwired: 8 in]
            n1395 = call <userlib>:"Tick Count (ms)__ogtk.vi"("error in (no error)"=w2996) -> ("error out"=w2995:errorcluster, "millisecond timer value"=w2994:u32)  [unwired: 9 in]
            n1396 = while {
              tunnel: w2995 -> [w3017]
              tunnel: w2993 -> [w3016]
              tunnel: w2994 -> [w3005]
              stop <- w3000 stop-if-true
              n1397 = Concatenate Strings("latencycheck" ("string"), "\r\n" ("End of Line Constant")) -> (w3012:string)
              n1398 = TCP Read(connection ID=w3016, bytes to read=512, error in (no error)=w3017, 7:T24."CRLF" ("mode (standard)"), 9:2000 ("timeout ms (25000)")) -> (connection ID out=w3009:refnum<k5>, data out=w3007:string, error out=w2999:errorcluster)
              n1399 = Tick Count (ms)() -> (millisecond timer value=w3006:u32)
              n1400 = Subtract(x=w3006, y=w3005) -> (x-y=w3004:u32)
              n1401 = Equal?(x=w3007, y=w3012) -> (x = y?=w3008:bool)
              n1402 = case shown="True" w3008 {
                tunnel: w3009 -> [_ w3030]
                tunnel: w3007 -> [w3022 _]
                tunnel: [w3018 FALSE] -> w3002
                tunnel: w2999 -> [_ w3024]
                frame False {
                  n1403 = Concatenate Strings("synctimer" ("string"), "\r\n" ("End of Line Constant")) -> (w3019:string)
                  n1404 = Equal?(x=w3022, y=w3019) -> (x = y?=w3018:bool)
                  "Sync Success?" <- w3018
                }
                frame True {
                  n1405 = Concatenate Strings("latencycheck:" ("string"), "\r\n" ("End of Line Constant")) -> (w3029:string)
                  n1406 = TCP Write(connection ID=w3030, data in=w3029, error in (no error)=w3024, 9:1000 ("timeout ms (25000)")) -> (error out=w3023:errorcluster)  [unwired: 2 out]
                  n1407 = call <vilib>:"Clear Errors.vi"("error in (no error)"=w3023) -> ()  [unwired: 5 in, 2 out]
                }
              }
              n1408 = Greater?(x=w3004, y=u32 10000 ("x-y")) -> (0:w3001:bool)
              n1409 = Or(x=w3002, y=w3001) -> (x .or. y?=w3000:bool)
            }
          }
        }
        n1410 = call <vilib>:"Add State(s) to Queue__JKI_lib_State_Machine.vi"("State(s) in (\"\")"=w2992) -> ("States Out"=w2991:string)  [unwired: 14 in]
      }
      frame "TCP: SendSettingMacro" {
        # "Template Separator\n(You can make a copy of, or modify, this frame)"
        n1411 = Unbundle By Name(w3034) -> ("System Status.TCP/IP"=w3033:bool)
        n1412 = case shown="True" w3033 {
          tunnel: ["" ("Empty String Constant") "TCP: sendSubjectID\nTCP: sendScaleBarSetting\nTCP: sendScaleMaxMin\nTCP: sendDeconChannel\nTCP: sendANSI\nTCP: sendRadius\nTCP: send3Dsetting\nTCP: sendFirefly\nTCP: sendPentero"] -> w3032
          frame False {
          }
          frame True {
          }
        }
        n1413 = call <vilib>:"Add State(s) to Queue__JKI_lib_State_Machine.vi"("State(s) in Front (\"\")"=w3032, "State(s) in (\"\")"=w3037) -> ("States Out"=w3036:string)  [unwired: 13 in]
      }
      frame "TCP: sendRunNum" {
        # "Send run number to AB PC\n(You can make a copy of, or modify, this frame)"
        n1414 = Unbundle By Name(w3044) -> ("System Status.TCP/IP"=w3041:bool, "IDs.RunID"=w3045:i8)
        n1415 = Increment(x=w3045) -> (x+1=w3040:i8)
        n1416 = case shown="True" w3041 {
          tunnel: w3040 -> [_ w3059]
          tunnel: [w3049 w3051] -> w3043
          tunnel: w3042 -> [w3049 w3050]
          frame False {
          }
          frame True {
            n1417 = Number To Decimal String(number=w3059, width (-)=i16 3) -> (decimal integer string=w3054:string)
            n1418 = call "TcpIDFGV.vi"("Error In"=w3050, "action"=enum16{"write", "read"}."read") -> ("Error Out"=w3052:errorcluster, "connection ID out"=w3056:refnum<k5>)  [unwired: 8 in]
            n1419 = Concatenate Strings("!run:", w3054) -> (w3053:string)
            n1420 = call "TCP_WriteRead.vi"("error in (no error)"=w3052, "data in"=w3053, "connectin ID in"=w3056) -> ("error out"=w3051:errorcluster)  [unwired: 4 in, 2 out]
          }
        }
        n1421 = call <vilib>:"Add State(s) to Queue__JKI_lib_State_Machine.vi"("State(s) in (\"\")"=w3048) -> ("States Out"=w3047:string)  [unwired: 14 in]
      }
      frame "TCP: sendVideoSource" {
        # "Send video source \n(You can make a copy of, or modify, this frame)"
        n1422 = Unbundle By Name(w3061) -> ("System Status.TCP/IP"=w3060:bool)
        n1423 = case shown="True" w3060 {
          tunnel: [w3067 w3069] -> w3063
          tunnel: w3062 -> [w3067 w3068]
          frame False {
          }
          frame True {
            n1424 = case shown="\"Camera\", Default" "Video Source" {
              tunnel: [0 1] -> w3074
              frame "Camera", Default {
              }
              frame "FrameGrabber" {
              }
            }
            n1425 = call "TcpIDFGV.vi"("Error In"=w3068, "action"=enum16{"write", "read"}."read") -> ("Error Out"=w3070:errorcluster, "connection ID out"=w3076:refnum<k5>)  [unwired: 8 in]
            n1426 = Number To Decimal String(number=w3074) -> (decimal integer string=w3072:string)  [unwired: 1 in]
            n1427 = Concatenate Strings("!invivo:" ("data in"), w3072) -> (w3071:string)
            n1428 = call "TCP_WriteRead.vi"("error in (no error)"=w3070, "data in"=w3071, "connectin ID in"=w3076) -> ("error out"=w3069:errorcluster)  [unwired: 4 in, 2 out]
          }
        }
        n1429 = call <vilib>:"Add State(s) to Queue__JKI_lib_State_Machine.vi"("State(s) in (\"\")"=w3066) -> ("States Out"=w3065:string)  [unwired: 14 in]
      }
      frame "TCP: startRun" {
        # "Template Separator\n(You can make a copy of, or modify, this frame)"
        n1430 = Unbundle By Name(w3081) -> ("System Status.TCP/IP"=w3080:bool)
        n1431 = case shown="True" w3080 {
          tunnel: [w3087 w3089] -> w3083
          tunnel: w3082 -> [w3087 w3088]
          frame False {
          }
          frame True {
            n1432 = call "TcpIDFGV.vi"("Error In"=w3088, "action"=enum16{"write", "read"}."read") -> ("Error Out"=w3090:errorcluster, "connection ID out"=w3091:refnum<k5>)  [unwired: 8 in]
            n1433 = call "TCP_WriteRead.vi"("error in (no error)"=w3090, "data in"="!acquire:1", "connectin ID in"=w3091) -> ("error out"=w3089:errorcluster)  [unwired: 4 in, 2 out]
          }
        }
        n1434 = call <vilib>:"Add State(s) to Queue__JKI_lib_State_Machine.vi"("State(s) in (\"\")"=w3086) -> ("States Out"=w3085:string)  [unwired: 14 in]
      }
      frame "TCP: stopRun" {
        # "Send stop run to AB PC\n(You can make a copy of, or modify, this frame)"
        n1435 = Unbundle By Name(w3095) -> ("System Status.TCP/IP"=w3094:bool)
        n1436 = case shown="True" w3094 {
          tunnel: [w3101 w3103] -> w3097
          tunnel: w3096 -> [w3101 w3102]
          frame False {
            # "if not connected, do nothing"
          }
          frame True {
            # "If TCP connected, send stop run"
            n1437 = call "TcpIDFGV.vi"("Error In"=w3102, "action"=enum16{"write", "read"}."read") -> ("Error Out"=w3104:errorcluster, "connection ID out"=w3106:refnum<k5>)  [unwired: 8 in]
            n1438 = call "TCP_WriteRead.vi"("error in (no error)"=w3104, "data in"="!acquire:0", "connectin ID in"=w3106) -> ("error out"=w3103:errorcluster)  [unwired: 4 in, 2 out]
          }
        }
        n1439 = call <vilib>:"Add State(s) to Queue__JKI_lib_State_Machine.vi"("State(s) in (\"\")"=w3100) -> ("States Out"=w3099:string)  [unwired: 14 in]
      }
      frame "TCP: CheckConnection" {
        # "Check TCP/IP connection statuse\n(If connection is lost, throw error)"
        n1440 = Unbundle By Name(w3109) -> ("System Status.TCP/IP"=w3108:bool)
        n1441 = case shown="True" w3108 {
          frame False {
          }
          frame True {
            # "If TCP/IP is true check, otherwise skip"
          }
        }
        n1442 = call <vilib>:"Add State(s) to Queue__JKI_lib_State_Machine.vi"("State(s) in (\"\")"=w3113) -> ("States Out"=w3112:string)  [unwired: 14 in]
      }
      frame "TCP: sendSubjectID" {
        # "Send subject ID"
        n1443 = Unbundle By Name(w3115) -> ("System Status.TCP/IP"=w3114:bool, "CaseID"=w3118:string)
        n1444 = case shown="True" w3114 {
          tunnel: w3118 -> [_ w3129]
          tunnel: [w3122 w3124] -> w3117
          tunnel: w3116 -> [w3122 w3123]
          frame False {
          }
          frame True {
            n1445 = call "TcpIDFGV.vi"("Error In"=w3123, "action"=enum16{"write", "read"}."read") -> ("Error Out"=w3125:errorcluster, "connection ID out"=w3127:refnum<k5>)  [unwired: 8 in]
            n1446 = Concatenate Strings("!subject:", w3129) -> (w3126:string)
            n1447 = call "TCP_WriteRead.vi"("error in (no error)"=w3125, "data in"=w3126, "connectin ID in"=w3127) -> ("error out"=w3124:errorcluster)  [unwired: 4 in, 2 out]
          }
        }
        n1448 = call <vilib>:"Add State(s) to Queue__JKI_lib_State_Machine.vi"("State(s) in (\"\")"=w3121) -> ("States Out"=w3120:string)  [unwired: 14 in]
      }
      frame "TCP: sendScaleBarSetting" {
        # "Template Separator\n(You can make a copy of, or modify, this frame)"
        n1449 = Unbundle By Name(w3133) -> ("System Status.TCP/IP"=w3131:bool, "VideoConfig.Scale Bar"=w3132:bool)
        n1450 = case shown="True" w3131 {
          tunnel: [w3139 w3148] -> w3135
          tunnel: w3134 -> [w3139 w3147]
          tunnel: w3132 -> [_ w3146]
          frame False {
          }
          frame True {
            n1451 = Boolean To (0,1)(Boolean=w3146) -> (0, 1=w3145:i16)
            n1452 = call "TcpIDFGV.vi"("Error In"=w3147, "action"=enum16{"write", "read"}."read") -> ("Error Out"=w3149:errorcluster, "connection ID out"=w3150:refnum<k5>)  [unwired: 8 in]
            n1453 = Number To Fractional String(number=w3145, width (-)=i16 1, precision (6)=i16 0) -> (F-format string=w3143:string)  [unwired: 1 in]
            n1454 = Concatenate Strings("!autocolor:" ("data in"), w3143) -> (w3141:string)
            n1455 = call "TCP_WriteRead.vi"("error in (no error)"=w3149, "data in"=w3141, "connectin ID in"=w3150) -> ("error out"=w3148:errorcluster)  [unwired: 4 in, 2 out]
          }
        }
        n1456 = call <vilib>:"Add State(s) to Queue__JKI_lib_State_Machine.vi"("State(s) in (\"\")"=w3138) -> ("States Out"=w3137:string)  [unwired: 14 in]
      }
      frame "TCP: sendScaleMaxMin" {
        # "Send scale bar max and min to AB PC\n(You can make a copy of, or modify, this frame)"
        n1457 = Unbundle By Name(w3155) -> ("System Status.TCP/IP"=w3152:bool, "VideoConfig.Scale Low"=w3154:dbl, "VideoConfig.Scale High"=w3153:dbl)
        n1458 = case shown="True" w3152 {
          tunnel: [w3161 w3174] -> w3157
          tunnel: w3156 -> [w3161 w3173]
          tunnel: w3154 -> [_ w3172]
          tunnel: w3153 -> [_ w3163]
          frame False {
          }
          frame True {
            n1459 = call "TcpIDFGV.vi"("Error In"=w3173, "action"=enum16{"write", "read"}."read") -> ("Error Out"=w3175:errorcluster, "connection ID out"=w3176:refnum<k5>)  [unwired: 8 in]
            n1460 = Number To Fractional String(number=w3172, width (-)=i16 4, precision (6)=i16 2) -> (F-format string=w3168:string)  [unwired: 1 in]
            n1461 = Number To Fractional String(number=w3163, width (-)=i16 4, precision (6)=i16 2) -> (F-format string=w3164:string)  [unwired: 1 in]
            n1462 = Concatenate Strings("!color:" ("string"), w3168, ";" ("string"), w3164) -> (w3162:string)
            n1463 = call "TCP_WriteRead.vi"("error in (no error)"=w3175, "data in"=w3162, "connectin ID in"=w3176) -> ("error out"=w3174:errorcluster)  [unwired: 4 in, 2 out]
          }
        }
        n1464 = call <vilib>:"Add State(s) to Queue__JKI_lib_State_Machine.vi"("State(s) in (\"\")"=w3160) -> ("States Out"=w3159:string)  [unwired: 14 in]
      }
      frame "TCP: sendDeconChannel" {
        # "Send Decon channel\n(You can make a copy of, or modify, this frame)"
        n1465 = Unbundle By Name(w3179) -> ("System Status.TCP/IP"=w3178:bool)
        n1466 = case shown="True" w3178 {
          tunnel: [w3185 w3190] -> w3181
          tunnel: w3180 -> [w3185 w3189]
          frame False {
          }
          frame True {
            n1467 = local read "Radio Buttons"() -> (w3188:T12)
            n1468 = Increment(x=w3188) -> (x+1=w3187:T12)
            n1469 = Number To Decimal String(number=w3187) -> (decimal integer string=w3186:string)  [unwired: 1 in]
            n1470 = call "TcpIDFGV.vi"("Error In"=w3189, "action"=enum16{"write", "read"}."read") -> ("Error Out"=w3191:errorcluster, "connection ID out"=w3194:refnum<k5>)  [unwired: 8 in]
            n1471 = Concatenate Strings("!channel:", w3186) -> (w3192:string)
            n1472 = call "TCP_WriteRead.vi"("error in (no error)"=w3191, "data in"=w3192, "connectin ID in"=w3194) -> ("error out"=w3190:errorcluster)  [unwired: 4 in, 2 out]
          }
        }
        n1473 = call <vilib>:"Add State(s) to Queue__JKI_lib_State_Machine.vi"("State(s) in (\"\")"=w3184) -> ("States Out"=w3183:string)  [unwired: 14 in]
      }
      frame "TCP: sendANSI" {
        # "Template Separator\n(You can make a copy of, or modify, this frame)"
        n1474 = Unbundle By Name(w3198) -> ("System Status.TCP/IP"=w3196:bool, "VideoConfig.ANSI"=w3197:dbl)
        n1475 = case shown="True" w3196 {
          tunnel: [w3204 w3210] -> w3200
          tunnel: w3199 -> [w3204 w3209]
          tunnel: w3197 -> [_ w3208]
          frame False {
          }
          frame True {
            n1476 = Number To Fractional String(number=w3208) -> (F-format string=w3206:string)  [unwired: 3 in]
            n1477 = call "TcpIDFGV.vi"("Error In"=w3209, "action"=enum16{"write", "read"}."read") -> ("Error Out"=w3211:errorcluster, "connection ID out"=w3212:refnum<k5>)  [unwired: 8 in]
            n1478 = Concatenate Strings("!ansi:" ("data in"), w3206) -> (w3205:string)
            n1479 = call "TCP_WriteRead.vi"("error in (no error)"=w3211, "data in"=w3205, "connectin ID in"=w3212) -> ("error out"=w3210:errorcluster)  [unwired: 4 in, 2 out]
          }
        }
        n1480 = call <vilib>:"Add State(s) to Queue__JKI_lib_State_Machine.vi"("State(s) in (\"\")"=w3203) -> ("States Out"=w3202:string)  [unwired: 14 in]
      }
      frame "TCP: sendRadius" {
        # "Send drawing radius to AB PC\n(You can make a copy of, or modify, this frame)"
        n1481 = Unbundle By Name(w3216) -> ("System Status.TCP/IP"=w3214:bool, "VideoConfig.Radius"=w3215:dbl)
        n1482 = case shown="True" w3214 {
          tunnel: [w3222 w3228] -> w3218
          tunnel: w3217 -> [w3222 w3227]
          tunnel: w3215 -> [_ w3226]
          frame False {
          }
          frame True {
            n1483 = Number To Fractional String(number=w3226) -> (F-format string=w3225:string)  [unwired: 3 in]
            n1484 = Concatenate Strings("!radius:" ("data in"), w3225) -> (w3223:string)
            n1485 = call "TcpIDFGV.vi"("Error In"=w3227, "action"=enum16{"write", "read"}."read") -> ("Error Out"=w3229:errorcluster, "connection ID out"=w3230:refnum<k5>)  [unwired: 8 in]
            n1486 = call "TCP_WriteRead.vi"("error in (no error)"=w3229, "data in"=w3223, "connectin ID in"=w3230) -> ("error out"=w3228:errorcluster)  [unwired: 4 in, 2 out]
          }
        }
        n1487 = call <vilib>:"Add State(s) to Queue__JKI_lib_State_Machine.vi"("State(s) in (\"\")"=w3221) -> ("States Out"=w3220:string)  [unwired: 14 in]
      }
      frame "TCP: send3Dsetting" {
        # "Send 3D setting to AB computer\n(You can make a copy of, or modify, this frame)"
        n1488 = Unbundle By Name(w3234) -> ("System Status.TCP/IP"=w3232:bool, "VideoConfig.3D?"=w3233:bool)
        n1489 = case shown="True" w3232 {
          tunnel: [w3240 w3247] -> w3236
          tunnel: w3235 -> [w3240 w3246]
          tunnel: w3233 -> [_ w3245]
          frame False {
          }
          frame True {
            n1490 = Boolean To (0,1)(Boolean=w3245) -> (0, 1=w3244:i16)
            n1491 = Number To Fractional String(number=w3244) -> (F-format string=w3243:string)  [unwired: 3 in]
            n1492 = call "TcpIDFGV.vi"("Error In"=w3246, "action"=enum16{"write", "read"}."read") -> ("Error Out"=w3248:errorcluster, "connection ID out"=w3249:refnum<k5>)  [unwired: 8 in]
            n1493 = Concatenate Strings("!3dset:" ("data in"), w3243) -> (w3241:string)
            n1494 = call "TCP_WriteRead.vi"("error in (no error)"=w3248, "data in"=w3241, "connectin ID in"=w3249) -> ("error out"=w3247:errorcluster)  [unwired: 4 in, 2 out]
          }
        }
        n1495 = call <vilib>:"Add State(s) to Queue__JKI_lib_State_Machine.vi"("State(s) in (\"\")"=w3239) -> ("States Out"=w3238:string)  [unwired: 14 in]
      }
      frame "TCP: sendFirefly" {
        # "Template Separator\n(You can make a copy of, or modify, this frame)"
        n1496 = Unbundle By Name(w3252) -> ("System Status.TCP/IP"=w3251:bool)
        n1497 = case shown="False" w3251 {
          tunnel: [w3258 w3260] -> w3254
          tunnel: w3253 -> [w3258 w3259]
          frame False {
          }
          frame True {
            n1498 = call "TcpIDFGV.vi"("Error In"=w3259, "action"=enum16{"write", "read"}."read") -> ("Error Out"=w3261:errorcluster, "connection ID out"=w3263:refnum<k5>)  [unwired: 8 in]
            n1499 = call "TCP_WriteRead.vi"("error in (no error)"=w3261, "data in"="!firefly:0", "connectin ID in"=w3263) -> ("error out"=w3260:errorcluster)  [unwired: 4 in, 2 out]
          }
        }
        n1500 = call <vilib>:"Add State(s) to Queue__JKI_lib_State_Machine.vi"("State(s) in (\"\")"=w3257) -> ("States Out"=w3256:string)  [unwired: 14 in]
      }
      frame "TCP: sendPentero" {
        # "Send Pentero setting to AB computer\n(You can make a copy of, or modify, this frame)"
        n1501 = Unbundle By Name(w3266) -> ("System Status.TCP/IP"=w3265:bool)
        n1502 = case shown="True" w3265 {
          tunnel: [w3272 w3274] -> w3268
          tunnel: w3267 -> [w3272 w3273]
          frame False {
          }
          frame True {
            n1503 = call "TcpIDFGV.vi"("Error In"=w3273, "action"=enum16{"write", "read"}."read") -> ("Error Out"=w3275:errorcluster, "connection ID out"=w3277:refnum<k5>)  [unwired: 8 in]
            n1504 = call "TCP_WriteRead.vi"("error in (no error)"=w3275, "data in"="!pentero:0", "connectin ID in"=w3277) -> ("error out"=w3274:errorcluster)  [unwired: 4 in, 2 out]
          }
        }
        n1505 = call <vilib>:"Add State(s) to Queue__JKI_lib_State_Machine.vi"("State(s) in (\"\")"=w3271) -> ("States Out"=w3270:string)  [unwired: 14 in]
      }
      frame "TCP: sendChannel" {
        # "Send DeCon Channel to AB computer\n()"
        n1506 = Unbundle By Name(w3280) -> ("System Status.TCP/IP"=w3279:bool)
        n1507 = case shown="True" w3279 {
          tunnel: [w3286 w3290] -> w3282
          tunnel: w3281 -> [w3286 w3289]
          frame False {
          }
          frame True {
            n1508 = local read "Radio Buttons"() -> (w3288:T12)
            n1509 = case shown="\"No Selection\", Default" w3288 {
              tunnel: ["" ("data in") "!channel:1" ("data in") "!channel:2" ("data in") "!channel:3" ("data in")] -> w3287
              frame "No Selection", Default {
              }
              frame "Ch1" {
              }
              frame "Ch2" {
              }
              frame "Ch3" {
              }
            }
            n1510 = call "TcpIDFGV.vi"("Error In"=w3289, "action"=enum16{"write", "read"}."read") -> ("Error Out"=w3291:errorcluster, "connection ID out"=w3292:refnum<k5>)  [unwired: 8 in]
            n1511 = call "TCP_WriteRead.vi"("error in (no error)"=w3291, "data in"=w3287, "connectin ID in"=w3292) -> ("error out"=w3290:errorcluster)  [unwired: 4 in, 2 out]
          }
        }
        n1512 = call <vilib>:"Add State(s) to Queue__JKI_lib_State_Machine.vi"("State(s) in (\"\")"=w3285) -> ("States Out"=w3284:string)  [unwired: 14 in]
      }
      frame "TCP: startCam" {
        # "Send Pentero setting to AB computer\n(You can make a copy of, or modify, this frame)"
        n1513 = Unbundle By Name(w3299) -> ("System Status.TCP/IP"=w3298:bool)
        n1514 = case shown="True" w3298 {
          tunnel: [w3305 w3307] -> w3301
          tunnel: w3300 -> [w3305 w3306]
          frame False {
          }
          frame True {
            n1515 = call "TcpIDFGV.vi"("Error In"=w3306, "action"=enum16{"write", "read"}."read") -> ("Error Out"=w3308:errorcluster, "connection ID out"=w3310:refnum<k5>)  [unwired: 8 in]
            n1516 = call "TCP_WriteRead.vi"("error in (no error)"=w3308, "data in"="!focus:1", "connectin ID in"=w3310) -> ("error out"=w3307:errorcluster)  [unwired: 4 in, 2 out]
          }
        }
        n1517 = call <vilib>:"Add State(s) to Queue__JKI_lib_State_Machine.vi"("State(s) in (\"\")"=w3304) -> ("States Out"=w3303:string)  [unwired: 14 in]
      }
      frame "TCP: stopCam" {
        # "Send Pentero setting to AB computer\n(You can make a copy of, or modify, this frame)"
        n1518 = Unbundle By Name(w3313) -> ("System Status.TCP/IP"=w3312:bool)
        n1519 = case shown="True" w3312 {
          tunnel: [w3319 w3321] -> w3315
          tunnel: w3314 -> [w3319 w3320]
          frame False {
          }
          frame True {
            n1520 = call "TcpIDFGV.vi"("Error In"=w3320, "action"=enum16{"write", "read"}."read") -> ("Error Out"=w3322:errorcluster, "connection ID out"=w3324:refnum<k5>)  [unwired: 8 in]
            n1521 = call "TCP_WriteRead.vi"("error in (no error)"=w3322, "data in"="!focus:0", "connectin ID in"=w3324) -> ("error out"=w3321:errorcluster)  [unwired: 4 in, 2 out]
          }
        }
        n1522 = call <vilib>:"Add State(s) to Queue__JKI_lib_State_Machine.vi"("State(s) in (\"\")"=w3318) -> ("States Out"=w3317:string)  [unwired: 14 in]
      }
      frame "TCP: Close" {
        # "Close TCP connection\n()"
        n1523 = Unbundle By Name(w3328) -> ("System Status.TCP/IP"=w3326:bool)
        n1524 = case shown="True" w3326 {
          tunnel: [w3334 w3336] -> w3329
          tunnel: w3327 -> [w3334 w3335]
          frame False {
          }
          frame True {
            n1525 = call "TcpIDFGV.vi"("Error In"=w3335, "action"=enum16{"write", "read"}."read") -> ("Error Out"=w3338:errorcluster, "connection ID out"=w3339:refnum<k5>)  [unwired: 8 in]
            n1526 = TCP Close Connection(connection ID=w3339, error in (no error)=w3338) -> (error out=w3336:errorcluster)  [unwired: 1 in, 1 out]
          }
        }
        n1527 = case shown="Error .." w3329 {
          tunnel: [w3342 w3343] -> w3330
          tunnel: w3328 -> [w3341 w3343]
          frame No Error {
            w3340 = FALSE ("System Status.TCP/IP")
            n1528 = Bundle By Name(cluster=w3341, "System Status.TCP/IP"=w3340) -> (w3342:T29)
            n1529 = global write "GlobalVariables.vi" "TCP connected?"(w3340) -> ()
          }
          frame Error {
          }
        }
        n1530 = call <vilib>:"Add State(s) to Queue__JKI_lib_State_Machine.vi"("State(s) in (\"\")"=w3333) -> ("States Out"=w3332:string)  [unwired: 14 in]
      }
      frame "---------- PID ----------" {
        # "Template Separator\n(You can make a copy of, or modify, this frame)"
        n1531 = call <vilib>:"Add State(s) to Queue__JKI_lib_State_Machine.vi"("State(s) in (\"\")"=w3348) -> ("States Out"=w3347:string)  [unwired: 14 in]
      }
      frame "PID: loadPID" {
        # "Template Separator\n(You can make a copy of, or modify, this frame)"
        n1532 = call "readPIDSetting.vi"("Error In"=w3352) -> ("Error Out"=w3353:errorcluster, "Ch3 PID out"=w3349:T11, "Ch2 PID out"=w3350:T11, "Ch1 PID out"=w3351:T11)  [unwired: 7 in]
        n1533 = local write "Ch1 PID gains"(w3351) -> ()
        n1534 = local write "Ch2 PID gains"(w3350) -> ()
        n1535 = local write "Ch3 PID gains"(w3349) -> ()
        n1536 = local write "Ch4 PID gains"(w3349) -> ()
        n1537 = call <vilib>:"Add State(s) to Queue__JKI_lib_State_Machine.vi"("State(s) in (\"\")"=w3357) -> ("States Out"=w3356:string)  [unwired: 14 in]
      }
      frame "---------- USBCAM ----------" {
        # "Template Separator\n(You can make a copy of, or modify, this frame)"
        n1538 = call <vilib>:"Add State(s) to Queue__JKI_lib_State_Machine.vi"("State(s) in (\"\")"=w3362) -> ("States Out"=w3361:string)  [unwired: 14 in]
      }
      frame "USBCAM: Init" {
        # "Initilize USB camera\n(You can make a copy of, or modify, this frame)"
        n1539 = call <vilib>:"IMAQdx Open Camera.vi"("Camera Control Mode"=IMAQdx_Camera_Control_Mode."Controller", "error in"=w3368, "Session In"=T26 "cam0") -> ("error out"=w3365:errorcluster, "Session Out"=w3366:T26)  [unwired: 7 in]
        n1540 = call "USBCAM_FGV.vi"("error in (no error)"=w3365, "Operation (Read)"=enum16{"Write", "Read"}."Write", "Session In"=w3366) -> ("error out"=w3364:errorcluster)  [unwired: 7 in, 1 out]
        n1541 = call <vilib>:"Add State(s) to Queue__JKI_lib_State_Machine.vi"("State(s) in (\"\")"=w3373) -> ("States Out"=w3372:string)  [unwired: 14 in]
      }
      frame "USBCAM: Config" {
        # "Config Camera\n(You can make a copy of, or modify, this frame)"
        n1542 = call "USBCAM_FGV.vi"("error in (no error)"=w3381) -> ("error out"=w3377:errorcluster, "Session Out"=w3378:T26)  [unwired: 9 in]
        n1543 = property class="IMAQdx"(reference=w3378, error in=w3377, "VideoMode"="VideoMode") -> (error out=w3376:errorcluster)  [unwired: 1 out]
        n1544 = call <vilib>:"IMAQdx Configure Acquisition.vi"("error in"=w3376, "Number of Buffers"=u32 5, "Continuous?"=IMAQdx_Acquisition_Mode."Continuous", "Session In"=w3378) -> ("error out"=w3374:errorcluster)  [unwired: 6 in, 1 out]
        n1545 = call <vilib>:"Add State(s) to Queue__JKI_lib_State_Machine.vi"("State(s) in (\"\")"=w3385) -> ("States Out"=w3384:string)  [unwired: 14 in]
      }
      frame "USBCAM: StartAndSave" {
        # "Start Camera send user event\n(You can make a copy of, or modify, this frame)"
        n1546 = Unbundle By Name(w3398) -> ("Pathes.DataPath"=w3397:path, "IDs.RunID"=w3395:i8)
        n1547 = Increment(x=w3395) -> (x+1=w3394:i8)
        n1548 = call "USBCAM_FGV.vi"("error in (no error)"=w3399) -> ("error out"=w3403:errorcluster, "Session Out"=w3402:T26)  [unwired: 9 in]
        n1549 = Format Value(format string="Run_%02d", value (0)=w3394) -> (output string=w3393:string)  [unwired: 1 in]
        n1550 = call <vilib>:"IMAQdx Start Acquisition.vi"("error in"=w3403, "Session In"=w3402) -> ("error out"=w3388:errorcluster)  [unwired: 8 in, 1 out]
        n1551 = Build Path(base path=w3397, name or relative path=w3393) -> (appended path=w3389:path)
        n1552 = Create Folder(path (use dialog)=w3389, error in=w3388) -> (created path=w3387:path, error out=w3386:errorcluster)  [unwired: 1 in, 1 out]
        n1553 = Bundle("created path"=w3387, TRUE) -> (w3391:cluster{"created path":path, bool})  [unwired: 1 in]
        n1554 = Generate User Event(priority (normal)=usereventprio."high priority", user event=w3401, event data cluster=w3391, error in=w3386) -> (error out=w3400:errorcluster)  [unwired: 1 out]
        n1555 = call <vilib>:"Add State(s) to Queue__JKI_lib_State_Machine.vi"("State(s) in (\"\")"=w3406) -> ("States Out"=w3405:string)  [unwired: 14 in]
      }
      frame "USBCAM: StartNoSave" {
        # "Start Camera send user event\n(You can make a copy of, or modify, this frame)"
        n1556 = call "USBCAM_FGV.vi"("error in (no error)"=w3413) -> ("error out"=w3417:errorcluster, "Session Out"=w3416:T26)  [unwired: 9 in]
        n1557 = call <vilib>:"IMAQdx Start Acquisition.vi"("error in"=w3417, "Session In"=w3416) -> ("error out"=w3408:errorcluster)  [unwired: 8 in, 1 out]
        n1558 = Bundle(path "", FALSE) -> (w3410:cluster{path, bool})  [unwired: 1 in]
        n1559 = Generate User Event(priority (normal)=usereventprio."high priority", user event=w3415, event data cluster=w3410, error in=w3408) -> (error out=w3414:errorcluster)  [unwired: 1 out]
        n1560 = call <vilib>:"Add State(s) to Queue__JKI_lib_State_Machine.vi"("State(s) in (\"\")"=w3420) -> ("States Out"=w3419:string)  [unwired: 14 in]
      }
      frame "USBCAM: Stop" {
        # "Stop USB Cam\n(You can make a copy of, or modify, this frame)"
        n1561 = call "USBCAM_FGV.vi"("error in (no error)"=w3421) -> ("error out"=w3424:errorcluster, "Session Out"=w3423:T26)  [unwired: 9 in]
        n1562 = call <vilib>:"IMAQdx Stop Acquisition.vi"("error in"=w3424, "Session In"=w3423) -> ("error out"=w3422:errorcluster)  [unwired: 8 in, 1 out]
        n1563 = call <vilib>:"Add State(s) to Queue__JKI_lib_State_Machine.vi"("State(s) in (\"\")"=w3428) -> ("States Out"=w3427:string)  [unwired: 14 in]
      }
      frame "USBCAM: Close" {
        # "Close Camera\n(You can make a copy of, or modify, this frame)"
        n1564 = call "USBCAM_FGV.vi"("error in (no error)"=w3434, "Operation (Read)"=enum16{"Write", "Read"}."Read") -> ("error out"=w3430:errorcluster, "Session Out"=w3432:T26)  [unwired: 8 in]
        n1565 = call <vilib>:"IMAQdx Unconfigure Acquisition.vi"("error in"=w3430, "Session In"=w3432) -> ("error out"=w3429:errorcluster, "Session Out"=w3431:T26)  [unwired: 8 in]
        n1566 = call <vilib>:"IMAQdx Close Camera.vi"("error in"=w3429, "Session In"=w3431) -> ("error out"=w3435:errorcluster)  [unwired: 9 in]
        n1567 = call <vilib>:"Add State(s) to Queue__JKI_lib_State_Machine.vi"("State(s) in (\"\")"=w3439) -> ("States Out"=w3438:string)  [unwired: 14 in]
      }
      frame "---------- Stage ----------" {
        # "Thorlabs stage control\n(You can make a copy of, or modify, this frame)"
        n1568 = call <vilib>:"Add State(s) to Queue__JKI_lib_State_Machine.vi"("State(s) in (\"\")"=w3444) -> ("States Out"=w3443:string)  [unwired: 14 in]
      }
      frame "Stage: BuildDeviceList" {
        # "Thorlabs stage control\n(You can make a copy of, or modify, this frame)"
        n1569 = constructor class="DeviceManagerCLI"(error in=w3445) -> (reference out=w3447:refnum<k24>)  [unwired: 2 in, 2 out]
        n1570 = invoke class="DeviceManagerCLI" method="BuildDeviceList"(reference=w3447) -> (error out=w3446:errorcluster)  [unwired: 2 in, 2 out]
        n1571 = call <vilib>:"Add State(s) to Queue__JKI_lib_State_Machine.vi"("State(s) in (\"\")"=w3451) -> ("States Out"=w3450:string)  [unwired: 14 in]
      }
      frame "Stage: Connect" {
        w3464 = 1 items=["UseDeviceSettings"=1, "UseFileSettings"=2, "UseConfiguredSettings"=3] ("startupSettingsMode")
        # "Connect stage and start polling\n(You can make a copy of, or modify, this frame)"
        n1572 = invoke class="KCubeDCServo" method="CreateKCubeDCServo"(reference=refnum<k24> refnum ("target class"), error in=w3459, "serialNo"="SerialNumber(Slow)") -> (error out=w3453:errorcluster, "CreateKCubeDCServo"=w3467:refnum<k24>)  [unwired: 1 in, 2 out]
        n1573 = call <userlib>:"Wait (ms)__ogtk.vi"("error in (no error)"=w3453, "milliseconds to wait"=u32 500) -> ("error out"=w3452:errorcluster)  [unwired: 8 in, 1 out]
        n1574 = invoke class="KCubeDCServo" method="Connect"(reference=w3467, error in=w3452, "device"="SerialNumber(Slow)") -> (reference out=w3472:refnum<k24>, error out=w3471:errorcluster)  [unwired: 1 in, 2 out]
        n1575 = call <userlib>:"Wait (ms)__ogtk.vi"("error in (no error)"=w3471, "milliseconds to wait"=u32 500) -> ("error out"=w3470:errorcluster)  [unwired: 8 in, 1 out]
        n1576 = invoke class="KCubeDCServo" method="LoadMotorConfiguration"(reference=w3472, error in=w3470, "serialNo"="SerialNumber(Slow)", "startupSettingsMode"=w3464) -> (reference out=w3469:refnum<k24>, error out=w3468:errorcluster)  [unwired: 1 in, 3 out]
        n1577 = invoke class="KCubeDCServo" method="StartPolling"(reference=w3469, error in=w3468, "ms"=250) -> (reference out=w3458:refnum<k24>, error out=w3456:errorcluster)  [unwired: 1 in, 2 out]
        n1578 = Bundle By Name(cluster=w3461, "StageSerial"="SerialNumber(Slow)", "DeviceHandle"=w3458) -> (w3462:T29)
        n1579 = call "Stage_FGV.vi"("Operation(Read)"=enum16{"Write", "Read"}."Write", "error in (no error)"=w3456, "reference in"=w3458) -> ("error out"=w3455:errorcluster)  [unwired: 7 in, 1 out]
        n1580 = call <vilib>:"Add State(s) to Queue__JKI_lib_State_Machine.vi"("State(s) in (\"\")"=w3475) -> ("States Out"=w3474:string)  [unwired: 14 in]
      }
      frame "Stage: WaitSettingToLoad" {
        # "Wait for setting to load\n(You can make a copy of, or modify, this frame)"
        n1581 = Unbundle By Name(w3479) -> ("DeviceHandle"=w3478:refnum<k24>)
        n1582 = while {
          tunnel: w3478 -> [w3488]
          shift-right: [w3485] -> w3477
          shift-left: w3476 -> [w3486]
          stop <- w3483 stop-if-true
          n1583 = invoke class="KCubeDCServo" method="IsSettingsInitialized"(reference=w3488, error in=w3486) -> (error out=w3485:errorcluster, "IsSettingsInitialized"=w3484:bool)  [unwired: 1 in, 1 out]
          n1584 = Wait (ms)(milliseconds to wait=u32 100) -> ()  [unwired: 1 out]
          n1585 = Or(x=w3485, y=w3484) -> (x .or. y?=w3483:bool)
        }
        n1586 = call <vilib>:"Add State(s) to Queue__JKI_lib_State_Machine.vi"("State(s) in (\"\")"=w3482) -> ("States Out"=w3481:string)  [unwired: 14 in]
      }
      frame "Stage: GetDeviceInfo" {
        w3489 = "MTS50-Z8"  # SlowAxisModel
        # "Get Thorlabs stage info\n(You can make a copy of, or modify, this frame)"
        n1587 = Unbundle By Name(w3490) -> ("DeviceHandle"=w3495:refnum<k24>)
        n1588 = invoke class="KCubeDCServo" method="GetDeviceInfo"(reference=w3495) -> (error out=w3496:errorcluster, "GetDeviceInfo"=w3497:refnum<k24>)  [unwired: 2 in, 1 out]
        n1589 = property class="DeviceInfo"(reference=w3497, error in=w3496) -> ("Name"=w3494:string, "Description"=w3493:string, "SerialNumber"=w3492:u32)  [unwired: 2 out]
        n1590 = Bundle("SlowAxisModel"=w3489, "Name"=w3494, "Description"=w3493, "SerialNumber"=w3492) -> (→"SlowAxisInfo":T5)  [unwired: 1 in]
        n1591 = call <vilib>:"Add State(s) to Queue__JKI_lib_State_Machine.vi"("State(s) in (\"\")"=w3501) -> ("States Out"=w3500:string)  [unwired: 14 in]
      }
      frame "Stage: CheckStatus" {
        # "Thorlabs stage control\n(You can make a copy of, or modify, this frame)"
        n1592 = Unbundle By Name(w3502) -> ("DeviceHandle"=w3511:refnum<k24>)
        n1593 = property class="KCubeDCServo"(reference=w3511) -> (error out=w3509:errorcluster, "Status"=w3510:refnum<k24>, "Position"=w3506:dbl)  [unwired: 1 in, 1 out]
        n1594 = property class="StatusBase"(reference=w3510, error in=w3509) -> ("IsEnabled"=w3508:bool, "IsHomed"=w3504:bool, "IsInMotion"=w3507:bool)  [unwired: 2 out]
        n1595 = Bundle("IsEnabled"=w3508, "IsHomed"=w3504, "IsInMotion"=w3507, "Position"=w3506) -> (→"SlowAxisStatus":T53)  [unwired: 1 in]
        n1596 = Bundle By Name(cluster=w3502, "StageHomed?"=w3504) -> (w3503:T29)
        n1597 = call <vilib>:"Add State(s) to Queue__JKI_lib_State_Machine.vi"("State(s) in (\"\")"=w3515) -> ("States Out"=w3514:string)  [unwired: 14 in]
      }
      frame "Stage: Home" {
        # "Thorlabs stage control\n(You can make a copy of, or modify, this frame)"
        n1598 = Unbundle By Name(w3519) -> ("StageHomed?"=w3516:bool, "DeviceHandle"=w3520:refnum<k24>)
        n1599 = case shown="False" w3516 {
          tunnel: w3520 -> [w3531 w3539]
          tunnel: [w3525 w3537] -> w3518
          tunnel: w3517 -> [w3524 w3536]
          frame False {
            # "if not homed, home stage"
            n1600 = flat-sequence {
              tunnel: [w3533] -> w3532
              tunnel: w3524 -> [w3533]
              frame #0 {
                n1601 = One Button Dialog(message="Slow Axis will home.\nPlease clear all obstacles!", button name ("OK")="Confirm!") -> ()  [unwired: 1 out]
              }
            }
            n1602 = invoke class="KCubeDCServo" method="EnableDevice"(reference=w3531, error in=w3532) -> (reference out=w3528:refnum<k24>, error out=w3530:errorcluster)  [unwired: 1 in, 1 out]
            n1603 = call <userlib>:"Wait (ms)__ogtk.vi"("error in (no error)"=w3530, "milliseconds to wait"=u32 500) -> ("error out"=w3527:errorcluster)  [unwired: 8 in, 1 out]
            n1604 = invoke class="KCubeDCServo" method="Home"(reference=w3528, error in=w3527, "waitTimeout"=60000) -> (error out=w3525:errorcluster)  [unwired: 1 in, 3 out]
          }
          frame True {
            # "if homed, go to 0"
            n1605 = invoke class="KCubeDCServo" method="SetMoveAbsolutePosition"(reference=w3539, error in=w3536, "position"=0.0) -> (reference out=w3542:refnum<k24>, error out=w3541:errorcluster)  [unwired: 1 in, 2 out]
            n1606 = invoke class="KCubeDCServo" method="MoveAbsolute"(reference=w3542, error in=w3541, "waitTimeout"=20000) -> (error out=w3537:errorcluster)  [unwired: 1 in, 3 out]
          }
        }
        n1607 = call <vilib>:"Add State(s) to Queue__JKI_lib_State_Machine.vi"("State(s) in (\"\")"=w3523) -> ("States Out"=w3522:string)  [unwired: 14 in]
      }
      frame "Stage: Scan" {
        # "Thorlabs stage control\n(You can make a copy of, or modify, this frame)"
        n1608 = Send Notification(notification="ScanRange(mm)", notifier=w3546, error in (no error)=w3544) -> (error out=w3545:errorcluster)  [unwired: 1 out]
        n1609 = call <vilib>:"Add State(s) to Queue__JKI_lib_State_Machine.vi"("State(s) in (\"\")"=w3550) -> ("States Out"=w3549:string)  [unwired: 14 in]
      }
      frame "Stage: Close" {
        # "Disconnect Thorlabs stage\n(You can make a copy of, or modify, this frame)"
        n1610 = Unbundle By Name(w3551) -> ("DeviceHandle"=w3555:refnum<k24>)
        n1611 = invoke class="KCubeDCServo" method="StopPolling"(reference=w3555) -> (reference out=w3554:refnum<k24>, error out=w3553:errorcluster)  [unwired: 2 in, 1 out]
        n1612 = invoke class="KCubeDCServo" method="Disconnect"(reference=w3554, error in=w3553) -> (error out=w3552:errorcluster)  [unwired: 1 in, 2 out]
        n1613 = call <vilib>:"Simple Error Handler.vi"("error in (no error)"=w3552) -> ()  [unwired: 4 in, 5 out]
        n1614 = call <vilib>:"Add State(s) to Queue__JKI_lib_State_Machine.vi"("State(s) in (\"\")"=w3559) -> ("States Out"=w3558:string)  [unwired: 14 in]
      }
      frame "---------- Temp (copy) ----------" {
        # "Template Separator\n(You can make a copy of, or modify, this frame)"
        n1615 = call <vilib>:"Add State(s) to Queue__JKI_lib_State_Machine.vi"("State(s) in (\"\")"=w3564) -> ("States Out"=w3563:string)  [unwired: 14 in]
      }
    }
    n1616 = Not(x=w85) -> (.not. x?=w84:bool)
    n1617 = local write "ML?"(w84) -> ()
    "ML?" <- TRUE ("main loop running?")
  }
  n1618 = disable-structure "Diagram Disable Structure" shown="Disabled" {
    frame Disabled {
      w3565 = T54 {"Horizontal"=500, "Vertical"=100}  # Top Left Corner
      n1619 = Control Help Window(0:w3565, 1:TRUE ("Show")) -> ()
      n1620 = call <vilib>:"TDMS - File Viewer.vi"() -> ()  [unwired: 6 in, 2 out]
    }
    frame Enabled {
    }
  }
  n1621 = while {
    tunnel: w68 -> [w3579]
    tunnel: w58 -> [w3578]
    tunnel: [w3577] -> w66
    tunnel: w29 -> [w3576]
    tunnel: [w3575] -> w62
    tunnel: w47 -> [w3573]
    tunnel: w8 -> [w3572]
    tunnel: w44 -> [w3567]
    stop <- w3570 stop-if-true
    # "acquire data and send it to processing loop"
    # "Data Aquisition Loop"
    n1622 = event shown="[1] <Start digitizer>: User Event" {
      selector: w3578 -> [_ _]
      dyn-events: [_ _] -> w3577
      timeout: 20 -> [_ _]
      tunnel: w3579 -> [w3585 w3595]
      tunnel: [w3580 _] -> w3570
      tunnel: w3576 -> [w3584 w3602]
      tunnel: [w3584 w3601] -> w3575
      tunnel: w3573 -> [_ w3599]
      tunnel: w3572 -> [w3583 w3594]
      tunnel: w3567 -> [_ w3592]
      event Timeout {
        # "use queue to stop data loop\nwhen queue ref is released, error will stop this loop"
        n1623 = event-data() -> ()  [unwired: 1 in, 3 out]
        n1624 = Get Queue Status(queue=w3585) -> (error out=w3582:errorcluster)  [unwired: 2 in, 7 out]
        n1625 = Get Queue Status(queue=w3583) -> (error out=w3581:errorcluster)  [unwired: 2 in, 7 out]
        n1626 = Merge Errors(w3582, w3581) -> (w3580:errorcluster)
      }
      event User Event {
        w3600 = enum16{"Write", "Read"}."Read" ("Operation")
        n1627 = event-data() -> ("Time"=→"RunStartTime":u32)  [unwired: 1 in, 3 out]
        n1628 = call "FLImDAQ_FGV.vi"() -> ("Read data"=w3597:T9)  [unwired: 10 in, 1 out]
        n1629 = call "Digitizer1_FGV.vi"("Operation (Read)"=w3600) -> ("Read data"=w3591:refnum<k15>)  [unwired: 9 in, 1 out]
        n1630 = call "Digitizer2_FGV.vi"("Operation (Read)"=w3600) -> ("Read data"=w3598:refnum<k15>)  [unwired: 9 in, 1 out]
        n1631 = Unbundle By Name(w3597) -> ("Waveform to Avg"=w3596:i16)
        n1632 = property on="Property Node" class="niScope"(reference=w3591) -> (reference out=w3590:refnum<k15>, "Vertical Range"=w3589:dbl, "Vertical Offset"=w3588:dbl)  [unwired: 1 in, 1 out]
        n1633 = Tick Count (ms)() -> (millisecond timer value=w3587:u32)
        n1634 = while {
          tunnel: w3602 -> [w3665]
          tunnel: [w3664] -> w3601
          tunnel: w3598 -> [w3658]
          tunnel: w3590 -> [w3657]
          tunnel: w3599 -> [w3656]
          shift-right: [w3625] -> _
          shift-left: u32 0 ("millisecond timer value") -> [w3650]
          tunnel: w3596 -> [w3605]
          tunnel: w3595 -> [w3647]
          tunnel: w3594 -> [w3645]
          tunnel: w3592 -> [w3638]
          tunnel: w3589 -> [w3635]
          tunnel: w3588 -> [w3636]
          shift-right: [w3630] -> _
          shift-left: w3587 -> [w3629]
          i -> [w3604]
          stop <- w3628 stop-if-true
          w3618 = enum16{"write", "read"}."read" ("action")
          w3651 = 65536
          # "enqueue V"
          # "enqueue ch3 data"
          # "enqueue ch1&2 data"
          # "acquire ch3"
          # "acquire ch1&2"
          # "send data for processing"
          n1635 = Multiply(x=w3605, y=w3604) -> (x*y=w3615:i32)
          "Fetch Record #" <- w3615
          n1636 = property on="Property Node" class="niScope"(reference=w3657, "Fetch Record Number"=w3615) -> (reference out=w3669:refnum<k15>, error out=w3668:errorcluster, "Records Done"=w3637:i32)  [unwired: 1 in]
          n1637 = Equal To 0?(x=w3604) -> (x = 0?=w3603:bool)
          n1638 = case shown="True" w3603 {
            frame False {
            }
            frame True {
              n1639 = call "High Resolution Timer Helper.vi"() -> ("Current Time"=→"FLIm 1st point time":dbl)  [unwired: 9 in, 2 out]
            }
          }
          n1640 = Subtract(x=w3637, y=w3615) -> (x-y=→"Record Backlog":i32)
          n1641 = call-poly <instrlib>:"niScope Fetch (poly).vi"("timeout"=1.0, "error in"=w3668, "channels"="0,1", "instrument handle"=w3669) -> ("error out"=w3612:errorcluster, "wfm"=w3613:i16[][], "wfm info"=w3634:T55)  [unwired: 4 in, 1 out]
          n1642 = property on="Property Node" class="niScope"(reference=w3658, "Fetch Record Number"=w3615) -> (reference out=w3662:refnum<k15>, error out=w3659:errorcluster, "Records Done"=w3616:i32)  [unwired: 1 in]
          n1643 = Divide(x=w3613, y=w3651) -> (x/y=w3624:dbl[][])
          n1644 = Tick Count (ms)() -> (millisecond timer value=w3625:u32)
          n1645 = Subtract(x=w3616, y=w3615) -> (x-y=→"Record Backlog 2":i32)
          n1646 = Subtract(x=w3625, y=w3650) -> (x-y=→"Aquisition loop timing(ms)":u32)
          n1647 = Subtract(x=w3625, y=w3629) -> (x-y=w3633:u32)
          n1648 = Multiply(x=w3624, y=w3635) -> (x*y=w3655:dbl[][])
          n1649 = call-poly <instrlib>:"niScope Fetch (poly).vi"("timeout"=0.25, "error in"=w3659, "channels"="0,1", "instrument handle"=w3662) -> ("error out"=w3611:errorcluster, "wfm"=w3652:i16[][])  [unwired: 4 in, 2 out]
          n1650 = Greater?(x=w3633, y=u32 1000) -> (0:w3631:bool)
          n1651 = Add(x=w3655, y=w3636) -> (x+y=w3646:dbl[][])
          n1652 = case shown="True" w3631 {
            tunnel: w3634 -> [_ w3679]
            tunnel: w3625 -> [_ w3678]
            tunnel: [w3672 w3678] -> w3630
            tunnel: w3629 -> [w3672 _]
            tunnel: [errorcluster {"status"=FALSE, "code"=0, "source"=""} ("error constant") w3675] -> w3626
            frame False {
            }
            frame True {
              # "[Covers: REQ29]"
              n1653 = call "CheckFrequency(SubVI).vi"("wfm info"=w3679) -> ("f (Hz)"=w3677:dbl)  [unwired: 10 in]
              "Laser f (Hz)" <- w3677
              n1654 = local read "Laser Rep Rate"() -> (w3674:dbl)
              n1655 = Increment(x=w3674) -> (x+1=w3673:dbl)
              n1656 = Greater?(x=w3677, y=w3673) -> (0:w3676:bool)
              n1657 = case shown="True" w3676 {
                tunnel: [errorcluster {"status"=FALSE, "code"=0, "source"=""} ("error constant") errorcluster {"status"=TRUE, "code"=0, "source"=""} ("error constant")] -> w3675
                frame False {
                }
                frame True {
                }
              }
            }
          }
          n1658 = Divide(x=w3652, y=w3651) -> (x/y=w3654:dbl[][])
          n1659 = Enqueue Element(queue=w3647, element=w3646, error in (no error)=w3612) -> (error out=w3610:errorcluster)  [unwired: 1 in, 2 out]
          n1660 = Multiply(x=w3654, y=w3635) -> (x*y=w3653:dbl[][])
          n1661 = Add(x=w3653, y=w3636) -> (x+y=w3644:dbl[][])
          n1662 = Enqueue Element(queue=w3645, element=w3644, error in (no error)=w3611) -> (error out=w3609:errorcluster)  [unwired: 1 in, 2 out]
          n1663 = Increment(x=w3604) -> (x+1=w3607:i32)
          n1664 = Merge Errors(w3610, w3609) -> (w3608:errorcluster)
          n1665 = call "V1FGV.vi"("Error In"=w3608, "action (write)"=w3618) -> ("Error Out"=w3642:errorcluster, "V1 out"=w3640:dbl)  [unwired: 8 in]
          n1666 = call "V2FGV.vi"("Error In"=w3642, "action(write)"=w3618) -> ("Error Out"=w3641:errorcluster, "V2 out"=w3639:dbl)  [unwired: 8 in]
          n1667 = Multiply(x=w3607, y=w3605) -> (x*y=w3606:i32)
          n1668 = call "V3FGV.vi"("Error In"=w3641, "action(write)"=w3618) -> ("Error Out"=w3621:errorcluster, "V3 out"=w3620:dbl)  [unwired: 8 in]
          n1669 = call "V4FGV.vi"("Error In"=w3621, "action(write)"=w3618, "V3 in"=w3620) -> ("Error Out"=w3619:errorcluster, "V3 out"=w3617:dbl)  [unwired: 7 in]
          n1670 = Bundle("V1 out"=w3640, "V2 out"=w3639, "V3 out"=w3620, "V3 out"=w3617) -> (w3623:T56)  [unwired: 1 in]
          n1671 = Bundle(w3606, w3646, w3644, w3623) -> (w3648:T57)  [unwired: 1 in]
          n1672 = Enqueue Element(queue=w3638, element=w3623, error in (no error)=w3619) -> (error out=w3622:errorcluster)  [unwired: 1 in, 2 out]
          n1673 = Send Notification(notification=w3648, notifier=w3665, error in (no error)=w3622) -> (notifier out=w3664:refnum<notifier>, error out=w3627:errorcluster)
          n1674 = Merge Errors(w3626, w3627) -> (w3643:errorcluster)
          n1675 = case shown="Error .." w3643 {
            selector: w3643 -> [w3682 w3683]
            tunnel: w3656 -> [_ w3686]
            tunnel: [w3682 w3683] -> w3628
            frame No Error {
            }
            frame Error {
              # "Send user event to signal aquisition has stoped"
              n1676 = Generate User Event(priority (normal)=usereventprio."high priority", user event=w3686, event data cluster=TRUE ("event data")) -> ()  [unwired: 1 in, 2 out]
            }
          }
          "aquisition loop Error Out" <- w3628
          "Auisition Loop idx" <- w3604
        }
      }
    }
    n1677 = Unbundle By Name(w3570) -> ("status"=w3569:bool)
    n1678 = Not(x=w3569) -> (.not. x?=w3568:bool)
    n1679 = local write "Aq Loop?"(w3568) -> ()
    "Aq Loop?" <- TRUE ("Aq L?")
  }
  n1680 = while {
    tunnel: w29 -> [w3734]
    shift-right: [w3697] -> _
    shift-left: _ -> [w3730]
    tunnel: [w3688] -> w13 mode=indexing
    i -> [w3714]
    stop <- w3694 stop-if-true
    # "Channel 3"
    # "Channel 2"
    # "Channel 1"
    # "use FGV for gain value"
    # "stop on error"
    # "Gain adjustment and Data processing"
    n1681 = Tick Count (ms)() -> (millisecond timer value=w3697:u32)
    n1682 = Wait on Notification(notifier=w3734, ignore previous (F)=TRUE) -> (notification=w3708:T17, error out=w3687:errorcluster)  [unwired: 2 in, 2 out]
    n1683 = Subtract(x=w3697, y=w3730) -> (x-y=→"PID loop timing(ms)":u32)
    n1684 = Unbundle(w3708) -> ("CH1&2"=w3724:dbl[][], "CH3"=w3723:dbl[][])  [unwired: 2 out]
    n1685 = call "SeperateChanData.vi"("Input (Ch1&2)"=w3724) -> ("Ch1"=w3719:dbl[][], "Ch2"=w3717:dbl[][])
    n1686 = call "SeperateChanData.vi"("Input (Ch1&2)"=w3723) -> ("Ch1"=w3713:dbl[][], "Ch2"=w3706:dbl[][])
    n1687 = call "AvgArrayTimeCritical.vi"("2D array"=w3719) -> ("1D Avg"=w3718:dbl[])  [unwired: 10 in]
    n1688 = call "AvgArrayTimeCritical.vi"("2D array"=w3717) -> ("1D Avg"=w3728:dbl[])  [unwired: 10 in]
    n1689 = call "AvgArrayTimeCritical.vi"("2D array"=w3713) -> ("1D Avg"=w3725:dbl[])  [unwired: 10 in]
    n1690 = call "AvgArrayTimeCritical.vi"("2D array"=w3706) -> ("1D Avg"=w3705:dbl[])  [unwired: 10 in]
    n1691 = Array Max & Min(array=w3718) -> (max value=w3716:dbl)  [unwired: 3 out]
    n1692 = Array Max & Min(array=w3728) -> (max value=w3715:dbl)  [unwired: 3 out]
    n1693 = Array Max & Min(array=w3725) -> (max value=w3698:dbl)  [unwired: 3 out]
    n1694 = Array Max & Min(array=w3705) -> (max value=w3703:dbl)  [unwired: 3 out]
    n1695 = local read "Auto gain ch4"() -> (w3704:bool)
    n1696 = local read "Auto gain ch1"() -> (w3722:bool)
    n1697 = local read "Auto gain ch2"() -> (w3721:bool)
    n1698 = local read "Auto gain ch3"() -> (w3720:bool)
    n1699 = case shown="True" w3704 {
      tunnel: w3703 -> [_ w3781]
      tunnel: "V target(1.0)" -> [_ w3779]
      tunnel: [FALSE w3776] -> w3701
      tunnel: [0.0 ("CtrlV") w3771] -> w3702
      frame False {
        # "Manual control"
      }
      frame True {
        # "PID control"
        n1700 = global read "GlobalVariables.vi" "Ch4GainLim(Log)"() -> (w3782:cluster{"GainMax":dbl, "GainMin":dbl})
        n1701 = call-poly <vilib>:"PID.vi"("output range"=w3782, "PID gains"="Ch4 PID gains", "process variable"=w3781, "setpoint"=w3779) -> ("output"=w3780:dbl)  [unwired: 6 in, 1 out]
        n1702 = Power Of 10(x=w3780) -> (10^x=w3772:dbl)
        "Gain4" <- w3772
        n1703 = call "V4FGV.vi"("action(write)"=enum16{"write", "read"}."read") -> ("Error Out"=w3775:errorcluster, "V3 out"=w3777:dbl)  [unwired: 9 in]
        n1704 = call "GainToCtrlV.vi"("Gain"=w3772, "Channel"=enum16{"Ch1", "Ch2", "Ch3", "Ch4"}."Ch4") -> ("CtrlV"=w3771:dbl)  [unwired: 8 in, 1 out]
        n1705 = call "V4FGV.vi"("Error In"=w3775, "V3 in"=w3771) -> ()  [unwired: 8 in, 2 out]
        n1706 = local write "V 4"(w3771) -> ()
        n1707 = Not Equal?(x=w3771, y=w3777) -> (x != y?=w3776:bool)
      }
    }
    n1708 = case shown="True" w3722 {
      tunnel: "V target(1.0)" -> [_ w3796]
      tunnel: w3716 -> [_ w3793]
      tunnel: [0.0 ("CtrlV") w3785] -> w3695
      tunnel: [FALSE w3787] -> w3712
      frame False {
        # "Manual control"
      }
      frame True {
        # "PID control"
        n1709 = global read "GlobalVariables.vi" "Ch1GainLim(Log)"() -> (w3792:cluster{"GainMax":dbl, "GainMin":dbl})
        n1710 = call-poly <vilib>:"PID.vi"("output range"=w3792, "PID gains"="Ch1 PID gains", "process variable"=w3793, "setpoint"=w3796) -> ("output"=w3791:dbl)  [unwired: 6 in, 1 out]
        n1711 = Power Of 10(x=w3791) -> (10^x=w3790:dbl)
        "Gain1" <- w3790
        n1712 = call "V1FGV.vi"("action (write)"=enum16{"write", "read"}."read") -> ("Error Out"=w3786:errorcluster, "V1 out"=w3788:dbl)  [unwired: 9 in]
        n1713 = call "GainToCtrlV.vi"("Gain"=w3790, "Channel"=enum16{"Ch1", "Ch2", "Ch3"}."Ch1") -> ("CtrlV"=w3785:dbl)  [unwired: 8 in, 1 out]
        n1714 = local write "V 1"(w3785) -> ()
        n1715 = call "V1FGV.vi"("Error In"=w3786, "V1 in"=w3785) -> ()  [unwired: 8 in, 2 out]
        n1716 = Not Equal?(x=w3785, y=w3788) -> (x != y?=w3787:bool)
      }
    }
    n1717 = case shown="True" w3721 {
      tunnel: w3715 -> [_ w3823]
      tunnel: "V target(1.0)" -> [_ w3824]
      tunnel: [FALSE w3817] -> w3711
      tunnel: [0.0 ("CtrlV") w3813] -> w3707
      frame False {
        # "Manual control"
      }
      frame True {
        # "PID control"
        n1718 = global read "GlobalVariables.vi" "Ch2GainLim(Log)"() -> (w3821:cluster{"GainMax":dbl, "GainMin":dbl})
        n1719 = call-poly <vilib>:"PID.vi"("output range"=w3821, "PID gains"="Ch2 PID gains", "process variable"=w3823, "setpoint"=w3824) -> ("output"=w3820:dbl)  [unwired: 6 in, 1 out]
        n1720 = Power Of 10(x=w3820) -> (10^x=w3818:dbl)
        "Gain2" <- w3818
        n1721 = call "V2FGV.vi"("action(write)"=enum16{"write", "read"}."read") -> ("Error Out"=w3814:errorcluster, "V2 out"=w3815:dbl)  [unwired: 9 in]
        n1722 = call "GainToCtrlV.vi"("Gain"=w3818, "Channel"=enum16{"Ch1", "Ch2", "Ch3"}."Ch2") -> ("CtrlV"=w3813:dbl)  [unwired: 8 in, 1 out]
        n1723 = local write "V 2"(w3813) -> ()
        n1724 = call "V2FGV.vi"("Error In"=w3814, "V2 in"=w3813) -> ()  [unwired: 8 in, 2 out]
        n1725 = Not Equal?(x=w3813, y=w3815) -> (x != y?=w3817:bool)
      }
    }
    n1726 = case shown="True" w3720 {
      tunnel: w3698 -> [_ w3808]
      tunnel: "V target(1.0)" -> [_ w3805]
      tunnel: [FALSE w3801] -> w3710
      tunnel: [0.0 ("CtrlV") w3799] -> w3709
      frame False {
        # "Manual control"
      }
      frame True {
        # "PID control"
        n1727 = global read "GlobalVariables.vi" "Ch3GainLim(Log)"() -> (w3809:cluster{"GainMax":dbl, "GainMin":dbl})
        n1728 = call-poly <vilib>:"PID.vi"("output range"=w3809, "PID gains"="Ch3 PID gains", "process variable"=w3808, "setpoint"=w3805) -> ("output"=w3807:dbl)  [unwired: 6 in, 1 out]
        n1729 = Power Of 10(x=w3807) -> (10^x=w3804:dbl)
        "Gain3" <- w3804
        n1730 = call "V3FGV.vi"("action(write)"=enum16{"write", "read"}."read") -> ("Error Out"=w3800:errorcluster, "V3 out"=w3802:dbl)  [unwired: 9 in]
        n1731 = call "GainToCtrlV.vi"("Gain"=w3804, "Channel"=enum16{"Ch1", "Ch2", "Ch3"}."Ch3") -> ("CtrlV"=w3799:dbl)  [unwired: 8 in, 1 out]
        n1732 = local write "V 3"(w3799) -> ()
        n1733 = call "V3FGV.vi"("Error In"=w3800, "V3 in"=w3799) -> ()  [unwired: 8 in, 2 out]
        n1734 = Not Equal?(x=w3799, y=w3802) -> (x != y?=w3801:bool)
      }
    }
    n1735 = call "LabJack_FGV.vi"("Operation(Read)"=enum16{"Write", "Read"}."Read" ("Operation"), "error in (no error)"=w3687) -> ("error out"=w3696:errorcluster, "Read data"=w3732:i32)  [unwired: 8 in]
    n1736 = flat-sequence {
      tunnel: [w3736] -> w3693
      tunnel: w3687 -> [_]
      frame #0 {
        n1737 = Tick Count (ms)() -> (millisecond timer value=w3736:u32)
      }
    }
    n1738 = case "Channel 1" shown="True" w3712 {
      tunnel: w3696 -> [w3762 w3768]
      tunnel: w3732 -> [w3761 w3767]
      tunnel: [w3762 w3763] -> w3691
      tunnel: [w3761 w3766] -> w3727
      tunnel: w3695 -> [_ w3764]
      frame False {
        # "Do nothing"
      }
      frame True {
        # "request V\nupdate FGV"
        n1739 = global read "GlobalVariables.vi" "Ch1 LJ pin"() -> (w3765:string)
        n1740 = call "LJM_eWriteName.vi"("Handle In"=w3767, "Name"=w3765, "Value"=w3764, "error in"=w3768) -> ("Handle Out"=w3766:i32, "error out"=w3763:errorcluster)  [unwired: 10 in]
      }
    }
    n1741 = case "Channel 2" shown="True" w3711 {
      tunnel: w3691 -> [w3753 w3760]
      tunnel: [w3753 w3755] -> w3690
      tunnel: w3727 -> [w3754 w3759]
      tunnel: [w3754 w3758] -> w3726
      tunnel: w3707 -> [_ w3756]
      frame False {
        # "Do nothing"
      }
      frame True {
        # "request V\nupdate FGV"
        n1742 = global read "GlobalVariables.vi" "Ch2 LJ pin"() -> (w3757:string)
        n1743 = call "LJM_eWriteName.vi"("Handle In"=w3759, "Name"=w3757, "Value"=w3756, "error in"=w3760) -> ("Handle Out"=w3758:i32, "error out"=w3755:errorcluster)  [unwired: 10 in]
      }
    }
    n1744 = case "Channel 3" shown="True" w3710 {
      tunnel: w3690 -> [w3746 w3752]
      tunnel: [w3746 w3748] -> w3689
      tunnel: w3726 -> [w3745 w3751]
      tunnel: w3709 -> [_ w3749]
      tunnel: [w3745 w3747] -> w3700
      frame False {
        # "Do nothing"
      }
      frame True {
        # "request V\nupdate FGV"
        n1745 = global read "GlobalVariables.vi" "Ch3 LJ pin"() -> (w3750:string)
        n1746 = call "LJM_eWriteName.vi"("Handle In"=w3751, "Name"=w3750, "Value"=w3749, "error in"=w3752) -> ("Handle Out"=w3747:i32, "error out"=w3748:errorcluster)  [unwired: 10 in]
      }
    }
    n1747 = case "Channel 4" shown="True" w3701 {
      tunnel: w3689 -> [w3738 w3744]
      tunnel: w3700 -> [w3737 w3743]
      tunnel: [w3738 w3739] -> w3694
      tunnel: [w3737 w3742] -> _
      tunnel: w3702 -> [_ w3740]
      frame False {
        # "Do nothing"
      }
      frame True {
        # "request V\nupdate FGV"
        n1748 = global read "GlobalVariables.vi" "Ch4 LJ pin"() -> (w3741:string)
        n1749 = call "LJM_eWriteName.vi"("Handle In"=w3743, "Name"=w3741, "Value"=w3740, "error in"=w3744) -> ("Handle Out"=w3742:i32, "error out"=w3739:errorcluster)  [unwired: 10 in]
      }
    }
    "PID loop error out" <- w3694
    n1750 = flat-sequence {
      tunnel: [w3735] -> w3692
      tunnel: w3694 -> [_]
      frame #0 {
        n1751 = Tick Count (ms)() -> (millisecond timer value=w3735:u32)
      }
    }
    n1752 = Subtract(x=w3692, y=w3693) -> (x-y=w3688:u32)
    "LJ process (ms)" <- w3688
    "PID loop" <- w3714
  }
  "LJ time(ms)" <- w13
  n1753 = while {
    tunnel: w29 -> [w3856]
    tunnel: w25 -> [w3849]
    tunnel: [w3848] -> w28
    shift-right: [w3840] -> _
    shift-left: _ -> [w3841]
    stop <- w3838 stop-if-true
    # "Read data from notifier and deconvolve it and send to Aiming Beam computer"
    n1754 = Wait on Notification(notifier=w3856, ignore previous (F)=FALSE) -> (notification=w3855:T17, error out=w3826:errorcluster)  [unwired: 2 in, 2 out]
    n1755 = flat-sequence {
      tunnel: [w3857] -> w3840
      tunnel: w3826 -> [_]
      frame #0 {
        n1756 = call <vilib>:"High Resolution Relative Seconds.vi"() -> ("relative seconds"=w3857:dbl)
      }
    }
    n1757 = Unbundle(w3855) -> ("CH1&2"=w3854:dbl[][], "CH3"=w3853:dbl[][], "V cluster"=w3844:cluster{"V1":dbl, "V2":dbl, "V3":dbl, "V4":dbl})  [unwired: 1 out]
    n1758 = call "SeperateChanData.vi"("Input (Ch1&2)"=w3854) -> ("Ch1"=w3836:dbl[][], "Ch2"=w3834:dbl[][])
    n1759 = call "SeperateChanData.vi"("Input (Ch1&2)"=w3853) -> ("Ch1"=w3832:dbl[][], "Ch2"=w3830:dbl[][])
    n1760 = Subtract(x=w3840, y=w3841) -> (x-y=w3843:dbl)
    n1761 = call "AvgArrayTimeCritical.vi"("2D array"=w3836) -> ("1D Avg"=w3835:dbl[])  [unwired: 10 in]
    n1762 = call "AvgArrayTimeCritical.vi"("2D array"=w3834) -> ("1D Avg"=w3833:dbl[])  [unwired: 10 in]
    n1763 = call "AvgArrayTimeCritical.vi"("2D array"=w3832) -> ("1D Avg"=w3831:dbl[])  [unwired: 10 in]
    n1764 = call "AvgArrayTimeCritical.vi"("2D array"=w3830) -> ("1D Avg"=w3829:dbl[])  [unwired: 10 in]
    n1765 = Multiply(x=w3843, y=1000.0) -> (x*y=→"Decon Loop timing (ms)" →"Waveform Chart":dbl)
    n1766 = case shown="\"Ch1\"" "Radio Buttons" {
      selector: "Radio Buttons" -> [_ w3870 w3884 w3899 w3916]
      tunnel: w3835 -> [w3867 w3878 w3890 w3904 w3920]
      tunnel: w3833 -> [w3865 w3875 w3892 w3902 w3918]
      tunnel: w3831 -> [w3863 w3873 w3887 w3907 w3910]
      tunnel: FALSE -> [_ w3881 w3895 w3909 w3923]
      tunnel: w3826 -> [w3861 w3880 w3894 w3898 w3915]
      tunnel: [w3861 w3879 w3893 w3908 w3922] -> w3838
      tunnel: [w3866 w3876 w3888 w3903 w3919] -> w3847
      tunnel: [w3864 w3874 w3889 w3901 w3917] -> w3846
      tunnel: [w3862 w3872 w3886 w3905 w3911] -> w3845
      tunnel: [0.0 ("lifetime (ns)") w3871 w3885 w3900 w3914] -> w3825
      tunnel: w3829 -> [w3859 w3869 w3883 w3897 w3913]
      tunnel: [w3858 w3868 w3882 w3896 w3912] -> w3828
      frame "No Selection", Default {
        n1767 = Build Array(w3867) -> (w3866:dbl[][])
        n1768 = Build Array(w3865) -> (w3864:dbl[][])
        n1769 = Build Array(w3863) -> (w3862:dbl[][])
        n1770 = Build Array(w3859) -> (w3858:dbl[][])
      }
      frame "Ch1" {
        n1771 = call "Deconvolution.vi"("DeconChannel"=w3870, "iRF align"=w3881, "error in (no error)"=w3880, "Waveform"=w3878) -> ("error out"=w3879:errorcluster, "lifetime (ns)"=w3871:dbl, "Fitting"=w3877:dbl[])  [unwired: 5 in]
        "Lifetime 1" <- w3871
        n1772 = Build Array(w3878, w3877) -> (w3876:dbl[][])
        n1773 = Build Array(w3875) -> (w3874:dbl[][])
        n1774 = Build Array(w3873) -> (w3872:dbl[][])
        n1775 = Build Array(w3869) -> (w3868:dbl[][])
      }
      frame "Ch2" {
        n1776 = call "Deconvolution.vi"("DeconChannel"=w3884, "iRF align"=w3895, "error in (no error)"=w3894, "Waveform"=w3892) -> ("error out"=w3893:errorcluster, "lifetime (ns)"=w3885:dbl, "Fitting"=w3891:dbl[])  [unwired: 5 in]
        "Lifetime 2" <- w3885
        n1777 = Build Array(w3890) -> (w3888:dbl[][])
        n1778 = Build Array(w3892, w3891) -> (w3889:dbl[][])
        n1779 = Build Array(w3887) -> (w3886:dbl[][])
        n1780 = Build Array(w3883) -> (w3882:dbl[][])
      }
      frame "Ch3" {
        n1781 = call "Deconvolution.vi"("DeconChannel"=w3899, "iRF align"=w3909, "error in (no error)"=w3898, "Waveform"=w3907) -> ("error out"=w3908:errorcluster, "lifetime (ns)"=w3900:dbl, "Fitting"=w3906:dbl[])  [unwired: 5 in]
        "Lifetime 3" <- w3900
        n1782 = Build Array(w3904) -> (w3903:dbl[][])
        n1783 = Build Array(w3902) -> (w3901:dbl[][])
        n1784 = Build Array(w3907, w3906) -> (w3905:dbl[][])
        n1785 = Build Array(w3897) -> (w3896:dbl[][])
      }
      frame "Ch4" {
        n1786 = call "Deconvolution.vi"("DeconChannel"=w3916, "iRF align"=w3923, "error in (no error)"=w3915, "Waveform"=w3913) -> ("error out"=w3922:errorcluster, "lifetime (ns)"=w3914:dbl, "Fitting"=w3921:dbl[])  [unwired: 5 in]
        "Lifetime 4" <- w3914
        n1787 = Build Array(w3920) -> (w3919:dbl[][])
        n1788 = Build Array(w3918) -> (w3917:dbl[][])
        n1789 = Build Array(w3913, w3921) -> (w3912:dbl[][])
        n1790 = Build Array(w3910) -> (w3911:dbl[][])
      }
    }
    "Lifetime (ns)" <- w3825
    n1791 = Bundle(w3847, w3846, w3845, w3828, "V cluster"=w3844) -> (w3850:T58)  [unwired: 1 in]
    n1792 = Send Notification(notification=w3850, notifier=w3849, error in (no error)=w3838) -> (notifier out=w3848:refnum<notifier>, error out=→"decon error out":errorcluster)
  }
  n1793 = while {
    tunnel: w9 -> [w3926]
    tunnel: w8 -> [w3925]
    tunnel: [w3924] -> w6
    stop <- w3927 stop-if-true
    n1794 = event shown="[1] <startCam>: User Event" {
      selector: w3926 -> [_ _]
      dyn-events: [_ _] -> w3924
      timeout: 30 -> [_ _]
      tunnel: [w3930 _] -> w3927
      tunnel: w3925 -> [w3929 _]
      event Timeout {
        # "if queue is destoried, stop cam loop"
        n1795 = event-data() -> ()  [unwired: 1 in, 3 out]
        n1796 = Get Queue Status(queue=w3929) -> (error out=w3930:errorcluster)  [unwired: 2 in, 7 out]
      }
      event User Event {
        n1797 = event-data() -> ("savePath"=w3935:path, "saveData?"=w3936:bool)  [unwired: 1 in, 4 out]
        n1798 = call "USBCAM_FGV.vi"() -> ("error out"=w3939:errorcluster, "Session Out"=w3940:T26)  [unwired: 10 in]
        n1799 = call "IMAQ Create"("Image Name"="Acquire Most Recent Image") -> ("New Image"=w3937:T1, "error out"=w3934:errorcluster)  [unwired: 3 in, 1 out]
        n1800 = while {
          tunnel: w3940 -> [w3962]
          shift-right: [w3952] -> w3932
          shift-left: w3939 -> [w3961]
          tunnel: w3937 -> [w3959]
          tunnel: [w3956] -> w3931 mode=indexing
          tunnel: w3936 -> [w3955]
          tunnel: w3935 -> [w3954]
          tunnel: [w3950] -> w3933
          i -> [w3951]
          stop <- w3953 stop-if-true
          n1801 = call <vilib>:"IMAQdx Get Image2.vi"("Timeout (ms)"=2000, "Buffer Number Mode (Next)"=IMAQdx_Buffer_Number_Mode."Next", "error in"=w3961, "Image In"=w3959, "Session In"=w3962) -> ("error out"=w3953:errorcluster, "Buffer Number Out"=w3958:u32, "Image Out"=w3950:T1)  [unwired: 3 in, 1 out]
          "Image 2" <- w3950
          n1802 = call <vilib>:"Calculate Frames per Second.vi"("Buffer Number"=w3958) -> ("Acquired Frames/s"=→"Acquired Frames/s":dbl)  [unwired: 8 in, 2 out]
          n1803 = call "High Resolution Timer Helper.vi"("error in (no error)"=w3953) -> ("error out"=w3949:errorcluster, "Current Time"=w3956:dbl)  [unwired: 8 in, 1 out]
          n1804 = case shown="True" w3955 {
            tunnel: w3950 -> [_ w3976]
            tunnel: w3954 -> [_ w3974]
            tunnel: w3949 -> [w3964 w3970]
            tunnel: [w3964 w3965] -> w3952
            tunnel: w3951 -> [_ w3973]
            frame False {
            }
            frame True {
              n1805 = Format Into String(format string="Image %04d.png", w3973) -> (resulting string=w3975:string)  [unwired: 2 in, 1 out]
              n1806 = call "High Resolution Timer Helper.vi"("error in (no error)"=w3970) -> ("error out"=w3966:errorcluster, "Current Time"=w3968:dbl)  [unwired: 8 in, 1 out]
              n1807 = Build Path(base path=w3974, name or relative path=w3975) -> (appended path=w3971:path)
              n1808 = call-poly "IMAQ Write File 2"("error in (no error)"=w3966, "File Path"=w3971, "Image"=w3976) -> ("error out"=w3969:errorcluster)  [unwired: 7 in, 1 out]
              n1809 = call "High Resolution Timer Helper.vi"("error in (no error)"=w3969, "Previous Time"=w3968) -> ("error out"=w3965:errorcluster, "Time Difference (ms)"=→"PNG write time (ms)":dbl)  [unwired: 7 in, 1 out]
            }
          }
        }
        "Cam error out" <- w3932
        n1810 = case shown="True" w3936 {
          tunnel: w3935 -> [_ w3947]
          tunnel: w3939 -> [_ w3944]
          tunnel: w3931 -> [_ w3943]
          frame False {
          }
          frame True {
            n1811 = local read "FLIm 1st point time"() -> (w3941:dbl)
            n1812 = Subtract(x=w3943, y=w3941) -> (x-y=w3942:dbl[])
            n1813 = Build Path(base path=w3947, name or relative path="TimeSych.txt") -> (appended path=w3945:path)
            n1814 = call-poly <vilib>:"Write Delimited Spreadsheet.vi"("file path (dialog if empty)"=w3945, "format (%.3f)"="%.5f", "1D data"=w3942, "error in (no error)"=w3944) -> ()  [unwired: 10 in, 2 out]
          }
        }
        n1815 = call "Imaq Dispose"("Image"=w3933, "error in (no error)"=w3934) -> ()  [unwired: 4 in, 1 out]
      }
    }
  }
  n1816 = while {
    tunnel: w1 -> [w3991]
    stop <- w3990 stop-if-true
    # "stage control loop, wait for notifier to run once"
    n1817 = Wait on Notification(notifier=w3991) -> (notification=w3985:dbl, error out=w3990:errorcluster)  [unwired: 3 in, 2 out]
    n1818 = call "Stage_FGV.vi"("error in (no error)"=w3990) -> ("error out"=w3984:errorcluster, "reference out"=w3986:refnum<k24>)  [unwired: 9 in]
    n1819 = invoke class="KCubeDCServo" method="SetMoveAbsolutePosition"(reference=w3986, error in=w3984, "position"=w3985) -> (reference out=w3989:refnum<k24>, error out=w3988:errorcluster)  [unwired: 1 in, 2 out]
    n1820 = invoke class="KCubeDCServo" method="MoveAbsolute"(reference=w3989, error in=w3988, "waitTimeout"=20000) -> (reference out=w3977:refnum<k24>, error out=w3980:errorcluster)  [unwired: 1 in, 2 out]
    n1821 = invoke class="KCubeDCServo" method="SetMoveAbsolutePosition"(reference=w3977, error in=w3980, "position"=0.0) -> (reference out=w3983:refnum<k24>, error out=w3982:errorcluster)  [unwired: 1 in, 2 out]
    n1822 = invoke class="KCubeDCServo" method="MoveAbsolute"(reference=w3983, error in=w3982, "waitTimeout"=20000) -> (error out=w3978:errorcluster)  [unwired: 1 in, 3 out]
    n1823 = flat-sequence {
      tunnel: w3978 -> [_]
      frame #0 {
        n1824 = property on="StopButton" class="Bool (strict)"("Val(Sgnl)"=TRUE ("Value (Signaling)")) -> (error out=w3993:errorcluster)  [unwired: 2 in, 1 out]
        n1825 = property on="StopButton" class="Bool (strict)"(error in=w3993, "Value"=FALSE ("StopButton")) -> ()  [unwired: 1 in, 2 out]
      }
    }
  }
  n1826 = while {
    tunnel: w25 -> [w4005]
    shift-right: [w3996] -> _
    shift-left: w27 -> [w4003]
    shift-right: [w3998] -> _
    shift-left: w27 -> [w3997]
    i -> [w3999]
    stop <- w4000 stop-if-true
    # "Data display loop(30Hz)"
    n1827 = Wait on Notification(notifier=w4005, ignore previous (F)=FALSE) -> (notification=w4001:T16, error out=w4000:errorcluster)  [unwired: 2 in, 2 out]
    n1828 = Wait Until Next ms Multiple(millisecond multiple=u32 33) -> ()  [unwired: 1 out]
    n1829 = Tick Count (ms)() -> (millisecond timer value=w3996:u32)
    n1830 = Subtract(x=w3996, y=w4003) -> (x-y=→"display loop timing(ms)":u32)
    n1831 = case shown="No Error" w4000 {
      tunnel: w4001 -> [w4078 _]
      tunnel: w3997 -> [w4050 w4150]
      tunnel: [w4052 w4150] -> w3998
      tunnel: w3996 -> [w4049 _]
      frame No Error {
        w4007 = u32 1 ("Active Plot")
        w4026 = 0 ("index (row)")
        n1832 = Subtract(x=w4049, y=w4050) -> (x-y=w4051:u32)
        n1833 = Unbundle(w4078) -> ("CH1"=w4073:dbl[][], "CH2"=w4071:dbl[][], "CH3"=w4068:dbl[][], "CH4"=w4021:dbl[][], "Gain cluster"=w4027:cluster{"V1":dbl, "V2":dbl, "V3":dbl, "V4":dbl})
        n1834 = Unbundle By Name(w4027) -> ("V1"=w4045:dbl, "V2"=w4043:dbl, "V3"=w4041:dbl, "V4"=w4019:dbl)
        n1835 = Index Array(array=w4073, index (row)=w4026) -> (element=w4057:dbl[])  [unwired: 1 in]
        n1836 = Index Array(array=w4071, index (row)=w4026) -> (element=w4055:dbl[])  [unwired: 1 in]
        n1837 = Index Array(array=w4068, index (row)=w4026) -> (element=w4056:dbl[])  [unwired: 1 in]
        n1838 = Index Array(array=w4021, index (row)=w4026) -> (element=w4025:dbl[])  [unwired: 1 in]
        n1839 = call "RemoveDCBG.vi"("Channel"=enum16{"DC Only", "Ch1", "Ch2", "Ch3", "Ch4"}."Ch4", "WF in"=w4025) -> ("DC"=w4023:dbl, "WF out"=w4012:dbl[])  [unwired: 7 in, 1 out]
        n1840 = Greater?(x=w4051, y=u32 200) -> (0:w4053:bool)
        n1841 = call "CtrlVtoGain.vi"("CtrlV(V)"=w4019, "Channel"=enum16{"Ch1", "Ch2", "Ch3", "Ch4"}."Ch4") -> ("Gain"=w4011:dbl)  [unwired: 8 in, 1 out]
        n1842 = call "CtrlVtoGain.vi"("CtrlV(V)"=w4045, "Channel"=enum16{"Ch1", "Ch2", "Ch3"}."Ch1") -> ("Gain"=w4039:dbl)  [unwired: 8 in, 1 out]
        n1843 = call "RemoveDCBG.vi"("Channel"=enum16{"DC Only", "Ch1", "Ch2", "Ch3"}."Ch1", "WF in"=w4057) -> ("DC"=w4074:dbl, "WF out"=w4046:dbl[])  [unwired: 7 in, 1 out]
        n1844 = call "RemoveDCBG.vi"("Channel"=enum16{"DC Only", "Ch1", "Ch2", "Ch3"}."Ch2", "WF in"=w4055) -> ("DC"=w4070:dbl, "WF out"=w4047:dbl[])  [unwired: 7 in, 1 out]
        n1845 = call "CtrlVtoGain.vi"("CtrlV(V)"=w4043, "Channel"=enum16{"Ch1", "Ch2", "Ch3"}."Ch2") -> ("Gain"=w4034:dbl)  [unwired: 8 in, 1 out]
        n1846 = call "RemoveDCBG.vi"("Channel"=enum16{"DC Only", "Ch1", "Ch2", "Ch3"}."Ch3", "WF in"=w4056) -> ("DC"=w4067:dbl, "WF out"=w4048:dbl[])  [unwired: 7 in, 1 out]
        n1847 = call "CtrlVtoGain.vi"("CtrlV(V)"=w4041, "Channel"=enum16{"Ch1", "Ch2", "Ch3"}."Ch3") -> ("Gain"=w4030:dbl)  [unwired: 8 in, 1 out]
        n1848 = formula code="int32 out = 2;\nif (G<5){\nout = 1;\n}\nif (G>200){\nout = 3;\n}"("G"=w4011) -> ("out"=→"output variable":i32)
        n1849 = Add(x=w4012, y=w4023) -> (x+y=w4022:dbl[])
        n1850 = Less?(x=w4011, y=5.0) -> (x < y?=w4017:bool)
        n1851 = case shown="True" w4053 {
          tunnel: w4046 -> [_ w4107]
          tunnel: w4047 -> [_ w4110]
          tunnel: w4048 -> [_ w4109]
          tunnel: w4049 -> [_ w4125]
          tunnel: [w4089 w4125] -> w4052
          tunnel: w4050 -> [w4089 _]
          tunnel: w4039 -> [_ w4103]
          tunnel: w4034 -> [_ w4102]
          tunnel: w4030 -> [_ w4101]
          tunnel: w4012 -> [_ w4097]
          tunnel: w4011 -> [_ w4094]
          frame False {
          }
          frame True {
            n1852 = call "GetSNR(SubVI).vi"("Waveform"=w4107) -> ("SNR"=→"SNR1":dbl)  [unwired: 10 in]
            n1853 = Array Size(array=w4107) -> (size(s)=w4108:i32)
            n1854 = call "GetSNR(SubVI).vi"("Waveform"=w4110) -> ("SNR"=→"SNR2":dbl)  [unwired: 10 in]
            n1855 = call "GetSNR(SubVI).vi"("Waveform"=w4109) -> ("SNR"=→"SNR3":dbl)  [unwired: 10 in]
            n1856 = call "GetSNR(SubVI).vi"("Waveform"=w4097) -> ("SNR"=→"SNR4":dbl)  [unwired: 10 in]
            n1857 = global read "GlobalVariables.vi" "BG Idx2"() -> (w4096:i32)
            n1858 = Subtract(x=w4108, y=w4096) -> (x-y=w4095:i32)
            n1859 = Array Subset(array=w4107, index=w4096, length=w4095) -> (w4114:dbl[])
            n1860 = Array Subset(array=w4110, index=w4096, length=w4095) -> (w4116:dbl[])
            n1861 = Array Subset(array=w4109, index=w4096, length=w4095) -> (w4118:dbl[])
            n1862 = Array Subset(array=w4097, index=w4096, length=w4095) -> (w4098:dbl[])
            n1863 = Add Array Elements(numeric array=w4114) -> (sum=w4115:dbl)
            n1864 = Add Array Elements(numeric array=w4116) -> (sum=w4117:dbl)
            n1865 = Add Array Elements(numeric array=w4118) -> (sum=w4119:dbl)
            n1866 = Add Array Elements(numeric array=w4098) -> (sum=w4099:dbl)
            n1867 = Divide(x=w4115, y=w4103) -> (x/y=w4120:dbl)
            n1868 = Divide(x=w4117, y=w4102) -> (x/y=w4121:dbl)
            n1869 = Divide(x=w4119, y=w4101) -> (x/y=w4122:dbl)
            n1870 = Divide(x=w4099, y=w4094) -> (x/y=w4093:dbl)
            n1871 = Build Array(w4120, w4121, w4122, w4093) -> (w4123:dbl[])
            n1872 = Add Array Elements(numeric array=w4123) -> (sum=w4124:dbl)
            n1873 = Divide(x=w4123, y=w4124) -> (x/y=w4092:dbl[])
            n1874 = Index Array(array=w4092, index=2) -> (element=→"IntR3":dbl)
            n1875 = Index Array(array=w4092, index=1) -> (element=→"IntR2":dbl)
            n1876 = Index Array(array=w4092, index=0) -> (element=→"IntR1":dbl)
            n1877 = Index Array(array=w4092, index=3) -> (element=→"IntR4":dbl)
          }
        }
        n1878 = Add(x=w4046, y=w4074) -> (x+y=w4072:dbl[])
        n1879 = Add(x=w4047, y=w4070) -> (x+y=w4069:dbl[])
        n1880 = Add(x=w4048, y=w4067) -> (x+y=w4066:dbl[])
        n1881 = Less?(x=w4039, y=5.0 ("x")) -> (x < y?=w4037:bool)
        n1882 = Less?(x=w4034, y=5.0 ("x")) -> (x < y?=w4033:bool)
        n1883 = Less?(x=w4030, y=5.0 ("x")) -> (x < y?=w4029:bool)
        n1884 = case shown="False" w4029 {
          tunnel: [u32 16448250 ("Plot.Plot Color") u32 16711680 ("Plot.Plot Color")] -> w4028
          frame False {
          }
          frame True {
          }
        }
        n1885 = case shown="True" "Show BG removed?" {
          tunnel: w4073 -> [w4132 w4148]
          tunnel: w4072 -> [_ w4138]
          tunnel: [w4132 w4147] -> w4065
          tunnel: w4071 -> [w4131 w4146]
          tunnel: [w4131 w4145] -> w4009
          tunnel: w4069 -> [_ w4134]
          tunnel: w4068 -> [w4130 w4144]
          tunnel: [w4130 w4143] -> w4060
          tunnel: w4066 -> [_ w4139]
          tunnel: [w4129 w4142] -> w4016
          tunnel: w4022 -> [_ w4136]
          tunnel: w4021 -> [w4129 w4141]
          frame False {
          }
          frame True {
            n1886 = Insert Into Array(array=w4144, index (row)=1, new element=w4139) -> (w4143:dbl[][])  [unwired: 1 in]
            n1887 = Insert Into Array(array=w4148, index (row)=1, new element=w4138) -> (w4147:dbl[][])  [unwired: 1 in]
            n1888 = Insert Into Array(array=w4146, index (row)=1, new element=w4134) -> (w4145:dbl[][])  [unwired: 1 in]
            n1889 = Insert Into Array(array=w4141, index (row)=1, new element=w4136) -> (w4142:dbl[][])  [unwired: 1 in]
          }
        }
        "Channel 1" <- w4065
        "Channel 2" <- w4009
        "Channel 3" <- w4060
        "Channel 4" <- w4016
        n1890 = case shown="False" w4037 {
          tunnel: [u32 16448250 ("Plot.Plot Color") u32 16711680 ("Plot.Plot Color")] -> w4036
          frame False {
          }
          frame True {
          }
        }
        n1891 = case shown="False" w4033 {
          tunnel: [u32 16448250 ("Plot.Plot Color") u32 16711680 ("Plot.Plot Color")] -> w4032
          frame False {
          }
          frame True {
          }
        }
        n1892 = case shown="False" w4017 {
          tunnel: [u32 16448250 ("Plot.Plot Color") u32 16711680 ("Plot.Plot Color")] -> w4013
          frame False {
          }
          frame True {
          }
        }
        n1893 = case shown="False" "Show BG removed?" {
          tunnel: [u32 16744703 ("Plot.Plot Color") u32 16741120 ("Plot.Plot Color")] -> w4006
          frame False {
          }
          frame True {
          }
        }
        n1894 = property on="Channel 1" class="WFGraph (strict)"("Active Plot"=w4007, "Plot.Plot Color"=w4006, "Plot.Line Style"=u8 1, "Plot.Line Width"=u8 2, "BG Color"=w4036) -> ()  [unwired: 2 in, 2 out]
        n1895 = property on="Channel 2" class="WFGraph (strict)"("Active Plot"=w4007, "Plot.Plot Color"=w4006, "Plot.Line Style"=u8 1, "Plot.Line Width"=u8 2, "BG Color"=w4032) -> ()  [unwired: 2 in, 2 out]
        n1896 = property on="Channel 4" class="WFGraph (strict)"("Active Plot"=w4007, "Plot.Plot Color"=w4006, "Plot.Line Style"=u8 1, "Plot.Line Width"=u8 2, "BG Color"=w4013) -> ()  [unwired: 2 in, 2 out]
        n1897 = property on="Channel 3" class="WFGraph (strict)"("Active Plot"=w4007, "Plot.Plot Color"=w4006, "Plot.Line Style"=u8 1, "Plot.Line Width"=u8 2, "BG Color"=w4028) -> ()  [unwired: 2 in, 2 out]
      }
      frame Error {
        w4149 = u32 16448250 ("Plot Area:Colors:BG Color")
        n1898 = property on="Channel 1" class="WFGraph (strict)"("BG Color"=w4149) -> ()  [unwired: 2 in, 2 out]
        n1899 = property on="Channel 2" class="WFGraph (strict)"("BG Color"=w4149) -> ()  [unwired: 2 in, 2 out]
        n1900 = property on="Channel 3" class="WFGraph (strict)"("BG Color"=w4149) -> ()  [unwired: 2 in, 2 out]
      }
    }
    "DisplayLoop" <- w3999
  }
  n1901 = Release Notifier(notifier=w28, error in (no error)=w52) -> (error out=w53:errorcluster)  [unwired: 1 in, 2 out]
  n1902 = Unregister For Events(event registration refnum=w50, error in=w16) -> (error out=w55:errorcluster)
  n1903 = call <vilib>:"Simple Error Handler.vi"("error in (no error)"=w53) -> ()  [unwired: 4 in, 5 out]
  n1904 = Destroy User Event(user event=w47, error in=w55) -> (error out=w15:errorcluster)
  n1905 = Unregister For Events(event registration refnum=w6) -> (error out=w7:errorcluster)  [unwired: 1 in]
  n1906 = Close File(refnum=w31, error in=w15) -> ()  [unwired: 2 out]
  n1907 = Destroy User Event(user event=w5, error in=w7) -> ()  [unwired: 1 out]
  n1908 = Release Notifier(notifier=w62, error in (no error)=w61) -> (error out=w60:errorcluster)  [unwired: 1 in, 2 out]
  n1909 = Unregister For Events(event registration refnum=w66, error in=w64) -> (error out=w65:errorcluster)
  n1910 = call <vilib>:"Simple Error Handler.vi"("error in (no error)"=w60) -> ()  [unwired: 4 in, 5 out]
  n1911 = Destroy User Event(user event=w56, error in=w65) -> ()  [unwired: 1 out]
